vi "ParseResults.vi"(8 "error in (no error)":errorcluster, 10 "Path":path=path "C:/temp/MEScannerF1_262_153145_G16_PD_TS_v3__G16_OC_TS_v2.txt", 11 "Sequence Context In":refnum<k7>) -> (0 "error out":errorcluster, 1 "Array":T1[](array[typedef])=[{"Test_Name"="59. GetScannerDeviceType", "Step_Type"="StringValueTest", "LowLimit"=0.0, "HighLimit"=0.0, "RValue"="7", "RStatus"="PASS", "RetVal"="0", "Units"="", "header1"="", "header2"="\r", "ExpectedValue"=""}, {"Test_Name"="66. PromptUserPassFail \"Please listen for a beep!\" \"OK\" \"Cancel\"", "Step_Type"="StringValueTest", "LowLimit"=0.0, "HighLimit"=0.0, "RValue"="True", "RStatus"="PASS", "RetVal"="None", "Units"="", "header1"="", "header2"="\r\r", "ExpectedValue"=""}, {"Test_Name"="67. Beep", "Step_Type"="", "LowLimit"=0.0, "HighLimit"=0.0, "RValue"="", "RStatus"="", "RetVal"="0", "Units"="", "header1"="", "header2"="\r\r\r", "ExpectedValue"=""}, {"Test_Name"="68. PromptUserPassFail \"Did you hear a beep?\" \"YES\" \"NO\"", "Step_Type"="StringValueTest", "LowLimit"=0.0, "HighLimit"=0.0, "RValue"="True", "RStatus"="PASS", "RetVal"="None", "Units"="", "header1"="", "header2"="\r\r\r\r", "ExpectedValue"=""}, {"Test_Name"="71. SetDebugLEDs \"1\"", "Step_Type"="", "LowLimit"=0.0, "HighLimit"=0.0, "RValue"="", "RStatus"="", "RetVal"="0", "Units"="", "header1"="", "header2"="\r\r\r\r\r", "ExpectedValue"=""}, {"Test_Name"="72. PromptUserPassFail \"Did you Verify the 2 LEDs turn on near uSD connector?\" \"YES\" \"NO\"", "Step_Type"="StringValueTest", "LowLimit"=0.0, "HighLimit"=0.0, "RValue"="True", "RStatus"="PASS", "RetVal"="None", "Units"="", "header1"="", "header2"="\r\r\r\r\r\r", "ExpectedValue"=""}, {"Test_Name"="73. SetDebugLEDs \"0\"", "Step_Type"="", "LowLimit"=0.0, "HighLimit"=0.0, "RValue"="", "RStatus"="", "RetVal"="0", "Units"="", "header1"="", "header2"="\r\r\r\r\r\r\r", "ExpectedValue"=""}, {"Test_Name"="93. --- Pin Driver Complete Test ---", "Step_Type"="", "LowLimit"=0.0, "HighLimit"=0.0, "RValue"="", "RStatus"="", "RetVal"="", "Units"="", "header1"="", "header2"="--- Pin Driver Complete Test -----------\r", "ExpectedValue"=""}, {"Test_Name"="96. SetG15PullupVbat \"0\" \"0\"", "Step_Type"="", "LowLimit"=0.0, "HighLimit"=0.0, "RValue"="", "RStatus"="", "RetVal"="0", "Units"="", "header1"="", "header2"="--- Pin Driver Complete Test -----------\r\r", "ExpectedValue"=""}, {"Test_Name"="97. SetG15PullUp \"A\" \"0\"", "Step_Type"="", "LowLimit"=0.0, "HighLimit"=0.0, "RValue"="", "RStatus"="", "RetVal"="0", "Units"="", "header1"="", "header2"="--- Pin Driver Complete Test -----------\r\r\r", "ExpectedValue"=""}, {"Test_Name"="98. SetG15PullUp \"B\" \"0\"", "Step_Type"="", "LowLimit"=0.0, "HighLimit"=0.0, "RValue"="", "RStatus"="", "RetVal"="0", "Units"="", "header1"="", "header2"="--- Pin Driver Complete Test -----------\r\r\r\r", "ExpectedValue"=""}, {"Test_Name"="99. SetG15PullDown \"A\" \"0\"", "Step_Type"="", "LowLimit"=0.0, "HighLimit"=0.0, "RValue"="", "RStatus"="", "RetVal"="0", "Units"="", "header1"="", "header2"="--- Pin Driver Complete Test -----------\r\r\r\r\r", "ExpectedValue"=""}, {"Test_Name"="100. SetG15PullDown \"B\" \"0\"", "Step_Type"="", "LowLimit"=0.0, "HighLimit"=0.0, "RValue"="", "RStatus"="", "RetVal"="0", "Units"="", "header1"="", "header2"="--- Pin Driver Complete Test -----------\r\r\r\r\r\r", "ExpectedValue"=""}, {"Test_Name"="101. SelectAllMuxA \"1\" \"0\"", "Step_Type"="", "LowLimit"=0.0, "HighLimit"=0.0, "RValue"="", "RStatus"="", "RetVal"="0", "Units"="", "header1"="", "header2"="--- Pin Driver Complete Test -----------\r\r\r\r\r\r\r", "ExpectedValue"=""}, {"Test_Name"="102. SelectAllMuxB \"1\" \"0\"", "Step_Type"="", "LowLimit"=0.0, "HighLimit"=0.0, "RValue"="", "RStatus"="", "RetVal"="0", "Units"="", "header1"="", "header2"="--- Pin Driver Complete Test -----------\r\r\r\r\r\r\r\r", "ExpectedValue"=""}, {"Test_Name"="103. SetG15PullUp \"C\" \"0\"", "Step_Type"="", "LowLimit"=0.0, "HighLimit"=0.0, "RValue"="", "RStatus"="", "RetVal"="0", "Units"="", "header1"="", "header2"="--- Pin Driver Complete Test -----------\r\r\r\r\r\r\r\r\r", "ExpectedValue"=""}, {"Test_Name"="104. SetG15PullUp \"D\" \"0\"", "Step_Type"="", "LowLimit"=0.0, "HighLimit"=0.0, "RValue"="", "RStatus"="", "RetVal"="0", "Units"="", "header1"="", "header2"="--- Pin Driver Complete Test -----------\r\r\r\r\r\r\r\r\r\r", "ExpectedValue"=""}, {"Test_Name"="105. SetG15PullDown \"C\" \"0\"", "Step_Type"="", "LowLimit"=0.0, "HighLimit"=0.0, "RValue"="", "RStatus"="", "RetVal"="0", "Units"="", "header1"="", "header2"="--- Pin Driver Complete Test -----------\r\r\r\r\r\r\r\r\r\r\r", "ExpectedValue"=""}, {"Test_Name"="106. SetG15PullDown \"D\" \"0\"", "Step_Type"="", "LowLimit"=0.0, "HighLimit"=0.0, "RValue"="", "RStatus"="", "RetVal"="0", "Units"="", "header1"="", "header2"="--- Pin Driver Complete Test -----------\r\r\r\r\r\r\r\r\r\r\r\r", "ExpectedValue"=""}, {"Test_Name"="107. SelectAllMuxA \"2\" \"0\"", "Step_Type"="", "LowLimit"=0.0, "HighLimit"=0.0, "RValue"="", "RStatus"="", "RetVal"="0", "Units"="", "header1"="", "header2"="--- Pin Driver Complete Test -----------\r\r\r\r\r\r\r\r\r\r\r\r\r", "ExpectedValue"=""}, {"Test_Name"="108. SelectAllMuxB \"2\" \"0\"", "Step_Type"="", "LowLimit"=0.0, "HighLimit"=0.0, "RValue"="", "RStatus"="", "RetVal"="0", "Units"="", "header1"="", "header2"="--- Pin Driver Complete Test -----------\r\r\r\r\r\r\r\r\r\r\r\r\r\r", "ExpectedValue"=""}, {"Test_Name"="109. SelectAllPins \"0\"", "Step_Type"="", "LowLimit"=0.0, "HighLimit"=0.0, "RValue"="", "RStatus"="", "RetVal"="0", "Units"="", "header1"="", "header2"="--- Pin Driver Complete Test -----------\r\r\r\r\r\r\r\r\r\r\r\r\r\r\r", "ExpectedValue"=""}, {"Test_Name"="110. ResetAsicRegister \"1\" \"ALL\"", "Step_Type"="", "LowLimit"=0.0, "HighLimit"=0.0, "RValue"="", "RStatus"="", "RetVal"="0", "Units"="", "header1"="", "header2"="--- Pin Driver Complete Test -----------\r\r\r\r\r\r\r\r\r\r\r\r\r\r\r\r", "ExpectedValue"=""}, {"Test_Name"="111. ResetAsicRegister \"2\" \"ALL\"", "Step_Type"="", "LowLimit"=0.0, "HighLimit"=0.0, "RValue"="", "RStatus"="", "RetVal"="0", "Units"="", "header1"="", "header2"="--- Pin Driver Complete Test -----------\r\r\r\r\r\r\r\r\r\r\r\r\r\r\r\r\r", "ExpectedValue"=""}, {"Test_Name"="112. SetFpgaRegister \"129\" \"0\"", "Step_Type"="", "LowLimit"=0.0, "HighLimit"=0.0, "RValue"="", "RStatus"="", "RetVal"="0", "Units"="", "header1"="", "header2"="--- Pin Driver Complete Test -----------\r\r\r\r\r\r\r\r\r\r\r\r\r\r\r\r\r\r", "ExpectedValue"=""}, {"Test_Name"="113. SetFpgaRegister \"8AD\" \"1\"", "Step_Type"="", "LowLimit"=0.0, "HighLimit"=0.0, "RValue"="", "RStatus"="", "RetVal"="0", "Units"="", "header1"="", "header2"="--- Pin Driver Complete Test -----------\r\r\r\r\r\r\r\r\r\r\r\r\r\r\r\r\r\r\r", "ExpectedValue"=""}, {"Test_Name"="115. ---CHECK System MEMORY---", "Step_Type"="", "LowLimit"=0.0, "HighLimit"=0.0, "RValue"="", "RStatus"="", "RetVal"="", "Units"="", "header1"="", "header2"="---CHECK System MEMORY------------------\r", "ExpectedValue"=""}, {"Test_Name"="116. CheckSystemMemory", "Step_Type"="", "LowLimit"=0.0, "HighLimit"=0.0, "RValue"="", "RStatus"="", "RetVal"="0", "Units"="", "header1"="", "header2"="---CHECK System MEMORY------------------\r\r", "ExpectedValue"=""}, {"Test_Name"="118. --- Software Verification ---", "Step_Type"="", "LowLimit"=0.0, "HighLimit"=0.0, "RValue"="", "RStatus"="", "RetVal"="", "Units"="", "header1"="", "header2"="--- Software Verification --------------\r", "ExpectedValue"=""}, {"Test_Name"="119. CheckTestAppVersion \"2.6\"", "Step_Type"="StringValueTest", "LowLimit"=0.0, "HighLimit"=0.0, "RValue"="2.6", "RStatus"="PASS", "RetVal"="None", "Units"="", "header1"="", "header2"="--- Software Verification --------------\r\r", "ExpectedValue"=""}, {"Test_Name"="120. CheckFPGAVersion \"2.7\"", "Step_Type"="StringValueTest", "LowLimit"=0.0, "HighLimit"=0.0, "RValue"="2.7", "RStatus"="PASS", "RetVal"="None", "Units"="", "header1"="", "header2"="--- Software Verification --------------\r\r\r", "ExpectedValue"=""}, {"Test_Name"="121. CheckIPLVersion \"0.6\"", "Step_Type"="StringValueTest", "LowLimit"=0.0, "HighLimit"=0.0, "RValue"="0.6", "RStatus"="PASS", "RetVal"="None", "Units"="", "header1"="", "header2"="--- Software Verification --------------\r\r\r\r", "ExpectedValue"=""}, {"Test_Name"="122. CheckSPL1Version \"0.8\"", "Step_Type"="StringValueTest", "LowLimit"=0.0, "HighLimit"=0.0, "RValue"="0.8", "RStatus"="PASS", "RetVal"="None", "Units"="", "header1"="", "header2"="--- Software Verification --------------\r\r\r\r\r", "ExpectedValue"=""}, {"Test_Name"="125. SetRealtimeClock", "Step_Type"="", "LowLimit"=0.0, "HighLimit"=0.0, "RValue"="", "RStatus"="", "RetVal"="0", "Units"="", "header1"="", "header2"="--- Software Verification --------------\r\r\r\r\r\r", "ExpectedValue"=""}, {"Test_Name"="127. ---   ADC VEHICLE VBAT check ---", "Step_Type"="", "LowLimit"=0.0, "HighLimit"=0.0, "RValue"="", "RStatus"="", "RetVal"="", "Units"="", "header1"="", "header2"="---   ADC VEHICLE VBAT check -----------\r", "ExpectedValue"=""}, {"Test_Name"="128. CheckCFAdc \"VBAT\" \"14.5\" \"15.6\"", "Step_Type"="NumericLimitTest", "LowLimit"=14.5, "HighLimit"=15.6, "RValue"="14.722999572753906", "RStatus"="PASS", "RetVal"="0", "Units"="Volts", "header1"="", "header2"="---   ADC VEHICLE VBAT check -----------\r\r", "ExpectedValue"=""}, {"Test_Name"="129. Apply_10V_to_J5001-T5002.exe", "Step_Type"="", "LowLimit"=0.0, "HighLimit"=0.0, "RValue"="", "RStatus"="", "RetVal"="", "Units"="", "header1"="", "header2"="---   ADC VEHICLE VBAT check -----------\r\r\r", "ExpectedValue"=""}, {"Test_Name"="131. CheckCFAdc \"PVA_Volts\" \"9.7\" \"10.3\"", "Step_Type"="NumericLimitTest", "LowLimit"=9.7, "HighLimit"=10.3, "RValue"="9.906999588012695", "RStatus"="PASS", "RetVal"="0", "Units"="Volts", "header1"="", "header2"="---   ADC VEHICLE VBAT check -----------\r\r\r\r", "ExpectedValue"=""}, {"Test_Name"="133. --- 20 VOLT CAL CHECK ---", "Step_Type"="", "LowLimit"=0.0, "HighLimit"=0.0, "RValue"="", "RStatus"="", "RetVal"="", "Units"="", "header1"="", "header2"="--- 20 VOLT CAL CHECK ------------------\r", "ExpectedValue"=""}, {"Test_Name"="134. Apply_20V_to_J5000-1.exe", "Step_Type"="", "LowLimit"=0.0, "HighLimit"=0.0, "RValue"="", "RStatus"="", "RetVal"="", "Units"="", "header1"="", "header2"="--- 20 VOLT CAL CHECK ------------------\r\r", "ExpectedValue"=""}, {"Test_Name"="136. SelectMuxA \"1\" \"1\" \"1\"", "Step_Type"="", "LowLimit"=0.0, "HighLimit"=0.0, "RValue"="", "RStatus"="", "RetVal"="0", "Units"="", "header1"="", "header2"="--- 20 VOLT CAL CHECK ------------------\r\r\r", "ExpectedValue"=""}, {"Test_Name"="137. SelectMuxB \"1\" \"1\" \"1\"", "Step_Type"="", "LowLimit"=0.0, "HighLimit"=0.0, "RValue"="", "RStatus"="", "RetVal"="0", "Units"="", "header1"="", "header2"="--- 20 VOLT CAL CHECK ------------------\r\r\r\r", "ExpectedValue"=""}, {"Test_Name"="138. SelectMuxA \"2\" \"1\" \"1\"", "Step_Type"="", "LowLimit"=0.0, "HighLimit"=0.0, "RValue"="", "RStatus"="", "RetVal"="0", "Units"="", "header1"="", "header2"="--- 20 VOLT CAL CHECK ------------------\r\r\r\r\r", "ExpectedValue"=""}, {"Test_Name"="139. SelectMuxB \"2\" \"1\" \"1\"", "Step_Type"="", "LowLimit"=0.0, "HighLimit"=0.0, "RValue"="", "RStatus"="", "RetVal"="0", "Units"="", "header1"="", "header2"="--- 20 VOLT CAL CHECK ------------------\r\r\r\r\r\r", "ExpectedValue"=""}, {"Test_Name"="140. CheckCFAdc \"PD1\" \"19.5\" \"20.5\"", "Step_Type"="NumericLimitTest", "LowLimit"=19.5, "HighLimit"=20.5, "RValue"="20.009000778198242", "RStatus"="PASS", "RetVal"="0", "Units"="Volts", "header1"="", "header2"="--- 20 VOLT CAL CHECK ------------------\r\r\r\r\r\r\r", "ExpectedValue"=""}, {"Test_Name"="141. CheckCFAdc \"PD2\" \"19.5\" \"20.5\"", "Step_Type"="NumericLimitTest", "LowLimit"=19.5, "HighLimit"=20.5, "RValue"="20.009000778198242", "RStatus"="PASS", "RetVal"="0", "Units"="Volts", "header1"="", "header2"="--- 20 VOLT CAL CHECK ------------------\r\r\r\r\r\r\r\r", "ExpectedValue"=""}, {"Test_Name"="142. CheckCFAdc \"PD3\" \"19.5\" \"20.5\"", "Step_Type"="NumericLimitTest", "LowLimit"=19.5, "HighLimit"=20.5, "RValue"="20.01799964904785", "RStatus"="PASS", "RetVal"="0", "Units"="Volts", "header1"="", "header2"="--- 20 VOLT CAL CHECK ------------------\r\r\r\r\r\r\r\r\r", "ExpectedValue"=""}, {"Test_Name"="143. CheckCFAdc \"PD4\" \"19.5\" \"20.5\"", "Step_Type"="NumericLimitTest", "LowLimit"=19.5, "HighLimit"=20.5, "RValue"="20.009000778198242", "RStatus"="PASS", "RetVal"="0", "Units"="Volts", "header1"="", "header2"="--- 20 VOLT CAL CHECK ------------------\r\r\r\r\r\r\r\r\r\r", "ExpectedValue"=""}, {"Test_Name"="144. CheckFpgaRegister \"8ae\" \"0\" \"1\"", "Step_Type"="StringValueTest", "LowLimit"=0.0, "HighLimit"=0.0, "RValue"="1", "RStatus"="PASS", "RetVal"="0", "Units"="", "header1"="", "header2"="--- 20 VOLT CAL CHECK ------------------\r\r\r\r\r\r\r\r\r\r\r", "ExpectedValue"=""}, {"Test_Name"="145. SelectMuxA \"1\" \"1\" \"0\"", "Step_Type"="", "LowLimit"=0.0, "HighLimit"=0.0, "RValue"="", "RStatus"="", "RetVal"="0", "Units"="", "header1"="", "header2"="--- 20 VOLT CAL CHECK ------------------\r\r\r\r\r\r\r\r\r\r\r\r", "ExpectedValue"=""}, {"Test_Name"="146. SelectMuxB \"1\" \"1\" \"0\"", "Step_Type"="", "LowLimit"=0.0, "HighLimit"=0.0, "RValue"="", "RStatus"="", "RetVal"="0", "Units"="", "header1"="", "header2"="--- 20 VOLT CAL CHECK ------------------\r\r\r\r\r\r\r\r\r\r\r\r\r", "ExpectedValue"=""}, {"Test_Name"="147. SelectMuxA \"2\" \"1\" \"0\"", "Step_Type"="", "LowLimit"=0.0, "HighLimit"=0.0, "RValue"="", "RStatus"="", "RetVal"="0", "Units"="", "header1"="", "header2"="--- 20 VOLT CAL CHECK ------------------\r\r\r\r\r\r\r\r\r\r\r\r\r\r", "ExpectedValue"=""}, {"Test_Name"="148. SelectMuxB \"2\" \"1\" \"0\"", "Step_Type"="", "LowLimit"=0.0, "HighLimit"=0.0, "RValue"="", "RStatus"="", "RetVal"="0", "Units"="", "header1"="", "header2"="--- 20 VOLT CAL CHECK ------------------\r\r\r\r\r\r\r\r\r\r\r\r\r\r\r", "ExpectedValue"=""}, {"Test_Name"="149. Disconnect_Voltage_Reference_from_UUT.exe", "Step_Type"="", "LowLimit"=0.0, "HighLimit"=0.0, "RValue"="", "RStatus"="", "RetVal"="", "Units"="", "header1"="", "header2"="--- 20 VOLT CAL CHECK ------------------\r\r\r\r\r\r\r\r\r\r\r\r\r\r\r\r", "ExpectedValue"=""}, {"Test_Name"="153. --- Start Pin Driver test for ASIC 1 ---", "Step_Type"="", "LowLimit"=0.0, "HighLimit"=0.0, "RValue"="", "RStatus"="", "RetVal"="", "Units"="", "header1"="", "header2"="--- Start Pin Driver test for ASIC 1 ---\r", "ExpectedValue"=""}, {"Test_Name"="155. SetReference \"128\"", "Step_Type"="", "LowLimit"=0.0, "HighLimit"=0.0, "RValue"="", "RStatus"="", "RetVal"="0", "Units"="", "header1"="", "header2"="--- Start Pin Driver test for ASIC 1 ---\r\r", "ExpectedValue"=""}, {"Test_Name"="156. SetBaud \"1\"", "Step_Type"="", "LowLimit"=0.0, "HighLimit"=0.0, "RValue"="", "RStatus"="", "RetVal"="0", "Units"="", "header1"="", "header2"="--- Start Pin Driver test for ASIC 1 ---\r\r\r", "ExpectedValue"=""}, {"Test_Name"="157. SelectAllMuxA \"1\" \"0\"", "Step_Type"="", "LowLimit"=0.0, "HighLimit"=0.0, "RValue"="", "RStatus"="", "RetVal"="0", "Units"="", "header1"="", "header2"="--- Start Pin Driver test for ASIC 1 ---\r\r\r\r", "ExpectedValue"=""}, {"Test_Name"="158. SelectAllMuxB \"1\" \"0\"", "Step_Type"="", "LowLimit"=0.0, "HighLimit"=0.0, "RValue"="", "RStatus"="", "RetVal"="0", "Units"="", "header1"="", "header2"="--- Start Pin Driver test for ASIC 1 ---\r\r\r\r\r", "ExpectedValue"=""}, {"Test_Name"="159. SelectAllMuxA \"2\" \"0\"", "Step_Type"="", "LowLimit"=0.0, "HighLimit"=0.0, "RValue"="", "RStatus"="", "RetVal"="0", "Units"="", "header1"="", "header2"="--- Start Pin Driver test for ASIC 1 ---\r\r\r\r\r\r", "ExpectedValue"=""}, {"Test_Name"="160. SelectAllMuxB \"2\" \"0\"", "Step_Type"="", "LowLimit"=0.0, "HighLimit"=0.0, "RValue"="", "RStatus"="", "RetVal"="0", "Units"="", "header1"="", "header2"="--- Start Pin Driver test for ASIC 1 ---\r\r\r\r\r\r\r", "ExpectedValue"=""}, {"Test_Name"="163. SetG15PullUp \"A\" \"1\"", "Step_Type"="", "LowLimit"=0.0, "HighLimit"=0.0, "RValue"="", "RStatus"="", "RetVal"="0", "Units"="", "header1"="", "header2"="--- Start Pin Driver test for ASIC 1 ---\r\r\r\r\r\r\r\r", "ExpectedValue"=""}, {"Test_Name"="164. SetG15PullUp \"B\" \"1\"", "Step_Type"="", "LowLimit"=0.0, "HighLimit"=0.0, "RValue"="", "RStatus"="", "RetVal"="0", "Units"="", "header1"="", "header2"="--- Start Pin Driver test for ASIC 1 ---\r\r\r\r\r\r\r\r\r", "ExpectedValue"=""}, {"Test_Name"="165. CheckCFAdc \"PD1\" \"4.5\" \"5.0\"", "Step_Type"="NumericLimitTest", "LowLimit"=4.5, "HighLimit"=5.0, "RValue"="4.775000095367432", "RStatus"="PASS", "RetVal"="0", "Units"="Volts", "header1"="", "header2"="--- Start Pin Driver test for ASIC 1 ---\r\r\r\r\r\r\r\r\r\r", "ExpectedValue"=""}, {"Test_Name"="166. CheckCFAdc \"PD2\" \"4.5\" \"5.0\"", "Step_Type"="NumericLimitTest", "LowLimit"=4.5, "HighLimit"=5.0, "RValue"="4.78000020980835", "RStatus"="PASS", "RetVal"="0", "Units"="Volts", "header1"="", "header2"="--- Start Pin Driver test for ASIC 1 ---\r\r\r\r\r\r\r\r\r\r\r", "ExpectedValue"=""}, {"Test_Name"="169. SetG15PullDown \"A\" \"3\"", "Step_Type"="", "LowLimit"=0.0, "HighLimit"=0.0, "RValue"="", "RStatus"="", "RetVal"="0", "Units"="", "header1"="", "header2"="--- Start Pin Driver test for ASIC 1 ---\r\r\r\r\r\r\r\r\r\r\r\r", "ExpectedValue"=""}, {"Test_Name"="170. SetG15PullDown \"B\" \"3\"", "Step_Type"="", "LowLimit"=0.0, "HighLimit"=0.0, "RValue"="", "RStatus"="", "RetVal"="0", "Units"="", "header1"="", "header2"="--- Start Pin Driver test for ASIC 1 ---\r\r\r\r\r\r\r\r\r\r\r\r\r", "ExpectedValue"=""}, {"Test_Name"="171. CheckCFAdc \"PD1\" \"4.1\" \"4.55\"", "Step_Type"="NumericLimitTest", "LowLimit"=4.1, "HighLimit"=4.55, "RValue"="4.36899995803833", "RStatus"="PASS", "RetVal"="0", "Units"="Volts", "header1"="", "header2"="--- Start Pin Driver test for ASIC 1 ---\r\r\r\r\r\r\r\r\r\r\r\r\r\r", "ExpectedValue"=""}, {"Test_Name"="172. CheckCFAdc \"PD2\" \"4.1\" \"4.55\"", "Step_Type"="NumericLimitTest", "LowLimit"=4.1, "HighLimit"=4.55, "RValue"="4.364999771118164", "RStatus"="PASS", "RetVal"="0", "Units"="Volts", "header1"="", "header2"="--- Start Pin Driver test for ASIC 1 ---\r\r\r\r\r\r\r\r\r\r\r\r\r\r\r", "ExpectedValue"=""}, {"Test_Name"="175. SetG15PullUp \"A\" \"7\"", "Step_Type"="", "LowLimit"=0.0, "HighLimit"=0.0, "RValue"="", "RStatus"="", "RetVal"="0", "Units"="", "header1"="", "header2"="--- Start Pin Driver test for ASIC 1 ---\r\r\r\r\r\r\r\r\r\r\r\r\r\r\r\r", "ExpectedValue"=""}, {"Test_Name"="176. SetG15PullUp \"B\" \"7\"", "Step_Type"="", "LowLimit"=0.0, "HighLimit"=0.0, "RValue"="", "RStatus"="", "RetVal"="0", "Units"="", "header1"="", "header2"="--- Start Pin Driver test for ASIC 1 ---\r\r\r\r\r\r\r\r\r\r\r\r\r\r\r\r\r", "ExpectedValue"=""}, {"Test_Name"="177. CheckCFAdc \"PD1\" \"2.3\" \"2.6\"", "Step_Type"="NumericLimitTest", "LowLimit"=2.3, "HighLimit"=2.6, "RValue"="2.428999900817871", "RStatus"="PASS", "RetVal"="0", "Units"="Volts", "header1"="", "header2"="--- Start Pin Driver test for ASIC 1 ---\r\r\r\r\r\r\r\r\r\r\r\r\r\r\r\r\r\r", "ExpectedValue"=""}, {"Test_Name"="178. CheckCFAdc \"PD2\" \"2.3\" \"2.6\"", "Step_Type"="NumericLimitTest", "LowLimit"=2.3, "HighLimit"=2.6, "RValue"="2.444999933242798", "RStatus"="PASS", "RetVal"="0", "Units"="Volts", "header1"="", "header2"="--- Start Pin Driver test for ASIC 1 ---\r\r\r\r\r\r\r\r\r\r\r\r\r\r\r\r\r\r\r", "ExpectedValue"=""}, {"Test_Name"="181. SetG15PullUp \"A\" \"1\"", "Step_Type"="", "LowLimit"=0.0, "HighLimit"=0.0, "RValue"="", "RStatus"="", "RetVal"="0", "Units"="", "header1"="", "header2"="--- Start Pin Driver test for ASIC 1 ---\r\r\r\r\r\r\r\r\r\r\r\r\r\r\r\r\r\r\r\r", "ExpectedValue"=""}, {"Test_Name"="182. SetG15PullUp \"B\" \"1\"", "Step_Type"="", "LowLimit"=0.0, "HighLimit"=0.0, "RValue"="", "RStatus"="", "RetVal"="0", "Units"="", "header1"="", "header2"="--- Start Pin Driver test for ASIC 1 ---\r\r\r\r\r\r\r\r\r\r\r\r\r\r\r\r\r\r\r\r\r", "ExpectedValue"=""}, {"Test_Name"="183. SetG15PullDown \"A\" \"4\"", "Step_Type"="", "LowLimit"=0.0, "HighLimit"=0.0, "RValue"="", "RStatus"="", "RetVal"="0", "Units"="", "header1"="", "header2"="--- Start Pin Driver test for ASIC 1 ---\r\r\r\r\r\r\r\r\r\r\r\r\r\r\r\r\r\r\r\r\r\r", "ExpectedValue"=""}, {"Test_Name"="184. SetG15PullDown \"B\" \"4\"", "Step_Type"="", "LowLimit"=0.0, "HighLimit"=0.0, "RValue"="", "RStatus"="", "RetVal"="0", "Units"="", "header1"="", "header2"="--- Start Pin Driver test for ASIC 1 ---\r\r\r\r\r\r\r\r\r\r\r\r\r\r\r\r\r\r\r\r\r\r\r", "ExpectedValue"=""}, {"Test_Name"="185. CheckCFAdc \"PD1\" \"4.35\" \"4.85\"", "Step_Type"="NumericLimitTest", "LowLimit"=4.35, "HighLimit"=4.85, "RValue"="4.599999904632568", "RStatus"="PASS", "RetVal"="0", "Units"="Volts", "header1"="", "header2"="--- Start Pin Driver test for ASIC 1 ---\r\r\r\r\r\r\r\r\r\r\r\r\r\r\r\r\r\r\r\r\r\r\r\r", "ExpectedValue"=""}, {"Test_Name"="186. CheckCFAdc \"PD2\" \"4.35\" \"4.85\"", "Step_Type"="NumericLimitTest", "LowLimit"=4.35, "HighLimit"=4.85, "RValue"="4.613999843597412", "RStatus"="PASS", "RetVal"="0", "Units"="Volts", "header1"="", "header2"="--- Start Pin Driver test for ASIC 1 ---\r\r\r\r\r\r\r\r\r\r\r\r\r\r\r\r\r\r\r\r\r\r\r\r\r", "ExpectedValue"=""}, {"Test_Name"="189. SetG15PullUp \"A\" \"2\"", "Step_Type"="", "LowLimit"=0.0, "HighLimit"=0.0, "RValue"="", "RStatus"="", "RetVal"="0", "Units"="", "header1"="", "header2"="--- Start Pin Driver test for ASIC 1 ---\r\r\r\r\r\r\r\r\r\r\r\r\r\r\r\r\r\r\r\r\r\r\r\r\r\r", "ExpectedValue"=""}, {"Test_Name"="190. SetG15PullUp \"B\" \"2\"", "Step_Type"="", "LowLimit"=0.0, "HighLimit"=0.0, "RValue"="", "RStatus"="", "RetVal"="0", "Units"="", "header1"="", "header2"="--- Start Pin Driver test for ASIC 1 ---\r\r\r\r\r\r\r\r\r\r\r\r\r\r\r\r\r\r\r\r\r\r\r\r\r\r\r", "ExpectedValue"=""}, {"Test_Name"="191. SetG15PullDown \"A\" \"3\"", "Step_Type"="", "LowLimit"=0.0, "HighLimit"=0.0, "RValue"="", "RStatus"="", "RetVal"="0", "Units"="", "header1"="", "header2"="--- Start Pin Driver test for ASIC 1 ---\r\r\r\r\r\r\r\r\r\r\r\r\r\r\r\r\r\r\r\r\r\r\r\r\r\r\r\r", "ExpectedValue"=""}, {"Test_Name"="192. SetG15PullDown \"B\" \"3\"", "Step_Type"="", "LowLimit"=0.0, "HighLimit"=0.0, "RValue"="", "RStatus"="", "RetVal"="0", "Units"="", "header1"="", "header2"="--- Start Pin Driver test for ASIC 1 ---\r\r\r\r\r\r\r\r\r\r\r\r\r\r\r\r\r\r\r\r\r\r\r\r\r\r\r\r\r", "ExpectedValue"=""}, {"Test_Name"="193. CheckCFAdc \"PD1\" \"3.95\" \"4.45\"", "Step_Type"="NumericLimitTest", "LowLimit"=3.95, "HighLimit"=4.45, "RValue"="4.230000019073486", "RStatus"="PASS", "RetVal"="0", "Units"="Volts", "header1"="", "header2"="--- Start Pin Driver test for ASIC 1 ---\r\r\r\r\r\r\r\r\r\r\r\r\r\r\r\r\r\r\r\r\r\r\r\r\r\r\r\r\r\r", "ExpectedValue"=""}, {"Test_Name"="194. CheckCFAdc \"PD2\" \"3.95\" \"4.45\"", "Step_Type"="NumericLimitTest", "LowLimit"=3.95, "HighLimit"=4.45, "RValue"="4.236000061035156", "RStatus"="PASS", "RetVal"="0", "Units"="Volts", "header1"="", "header2"="--- Start Pin Driver test for ASIC 1 ---\r\r\r\r\r\r\r\r\r\r\r\r\r\r\r\r\r\r\r\r\r\r\r\r\r\r\r\r\r\r\r", "ExpectedValue"=""}, {"Test_Name"="197. SetG15PullUp \"A\" \"2\"", "Step_Type"="", "LowLimit"=0.0, "HighLimit"=0.0, "RValue"="", "RStatus"="", "RetVal"="0", "Units"="", "header1"="", "header2"="--- Start Pin Driver test for ASIC 1 ---\r\r\r\r\r\r\r\r\r\r\r\r\r\r\r\r\r\r\r\r\r\r\r\r\r\r\r\r\r\r\r\r", "ExpectedValue"=""}, {"Test_Name"="198. SetG15PullUp \"B\" \"2\"", "Step_Type"="", "LowLimit"=0.0, "HighLimit"=0.0, "RValue"="", "RStatus"="", "RetVal"="0", "Units"="", "header1"="", "header2"="--- Start Pin Driver test for ASIC 1 ---\r\r\r\r\r\r\r\r\r\r\r\r\r\r\r\r\r\r\r\r\r\r\r\r\r\r\r\r\r\r\r\r\r", "ExpectedValue"=""}, {"Test_Name"="199. SetG15PullDown \"A\" \"4\"", "Step_Type"="", "LowLimit"=0.0, "HighLimit"=0.0, "RValue"="", "RStatus"="", "RetVal"="0", "Units"="", "header1"="", "header2"="--- Start Pin Driver test for ASIC 1 ---\r\r\r\r\r\r\r\r\r\r\r\r\r\r\r\r\r\r\r\r\r\r\r\r\r\r\r\r\r\r\r\r\r\r", "ExpectedValue"=""}, {"Test_Name"="200. SetG15PullDown \"B\" \"4\"", "Step_Type"="", "LowLimit"=0.0, "HighLimit"=0.0, "RValue"="", "RStatus"="", "RetVal"="0", "Units"="", "header1"="", "header2"="--- Start Pin Driver test for ASIC 1 ---\r\r\r\r\r\r\r\r\r\r\r\r\r\r\r\r\r\r\r\r\r\r\r\r\r\r\r\r\r\r\r\r\r\r\r", "ExpectedValue"=""}, {"Test_Name"="201. CheckCFAdc \"PD1\" \"4.3\" \"4.8\"", "Step_Type"="NumericLimitTest", "LowLimit"=4.3, "HighLimit"=4.8, "RValue"="4.563000202178955", "RStatus"="PASS", "RetVal"="0", "Units"="Volts", "header1"="", "header2"="--- Start Pin Driver test for ASIC 1 ---\r\r\r\r\r\r\r\r\r\r\r\r\r\r\r\r\r\r\r\r\r\r\r\r\r\r\r\r\r\r\r\r\r\r\r\r", "ExpectedValue"=""}, {"Test_Name"="202. CheckCFAdc \"PD2\" \"4.3\" \"4.8\"", "Step_Type"="NumericLimitTest", "LowLimit"=4.3, "HighLimit"=4.8, "RValue"="4.567999839782715", "RStatus"="PASS", "RetVal"="0", "Units"="Volts", "header1"="", "header2"="--- Start Pin Driver test for ASIC 1 ---\r\r\r\r\r\r\r\r\r\r\r\r\r\r\r\r\r\r\r\r\r\r\r\r\r\r\r\r\r\r\r\r\r\r\r\r\r", "ExpectedValue"=""}, {"Test_Name"="205. SetG15PullUp \"A\" \"3\"", "Step_Type"="", "LowLimit"=0.0, "HighLimit"=0.0, "RValue"="", "RStatus"="", "RetVal"="0", "Units"="", "header1"="", "header2"="--- Start Pin Driver test for ASIC 1 ---\r\r\r\r\r\r\r\r\r\r\r\r\r\r\r\r\r\r\r\r\r\r\r\r\r\r\r\r\r\r\r\r\r\r\r\r\r\r", "ExpectedValue"=""}, {"Test_Name"="206. SetG15PullUp \"B\" \"3\"", "Step_Type"="", "LowLimit"=0.0, "HighLimit"=0.0, "RValue"="", "RStatus"="", "RetVal"="0", "Units"="", "header1"="", "header2"="--- Start Pin Driver test for ASIC 1 ---\r\r\r\r\r\r\r\r\r\r\r\r\r\r\r\r\r\r\r\r\r\r\r\r\r\r\r\r\r\r\r\r\r\r\r\r\r\r\r", "ExpectedValue"=""}, {"Test_Name"="207. SetG15PullDown \"A\" \"4\"", "Step_Type"="", "LowLimit"=0.0, "HighLimit"=0.0, "RValue"="", "RStatus"="", "RetVal"="0", "Units"="", "header1"="", "header2"="--- Start Pin Driver test for ASIC 1 ---\r\r\r\r\r\r\r\r\r\r\r\r\r\r\r\r\r\r\r\r\r\r\r\r\r\r\r\r\r\r\r\r\r\r\r\r\r\r\r\r", "ExpectedValue"=""}, {"Test_Name"="208. SetG15PullDown \"B\" \"4\"", "Step_Type"="", "LowLimit"=0.0, "HighLimit"=0.0, "RValue"="", "RStatus"="", "RetVal"="0", "Units"="", "header1"="", "header2"="--- Start Pin Driver test for ASIC 1 ---\r\r\r\r\r\r\r\r\r\r\r\r\r\r\r\r\r\r\r\r\r\r\r\r\r\r\r\r\r\r\r\r\r\r\r\r\r\r\r\r\r", "ExpectedValue"=""}, {"Test_Name"="209. CheckCFAdc \"PD1\" \"4.1\" \"4.6\"", "Step_Type"="NumericLimitTest", "LowLimit"=4.1, "HighLimit"=4.6, "RValue"="4.314000129699707", "RStatus"="PASS", "RetVal"="0", "Units"="Volts", "header1"="", "header2"="--- Start Pin Driver test for ASIC 1 ---\r\r\r\r\r\r\r\r\r\r\r\r\r\r\r\r\r\r\r\r\r\r\r\r\r\r\r\r\r\r\r\r\r\r\r\r\r\r\r\r\r\r", "ExpectedValue"=""}, {"Test_Name"="210. CheckCFAdc \"PD2\" \"4.1\" \"4.6\"", "Step_Type"="NumericLimitTest", "LowLimit"=4.1, "HighLimit"=4.6, "RValue"="4.328000068664551", "RStatus"="PASS", "RetVal"="0", "Units"="Volts", "header1"="", "header2"="--- Start Pin Driver test for ASIC 1 ---\r\r\r\r\r\r\r\r\r\r\r\r\r\r\r\r\r\r\r\r\r\r\r\r\r\r\r\r\r\r\r\r\r\r\r\r\r\r\r\r\r\r\r", "ExpectedValue"=""}, {"Test_Name"="213. SetG15PullUp \"A\" \"4\"", "Step_Type"="", "LowLimit"=0.0, "HighLimit"=0.0, "RValue"="", "RStatus"="", "RetVal"="0", "Units"="", "header1"="", "header2"="--- Start Pin Driver test for ASIC 1 ---\r\r\r\r\r\r\r\r\r\r\r\r\r\r\r\r\r\r\r\r\r\r\r\r\r\r\r\r\r\r\r\r\r\r\r\r\r\r\r\r\r\r\r\r", "ExpectedValue"=""}, {"Test_Name"="214. SetG15PullUp \"B\" \"4\"", "Step_Type"="", "LowLimit"=0.0, "HighLimit"=0.0, "RValue"="", "RStatus"="", "RetVal"="0", "Units"="", "header1"="", "header2"="--- Start Pin Driver test for ASIC 1 ---\r\r\r\r\r\r\r\r\r\r\r\r\r\r\r\r\r\r\r\r\r\r\r\r\r\r\r\r\r\r\r\r\r\r\r\r\r\r\r\r\r\r\r\r\r", "ExpectedValue"=""}, {"Test_Name"="215. SetG15PullDown \"A\" \"4\"", "Step_Type"="", "LowLimit"=0.0, "HighLimit"=0.0, "RValue"="", "RStatus"="", "RetVal"="0", "Units"="", "header1"="", "header2"="--- Start Pin Driver test for ASIC 1 ---\r\r\r\r\r\r\r\r\r\r\r\r\r\r\r\r\r\r\r\r\r\r\r\r\r\r\r\r\r\r\r\r\r\r\r\r\r\r\r\r\r\r\r\r\r\r", "ExpectedValue"=""}, {"Test_Name"="216. SetG15PullDown \"B\" \"4\"", "Step_Type"="", "LowLimit"=0.0, "HighLimit"=0.0, "RValue"="", "RStatus"="", "RetVal"="0", "Units"="", "header1"="", "header2"="--- Start Pin Driver test for ASIC 1 ---\r\r\r\r\r\r\r\r\r\r\r\r\r\r\r\r\r\r\r\r\r\r\r\r\r\r\r\r\r\r\r\r\r\r\r\r\r\r\r\r\r\r\r\r\r\r\r", "ExpectedValue"=""}, {"Test_Name"="217. CheckCFAdc \"PD1\" \"3.7\" \"4.2\"", "Step_Type"="NumericLimitTest", "LowLimit"=3.7, "HighLimit"=4.2, "RValue"="3.953000068664551", "RStatus"="PASS", "RetVal"="0", "Units"="Volts", "header1"="", "header2"="--- Start Pin Driver test for ASIC 1 ---\r\r\r\r\r\r\r\r\r\r\r\r\r\r\r\r\r\r\r\r\r\r\r\r\r\r\r\r\r\r\r\r\r\r\r\r\r\r\r\r\r\r\r\r\r\r\r\r", "ExpectedValue"=""}, {"Test_Name"="218. CheckCFAdc \"PD2\" \"3.7\" \"4.2\"", "Step_Type"="NumericLimitTest", "LowLimit"=3.7, "HighLimit"=4.2, "RValue"="3.9679999351501465", "RStatus"="PASS", "RetVal"="0", "Units"="Volts", "header1"="", "header2"="--- Start Pin Driver test for ASIC 1 ---\r\r\r\r\r\r\r\r\r\r\r\r\r\r\r\r\r\r\r\r\r\r\r\r\r\r\r\r\r\r\r\r\r\r\r\r\r\r\r\r\r\r\r\r\r\r\r\r\r", "ExpectedValue"=""}, {"Test_Name"="221. SetG15PullUp \"A\" \"5\"", "Step_Type"="", "LowLimit"=0.0, "HighLimit"=0.0, "RValue"="", "RStatus"="", "RetVal"="0", "Units"="", "header1"="", "header2"="--- Start Pin Driver test for ASIC 1 ---\r\r\r\r\r\r\r\r\r\r\r\r\r\r\r\r\r\r\r\r\r\r\r\r\r\r\r\r\r\r\r\r\r\r\r\r\r\r\r\r\r\r\r\r\r\r\r\r\r\r", "ExpectedValue"=""}, {"Test_Name"="222. SetG15PullUp \"B\" \"5\"", "Step_Type"="", "LowLimit"=0.0, "HighLimit"=0.0, "RValue"="", "RStatus"="", "RetVal"="0", "Units"="", "header1"="", "header2"="--- Start Pin Driver test for ASIC 1 ---\r\r\r\r\r\r\r\r\r\r\r\r\r\r\r\r\r\r\r\r\r\r\r\r\r\r\r\r\r\r\r\r\r\r\r\r\r\r\r\r\r\r\r\r\r\r\r\r\r\r\r", "ExpectedValue"=""}, {"Test_Name"="223. SetG15PullDown \"A\" \"4\"", "Step_Type"="", "LowLimit"=0.0, "HighLimit"=0.0, "RValue"="", "RStatus"="", "RetVal"="0", "Units"="", "header1"="", "header2"="--- Start Pin Driver test for ASIC 1 ---\r\r\r\r\r\r\r\r\r\r\r\r\r\r\r\r\r\r\r\r\r\r\r\r\r\r\r\r\r\r\r\r\r\r\r\r\r\r\r\r\r\r\r\r\r\r\r\r\r\r\r\r", "ExpectedValue"=""}, {"Test_Name"="224. SetG15PullDown \"B\" \"4\"", "Step_Type"="", "LowLimit"=0.0, "HighLimit"=0.0, "RValue"="", "RStatus"="", "RetVal"="0", "Units"="", "header1"="", "header2"="--- Start Pin Driver test for ASIC 1 ---\r\r\r\r\r\r\r\r\r\r\r\r\r\r\r\r\r\r\r\r\r\r\r\r\r\r\r\r\r\r\r\r\r\r\r\r\r\r\r\r\r\r\r\r\r\r\r\r\r\r\r\r\r", "ExpectedValue"=""}, {"Test_Name"="225. CheckCFAdc \"PD1\" \"3.5\" \"4.0\"", "Step_Type"="NumericLimitTest", "LowLimit"=3.5, "HighLimit"=4.0, "RValue"="3.7780001163482666", "RStatus"="PASS", "RetVal"="0", "Units"="Volts", "header1"="", "header2"="--- Start Pin Driver test for ASIC 1 ---\r\r\r\r\r\r\r\r\r\r\r\r\r\r\r\r\r\r\r\r\r\r\r\r\r\r\r\r\r\r\r\r\r\r\r\r\r\r\r\r\r\r\r\r\r\r\r\r\r\r\r\r\r\r", "ExpectedValue"=""}, {"Test_Name"="226. CheckCFAdc \"PD2\" \"3.5\" \"4.0\"", "Step_Type"="NumericLimitTest", "LowLimit"=3.5, "HighLimit"=4.0, "RValue"="3.802000045776367", "RStatus"="PASS", "RetVal"="0", "Units"="Volts", "header1"="", "header2"="--- Start Pin Driver test for ASIC 1 ---\r\r\r\r\r\r\r\r\r\r\r\r\r\r\r\r\r\r\r\r\r\r\r\r\r\r\r\r\r\r\r\r\r\r\r\r\r\r\r\r\r\r\r\r\r\r\r\r\r\r\r\r\r\r\r", "ExpectedValue"=""}, {"Test_Name"="229. SetG15PullUp \"A\" \"6\"", "Step_Type"="", "LowLimit"=0.0, "HighLimit"=0.0, "RValue"="", "RStatus"="", "RetVal"="0", "Units"="", "header1"="", "header2"="--- Start Pin Driver test for ASIC 1 ---\r\r\r\r\r\r\r\r\r\r\r\r\r\r\r\r\r\r\r\r\r\r\r\r\r\r\r\r\r\r\r\r\r\r\r\r\r\r\r\r\r\r\r\r\r\r\r\r\r\r\r\r\r\r\r\r", "ExpectedValue"=""}, {"Test_Name"="230. SetG15PullUp \"B\" \"6\"", "Step_Type"="", "LowLimit"=0.0, "HighLimit"=0.0, "RValue"="", "RStatus"="", "RetVal"="0", "Units"="", "header1"="", "header2"="--- Start Pin Driver test for ASIC 1 ---\r\r\r\r\r\r\r\r\r\r\r\r\r\r\r\r\r\r\r\r\r\r\r\r\r\r\r\r\r\r\r\r\r\r\r\r\r\r\r\r\r\r\r\r\r\r\r\r\r\r\r\r\r\r\r\r\r", "ExpectedValue"=""}, {"Test_Name"="231. SetG15PullDown \"A\" \"4\"", "Step_Type"="", "LowLimit"=0.0, "HighLimit"=0.0, "RValue"="", "RStatus"="", "RetVal"="0", "Units"="", "header1"="", "header2"="--- Start Pin Driver test for ASIC 1 ---\r\r\r\r\r\r\r\r\r\r\r\r\r\r\r\r\r\r\r\r\r\r\r\r\r\r\r\r\r\r\r\r\r\r\r\r\r\r\r\r\r\r\r\r\r\r\r\r\r\r\r\r\r\r\r\r\r\r", "ExpectedValue"=""}, {"Test_Name"="232. SetG15PullDown \"B\" \"4\"", "Step_Type"="", "LowLimit"=0.0, "HighLimit"=0.0, "RValue"="", "RStatus"="", "RetVal"="0", "Units"="", "header1"="", "header2"="--- Start Pin Driver test for ASIC 1 ---\r\r\r\r\r\r\r\r\r\r\r\r\r\r\r\r\r\r\r\r\r\r\r\r\r\r\r\r\r\r\r\r\r\r\r\r\r\r\r\r\r\r\r\r\r\r\r\r\r\r\r\r\r\r\r\r\r\r\r", "ExpectedValue"=""}, {"Test_Name"="233. CheckCFAdc \"PD1\" \"3.4\" \"3.9\"", "Step_Type"="NumericLimitTest", "LowLimit"=3.4, "HighLimit"=3.9, "RValue"="3.6579999923706055", "RStatus"="PASS", "RetVal"="0", "Units"="Volts", "header1"="", "header2"="--- Start Pin Driver test for ASIC 1 ---\r\r\r\r\r\r\r\r\r\r\r\r\r\r\r\r\r\r\r\r\r\r\r\r\r\r\r\r\r\r\r\r\r\r\r\r\r\r\r\r\r\r\r\r\r\r\r\r\r\r\r\r\r\r\r\r\r\r\r\r", "ExpectedValue"=""}, {"Test_Name"="234. CheckCFAdc \"PD2\" \"3.4\" \"3.9\"", "Step_Type"="NumericLimitTest", "LowLimit"=3.4, "HighLimit"=3.9, "RValue"="3.6730000972747803", "RStatus"="PASS", "RetVal"="0", "Units"="Volts", "header1"="", "header2"="--- Start Pin Driver test for ASIC 1 ---\r\r\r\r\r\r\r\r\r\r\r\r\r\r\r\r\r\r\r\r\r\r\r\r\r\r\r\r\r\r\r\r\r\r\r\r\r\r\r\r\r\r\r\r\r\r\r\r\r\r\r\r\r\r\r\r\r\r\r\r\r", "ExpectedValue"=""}, {"Test_Name"="237. SetG15PullUp \"A\" \"7\"", "Step_Type"="", "LowLimit"=0.0, "HighLimit"=0.0, "RValue"="", "RStatus"="", "RetVal"="0", "Units"="", "header1"="", "header2"="--- Start Pin Driver test for ASIC 1 ---\r\r\r\r\r\r\r\r\r\r\r\r\r\r\r\r\r\r\r\r\r\r\r\r\r\r\r\r\r\r\r\r\r\r\r\r\r\r\r\r\r\r\r\r\r\r\r\r\r\r\r\r\r\r\r\r\r\r\r\r\r\r", "ExpectedValue"=""}, {"Test_Name"="238. SetG15PullUp \"B\" \"7\"", "Step_Type"="", "LowLimit"=0.0, "HighLimit"=0.0, "RValue"="", "RStatus"="", "RetVal"="0", "Units"="", "header1"="", "header2"="--- Start Pin Driver test for ASIC 1 ---\r\r\r\r\r\r\r\r\r\r\r\r\r\r\r\r\r\r\r\r\r\r\r\r\r\r\r\r\r\r\r\r\r\r\r\r\r\r\r\r\r\r\r\r\r\r\r\r\r\r\r\r\r\r\r\r\r\r\r\r\r\r\r", "ExpectedValue"=""}, {"Test_Name"="239. SetG15PullDown \"A\" \"4\"", "Step_Type"="", "LowLimit"=0.0, "HighLimit"=0.0, "RValue"="", "RStatus"="", "RetVal"="0", "Units"="", "header1"="", "header2"="--- Start Pin Driver test for ASIC 1 ---\r\r\r\r\r\r\r\r\r\r\r\r\r\r\r\r\r\r\r\r\r\r\r\r\r\r\r\r\r\r\r\r\r\r\r\r\r\r\r\r\r\r\r\r\r\r\r\r\r\r\r\r\r\r\r\r\r\r\r\r\r\r\r\r", "ExpectedValue"=""}, {"Test_Name"="240. SetG15PullDown \"B\" \"4\"", "Step_Type"="", "LowLimit"=0.0, "HighLimit"=0.0, "RValue"="", "RStatus"="", "RetVal"="0", "Units"="", "header1"="", "header2"="--- Start Pin Driver test for ASIC 1 ---\r\r\r\r\r\r\r\r\r\r\r\r\r\r\r\r\r\r\r\r\r\r\r\r\r\r\r\r\r\r\r\r\r\r\r\r\r\r\r\r\r\r\r\r\r\r\r\r\r\r\r\r\r\r\r\r\r\r\r\r\r\r\r\r\r", "ExpectedValue"=""}, {"Test_Name"="241. CheckCFAdc \"PD1\" \"3.25\" \"3.7\"", "Step_Type"="NumericLimitTest", "LowLimit"=3.25, "HighLimit"=3.7, "RValue"="3.4730000495910645", "RStatus"="PASS", "RetVal"="0", "Units"="Volts", "header1"="", "header2"="--- Start Pin Driver test for ASIC 1 ---\r\r\r\r\r\r\r\r\r\r\r\r\r\r\r\r\r\r\r\r\r\r\r\r\r\r\r\r\r\r\r\r\r\r\r\r\r\r\r\r\r\r\r\r\r\r\r\r\r\r\r\r\r\r\r\r\r\r\r\r\r\r\r\r\r\r", "ExpectedValue"=""}, {"Test_Name"="242. CheckCFAdc \"PD2\" \"3.25\" \"3.7\"", "Step_Type"="NumericLimitTest", "LowLimit"=3.25, "HighLimit"=3.7, "RValue"="3.48799991607666", "RStatus"="PASS", "RetVal"="0", "Units"="Volts", "header1"="", "header2"="--- Start Pin Driver test for ASIC 1 ---\r\r\r\r\r\r\r\r\r\r\r\r\r\r\r\r\r\r\r\r\r\r\r\r\r\r\r\r\r\r\r\r\r\r\r\r\r\r\r\r\r\r\r\r\r\r\r\r\r\r\r\r\r\r\r\r\r\r\r\r\r\r\r\r\r\r\r", "ExpectedValue"=""}, {"Test_Name"="245. SetG15PullUp \"A\" \"8\"", "Step_Type"="", "LowLimit"=0.0, "HighLimit"=0.0, "RValue"="", "RStatus"="", "RetVal"="0", "Units"="", "header1"="", "header2"="--- Start Pin Driver test for ASIC 1 ---\r\r\r\r\r\r\r\r\r\r\r\r\r\r\r\r\r\r\r\r\r\r\r\r\r\r\r\r\r\r\r\r\r\r\r\r\r\r\r\r\r\r\r\r\r\r\r\r\r\r\r\r\r\r\r\r\r\r\r\r\r\r\r\r\r\r\r\r", "ExpectedValue"=""}, {"Test_Name"="246. SetG15PullUp \"B\" \"8\"", "Step_Type"="", "LowLimit"=0.0, "HighLimit"=0.0, "RValue"="", "RStatus"="", "RetVal"="0", "Units"="", "header1"="", "header2"="--- Start Pin Driver test for ASIC 1 ---\r\r\r\r\r\r\r\r\r\r\r\r\r\r\r\r\r\r\r\r\r\r\r\r\r\r\r\r\r\r\r\r\r\r\r\r\r\r\r\r\r\r\r\r\r\r\r\r\r\r\r\r\r\r\r\r\r\r\r\r\r\r\r\r\r\r\r\r\r", "ExpectedValue"=""}, {"Test_Name"="247. SetG15PullDown \"A\" \"4\"", "Step_Type"="", "LowLimit"=0.0, "HighLimit"=0.0, "RValue"="", "RStatus"="", "RetVal"="0", "Units"="", "header1"="", "header2"="--- Start Pin Driver test for ASIC 1 ---\r\r\r\r\r\r\r\r\r\r\r\r\r\r\r\r\r\r\r\r\r\r\r\r\r\r\r\r\r\r\r\r\r\r\r\r\r\r\r\r\r\r\r\r\r\r\r\r\r\r\r\r\r\r\r\r\r\r\r\r\r\r\r\r\r\r\r\r\r\r", "ExpectedValue"=""}, {"Test_Name"="248. SetG15PullDown \"B\" \"4\"", "Step_Type"="", "LowLimit"=0.0, "HighLimit"=0.0, "RValue"="", "RStatus"="", "RetVal"="0", "Units"="", "header1"="", "header2"="--- Start Pin Driver test for ASIC 1 ---\r\r\r\r\r\r\r\r\r\r\r\r\r\r\r\r\r\r\r\r\r\r\r\r\r\r\r\r\r\r\r\r\r\r\r\r\r\r\r\r\r\r\r\r\r\r\r\r\r\r\r\r\r\r\r\r\r\r\r\r\r\r\r\r\r\r\r\r\r\r\r", "ExpectedValue"=""}, {"Test_Name"="249. CheckCFAdc \"PD1\" \"3.1\" \"3.5\"", "Step_Type"="NumericLimitTest", "LowLimit"=3.1, "HighLimit"=3.5, "RValue"="3.306999921798706", "RStatus"="PASS", "RetVal"="0", "Units"="Volts", "header1"="", "header2"="--- Start Pin Driver test for ASIC 1 ---\r\r\r\r\r\r\r\r\r\r\r\r\r\r\r\r\r\r\r\r\r\r\r\r\r\r\r\r\r\r\r\r\r\r\r\r\r\r\r\r\r\r\r\r\r\r\r\r\r\r\r\r\r\r\r\r\r\r\r\r\r\r\r\r\r\r\r\r\r\r\r\r", "ExpectedValue"=""}, {"Test_Name"="250. CheckCFAdc \"PD2\" \"3.1\" \"3.5\"", "Step_Type"="NumericLimitTest", "LowLimit"=3.1, "HighLimit"=3.5, "RValue"="3.322000026702881", "RStatus"="PASS", "RetVal"="0", "Units"="Volts", "header1"="", "header2"="--- Start Pin Driver test for ASIC 1 ---\r\r\r\r\r\r\r\r\r\r\r\r\r\r\r\r\r\r\r\r\r\r\r\r\r\r\r\r\r\r\r\r\r\r\r\r\r\r\r\r\r\r\r\r\r\r\r\r\r\r\r\r\r\r\r\r\r\r\r\r\r\r\r\r\r\r\r\r\r\r\r\r\r", "ExpectedValue"=""}, {"Test_Name"="253. SetG15PullUp \"A\" \"9\"", "Step_Type"="", "LowLimit"=0.0, "HighLimit"=0.0, "RValue"="", "RStatus"="", "RetVal"="0", "Units"="", "header1"="", "header2"="--- Start Pin Driver test for ASIC 1 ---\r\r\r\r\r\r\r\r\r\r\r\r\r\r\r\r\r\r\r\r\r\r\r\r\r\r\r\r\r\r\r\r\r\r\r\r\r\r\r\r\r\r\r\r\r\r\r\r\r\r\r\r\r\r\r\r\r\r\r\r\r\r\r\r\r\r\r\r\r\r\r\r\r\r", "ExpectedValue"=""}, {"Test_Name"="254. SetG15PullUp \"B\" \"9\"", "Step_Type"="", "LowLimit"=0.0, "HighLimit"=0.0, "RValue"="", "RStatus"="", "RetVal"="0", "Units"="", "header1"="", "header2"="--- Start Pin Driver test for ASIC 1 ---\r\r\r\r\r\r\r\r\r\r\r\r\r\r\r\r\r\r\r\r\r\r\r\r\r\r\r\r\r\r\r\r\r\r\r\r\r\r\r\r\r\r\r\r\r\r\r\r\r\r\r\r\r\r\r\r\r\r\r\r\r\r\r\r\r\r\r\r\r\r\r\r\r\r\r", "ExpectedValue"=""}, {"Test_Name"="255. SetG15PullDown \"A\" \"4\"", "Step_Type"="", "LowLimit"=0.0, "HighLimit"=0.0, "RValue"="", "RStatus"="", "RetVal"="0", "Units"="", "header1"="", "header2"="--- Start Pin Driver test for ASIC 1 ---\r\r\r\r\r\r\r\r\r\r\r\r\r\r\r\r\r\r\r\r\r\r\r\r\r\r\r\r\r\r\r\r\r\r\r\r\r\r\r\r\r\r\r\r\r\r\r\r\r\r\r\r\r\r\r\r\r\r\r\r\r\r\r\r\r\r\r\r\r\r\r\r\r\r\r\r", "ExpectedValue"=""}, {"Test_Name"="256. SetG15PullDown \"B\" \"4\"", "Step_Type"="", "LowLimit"=0.0, "HighLimit"=0.0, "RValue"="", "RStatus"="", "RetVal"="0", "Units"="", "header1"="", "header2"="--- Start Pin Driver test for ASIC 1 ---\r\r\r\r\r\r\r\r\r\r\r\r\r\r\r\r\r\r\r\r\r\r\r\r\r\r\r\r\r\r\r\r\r\r\r\r\r\r\r\r\r\r\r\r\r\r\r\r\r\r\r\r\r\r\r\r\r\r\r\r\r\r\r\r\r\r\r\r\r\r\r\r\r\r\r\r\r", "ExpectedValue"=""}, {"Test_Name"="257. CheckCFAdc \"PD1\" \"2.25\" \"2.65\"", "Step_Type"="NumericLimitTest", "LowLimit"=2.25, "HighLimit"=2.65, "RValue"="2.437999963760376", "RStatus"="PASS", "RetVal"="0", "Units"="Volts", "header1"="", "header2"="--- Start Pin Driver test for ASIC 1 ---\r\r\r\r\r\r\r\r\r\r\r\r\r\r\r\r\r\r\r\r\r\r\r\r\r\r\r\r\r\r\r\r\r\r\r\r\r\r\r\r\r\r\r\r\r\r\r\r\r\r\r\r\r\r\r\r\r\r\r\r\r\r\r\r\r\r\r\r\r\r\r\r\r\r\r\r\r\r", "ExpectedValue"=""}, {"Test_Name"="258. CheckCFAdc \"PD2\" \"2.25\" \"2.65\"", "Step_Type"="NumericLimitTest", "LowLimit"=2.25, "HighLimit"=2.65, "RValue"="2.4549999237060547", "RStatus"="PASS", "RetVal"="0", "Units"="Volts", "header1"="", "header2"="--- Start Pin Driver test for ASIC 1 ---\r\r\r\r\r\r\r\r\r\r\r\r\r\r\r\r\r\r\r\r\r\r\r\r\r\r\r\r\r\r\r\r\r\r\r\r\r\r\r\r\r\r\r\r\r\r\r\r\r\r\r\r\r\r\r\r\r\r\r\r\r\r\r\r\r\r\r\r\r\r\r\r\r\r\r\r\r\r\r", "ExpectedValue"=""}, {"Test_Name"="261. SetG15PullUp \"A\" \"2\"", "Step_Type"="", "LowLimit"=0.0, "HighLimit"=0.0, "RValue"="", "RStatus"="", "RetVal"="0", "Units"="", "header1"="", "header2"="--- Start Pin Driver test for ASIC 1 ---\r\r\r\r\r\r\r\r\r\r\r\r\r\r\r\r\r\r\r\r\r\r\r\r\r\r\r\r\r\r\r\r\r\r\r\r\r\r\r\r\r\r\r\r\r\r\r\r\r\r\r\r\r\r\r\r\r\r\r\r\r\r\r\r\r\r\r\r\r\r\r\r\r\r\r\r\r\r\r\r", "ExpectedValue"=""}, {"Test_Name"="262. SetG15PullUp \"B\" \"2\"", "Step_Type"="", "LowLimit"=0.0, "HighLimit"=0.0, "RValue"="", "RStatus"="", "RetVal"="0", "Units"="", "header1"="", "header2"="--- Start Pin Driver test for ASIC 1 ---\r\r\r\r\r\r\r\r\r\r\r\r\r\r\r\r\r\r\r\r\r\r\r\r\r\r\r\r\r\r\r\r\r\r\r\r\r\r\r\r\r\r\r\r\r\r\r\r\r\r\r\r\r\r\r\r\r\r\r\r\r\r\r\r\r\r\r\r\r\r\r\r\r\r\r\r\r\r\r\r\r", "ExpectedValue"=""}, {"Test_Name"="263. SetG15PullDown \"A\" \"0\"", "Step_Type"="", "LowLimit"=0.0, "HighLimit"=0.0, "RValue"="", "RStatus"="", "RetVal"="0", "Units"="", "header1"="", "header2"="--- Start Pin Driver test for ASIC 1 ---\r\r\r\r\r\r\r\r\r\r\r\r\r\r\r\r\r\r\r\r\r\r\r\r\r\r\r\r\r\r\r\r\r\r\r\r\r\r\r\r\r\r\r\r\r\r\r\r\r\r\r\r\r\r\r\r\r\r\r\r\r\r\r\r\r\r\r\r\r\r\r\r\r\r\r\r\r\r\r\r\r\r", "ExpectedValue"=""}, {"Test_Name"="264. SetG15PullDown \"B\" \"0\"", "Step_Type"="", "LowLimit"=0.0, "HighLimit"=0.0, "RValue"="", "RStatus"="", "RetVal"="0", "Units"="", "header1"="", "header2"="--- Start Pin Driver test for ASIC 1 ---\r\r\r\r\r\r\r\r\r\r\r\r\r\r\r\r\r\r\r\r\r\r\r\r\r\r\r\r\r\r\r\r\r\r\r\r\r\r\r\r\r\r\r\r\r\r\r\r\r\r\r\r\r\r\r\r\r\r\r\r\r\r\r\r\r\r\r\r\r\r\r\r\r\r\r\r\r\r\r\r\r\r\r", "ExpectedValue"=""}, {"Test_Name"="265. CheckCFAdc \"PD1\" \"4.55\" \"5.0\"", "Step_Type"="NumericLimitTest", "LowLimit"=4.55, "HighLimit"=5.0, "RValue"="4.811999797821045", "RStatus"="PASS", "RetVal"="0", "Units"="Volts", "header1"="", "header2"="--- Start Pin Driver test for ASIC 1 ---\r\r\r\r\r\r\r\r\r\r\r\r\r\r\r\r\r\r\r\r\r\r\r\r\r\r\r\r\r\r\r\r\r\r\r\r\r\r\r\r\r\r\r\r\r\r\r\r\r\r\r\r\r\r\r\r\r\r\r\r\r\r\r\r\r\r\r\r\r\r\r\r\r\r\r\r\r\r\r\r\r\r\r\r", "ExpectedValue"=""}, {"Test_Name"="266. CheckCFAdc \"PD2\" \"4.55\" \"5.0\"", "Step_Type"="NumericLimitTest", "LowLimit"=4.55, "HighLimit"=5.0, "RValue"="4.816999912261963", "RStatus"="PASS", "RetVal"="0", "Units"="Volts", "header1"="", "header2"="--- Start Pin Driver test for ASIC 1 ---\r\r\r\r\r\r\r\r\r\r\r\r\r\r\r\r\r\r\r\r\r\r\r\r\r\r\r\r\r\r\r\r\r\r\r\r\r\r\r\r\r\r\r\r\r\r\r\r\r\r\r\r\r\r\r\r\r\r\r\r\r\r\r\r\r\r\r\r\r\r\r\r\r\r\r\r\r\r\r\r\r\r\r\r\r", "ExpectedValue"=""}, {"Test_Name"="269. SetG15PullUp \"A\" \"2\"", "Step_Type"="", "LowLimit"=0.0, "HighLimit"=0.0, "RValue"="", "RStatus"="", "RetVal"="0", "Units"="", "header1"="", "header2"="--- Start Pin Driver test for ASIC 1 ---\r\r\r\r\r\r\r\r\r\r\r\r\r\r\r\r\r\r\r\r\r\r\r\r\r\r\r\r\r\r\r\r\r\r\r\r\r\r\r\r\r\r\r\r\r\r\r\r\r\r\r\r\r\r\r\r\r\r\r\r\r\r\r\r\r\r\r\r\r\r\r\r\r\r\r\r\r\r\r\r\r\r\r\r\r\r", "ExpectedValue"=""}, {"Test_Name"="270. SetG15PullUp \"B\" \"2\"", "Step_Type"="", "LowLimit"=0.0, "HighLimit"=0.0, "RValue"="", "RStatus"="", "RetVal"="0", "Units"="", "header1"="", "header2"="--- Start Pin Driver test for ASIC 1 ---\r\r\r\r\r\r\r\r\r\r\r\r\r\r\r\r\r\r\r\r\r\r\r\r\r\r\r\r\r\r\r\r\r\r\r\r\r\r\r\r\r\r\r\r\r\r\r\r\r\r\r\r\r\r\r\r\r\r\r\r\r\r\r\r\r\r\r\r\r\r\r\r\r\r\r\r\r\r\r\r\r\r\r\r\r\r\r", "ExpectedValue"=""}, {"Test_Name"="271. SetG15PullDown \"A\" \"5\"", "Step_Type"="", "LowLimit"=0.0, "HighLimit"=0.0, "RValue"="", "RStatus"="", "RetVal"="0", "Units"="", "header1"="", "header2"="--- Start Pin Driver test for ASIC 1 ---\r\r\r\r\r\r\r\r\r\r\r\r\r\r\r\r\r\r\r\r\r\r\r\r\r\r\r\r\r\r\r\r\r\r\r\r\r\r\r\r\r\r\r\r\r\r\r\r\r\r\r\r\r\r\r\r\r\r\r\r\r\r\r\r\r\r\r\r\r\r\r\r\r\r\r\r\r\r\r\r\r\r\r\r\r\r\r\r", "ExpectedValue"=""}, {"Test_Name"="272. SetG15PullDown \"B\" \"5\"", "Step_Type"="", "LowLimit"=0.0, "HighLimit"=0.0, "RValue"="", "RStatus"="", "RetVal"="0", "Units"="", "header1"="", "header2"="--- Start Pin Driver test for ASIC 1 ---\r\r\r\r\r\r\r\r\r\r\r\r\r\r\r\r\r\r\r\r\r\r\r\r\r\r\r\r\r\r\r\r\r\r\r\r\r\r\r\r\r\r\r\r\r\r\r\r\r\r\r\r\r\r\r\r\r\r\r\r\r\r\r\r\r\r\r\r\r\r\r\r\r\r\r\r\r\r\r\r\r\r\r\r\r\r\r\r\r", "ExpectedValue"=""}, {"Test_Name"="273. CheckCFAdc \"PD1\" \"-.15\" \".3\"", "Step_Type"="NumericLimitTest", "LowLimit"=-0.15, "HighLimit"=0.3, "RValue"="0.017999999225139618", "RStatus"="PASS", "RetVal"="0", "Units"="Volts", "header1"="", "header2"="--- Start Pin Driver test for ASIC 1 ---\r\r\r\r\r\r\r\r\r\r\r\r\r\r\r\r\r\r\r\r\r\r\r\r\r\r\r\r\r\r\r\r\r\r\r\r\r\r\r\r\r\r\r\r\r\r\r\r\r\r\r\r\r\r\r\r\r\r\r\r\r\r\r\r\r\r\r\r\r\r\r\r\r\r\r\r\r\r\r\r\r\r\r\r\r\r\r\r\r\r", "ExpectedValue"=""}, {"Test_Name"="274. CheckCFAdc \"PD2\" \"-.15\" \".3\"", "Step_Type"="NumericLimitTest", "LowLimit"=-0.15, "HighLimit"=0.3, "RValue"="0.017999999225139618", "RStatus"="PASS", "RetVal"="0", "Units"="Volts", "header1"="", "header2"="--- Start Pin Driver test for ASIC 1 ---\r\r\r\r\r\r\r\r\r\r\r\r\r\r\r\r\r\r\r\r\r\r\r\r\r\r\r\r\r\r\r\r\r\r\r\r\r\r\r\r\r\r\r\r\r\r\r\r\r\r\r\r\r\r\r\r\r\r\r\r\r\r\r\r\r\r\r\r\r\r\r\r\r\r\r\r\r\r\r\r\r\r\r\r\r\r\r\r\r\r\r", "ExpectedValue"=""}, {"Test_Name"="276. SetG15PullUp \"A\" \"0\"", "Step_Type"="", "LowLimit"=0.0, "HighLimit"=0.0, "RValue"="", "RStatus"="", "RetVal"="0", "Units"="", "header1"="", "header2"="--- Start Pin Driver test for ASIC 1 ---\r\r\r\r\r\r\r\r\r\r\r\r\r\r\r\r\r\r\r\r\r\r\r\r\r\r\r\r\r\r\r\r\r\r\r\r\r\r\r\r\r\r\r\r\r\r\r\r\r\r\r\r\r\r\r\r\r\r\r\r\r\r\r\r\r\r\r\r\r\r\r\r\r\r\r\r\r\r\r\r\r\r\r\r\r\r\r\r\r\r\r\r", "ExpectedValue"=""}, {"Test_Name"="277. SetG15PullUp \"B\" \"0\"", "Step_Type"="", "LowLimit"=0.0, "HighLimit"=0.0, "RValue"="", "RStatus"="", "RetVal"="0", "Units"="", "header1"="", "header2"="--- Start Pin Driver test for ASIC 1 ---\r\r\r\r\r\r\r\r\r\r\r\r\r\r\r\r\r\r\r\r\r\r\r\r\r\r\r\r\r\r\r\r\r\r\r\r\r\r\r\r\r\r\r\r\r\r\r\r\r\r\r\r\r\r\r\r\r\r\r\r\r\r\r\r\r\r\r\r\r\r\r\r\r\r\r\r\r\r\r\r\r\r\r\r\r\r\r\r\r\r\r\r\r", "ExpectedValue"=""}, {"Test_Name"="278. SetG15PullDown \"A\" \"0\"", "Step_Type"="", "LowLimit"=0.0, "HighLimit"=0.0, "RValue"="", "RStatus"="", "RetVal"="0", "Units"="", "header1"="", "header2"="--- Start Pin Driver test for ASIC 1 ---\r\r\r\r\r\r\r\r\r\r\r\r\r\r\r\r\r\r\r\r\r\r\r\r\r\r\r\r\r\r\r\r\r\r\r\r\r\r\r\r\r\r\r\r\r\r\r\r\r\r\r\r\r\r\r\r\r\r\r\r\r\r\r\r\r\r\r\r\r\r\r\r\r\r\r\r\r\r\r\r\r\r\r\r\r\r\r\r\r\r\r\r\r\r", "ExpectedValue"=""}, {"Test_Name"="279. SetG15PullDown \"B\" \"0\"", "Step_Type"="", "LowLimit"=0.0, "HighLimit"=0.0, "RValue"="", "RStatus"="", "RetVal"="0", "Units"="", "header1"="", "header2"="--- Start Pin Driver test for ASIC 1 ---\r\r\r\r\r\r\r\r\r\r\r\r\r\r\r\r\r\r\r\r\r\r\r\r\r\r\r\r\r\r\r\r\r\r\r\r\r\r\r\r\r\r\r\r\r\r\r\r\r\r\r\r\r\r\r\r\r\r\r\r\r\r\r\r\r\r\r\r\r\r\r\r\r\r\r\r\r\r\r\r\r\r\r\r\r\r\r\r\r\r\r\r\r\r\r", "ExpectedValue"=""}, {"Test_Name"="280. SelectAllPins \"0\"", "Step_Type"="", "LowLimit"=0.0, "HighLimit"=0.0, "RValue"="", "RStatus"="", "RetVal"="0", "Units"="", "header1"="", "header2"="--- Start Pin Driver test for ASIC 1 ---\r\r\r\r\r\r\r\r\r\r\r\r\r\r\r\r\r\r\r\r\r\r\r\r\r\r\r\r\r\r\r\r\r\r\r\r\r\r\r\r\r\r\r\r\r\r\r\r\r\r\r\r\r\r\r\r\r\r\r\r\r\r\r\r\r\r\r\r\r\r\r\r\r\r\r\r\r\r\r\r\r\r\r\r\r\r\r\r\r\r\r\r\r\r\r\r", "ExpectedValue"=""}, {"Test_Name"="282.  --- special test for pins 9, 7, and 15 ---", "Step_Type"="", "LowLimit"=0.0, "HighLimit"=0.0, "RValue"="", "RStatus"="", "RetVal"="", "Units"="", "header1"="", "header2"="--- special test for pins 9, 7, and 15 ---\r", "ExpectedValue"=""}, {"Test_Name"="286. SelectAllMuxA \"1\" \"0\"", "Step_Type"="", "LowLimit"=0.0, "HighLimit"=0.0, "RValue"="", "RStatus"="", "RetVal"="0", "Units"="", "header1"="", "header2"="--- special test for pins 9, 7, and 15 ---\r\r", "ExpectedValue"=""}, {"Test_Name"="287. SelectAllMuxB \"1\" \"0\"", "Step_Type"="", "LowLimit"=0.0, "HighLimit"=0.0, "RValue"="", "RStatus"="", "RetVal"="0", "Units"="", "header1"="", "header2"="--- special test for pins 9, 7, and 15 ---\r\r\r", "ExpectedValue"=""}, {"Test_Name"="290. SetG15PullUp \"A\" \"1\"", "Step_Type"="", "LowLimit"=0.0, "HighLimit"=0.0, "RValue"="", "RStatus"="", "RetVal"="0", "Units"="", "header1"="", "header2"="--- special test for pins 9, 7, and 15 ---\r\r\r\r", "ExpectedValue"=""}, {"Test_Name"="291. SetG15PullupVbat \"0\" \"1\"", "Step_Type"="", "LowLimit"=0.0, "HighLimit"=0.0, "RValue"="", "RStatus"="", "RetVal"="0", "Units"="", "header1"="", "header2"="--- special test for pins 9, 7, and 15 ---\r\r\r\r\r", "ExpectedValue"=""}, {"Test_Name"="292. CheckCFAdc \"PD1\" \"14\" \"15.5\"", "Step_Type"="NumericLimitTest", "LowLimit"=14.0, "HighLimit"=15.5, "RValue"="14.36400032043457", "RStatus"="PASS", "RetVal"="0", "Units"="Volts", "header1"="", "header2"="--- special test for pins 9, 7, and 15 ---\r\r\r\r\r\r", "ExpectedValue"=""}, {"Test_Name"="294. SelectMuxA \"1\" \"9\" \"1\"", "Step_Type"="", "LowLimit"=0.0, "HighLimit"=0.0, "RValue"="", "RStatus"="", "RetVal"="0", "Units"="", "header1"="", "header2"="--- special test for pins 9, 7, and 15 ---\r\r\r\r\r\r\r", "ExpectedValue"=""}, {"Test_Name"="295. SetFpgaRegister \"89F\" \"01\"", "Step_Type"="", "LowLimit"=0.0, "HighLimit"=0.0, "RValue"="", "RStatus"="", "RetVal"="0", "Units"="", "header1"="", "header2"="--- special test for pins 9, 7, and 15 ---\r\r\r\r\r\r\r\r", "ExpectedValue"=""}, {"Test_Name"="296. CheckCFAdc \"PD1\" \"-.15\" \".3\"", "Step_Type"="NumericLimitTest", "LowLimit"=-0.15, "HighLimit"=0.3, "RValue"="0.23000000417232513", "RStatus"="PASS", "RetVal"="0", "Units"="Volts", "header1"="", "header2"="--- special test for pins 9, 7, and 15 ---\r\r\r\r\r\r\r\r\r", "ExpectedValue"=""}, {"Test_Name"="297. SetFpgaRegister \"89F\" \"00\"", "Step_Type"="", "LowLimit"=0.0, "HighLimit"=0.0, "RValue"="", "RStatus"="", "RetVal"="0", "Units"="", "header1"="", "header2"="--- special test for pins 9, 7, and 15 ---\r\r\r\r\r\r\r\r\r\r", "ExpectedValue"=""}, {"Test_Name"="298. CheckCFAdc \"PD1\" \"14\" \"15.5\"", "Step_Type"="NumericLimitTest", "LowLimit"=14.0, "HighLimit"=15.5, "RValue"="14.36400032043457", "RStatus"="PASS", "RetVal"="0", "Units"="Volts", "header1"="", "header2"="--- special test for pins 9, 7, and 15 ---\r\r\r\r\r\r\r\r\r\r\r", "ExpectedValue"=""}, {"Test_Name"="300. SelectAllMuxA \"1\" \"0\"", "Step_Type"="", "LowLimit"=0.0, "HighLimit"=0.0, "RValue"="", "RStatus"="", "RetVal"="0", "Units"="", "header1"="", "header2"="--- special test for pins 9, 7, and 15 ---\r\r\r\r\r\r\r\r\r\r\r\r", "ExpectedValue"=""}, {"Test_Name"="301. SelectAllMuxB \"1\" \"0\"", "Step_Type"="", "LowLimit"=0.0, "HighLimit"=0.0, "RValue"="", "RStatus"="", "RetVal"="0", "Units"="", "header1"="", "header2"="--- special test for pins 9, 7, and 15 ---\r\r\r\r\r\r\r\r\r\r\r\r\r", "ExpectedValue"=""}, {"Test_Name"="302. SetG15PullUp \"A\" \"0\"", "Step_Type"="", "LowLimit"=0.0, "HighLimit"=0.0, "RValue"="", "RStatus"="", "RetVal"="0", "Units"="", "header1"="", "header2"="--- special test for pins 9, 7, and 15 ---\r\r\r\r\r\r\r\r\r\r\r\r\r\r", "ExpectedValue"=""}, {"Test_Name"="303. SetG15PullUp \"B\" \"0\"", "Step_Type"="", "LowLimit"=0.0, "HighLimit"=0.0, "RValue"="", "RStatus"="", "RetVal"="0", "Units"="", "header1"="", "header2"="--- special test for pins 9, 7, and 15 ---\r\r\r\r\r\r\r\r\r\r\r\r\r\r\r", "ExpectedValue"=""}, {"Test_Name"="304. SetG15PullDown \"A\" \"0\"", "Step_Type"="", "LowLimit"=0.0, "HighLimit"=0.0, "RValue"="", "RStatus"="", "RetVal"="0", "Units"="", "header1"="", "header2"="--- special test for pins 9, 7, and 15 ---\r\r\r\r\r\r\r\r\r\r\r\r\r\r\r\r", "ExpectedValue"=""}, {"Test_Name"="305. SetG15PullDown \"B\" \"0\"", "Step_Type"="", "LowLimit"=0.0, "HighLimit"=0.0, "RValue"="", "RStatus"="", "RetVal"="0", "Units"="", "header1"="", "header2"="--- special test for pins 9, 7, and 15 ---\r\r\r\r\r\r\r\r\r\r\r\r\r\r\r\r\r", "ExpectedValue"=""}, {"Test_Name"="308. SelectMuxA \"1\" \"7\" \"1\"", "Step_Type"="", "LowLimit"=0.0, "HighLimit"=0.0, "RValue"="", "RStatus"="", "RetVal"="0", "Units"="", "header1"="", "header2"="--- special test for pins 9, 7, and 15 ---\r\r\r\r\r\r\r\r\r\r\r\r\r\r\r\r\r\r", "ExpectedValue"=""}, {"Test_Name"="309. SelectMuxB \"1\" \"15\" \"1\"", "Step_Type"="", "LowLimit"=0.0, "HighLimit"=0.0, "RValue"="", "RStatus"="", "RetVal"="0", "Units"="", "header1"="", "header2"="--- special test for pins 9, 7, and 15 ---\r\r\r\r\r\r\r\r\r\r\r\r\r\r\r\r\r\r\r", "ExpectedValue"=""}, {"Test_Name"="310. SetAsicRegister \"1\" \"5\" \"0\"", "Step_Type"="", "LowLimit"=0.0, "HighLimit"=0.0, "RValue"="", "RStatus"="", "RetVal"="0", "Units"="", "header1"="", "header2"="--- special test for pins 9, 7, and 15 ---\r\r\r\r\r\r\r\r\r\r\r\r\r\r\r\r\r\r\r\r", "ExpectedValue"=""}, {"Test_Name"="312. CheckCFAdc \"PD1\" \"-.15\" \"1.2\"", "Step_Type"="NumericLimitTest", "LowLimit"=-0.15, "HighLimit"=1.2, "RValue"="0.6460000276565552", "RStatus"="PASS", "RetVal"="0", "Units"="Volts", "header1"="", "header2"="--- special test for pins 9, 7, and 15 ---\r\r\r\r\r\r\r\r\r\r\r\r\r\r\r\r\r\r\r\r\r", "ExpectedValue"=""}, {"Test_Name"="313. SetAsicRegister \"1\" \"5\" \"40\"", "Step_Type"="", "LowLimit"=0.0, "HighLimit"=0.0, "RValue"="", "RStatus"="", "RetVal"="0", "Units"="", "header1"="", "header2"="--- special test for pins 9, 7, and 15 ---\r\r\r\r\r\r\r\r\r\r\r\r\r\r\r\r\r\r\r\r\r\r", "ExpectedValue"=""}, {"Test_Name"="314. SetG15PullDown \"A\" \"3\"", "Step_Type"="", "LowLimit"=0.0, "HighLimit"=0.0, "RValue"="", "RStatus"="", "RetVal"="0", "Units"="", "header1"="", "header2"="--- special test for pins 9, 7, and 15 ---\r\r\r\r\r\r\r\r\r\r\r\r\r\r\r\r\r\r\r\r\r\r\r", "ExpectedValue"=""}, {"Test_Name"="315. CheckCFAdc \"PD1\" \"12.5\" \"13.5\"", "Step_Type"="NumericLimitTest", "LowLimit"=12.5, "HighLimit"=13.5, "RValue"="12.88599967956543", "RStatus"="PASS", "RetVal"="0", "Units"="Volts", "header1"="", "header2"="--- special test for pins 9, 7, and 15 ---\r\r\r\r\r\r\r\r\r\r\r\r\r\r\r\r\r\r\r\r\r\r\r\r", "ExpectedValue"=""}, {"Test_Name"="316. SetAsicRegister \"1\" \"5\" \"80\"", "Step_Type"="", "LowLimit"=0.0, "HighLimit"=0.0, "RValue"="", "RStatus"="", "RetVal"="0", "Units"="", "header1"="", "header2"="--- special test for pins 9, 7, and 15 ---\r\r\r\r\r\r\r\r\r\r\r\r\r\r\r\r\r\r\r\r\r\r\r\r\r", "ExpectedValue"=""}, {"Test_Name"="317. CheckCFAdc \"PD1\" \"11\" \"12.2\"", "Step_Type"="NumericLimitTest", "LowLimit"=11.0, "HighLimit"=12.2, "RValue"="11.583999633789062", "RStatus"="PASS", "RetVal"="0", "Units"="Volts", "header1"="", "header2"="--- special test for pins 9, 7, and 15 ---\r\r\r\r\r\r\r\r\r\r\r\r\r\r\r\r\r\r\r\r\r\r\r\r\r\r", "ExpectedValue"=""}, {"Test_Name"="318. SetG15PullDown \"A\" \"0\"", "Step_Type"="", "LowLimit"=0.0, "HighLimit"=0.0, "RValue"="", "RStatus"="", "RetVal"="0", "Units"="", "header1"="", "header2"="--- special test for pins 9, 7, and 15 ---\r\r\r\r\r\r\r\r\r\r\r\r\r\r\r\r\r\r\r\r\r\r\r\r\r\r\r", "ExpectedValue"=""}, {"Test_Name"="319. SetG15PullUp \"A\" \"0\"", "Step_Type"="", "LowLimit"=0.0, "HighLimit"=0.0, "RValue"="", "RStatus"="", "RetVal"="0", "Units"="", "header1"="", "header2"="--- special test for pins 9, 7, and 15 ---\r\r\r\r\r\r\r\r\r\r\r\r\r\r\r\r\r\r\r\r\r\r\r\r\r\r\r\r", "ExpectedValue"=""}, {"Test_Name"="321. CheckCFAdc \"PD2\" \"-.15\" \"1.4\"", "Step_Type"="NumericLimitTest", "LowLimit"=-0.15, "HighLimit"=1.4, "RValue"="0.968999981880188", "RStatus"="PASS", "RetVal"="0", "Units"="Volts", "header1"="", "header2"="--- special test for pins 9, 7, and 15 ---\r\r\r\r\r\r\r\r\r\r\r\r\r\r\r\r\r\r\r\r\r\r\r\r\r\r\r\r\r", "ExpectedValue"=""}, {"Test_Name"="322. SetAsicRegister \"1\" \"5\" \"10\"", "Step_Type"="", "LowLimit"=0.0, "HighLimit"=0.0, "RValue"="", "RStatus"="", "RetVal"="0", "Units"="", "header1"="", "header2"="--- special test for pins 9, 7, and 15 ---\r\r\r\r\r\r\r\r\r\r\r\r\r\r\r\r\r\r\r\r\r\r\r\r\r\r\r\r\r\r", "ExpectedValue"=""}, {"Test_Name"="323. SetG15PullDown \"B\" \"3\"", "Step_Type"="", "LowLimit"=0.0, "HighLimit"=0.0, "RValue"="", "RStatus"="", "RetVal"="0", "Units"="", "header1"="", "header2"="--- special test for pins 9, 7, and 15 ---\r\r\r\r\r\r\r\r\r\r\r\r\r\r\r\r\r\r\r\r\r\r\r\r\r\r\r\r\r\r\r", "ExpectedValue"=""}, {"Test_Name"="324. CheckCFAdc \"PD2\" \"12.3\" \"13.7\"", "Step_Type"="NumericLimitTest", "LowLimit"=12.3, "HighLimit"=13.7, "RValue"="12.892999649047852", "RStatus"="PASS", "RetVal"="0", "Units"="Volts", "header1"="", "header2"="--- special test for pins 9, 7, and 15 ---\r\r\r\r\r\r\r\r\r\r\r\r\r\r\r\r\r\r\r\r\r\r\r\r\r\r\r\r\r\r\r\r", "ExpectedValue"=""}, {"Test_Name"="325. SetAsicRegister \"1\" \"5\" \"20\"", "Step_Type"="", "LowLimit"=0.0, "HighLimit"=0.0, "RValue"="", "RStatus"="", "RetVal"="0", "Units"="", "header1"="", "header2"="--- special test for pins 9, 7, and 15 ---\r\r\r\r\r\r\r\r\r\r\r\r\r\r\r\r\r\r\r\r\r\r\r\r\r\r\r\r\r\r\r\r\r", "ExpectedValue"=""}, {"Test_Name"="326. CheckCFAdc \"PD2\" \"11\" \"12.2\"", "Step_Type"="NumericLimitTest", "LowLimit"=11.0, "HighLimit"=12.2, "RValue"="11.60099983215332", "RStatus"="PASS", "RetVal"="0", "Units"="Volts", "header1"="", "header2"="--- special test for pins 9, 7, and 15 ---\r\r\r\r\r\r\r\r\r\r\r\r\r\r\r\r\r\r\r\r\r\r\r\r\r\r\r\r\r\r\r\r\r\r", "ExpectedValue"=""}, {"Test_Name"="327. SetG15PullDown \"B\" \"0\"", "Step_Type"="", "LowLimit"=0.0, "HighLimit"=0.0, "RValue"="", "RStatus"="", "RetVal"="0", "Units"="", "header1"="", "header2"="--- special test for pins 9, 7, and 15 ---\r\r\r\r\r\r\r\r\r\r\r\r\r\r\r\r\r\r\r\r\r\r\r\r\r\r\r\r\r\r\r\r\r\r\r", "ExpectedValue"=""}, {"Test_Name"="328. CheckCFAdc \"PD2\" \"14\" \"15.5\"", "Step_Type"="NumericLimitTest", "LowLimit"=14.0, "HighLimit"=15.5, "RValue"="14.581999778747559", "RStatus"="PASS", "RetVal"="0", "Units"="Volts", "header1"="", "header2"="--- special test for pins 9, 7, and 15 ---\r\r\r\r\r\r\r\r\r\r\r\r\r\r\r\r\r\r\r\r\r\r\r\r\r\r\r\r\r\r\r\r\r\r\r\r", "ExpectedValue"=""}, {"Test_Name"="329. SetFpgaRegister \"89F\" \"04\"", "Step_Type"="", "LowLimit"=0.0, "HighLimit"=0.0, "RValue"="", "RStatus"="", "RetVal"="0", "Units"="", "header1"="", "header2"="--- special test for pins 9, 7, and 15 ---\r\r\r\r\r\r\r\r\r\r\r\r\r\r\r\r\r\r\r\r\r\r\r\r\r\r\r\r\r\r\r\r\r\r\r\r\r", "ExpectedValue"=""}, {"Test_Name"="330. CheckCFAdc \"PD2\" \"-.15\" \".3\"", "Step_Type"="NumericLimitTest", "LowLimit"=-0.15, "HighLimit"=0.3, "RValue"="0.04600000008940697", "RStatus"="PASS", "RetVal"="0", "Units"="Volts", "header1"="", "header2"="--- special test for pins 9, 7, and 15 ---\r\r\r\r\r\r\r\r\r\r\r\r\r\r\r\r\r\r\r\r\r\r\r\r\r\r\r\r\r\r\r\r\r\r\r\r\r\r", "ExpectedValue"=""}, {"Test_Name"="332. SelectAllMuxA \"1\" \"0\"", "Step_Type"="", "LowLimit"=0.0, "HighLimit"=0.0, "RValue"="", "RStatus"="", "RetVal"="0", "Units"="", "header1"="", "header2"="--- special test for pins 9, 7, and 15 ---\r\r\r\r\r\r\r\r\r\r\r\r\r\r\r\r\r\r\r\r\r\r\r\r\r\r\r\r\r\r\r\r\r\r\r\r\r\r\r", "ExpectedValue"=""}, {"Test_Name"="333. SelectAllMuxB \"1\" \"0\"", "Step_Type"="", "LowLimit"=0.0, "HighLimit"=0.0, "RValue"="", "RStatus"="", "RetVal"="0", "Units"="", "header1"="", "header2"="--- special test for pins 9, 7, and 15 ---\r\r\r\r\r\r\r\r\r\r\r\r\r\r\r\r\r\r\r\r\r\r\r\r\r\r\r\r\r\r\r\r\r\r\r\r\r\r\r\r", "ExpectedValue"=""}, {"Test_Name"="334. SetG15PullUp \"A\" \"0\"", "Step_Type"="", "LowLimit"=0.0, "HighLimit"=0.0, "RValue"="", "RStatus"="", "RetVal"="0", "Units"="", "header1"="", "header2"="--- special test for pins 9, 7, and 15 ---\r\r\r\r\r\r\r\r\r\r\r\r\r\r\r\r\r\r\r\r\r\r\r\r\r\r\r\r\r\r\r\r\r\r\r\r\r\r\r\r\r", "ExpectedValue"=""}, {"Test_Name"="335. SetG15PullUp \"B\" \"0\"", "Step_Type"="", "LowLimit"=0.0, "HighLimit"=0.0, "RValue"="", "RStatus"="", "RetVal"="0", "Units"="", "header1"="", "header2"="--- special test for pins 9, 7, and 15 ---\r\r\r\r\r\r\r\r\r\r\r\r\r\r\r\r\r\r\r\r\r\r\r\r\r\r\r\r\r\r\r\r\r\r\r\r\r\r\r\r\r\r", "ExpectedValue"=""}, {"Test_Name"="336. SetG15PullDown \"A\" \"0\"", "Step_Type"="", "LowLimit"=0.0, "HighLimit"=0.0, "RValue"="", "RStatus"="", "RetVal"="0", "Units"="", "header1"="", "header2"="--- special test for pins 9, 7, and 15 ---\r\r\r\r\r\r\r\r\r\r\r\r\r\r\r\r\r\r\r\r\r\r\r\r\r\r\r\r\r\r\r\r\r\r\r\r\r\r\r\r\r\r\r", "ExpectedValue"=""}, {"Test_Name"="337. SetG15PullDown \"B\" \"0\"", "Step_Type"="", "LowLimit"=0.0, "HighLimit"=0.0, "RValue"="", "RStatus"="", "RetVal"="0", "Units"="", "header1"="", "header2"="--- special test for pins 9, 7, and 15 ---\r\r\r\r\r\r\r\r\r\r\r\r\r\r\r\r\r\r\r\r\r\r\r\r\r\r\r\r\r\r\r\r\r\r\r\r\r\r\r\r\r\r\r\r", "ExpectedValue"=""}, {"Test_Name"="338. SetAsicRegister \"1\" \"5\" \"00\"", "Step_Type"="", "LowLimit"=0.0, "HighLimit"=0.0, "RValue"="", "RStatus"="", "RetVal"="0", "Units"="", "header1"="", "header2"="--- special test for pins 9, 7, and 15 ---\r\r\r\r\r\r\r\r\r\r\r\r\r\r\r\r\r\r\r\r\r\r\r\r\r\r\r\r\r\r\r\r\r\r\r\r\r\r\r\r\r\r\r\r\r", "ExpectedValue"=""}, {"Test_Name"="339. SetFpgaRegister \"89F\" \"00\"", "Step_Type"="", "LowLimit"=0.0, "HighLimit"=0.0, "RValue"="", "RStatus"="", "RetVal"="0", "Units"="", "header1"="", "header2"="--- special test for pins 9, 7, and 15 ---\r\r\r\r\r\r\r\r\r\r\r\r\r\r\r\r\r\r\r\r\r\r\r\r\r\r\r\r\r\r\r\r\r\r\r\r\r\r\r\r\r\r\r\r\r\r", "ExpectedValue"=""}, {"Test_Name"="341. ---Start Pull Up to 15v test---", "Step_Type"="", "LowLimit"=0.0, "HighLimit"=0.0, "RValue"="", "RStatus"="", "RetVal"="", "Units"="", "header1"="", "header2"="---Start Pull Up to 15v test------------\r", "ExpectedValue"=""}, {"Test_Name"="342. SetG15PullUp \"A\" \"9\"", "Step_Type"="", "LowLimit"=0.0, "HighLimit"=0.0, "RValue"="", "RStatus"="", "RetVal"="0", "Units"="", "header1"="", "header2"="---Start Pull Up to 15v test------------\r\r", "ExpectedValue"=""}, {"Test_Name"="343. SetG15PullUp \"B\" \"9\"", "Step_Type"="", "LowLimit"=0.0, "HighLimit"=0.0, "RValue"="", "RStatus"="", "RetVal"="0", "Units"="", "header1"="", "header2"="---Start Pull Up to 15v test------------\r\r\r", "ExpectedValue"=""}, {"Test_Name"="344. SetG15PullDown \"A\" \"4\"", "Step_Type"="", "LowLimit"=0.0, "HighLimit"=0.0, "RValue"="", "RStatus"="", "RetVal"="0", "Units"="", "header1"="", "header2"="---Start Pull Up to 15v test------------\r\r\r\r", "ExpectedValue"=""}, {"Test_Name"="345. SetG15PullDown \"B\" \"4\"", "Step_Type"="", "LowLimit"=0.0, "HighLimit"=0.0, "RValue"="", "RStatus"="", "RetVal"="0", "Units"="", "header1"="", "header2"="---Start Pull Up to 15v test------------\r\r\r\r\r", "ExpectedValue"=""}, {"Test_Name"="346. SetG15PullupVbat \"0\" \"1\"", "Step_Type"="", "LowLimit"=0.0, "HighLimit"=0.0, "RValue"="", "RStatus"="", "RetVal"="0", "Units"="", "header1"="", "header2"="---Start Pull Up to 15v test------------\r\r\r\r\r\r", "ExpectedValue"=""}, {"Test_Name"="347. CheckCFAdc \"PD1\" \"6.9\" \"7.7\"", "Step_Type"="NumericLimitTest", "LowLimit"=6.9, "HighLimit"=7.7, "RValue"="7.269999980926514", "RStatus"="PASS", "RetVal"="0", "Units"="Volts", "header1"="", "header2"="---Start Pull Up to 15v test------------\r\r\r\r\r\r\r", "ExpectedValue"=""}, {"Test_Name"="348. CheckCFAdc \"PD2\" \"6.9\" \"7.7\"", "Step_Type"="NumericLimitTest", "LowLimit"=6.9, "HighLimit"=7.7, "RValue"="7.309000015258789", "RStatus"="PASS", "RetVal"="0", "Units"="Volts", "header1"="", "header2"="---Start Pull Up to 15v test------------\r\r\r\r\r\r\r\r", "ExpectedValue"=""}, {"Test_Name"="350. SetG15PullupVbat \"0\" \"0\"", "Step_Type"="", "LowLimit"=0.0, "HighLimit"=0.0, "RValue"="", "RStatus"="", "RetVal"="0", "Units"="", "header1"="", "header2"="---Start Pull Up to 15v test------------\r\r\r\r\r\r\r\r\r", "ExpectedValue"=""}, {"Test_Name"="352. CheckCFAdc \"PD1\" \"2.15\" \"2.65\"", "Step_Type"="NumericLimitTest", "LowLimit"=2.15, "HighLimit"=2.65, "RValue"="2.437999963760376", "RStatus"="PASS", "RetVal"="0", "Units"="Volts", "header1"="", "header2"="---Start Pull Up to 15v test------------\r\r\r\r\r\r\r\r\r\r", "ExpectedValue"=""}, {"Test_Name"="353. CheckCFAdc \"PD2\" \"2.15\" \"2.65\"", "Step_Type"="NumericLimitTest", "LowLimit"=2.15, "HighLimit"=2.65, "RValue"="2.4549999237060547", "RStatus"="PASS", "RetVal"="0", "Units"="Volts", "header1"="", "header2"="---Start Pull Up to 15v test------------\r\r\r\r\r\r\r\r\r\r\r", "ExpectedValue"=""}, {"Test_Name"="355. SetG15PullUp \"A\" \"0\"", "Step_Type"="", "LowLimit"=0.0, "HighLimit"=0.0, "RValue"="", "RStatus"="", "RetVal"="0", "Units"="", "header1"="", "header2"="---Start Pull Up to 15v test------------\r\r\r\r\r\r\r\r\r\r\r\r", "ExpectedValue"=""}, {"Test_Name"="356. SetG15PullUp \"B\" \"0\"", "Step_Type"="", "LowLimit"=0.0, "HighLimit"=0.0, "RValue"="", "RStatus"="", "RetVal"="0", "Units"="", "header1"="", "header2"="---Start Pull Up to 15v test------------\r\r\r\r\r\r\r\r\r\r\r\r\r", "ExpectedValue"=""}, {"Test_Name"="357. SetG15PullDown \"A\" \"0\"", "Step_Type"="", "LowLimit"=0.0, "HighLimit"=0.0, "RValue"="", "RStatus"="", "RetVal"="0", "Units"="", "header1"="", "header2"="---Start Pull Up to 15v test------------\r\r\r\r\r\r\r\r\r\r\r\r\r\r", "ExpectedValue"=""}, {"Test_Name"="358. SetG15PullDown \"B\" \"0\"", "Step_Type"="", "LowLimit"=0.0, "HighLimit"=0.0, "RValue"="", "RStatus"="", "RetVal"="0", "Units"="", "header1"="", "header2"="---Start Pull Up to 15v test------------\r\r\r\r\r\r\r\r\r\r\r\r\r\r\r", "ExpectedValue"=""}, {"Test_Name"="361. --- DAC Comparator Tests ---", "Step_Type"="", "LowLimit"=0.0, "HighLimit"=0.0, "RValue"="", "RStatus"="", "RetVal"="", "Units"="", "header1"="", "header2"="--- DAC Comparator Tests ---------------\r", "ExpectedValue"=""}, {"Test_Name"="363. SetBaud \"1\"", "Step_Type"="", "LowLimit"=0.0, "HighLimit"=0.0, "RValue"="", "RStatus"="", "RetVal"="0", "Units"="", "header1"="", "header2"="--- DAC Comparator Tests ---------------\r\r", "ExpectedValue"=""}, {"Test_Name"="364. SelectMuxA \"1\" \"9\" \"1\"", "Step_Type"="", "LowLimit"=0.0, "HighLimit"=0.0, "RValue"="", "RStatus"="", "RetVal"="0", "Units"="", "header1"="", "header2"="--- DAC Comparator Tests ---------------\r\r\r", "ExpectedValue"=""}, {"Test_Name"="365. SelectMuxB \"1\" \"15\" \"1\"", "Step_Type"="", "LowLimit"=0.0, "HighLimit"=0.0, "RValue"="", "RStatus"="", "RetVal"="0", "Units"="", "header1"="", "header2"="--- DAC Comparator Tests ---------------\r\r\r\r", "ExpectedValue"=""}, {"Test_Name"="368. SetG15PullUp \"A\" \"9\"", "Step_Type"="", "LowLimit"=0.0, "HighLimit"=0.0, "RValue"="", "RStatus"="", "RetVal"="0", "Units"="", "header1"="", "header2"="--- DAC Comparator Tests ---------------\r\r\r\r\r", "ExpectedValue"=""}, {"Test_Name"="369. SetG15PullUp \"B\" \"9\"", "Step_Type"="", "LowLimit"=0.0, "HighLimit"=0.0, "RValue"="", "RStatus"="", "RetVal"="0", "Units"="", "header1"="", "header2"="--- DAC Comparator Tests ---------------\r\r\r\r\r\r", "ExpectedValue"=""}, {"Test_Name"="370. SetG15PullDown \"A\" \"4\"", "Step_Type"="", "LowLimit"=0.0, "HighLimit"=0.0, "RValue"="", "RStatus"="", "RetVal"="0", "Units"="", "header1"="", "header2"="--- DAC Comparator Tests ---------------\r\r\r\r\r\r\r", "ExpectedValue"=""}, {"Test_Name"="371. SetG15PullDown \"B\" \"4\"", "Step_Type"="", "LowLimit"=0.0, "HighLimit"=0.0, "RValue"="", "RStatus"="", "RetVal"="0", "Units"="", "header1"="", "header2"="--- DAC Comparator Tests ---------------\r\r\r\r\r\r\r\r", "ExpectedValue"=""}, {"Test_Name"="373. CheckCFAdc \"PD1\" \"2.15\" \"2.65\"", "Step_Type"="NumericLimitTest", "LowLimit"=2.15, "HighLimit"=2.65, "RValue"="2.437999963760376", "RStatus"="PASS", "RetVal"="0", "Units"="Volts", "header1"="", "header2"="--- DAC Comparator Tests ---------------\r\r\r\r\r\r\r\r\r", "ExpectedValue"=""}, {"Test_Name"="376. SetReference \"53\"", "Step_Type"="", "LowLimit"=0.0, "HighLimit"=0.0, "RValue"="", "RStatus"="", "RetVal"="0", "Units"="", "header1"="", "header2"="--- DAC Comparator Tests ---------------\r\r\r\r\r\r\r\r\r\r", "ExpectedValue"=""}, {"Test_Name"="377. Pause \"100\"", "Step_Type"="", "LowLimit"=0.0, "HighLimit"=0.0, "RValue"="", "RStatus"="", "RetVal"="0", "Units"="", "header1"="", "header2"="--- DAC Comparator Tests ---------------\r\r\r\r\r\r\r\r\r\r\r", "ExpectedValue"=""}, {"Test_Name"="378. CheckFpgaRegister \"8A8\" \"0\" \"0\"", "Step_Type"="StringValueTest", "LowLimit"=0.0, "HighLimit"=0.0, "RValue"="12", "RStatus"="PASS", "RetVal"="0", "Units"="", "header1"="", "header2"="--- DAC Comparator Tests ---------------\r\r\r\r\r\r\r\r\r\r\r\r", "ExpectedValue"=""}, {"Test_Name"="379. CheckFpgaRegister \"8A8\" \"1\" \"0\"", "Step_Type"="StringValueTest", "LowLimit"=0.0, "HighLimit"=0.0, "RValue"="12", "RStatus"="PASS", "RetVal"="0", "Units"="", "header1"="", "header2"="--- DAC Comparator Tests ---------------\r\r\r\r\r\r\r\r\r\r\r\r\r", "ExpectedValue"=""}, {"Test_Name"="380. CheckFpgaRegister \"858\" \"4\" \"0\"", "Step_Type"="StringValueTest", "LowLimit"=0.0, "HighLimit"=0.0, "RValue"="0", "RStatus"="PASS", "RetVal"="0", "Units"="", "header1"="", "header2"="--- DAC Comparator Tests ---------------\r\r\r\r\r\r\r\r\r\r\r\r\r\r", "ExpectedValue"=""}, {"Test_Name"="381. CheckFpgaRegister \"859\" \"6\" \"0\"", "Step_Type"="StringValueTest", "LowLimit"=0.0, "HighLimit"=0.0, "RValue"="0", "RStatus"="PASS", "RetVal"="0", "Units"="", "header1"="", "header2"="--- DAC Comparator Tests ---------------\r\r\r\r\r\r\r\r\r\r\r\r\r\r\r", "ExpectedValue"=""}, {"Test_Name"="382. ComparatorCheck \"9\" \"0\"", "Step_Type"="StringValueTest", "LowLimit"=0.0, "HighLimit"=0.0, "RValue"="", "RStatus"="PASS", "RetVal"="0", "Units"="", "header1"="", "header2"="--- DAC Comparator Tests ---------------\r\r\r\r\r\r\r\r\r\r\r\r\r\r\r\r", "ExpectedValue"=""}, {"Test_Name"="383. ComparatorCheck \"15\" \"0\"", "Step_Type"="StringValueTest", "LowLimit"=0.0, "HighLimit"=0.0, "RValue"="", "RStatus"="PASS", "RetVal"="0", "Units"="", "header1"="", "header2"="--- DAC Comparator Tests ---------------\r\r\r\r\r\r\r\r\r\r\r\r\r\r\r\r\r", "ExpectedValue"=""}, {"Test_Name"="385. ---Change comparator DAC voltage BELOW", "Step_Type"="", "LowLimit"=0.0, "HighLimit"=0.0, "RValue"="", "RStatus"="", "RetVal"="", "Units"="", "header1"="", "header2"="---Change comparator DAC voltage BELOW--\r", "ExpectedValue"=""}, {"Test_Name"="386. SetReference \"65\"", "Step_Type"="", "LowLimit"=0.0, "HighLimit"=0.0, "RValue"="", "RStatus"="", "RetVal"="0", "Units"="", "header1"="", "header2"="---Change comparator DAC voltage BELOW--\r\r", "ExpectedValue"=""}, {"Test_Name"="387. Pause \"100\"", "Step_Type"="", "LowLimit"=0.0, "HighLimit"=0.0, "RValue"="", "RStatus"="", "RetVal"="0", "Units"="", "header1"="", "header2"="---Change comparator DAC voltage BELOW--\r\r\r", "ExpectedValue"=""}, {"Test_Name"="388. CheckFpgaRegister \"8A8\" \"0\" \"1\"", "Step_Type"="StringValueTest", "LowLimit"=0.0, "HighLimit"=0.0, "RValue"="15", "RStatus"="PASS", "RetVal"="0", "Units"="", "header1"="", "header2"="---Change comparator DAC voltage BELOW--\r\r\r\r", "ExpectedValue"=""}, {"Test_Name"="389. CheckFpgaRegister \"8A8\" \"1\" \"1\"", "Step_Type"="StringValueTest", "LowLimit"=0.0, "HighLimit"=0.0, "RValue"="15", "RStatus"="PASS", "RetVal"="0", "Units"="", "header1"="", "header2"="---Change comparator DAC voltage BELOW--\r\r\r\r\r", "ExpectedValue"=""}, {"Test_Name"="390. CheckFpgaRegister \"858\" \"4\" \"1\"", "Step_Type"="StringValueTest", "LowLimit"=0.0, "HighLimit"=0.0, "RValue"="16", "RStatus"="PASS", "RetVal"="0", "Units"="", "header1"="", "header2"="---Change comparator DAC voltage BELOW--\r\r\r\r\r\r", "ExpectedValue"=""}, {"Test_Name"="391. CheckFpgaRegister \"859\" \"6\" \"1\"", "Step_Type"="StringValueTest", "LowLimit"=0.0, "HighLimit"=0.0, "RValue"="64", "RStatus"="PASS", "RetVal"="0", "Units"="", "header1"="", "header2"="---Change comparator DAC voltage BELOW--\r\r\r\r\r\r\r", "ExpectedValue"=""}, {"Test_Name"="392. ComparatorCheck \"9\" \"1\"", "Step_Type"="StringValueTest", "LowLimit"=0.0, "HighLimit"=0.0, "RValue"="", "RStatus"="PASS", "RetVal"="1", "Units"="", "header1"="", "header2"="---Change comparator DAC voltage BELOW--\r\r\r\r\r\r\r\r", "ExpectedValue"=""}, {"Test_Name"="393. ComparatorCheck \"15\" \"1\"", "Step_Type"="StringValueTest", "LowLimit"=0.0, "HighLimit"=0.0, "RValue"="", "RStatus"="PASS", "RetVal"="1", "Units"="", "header1"="", "header2"="---Change comparator DAC voltage BELOW--\r\r\r\r\r\r\r\r\r", "ExpectedValue"=""}, {"Test_Name"="395. SetReference \"128\"", "Step_Type"="", "LowLimit"=0.0, "HighLimit"=0.0, "RValue"="", "RStatus"="", "RetVal"="0", "Units"="", "header1"="", "header2"="---Change comparator DAC voltage BELOW--\r\r\r\r\r\r\r\r\r\r", "ExpectedValue"=""}, {"Test_Name"="396. SelectAllMuxA \"1\" \"0\"", "Step_Type"="", "LowLimit"=0.0, "HighLimit"=0.0, "RValue"="", "RStatus"="", "RetVal"="0", "Units"="", "header1"="", "header2"="---Change comparator DAC voltage BELOW--\r\r\r\r\r\r\r\r\r\r\r", "ExpectedValue"=""}, {"Test_Name"="397. SelectAllMuxB \"1\" \"0\"", "Step_Type"="", "LowLimit"=0.0, "HighLimit"=0.0, "RValue"="", "RStatus"="", "RetVal"="0", "Units"="", "header1"="", "header2"="---Change comparator DAC voltage BELOW--\r\r\r\r\r\r\r\r\r\r\r\r", "ExpectedValue"=""}, {"Test_Name"="398. SetG15PullUp \"A\" \"0\"", "Step_Type"="", "LowLimit"=0.0, "HighLimit"=0.0, "RValue"="", "RStatus"="", "RetVal"="0", "Units"="", "header1"="", "header2"="---Change comparator DAC voltage BELOW--\r\r\r\r\r\r\r\r\r\r\r\r\r", "ExpectedValue"=""}, {"Test_Name"="399. SetG15PullUp \"B\" \"0\"", "Step_Type"="", "LowLimit"=0.0, "HighLimit"=0.0, "RValue"="", "RStatus"="", "RetVal"="0", "Units"="", "header1"="", "header2"="---Change comparator DAC voltage BELOW--\r\r\r\r\r\r\r\r\r\r\r\r\r\r", "ExpectedValue"=""}, {"Test_Name"="400. SetG15PullDown \"A\" \"0\"", "Step_Type"="", "LowLimit"=0.0, "HighLimit"=0.0, "RValue"="", "RStatus"="", "RetVal"="0", "Units"="", "header1"="", "header2"="---Change comparator DAC voltage BELOW--\r\r\r\r\r\r\r\r\r\r\r\r\r\r\r", "ExpectedValue"=""}, {"Test_Name"="401. SetG15PullDown \"B\" \"0\"", "Step_Type"="", "LowLimit"=0.0, "HighLimit"=0.0, "RValue"="", "RStatus"="", "RetVal"="0", "Units"="", "header1"="", "header2"="---Change comparator DAC voltage BELOW--\r\r\r\r\r\r\r\r\r\r\r\r\r\r\r\r", "ExpectedValue"=""}, {"Test_Name"="404. --- Start Switch Matrix 1A MUX A (ASIC 1) and Switch Matrix 1A MUX C (ASIC 2) Tests ---", "Step_Type"="", "LowLimit"=0.0, "HighLimit"=0.0, "RValue"="", "RStatus"="", "RetVal"="", "Units"="", "header1"="", "header2"="--- Start Switch Matrix 1A MUX A (ASIC 1) and Switch Matrix 1A MUX C (ASIC 2) Tests ---\r", "ExpectedValue"=""}, {"Test_Name"="408. SelectAllMuxA \"1\" \"0\"", "Step_Type"="", "LowLimit"=0.0, "HighLimit"=0.0, "RValue"="", "RStatus"="", "RetVal"="0", "Units"="", "header1"="", "header2"="--- Start Switch Matrix 1A MUX A (ASIC 1) and Switch Matrix 1A MUX C (ASIC 2) Tests ---\r\r", "ExpectedValue"=""}, {"Test_Name"="409. SelectAllMuxA \"2\" \"0\"", "Step_Type"="", "LowLimit"=0.0, "HighLimit"=0.0, "RValue"="", "RStatus"="", "RetVal"="0", "Units"="", "header1"="", "header2"="--- Start Switch Matrix 1A MUX A (ASIC 1) and Switch Matrix 1A MUX C (ASIC 2) Tests ---\r\r\r", "ExpectedValue"=""}, {"Test_Name"="412. SetG15PullUp \"A\" \"9\"", "Step_Type"="", "LowLimit"=0.0, "HighLimit"=0.0, "RValue"="", "RStatus"="", "RetVal"="0", "Units"="", "header1"="", "header2"="--- Start Switch Matrix 1A MUX A (ASIC 1) and Switch Matrix 1A MUX C (ASIC 2) Tests ---\r\r\r\r", "ExpectedValue"=""}, {"Test_Name"="413. SetG15PullUp \"C\" \"0\"", "Step_Type"="", "LowLimit"=0.0, "HighLimit"=0.0, "RValue"="", "RStatus"="", "RetVal"="0", "Units"="", "header1"="", "header2"="--- Start Switch Matrix 1A MUX A (ASIC 1) and Switch Matrix 1A MUX C (ASIC 2) Tests ---\r\r\r\r\r", "ExpectedValue"=""}, {"Test_Name"="414. SetG15PullDown \"A\" \"4\"", "Step_Type"="", "LowLimit"=0.0, "HighLimit"=0.0, "RValue"="", "RStatus"="", "RetVal"="0", "Units"="", "header1"="", "header2"="--- Start Switch Matrix 1A MUX A (ASIC 1) and Switch Matrix 1A MUX C (ASIC 2) Tests ---\r\r\r\r\r\r", "ExpectedValue"=""}, {"Test_Name"="415. SetG15PullDown \"C\" \"0\"", "Step_Type"="", "LowLimit"=0.0, "HighLimit"=0.0, "RValue"="", "RStatus"="", "RetVal"="0", "Units"="", "header1"="", "header2"="--- Start Switch Matrix 1A MUX A (ASIC 1) and Switch Matrix 1A MUX C (ASIC 2) Tests ---\r\r\r\r\r\r\r", "ExpectedValue"=""}, {"Test_Name"="416. CheckCFAdc \"PD1\" \"2.2\" \"2.65\"", "Step_Type"="NumericLimitTest", "LowLimit"=2.2, "HighLimit"=2.65, "RValue"="2.437999963760376", "RStatus"="PASS", "RetVal"="0", "Units"="Volts", "header1"="", "header2"="--- Start Switch Matrix 1A MUX A (ASIC 1) and Switch Matrix 1A MUX C (ASIC 2) Tests ---\r\r\r\r\r\r\r\r", "ExpectedValue"=""}, {"Test_Name"="417. CheckCFAdc \"PD3\" \"-.15\" \"1.2\"", "Step_Type"="NumericLimitTest", "LowLimit"=-0.15, "HighLimit"=1.2, "RValue"="0.7519999742507935", "RStatus"="PASS", "RetVal"="0", "Units"="Volts", "header1"="", "header2"="--- Start Switch Matrix 1A MUX A (ASIC 1) and Switch Matrix 1A MUX C (ASIC 2) Tests ---\r\r\r\r\r\r\r\r\r", "ExpectedValue"=""}, {"Test_Name"="419. SelectMuxA \"1\" \"1\" \"1\"", "Step_Type"="", "LowLimit"=0.0, "HighLimit"=0.0, "RValue"="", "RStatus"="", "RetVal"="0", "Units"="", "header1"="", "header2"="--- Start Switch Matrix 1A MUX A (ASIC 1) and Switch Matrix 1A MUX C (ASIC 2) Tests ---\r\r\r\r\r\r\r\r\r\r", "ExpectedValue"=""}, {"Test_Name"="420. SelectMuxA \"2\" \"1\" \"1\"", "Step_Type"="", "LowLimit"=0.0, "HighLimit"=0.0, "RValue"="", "RStatus"="", "RetVal"="0", "Units"="", "header1"="", "header2"="--- Start Switch Matrix 1A MUX A (ASIC 1) and Switch Matrix 1A MUX C (ASIC 2) Tests ---\r\r\r\r\r\r\r\r\r\r\r", "ExpectedValue"=""}, {"Test_Name"="421. CheckCFAdc \"PD3\" \"2.2\" \"2.65\"", "Step_Type"="NumericLimitTest", "LowLimit"=2.2, "HighLimit"=2.65, "RValue"="2.4509999752044678", "RStatus"="PASS", "RetVal"="0", "Units"="Volts", "header1"="", "header2"="--- Start Switch Matrix 1A MUX A (ASIC 1) and Switch Matrix 1A MUX C (ASIC 2) Tests ---\r\r\r\r\r\r\r\r\r\r\r\r", "ExpectedValue"=""}, {"Test_Name"="422. SelectAllMuxA \"1\" \"0\"", "Step_Type"="", "LowLimit"=0.0, "HighLimit"=0.0, "RValue"="", "RStatus"="", "RetVal"="0", "Units"="", "header1"="", "header2"="--- Start Switch Matrix 1A MUX A (ASIC 1) and Switch Matrix 1A MUX C (ASIC 2) Tests ---\r\r\r\r\r\r\r\r\r\r\r\r\r", "ExpectedValue"=""}, {"Test_Name"="423. SelectAllMuxA \"2\" \"0\"", "Step_Type"="", "LowLimit"=0.0, "HighLimit"=0.0, "RValue"="", "RStatus"="", "RetVal"="0", "Units"="", "header1"="", "header2"="--- Start Switch Matrix 1A MUX A (ASIC 1) and Switch Matrix 1A MUX C (ASIC 2) Tests ---\r\r\r\r\r\r\r\r\r\r\r\r\r\r", "ExpectedValue"=""}, {"Test_Name"="425. SelectMuxA \"1\" \"2\" \"1\"", "Step_Type"="", "LowLimit"=0.0, "HighLimit"=0.0, "RValue"="", "RStatus"="", "RetVal"="0", "Units"="", "header1"="", "header2"="--- Start Switch Matrix 1A MUX A (ASIC 1) and Switch Matrix 1A MUX C (ASIC 2) Tests ---\r\r\r\r\r\r\r\r\r\r\r\r\r\r\r", "ExpectedValue"=""}, {"Test_Name"="426. SelectMuxA \"2\" \"2\" \"1\"", "Step_Type"="", "LowLimit"=0.0, "HighLimit"=0.0, "RValue"="", "RStatus"="", "RetVal"="0", "Units"="", "header1"="", "header2"="--- Start Switch Matrix 1A MUX A (ASIC 1) and Switch Matrix 1A MUX C (ASIC 2) Tests ---\r\r\r\r\r\r\r\r\r\r\r\r\r\r\r\r", "ExpectedValue"=""}, {"Test_Name"="427. CheckCFAdc \"PD3\" \"2.2\" \"2.65\"", "Step_Type"="NumericLimitTest", "LowLimit"=2.2, "HighLimit"=2.65, "RValue"="2.4509999752044678", "RStatus"="PASS", "RetVal"="0", "Units"="Volts", "header1"="", "header2"="--- Start Switch Matrix 1A MUX A (ASIC 1) and Switch Matrix 1A MUX C (ASIC 2) Tests ---\r\r\r\r\r\r\r\r\r\r\r\r\r\r\r\r\r", "ExpectedValue"=""}, {"Test_Name"="428. SelectAllMuxA \"1\" \"0\"", "Step_Type"="", "LowLimit"=0.0, "HighLimit"=0.0, "RValue"="", "RStatus"="", "RetVal"="0", "Units"="", "header1"="", "header2"="--- Start Switch Matrix 1A MUX A (ASIC 1) and Switch Matrix 1A MUX C (ASIC 2) Tests ---\r\r\r\r\r\r\r\r\r\r\r\r\r\r\r\r\r\r", "ExpectedValue"=""}, {"Test_Name"="429. SelectAllMuxA \"2\" \"0\"", "Step_Type"="", "LowLimit"=0.0, "HighLimit"=0.0, "RValue"="", "RStatus"="", "RetVal"="0", "Units"="", "header1"="", "header2"="--- Start Switch Matrix 1A MUX A (ASIC 1) and Switch Matrix 1A MUX C (ASIC 2) Tests ---\r\r\r\r\r\r\r\r\r\r\r\r\r\r\r\r\r\r\r", "ExpectedValue"=""}, {"Test_Name"="431. SelectMuxA \"1\" \"3\" \"1\"", "Step_Type"="", "LowLimit"=0.0, "HighLimit"=0.0, "RValue"="", "RStatus"="", "RetVal"="0", "Units"="", "header1"="", "header2"="--- Start Switch Matrix 1A MUX A (ASIC 1) and Switch Matrix 1A MUX C (ASIC 2) Tests ---\r\r\r\r\r\r\r\r\r\r\r\r\r\r\r\r\r\r\r\r", "ExpectedValue"=""}, {"Test_Name"="432. SelectMuxA \"2\" \"3\" \"1\"", "Step_Type"="", "LowLimit"=0.0, "HighLimit"=0.0, "RValue"="", "RStatus"="", "RetVal"="0", "Units"="", "header1"="", "header2"="--- Start Switch Matrix 1A MUX A (ASIC 1) and Switch Matrix 1A MUX C (ASIC 2) Tests ---\r\r\r\r\r\r\r\r\r\r\r\r\r\r\r\r\r\r\r\r\r", "ExpectedValue"=""}, {"Test_Name"="433. CheckCFAdc \"PD3\" \"2.2\" \"2.65\"", "Step_Type"="NumericLimitTest", "LowLimit"=2.2, "HighLimit"=2.65, "RValue"="2.4509999752044678", "RStatus"="PASS", "RetVal"="0", "Units"="Volts", "header1"="", "header2"="--- Start Switch Matrix 1A MUX A (ASIC 1) and Switch Matrix 1A MUX C (ASIC 2) Tests ---\r\r\r\r\r\r\r\r\r\r\r\r\r\r\r\r\r\r\r\r\r\r", "ExpectedValue"=""}, {"Test_Name"="434. SelectAllMuxA \"1\" \"0\"", "Step_Type"="", "LowLimit"=0.0, "HighLimit"=0.0, "RValue"="", "RStatus"="", "RetVal"="0", "Units"="", "header1"="", "header2"="--- Start Switch Matrix 1A MUX A (ASIC 1) and Switch Matrix 1A MUX C (ASIC 2) Tests ---\r\r\r\r\r\r\r\r\r\r\r\r\r\r\r\r\r\r\r\r\r\r\r", "ExpectedValue"=""}, {"Test_Name"="435. SelectAllMuxA \"2\" \"0\"", "Step_Type"="", "LowLimit"=0.0, "HighLimit"=0.0, "RValue"="", "RStatus"="", "RetVal"="0", "Units"="", "header1"="", "header2"="--- Start Switch Matrix 1A MUX A (ASIC 1) and Switch Matrix 1A MUX C (ASIC 2) Tests ---\r\r\r\r\r\r\r\r\r\r\r\r\r\r\r\r\r\r\r\r\r\r\r\r", "ExpectedValue"=""}, {"Test_Name"="437. SelectMuxA \"1\" \"6\" \"1\"", "Step_Type"="", "LowLimit"=0.0, "HighLimit"=0.0, "RValue"="", "RStatus"="", "RetVal"="0", "Units"="", "header1"="", "header2"="--- Start Switch Matrix 1A MUX A (ASIC 1) and Switch Matrix 1A MUX C (ASIC 2) Tests ---\r\r\r\r\r\r\r\r\r\r\r\r\r\r\r\r\r\r\r\r\r\r\r\r\r", "ExpectedValue"=""}, {"Test_Name"="438. SelectMuxA \"2\" \"6\" \"1\"", "Step_Type"="", "LowLimit"=0.0, "HighLimit"=0.0, "RValue"="", "RStatus"="", "RetVal"="0", "Units"="", "header1"="", "header2"="--- Start Switch Matrix 1A MUX A (ASIC 1) and Switch Matrix 1A MUX C (ASIC 2) Tests ---\r\r\r\r\r\r\r\r\r\r\r\r\r\r\r\r\r\r\r\r\r\r\r\r\r\r", "ExpectedValue"=""}, {"Test_Name"="439. CheckCFAdc \"PD3\" \"2.2\" \"2.65\"", "Step_Type"="NumericLimitTest", "LowLimit"=2.2, "HighLimit"=2.65, "RValue"="2.4509999752044678", "RStatus"="PASS", "RetVal"="0", "Units"="Volts", "header1"="", "header2"="--- Start Switch Matrix 1A MUX A (ASIC 1) and Switch Matrix 1A MUX C (ASIC 2) Tests ---\r\r\r\r\r\r\r\r\r\r\r\r\r\r\r\r\r\r\r\r\r\r\r\r\r\r\r", "ExpectedValue"=""}, {"Test_Name"="440. SelectAllMuxA \"1\" \"0\"", "Step_Type"="", "LowLimit"=0.0, "HighLimit"=0.0, "RValue"="", "RStatus"="", "RetVal"="0", "Units"="", "header1"="", "header2"="--- Start Switch Matrix 1A MUX A (ASIC 1) and Switch Matrix 1A MUX C (ASIC 2) Tests ---\r\r\r\r\r\r\r\r\r\r\r\r\r\r\r\r\r\r\r\r\r\r\r\r\r\r\r\r", "ExpectedValue"=""}, {"Test_Name"="441. SelectAllMuxA \"2\" \"0\"", "Step_Type"="", "LowLimit"=0.0, "HighLimit"=0.0, "RValue"="", "RStatus"="", "RetVal"="0", "Units"="", "header1"="", "header2"="--- Start Switch Matrix 1A MUX A (ASIC 1) and Switch Matrix 1A MUX C (ASIC 2) Tests ---\r\r\r\r\r\r\r\r\r\r\r\r\r\r\r\r\r\r\r\r\r\r\r\r\r\r\r\r\r", "ExpectedValue"=""}, {"Test_Name"="443. SelectMuxA \"1\" \"7\" \"1\"", "Step_Type"="", "LowLimit"=0.0, "HighLimit"=0.0, "RValue"="", "RStatus"="", "RetVal"="0", "Units"="", "header1"="", "header2"="--- Start Switch Matrix 1A MUX A (ASIC 1) and Switch Matrix 1A MUX C (ASIC 2) Tests ---\r\r\r\r\r\r\r\r\r\r\r\r\r\r\r\r\r\r\r\r\r\r\r\r\r\r\r\r\r\r", "ExpectedValue"=""}, {"Test_Name"="444. SelectMuxA \"2\" \"7\" \"1\"", "Step_Type"="", "LowLimit"=0.0, "HighLimit"=0.0, "RValue"="", "RStatus"="", "RetVal"="0", "Units"="", "header1"="", "header2"="--- Start Switch Matrix 1A MUX A (ASIC 1) and Switch Matrix 1A MUX C (ASIC 2) Tests ---\r\r\r\r\r\r\r\r\r\r\r\r\r\r\r\r\r\r\r\r\r\r\r\r\r\r\r\r\r\r\r", "ExpectedValue"=""}, {"Test_Name"="445. CheckCFAdc \"PD3\" \"2.2\" \"2.65\"", "Step_Type"="NumericLimitTest", "LowLimit"=2.2, "HighLimit"=2.65, "RValue"="2.431999921798706", "RStatus"="PASS", "RetVal"="0", "Units"="Volts", "header1"="", "header2"="--- Start Switch Matrix 1A MUX A (ASIC 1) and Switch Matrix 1A MUX C (ASIC 2) Tests ---\r\r\r\r\r\r\r\r\r\r\r\r\r\r\r\r\r\r\r\r\r\r\r\r\r\r\r\r\r\r\r\r", "ExpectedValue"=""}, {"Test_Name"="446. SelectAllMuxA \"1\" \"0\"", "Step_Type"="", "LowLimit"=0.0, "HighLimit"=0.0, "RValue"="", "RStatus"="", "RetVal"="0", "Units"="", "header1"="", "header2"="--- Start Switch Matrix 1A MUX A (ASIC 1) and Switch Matrix 1A MUX C (ASIC 2) Tests ---\r\r\r\r\r\r\r\r\r\r\r\r\r\r\r\r\r\r\r\r\r\r\r\r\r\r\r\r\r\r\r\r\r", "ExpectedValue"=""}, {"Test_Name"="447. SelectAllMuxA \"2\" \"0\"", "Step_Type"="", "LowLimit"=0.0, "HighLimit"=0.0, "RValue"="", "RStatus"="", "RetVal"="0", "Units"="", "header1"="", "header2"="--- Start Switch Matrix 1A MUX A (ASIC 1) and Switch Matrix 1A MUX C (ASIC 2) Tests ---\r\r\r\r\r\r\r\r\r\r\r\r\r\r\r\r\r\r\r\r\r\r\r\r\r\r\r\r\r\r\r\r\r\r", "ExpectedValue"=""}, {"Test_Name"="449. SelectMuxA \"1\" \"8\" \"1\"", "Step_Type"="", "LowLimit"=0.0, "HighLimit"=0.0, "RValue"="", "RStatus"="", "RetVal"="0", "Units"="", "header1"="", "header2"="--- Start Switch Matrix 1A MUX A (ASIC 1) and Switch Matrix 1A MUX C (ASIC 2) Tests ---\r\r\r\r\r\r\r\r\r\r\r\r\r\r\r\r\r\r\r\r\r\r\r\r\r\r\r\r\r\r\r\r\r\r\r", "ExpectedValue"=""}, {"Test_Name"="450. SelectMuxA \"2\" \"8\" \"1\"", "Step_Type"="", "LowLimit"=0.0, "HighLimit"=0.0, "RValue"="", "RStatus"="", "RetVal"="0", "Units"="", "header1"="", "header2"="--- Start Switch Matrix 1A MUX A (ASIC 1) and Switch Matrix 1A MUX C (ASIC 2) Tests ---\r\r\r\r\r\r\r\r\r\r\r\r\r\r\r\r\r\r\r\r\r\r\r\r\r\r\r\r\r\r\r\r\r\r\r\r", "ExpectedValue"=""}, {"Test_Name"="451. CheckCFAdc \"PD3\" \"2.2\" \"2.65\"", "Step_Type"="NumericLimitTest", "LowLimit"=2.2, "HighLimit"=2.65, "RValue"="2.4509999752044678", "RStatus"="PASS", "RetVal"="0", "Units"="Volts", "header1"="", "header2"="--- Start Switch Matrix 1A MUX A (ASIC 1) and Switch Matrix 1A MUX C (ASIC 2) Tests ---\r\r\r\r\r\r\r\r\r\r\r\r\r\r\r\r\r\r\r\r\r\r\r\r\r\r\r\r\r\r\r\r\r\r\r\r\r", "ExpectedValue"=""}, {"Test_Name"="452. SelectAllMuxA \"1\" \"0\"", "Step_Type"="", "LowLimit"=0.0, "HighLimit"=0.0, "RValue"="", "RStatus"="", "RetVal"="0", "Units"="", "header1"="", "header2"="--- Start Switch Matrix 1A MUX A (ASIC 1) and Switch Matrix 1A MUX C (ASIC 2) Tests ---\r\r\r\r\r\r\r\r\r\r\r\r\r\r\r\r\r\r\r\r\r\r\r\r\r\r\r\r\r\r\r\r\r\r\r\r\r\r", "ExpectedValue"=""}, {"Test_Name"="453. SelectAllMuxA \"2\" \"0\"", "Step_Type"="", "LowLimit"=0.0, "HighLimit"=0.0, "RValue"="", "RStatus"="", "RetVal"="0", "Units"="", "header1"="", "header2"="--- Start Switch Matrix 1A MUX A (ASIC 1) and Switch Matrix 1A MUX C (ASIC 2) Tests ---\r\r\r\r\r\r\r\r\r\r\r\r\r\r\r\r\r\r\r\r\r\r\r\r\r\r\r\r\r\r\r\r\r\r\r\r\r\r\r", "ExpectedValue"=""}, {"Test_Name"="455. SelectMuxA \"1\" \"9\" \"1\"", "Step_Type"="", "LowLimit"=0.0, "HighLimit"=0.0, "RValue"="", "RStatus"="", "RetVal"="0", "Units"="", "header1"="", "header2"="--- Start Switch Matrix 1A MUX A (ASIC 1) and Switch Matrix 1A MUX C (ASIC 2) Tests ---\r\r\r\r\r\r\r\r\r\r\r\r\r\r\r\r\r\r\r\r\r\r\r\r\r\r\r\r\r\r\r\r\r\r\r\r\r\r\r\r", "ExpectedValue"=""}, {"Test_Name"="456. SelectMuxA \"2\" \"9\" \"1\"", "Step_Type"="", "LowLimit"=0.0, "HighLimit"=0.0, "RValue"="", "RStatus"="", "RetVal"="0", "Units"="", "header1"="", "header2"="--- Start Switch Matrix 1A MUX A (ASIC 1) and Switch Matrix 1A MUX C (ASIC 2) Tests ---\r\r\r\r\r\r\r\r\r\r\r\r\r\r\r\r\r\r\r\r\r\r\r\r\r\r\r\r\r\r\r\r\r\r\r\r\r\r\r\r\r", "ExpectedValue"=""}, {"Test_Name"="457. CheckCFAdc \"PD3\" \"2.2\" \"2.65\"", "Step_Type"="NumericLimitTest", "LowLimit"=2.2, "HighLimit"=2.65, "RValue"="2.4509999752044678", "RStatus"="PASS", "RetVal"="0", "Units"="Volts", "header1"="", "header2"="--- Start Switch Matrix 1A MUX A (ASIC 1) and Switch Matrix 1A MUX C (ASIC 2) Tests ---\r\r\r\r\r\r\r\r\r\r\r\r\r\r\r\r\r\r\r\r\r\r\r\r\r\r\r\r\r\r\r\r\r\r\r\r\r\r\r\r\r\r", "ExpectedValue"=""}, {"Test_Name"="458. SelectAllMuxA \"1\" \"0\"", "Step_Type"="", "LowLimit"=0.0, "HighLimit"=0.0, "RValue"="", "RStatus"="", "RetVal"="0", "Units"="", "header1"="", "header2"="--- Start Switch Matrix 1A MUX A (ASIC 1) and Switch Matrix 1A MUX C (ASIC 2) Tests ---\r\r\r\r\r\r\r\r\r\r\r\r\r\r\r\r\r\r\r\r\r\r\r\r\r\r\r\r\r\r\r\r\r\r\r\r\r\r\r\r\r\r\r", "ExpectedValue"=""}, {"Test_Name"="459. SelectAllMuxA \"2\" \"0\"", "Step_Type"="", "LowLimit"=0.0, "HighLimit"=0.0, "RValue"="", "RStatus"="", "RetVal"="0", "Units"="", "header1"="", "header2"="--- Start Switch Matrix 1A MUX A (ASIC 1) and Switch Matrix 1A MUX C (ASIC 2) Tests ---\r\r\r\r\r\r\r\r\r\r\r\r\r\r\r\r\r\r\r\r\r\r\r\r\r\r\r\r\r\r\r\r\r\r\r\r\r\r\r\r\r\r\r\r", "ExpectedValue"=""}, {"Test_Name"="461. SelectMuxA \"1\" \"10\" \"1\"", "Step_Type"="", "LowLimit"=0.0, "HighLimit"=0.0, "RValue"="", "RStatus"="", "RetVal"="0", "Units"="", "header1"="", "header2"="--- Start Switch Matrix 1A MUX A (ASIC 1) and Switch Matrix 1A MUX C (ASIC 2) Tests ---\r\r\r\r\r\r\r\r\r\r\r\r\r\r\r\r\r\r\r\r\r\r\r\r\r\r\r\r\r\r\r\r\r\r\r\r\r\r\r\r\r\r\r\r\r", "ExpectedValue"=""}, {"Test_Name"="462. SelectMuxA \"2\" \"10\" \"1\"", "Step_Type"="", "LowLimit"=0.0, "HighLimit"=0.0, "RValue"="", "RStatus"="", "RetVal"="0", "Units"="", "header1"="", "header2"="--- Start Switch Matrix 1A MUX A (ASIC 1) and Switch Matrix 1A MUX C (ASIC 2) Tests ---\r\r\r\r\r\r\r\r\r\r\r\r\r\r\r\r\r\r\r\r\r\r\r\r\r\r\r\r\r\r\r\r\r\r\r\r\r\r\r\r\r\r\r\r\r\r", "ExpectedValue"=""}, {"Test_Name"="463. CheckCFAdc \"PD3\" \"2.2\" \"2.65\"", "Step_Type"="NumericLimitTest", "LowLimit"=2.2, "HighLimit"=2.65, "RValue"="2.4509999752044678", "RStatus"="PASS", "RetVal"="0", "Units"="Volts", "header1"="", "header2"="--- Start Switch Matrix 1A MUX A (ASIC 1) and Switch Matrix 1A MUX C (ASIC 2) Tests ---\r\r\r\r\r\r\r\r\r\r\r\r\r\r\r\r\r\r\r\r\r\r\r\r\r\r\r\r\r\r\r\r\r\r\r\r\r\r\r\r\r\r\r\r\r\r\r", "ExpectedValue"=""}, {"Test_Name"="464. SelectAllMuxA \"1\" \"0\"", "Step_Type"="", "LowLimit"=0.0, "HighLimit"=0.0, "RValue"="", "RStatus"="", "RetVal"="0", "Units"="", "header1"="", "header2"="--- Start Switch Matrix 1A MUX A (ASIC 1) and Switch Matrix 1A MUX C (ASIC 2) Tests ---\r\r\r\r\r\r\r\r\r\r\r\r\r\r\r\r\r\r\r\r\r\r\r\r\r\r\r\r\r\r\r\r\r\r\r\r\r\r\r\r\r\r\r\r\r\r\r\r", "ExpectedValue"=""}, {"Test_Name"="465. SelectAllMuxA \"2\" \"0\"", "Step_Type"="", "LowLimit"=0.0, "HighLimit"=0.0, "RValue"="", "RStatus"="", "RetVal"="0", "Units"="", "header1"="", "header2"="--- Start Switch Matrix 1A MUX A (ASIC 1) and Switch Matrix 1A MUX C (ASIC 2) Tests ---\r\r\r\r\r\r\r\r\r\r\r\r\r\r\r\r\r\r\r\r\r\r\r\r\r\r\r\r\r\r\r\r\r\r\r\r\r\r\r\r\r\r\r\r\r\r\r\r\r", "ExpectedValue"=""}, {"Test_Name"="467. SelectMuxA \"1\" \"11\" \"1\"", "Step_Type"="", "LowLimit"=0.0, "HighLimit"=0.0, "RValue"="", "RStatus"="", "RetVal"="0", "Units"="", "header1"="", "header2"="--- Start Switch Matrix 1A MUX A (ASIC 1) and Switch Matrix 1A MUX C (ASIC 2) Tests ---\r\r\r\r\r\r\r\r\r\r\r\r\r\r\r\r\r\r\r\r\r\r\r\r\r\r\r\r\r\r\r\r\r\r\r\r\r\r\r\r\r\r\r\r\r\r\r\r\r\r", "ExpectedValue"=""}, {"Test_Name"="468. SelectMuxA \"2\" \"11\" \"1\"", "Step_Type"="", "LowLimit"=0.0, "HighLimit"=0.0, "RValue"="", "RStatus"="", "RetVal"="0", "Units"="", "header1"="", "header2"="--- Start Switch Matrix 1A MUX A (ASIC 1) and Switch Matrix 1A MUX C (ASIC 2) Tests ---\r\r\r\r\r\r\r\r\r\r\r\r\r\r\r\r\r\r\r\r\r\r\r\r\r\r\r\r\r\r\r\r\r\r\r\r\r\r\r\r\r\r\r\r\r\r\r\r\r\r\r", "ExpectedValue"=""}, {"Test_Name"="469. CheckCFAdc \"PD3\" \"2.2\" \"2.65\"", "Step_Type"="NumericLimitTest", "LowLimit"=2.2, "HighLimit"=2.65, "RValue"="2.4509999752044678", "RStatus"="PASS", "RetVal"="0", "Units"="Volts", "header1"="", "header2"="--- Start Switch Matrix 1A MUX A (ASIC 1) and Switch Matrix 1A MUX C (ASIC 2) Tests ---\r\r\r\r\r\r\r\r\r\r\r\r\r\r\r\r\r\r\r\r\r\r\r\r\r\r\r\r\r\r\r\r\r\r\r\r\r\r\r\r\r\r\r\r\r\r\r\r\r\r\r\r", "ExpectedValue"=""}, {"Test_Name"="470. SelectAllMuxA \"1\" \"0\"", "Step_Type"="", "LowLimit"=0.0, "HighLimit"=0.0, "RValue"="", "RStatus"="", "RetVal"="0", "Units"="", "header1"="", "header2"="--- Start Switch Matrix 1A MUX A (ASIC 1) and Switch Matrix 1A MUX C (ASIC 2) Tests ---\r\r\r\r\r\r\r\r\r\r\r\r\r\r\r\r\r\r\r\r\r\r\r\r\r\r\r\r\r\r\r\r\r\r\r\r\r\r\r\r\r\r\r\r\r\r\r\r\r\r\r\r\r", "ExpectedValue"=""}, {"Test_Name"="471. SelectAllMuxA \"2\" \"0\"", "Step_Type"="", "LowLimit"=0.0, "HighLimit"=0.0, "RValue"="", "RStatus"="", "RetVal"="0", "Units"="", "header1"="", "header2"="--- Start Switch Matrix 1A MUX A (ASIC 1) and Switch Matrix 1A MUX C (ASIC 2) Tests ---\r\r\r\r\r\r\r\r\r\r\r\r\r\r\r\r\r\r\r\r\r\r\r\r\r\r\r\r\r\r\r\r\r\r\r\r\r\r\r\r\r\r\r\r\r\r\r\r\r\r\r\r\r\r", "ExpectedValue"=""}, {"Test_Name"="473. SelectMuxA \"1\" \"12\" \"1\"", "Step_Type"="", "LowLimit"=0.0, "HighLimit"=0.0, "RValue"="", "RStatus"="", "RetVal"="0", "Units"="", "header1"="", "header2"="--- Start Switch Matrix 1A MUX A (ASIC 1) and Switch Matrix 1A MUX C (ASIC 2) Tests ---\r\r\r\r\r\r\r\r\r\r\r\r\r\r\r\r\r\r\r\r\r\r\r\r\r\r\r\r\r\r\r\r\r\r\r\r\r\r\r\r\r\r\r\r\r\r\r\r\r\r\r\r\r\r\r", "ExpectedValue"=""}, {"Test_Name"="474. SelectMuxA \"2\" \"12\" \"1\"", "Step_Type"="", "LowLimit"=0.0, "HighLimit"=0.0, "RValue"="", "RStatus"="", "RetVal"="0", "Units"="", "header1"="", "header2"="--- Start Switch Matrix 1A MUX A (ASIC 1) and Switch Matrix 1A MUX C (ASIC 2) Tests ---\r\r\r\r\r\r\r\r\r\r\r\r\r\r\r\r\r\r\r\r\r\r\r\r\r\r\r\r\r\r\r\r\r\r\r\r\r\r\r\r\r\r\r\r\r\r\r\r\r\r\r\r\r\r\r\r", "ExpectedValue"=""}, {"Test_Name"="475. CheckCFAdc \"PD3\" \"2.2\" \"2.65\"", "Step_Type"="NumericLimitTest", "LowLimit"=2.2, "HighLimit"=2.65, "RValue"="2.4509999752044678", "RStatus"="PASS", "RetVal"="0", "Units"="Volts", "header1"="", "header2"="--- Start Switch Matrix 1A MUX A (ASIC 1) and Switch Matrix 1A MUX C (ASIC 2) Tests ---\r\r\r\r\r\r\r\r\r\r\r\r\r\r\r\r\r\r\r\r\r\r\r\r\r\r\r\r\r\r\r\r\r\r\r\r\r\r\r\r\r\r\r\r\r\r\r\r\r\r\r\r\r\r\r\r\r", "ExpectedValue"=""}, {"Test_Name"="476. SelectAllMuxA \"1\" \"0\"", "Step_Type"="", "LowLimit"=0.0, "HighLimit"=0.0, "RValue"="", "RStatus"="", "RetVal"="0", "Units"="", "header1"="", "header2"="--- Start Switch Matrix 1A MUX A (ASIC 1) and Switch Matrix 1A MUX C (ASIC 2) Tests ---\r\r\r\r\r\r\r\r\r\r\r\r\r\r\r\r\r\r\r\r\r\r\r\r\r\r\r\r\r\r\r\r\r\r\r\r\r\r\r\r\r\r\r\r\r\r\r\r\r\r\r\r\r\r\r\r\r\r", "ExpectedValue"=""}, {"Test_Name"="477. SelectAllMuxA \"2\" \"0\"", "Step_Type"="", "LowLimit"=0.0, "HighLimit"=0.0, "RValue"="", "RStatus"="", "RetVal"="0", "Units"="", "header1"="", "header2"="--- Start Switch Matrix 1A MUX A (ASIC 1) and Switch Matrix 1A MUX C (ASIC 2) Tests ---\r\r\r\r\r\r\r\r\r\r\r\r\r\r\r\r\r\r\r\r\r\r\r\r\r\r\r\r\r\r\r\r\r\r\r\r\r\r\r\r\r\r\r\r\r\r\r\r\r\r\r\r\r\r\r\r\r\r\r", "ExpectedValue"=""}, {"Test_Name"="479. SelectMuxA \"1\" \"13\" \"1\"", "Step_Type"="", "LowLimit"=0.0, "HighLimit"=0.0, "RValue"="", "RStatus"="", "RetVal"="0", "Units"="", "header1"="", "header2"="--- Start Switch Matrix 1A MUX A (ASIC 1) and Switch Matrix 1A MUX C (ASIC 2) Tests ---\r\r\r\r\r\r\r\r\r\r\r\r\r\r\r\r\r\r\r\r\r\r\r\r\r\r\r\r\r\r\r\r\r\r\r\r\r\r\r\r\r\r\r\r\r\r\r\r\r\r\r\r\r\r\r\r\r\r\r\r", "ExpectedValue"=""}, {"Test_Name"="480. SelectMuxA \"2\" \"13\" \"1\"", "Step_Type"="", "LowLimit"=0.0, "HighLimit"=0.0, "RValue"="", "RStatus"="", "RetVal"="0", "Units"="", "header1"="", "header2"="--- Start Switch Matrix 1A MUX A (ASIC 1) and Switch Matrix 1A MUX C (ASIC 2) Tests ---\r\r\r\r\r\r\r\r\r\r\r\r\r\r\r\r\r\r\r\r\r\r\r\r\r\r\r\r\r\r\r\r\r\r\r\r\r\r\r\r\r\r\r\r\r\r\r\r\r\r\r\r\r\r\r\r\r\r\r\r\r", "ExpectedValue"=""}, {"Test_Name"="481. CheckCFAdc \"PD3\" \"2.2\" \"2.65\"", "Step_Type"="NumericLimitTest", "LowLimit"=2.2, "HighLimit"=2.65, "RValue"="2.440999984741211", "RStatus"="PASS", "RetVal"="0", "Units"="Volts", "header1"="", "header2"="--- Start Switch Matrix 1A MUX A (ASIC 1) and Switch Matrix 1A MUX C (ASIC 2) Tests ---\r\r\r\r\r\r\r\r\r\r\r\r\r\r\r\r\r\r\r\r\r\r\r\r\r\r\r\r\r\r\r\r\r\r\r\r\r\r\r\r\r\r\r\r\r\r\r\r\r\r\r\r\r\r\r\r\r\r\r\r\r\r", "ExpectedValue"=""}, {"Test_Name"="482. SelectAllMuxA \"1\" \"0\"", "Step_Type"="", "LowLimit"=0.0, "HighLimit"=0.0, "RValue"="", "RStatus"="", "RetVal"="0", "Units"="", "header1"="", "header2"="--- Start Switch Matrix 1A MUX A (ASIC 1) and Switch Matrix 1A MUX C (ASIC 2) Tests ---\r\r\r\r\r\r\r\r\r\r\r\r\r\r\r\r\r\r\r\r\r\r\r\r\r\r\r\r\r\r\r\r\r\r\r\r\r\r\r\r\r\r\r\r\r\r\r\r\r\r\r\r\r\r\r\r\r\r\r\r\r\r\r", "ExpectedValue"=""}, {"Test_Name"="483. SelectAllMuxA \"2\" \"0\"", "Step_Type"="", "LowLimit"=0.0, "HighLimit"=0.0, "RValue"="", "RStatus"="", "RetVal"="0", "Units"="", "header1"="", "header2"="--- Start Switch Matrix 1A MUX A (ASIC 1) and Switch Matrix 1A MUX C (ASIC 2) Tests ---\r\r\r\r\r\r\r\r\r\r\r\r\r\r\r\r\r\r\r\r\r\r\r\r\r\r\r\r\r\r\r\r\r\r\r\r\r\r\r\r\r\r\r\r\r\r\r\r\r\r\r\r\r\r\r\r\r\r\r\r\r\r\r\r", "ExpectedValue"=""}, {"Test_Name"="485. SelectMuxA \"1\" \"14\" \"1\"", "Step_Type"="", "LowLimit"=0.0, "HighLimit"=0.0, "RValue"="", "RStatus"="", "RetVal"="0", "Units"="", "header1"="", "header2"="--- Start Switch Matrix 1A MUX A (ASIC 1) and Switch Matrix 1A MUX C (ASIC 2) Tests ---\r\r\r\r\r\r\r\r\r\r\r\r\r\r\r\r\r\r\r\r\r\r\r\r\r\r\r\r\r\r\r\r\r\r\r\r\r\r\r\r\r\r\r\r\r\r\r\r\r\r\r\r\r\r\r\r\r\r\r\r\r\r\r\r\r", "ExpectedValue"=""}, {"Test_Name"="486. SelectMuxA \"2\" \"14\" \"1\"", "Step_Type"="", "LowLimit"=0.0, "HighLimit"=0.0, "RValue"="", "RStatus"="", "RetVal"="0", "Units"="", "header1"="", "header2"="--- Start Switch Matrix 1A MUX A (ASIC 1) and Switch Matrix 1A MUX C (ASIC 2) Tests ---\r\r\r\r\r\r\r\r\r\r\r\r\r\r\r\r\r\r\r\r\r\r\r\r\r\r\r\r\r\r\r\r\r\r\r\r\r\r\r\r\r\r\r\r\r\r\r\r\r\r\r\r\r\r\r\r\r\r\r\r\r\r\r\r\r\r", "ExpectedValue"=""}, {"Test_Name"="487. CheckCFAdc \"PD3\" \"2.2\" \"2.65\"", "Step_Type"="NumericLimitTest", "LowLimit"=2.2, "HighLimit"=2.65, "RValue"="2.4509999752044678", "RStatus"="PASS", "RetVal"="0", "Units"="Volts", "header1"="", "header2"="--- Start Switch Matrix 1A MUX A (ASIC 1) and Switch Matrix 1A MUX C (ASIC 2) Tests ---\r\r\r\r\r\r\r\r\r\r\r\r\r\r\r\r\r\r\r\r\r\r\r\r\r\r\r\r\r\r\r\r\r\r\r\r\r\r\r\r\r\r\r\r\r\r\r\r\r\r\r\r\r\r\r\r\r\r\r\r\r\r\r\r\r\r\r", "ExpectedValue"=""}, {"Test_Name"="488. SelectAllMuxA \"1\" \"0\"", "Step_Type"="", "LowLimit"=0.0, "HighLimit"=0.0, "RValue"="", "RStatus"="", "RetVal"="0", "Units"="", "header1"="", "header2"="--- Start Switch Matrix 1A MUX A (ASIC 1) and Switch Matrix 1A MUX C (ASIC 2) Tests ---\r\r\r\r\r\r\r\r\r\r\r\r\r\r\r\r\r\r\r\r\r\r\r\r\r\r\r\r\r\r\r\r\r\r\r\r\r\r\r\r\r\r\r\r\r\r\r\r\r\r\r\r\r\r\r\r\r\r\r\r\r\r\r\r\r\r\r\r", "ExpectedValue"=""}, {"Test_Name"="489. SelectAllMuxA \"2\" \"0\"", "Step_Type"="", "LowLimit"=0.0, "HighLimit"=0.0, "RValue"="", "RStatus"="", "RetVal"="0", "Units"="", "header1"="", "header2"="--- Start Switch Matrix 1A MUX A (ASIC 1) and Switch Matrix 1A MUX C (ASIC 2) Tests ---\r\r\r\r\r\r\r\r\r\r\r\r\r\r\r\r\r\r\r\r\r\r\r\r\r\r\r\r\r\r\r\r\r\r\r\r\r\r\r\r\r\r\r\r\r\r\r\r\r\r\r\r\r\r\r\r\r\r\r\r\r\r\r\r\r\r\r\r\r", "ExpectedValue"=""}, {"Test_Name"="491. SelectMuxA \"1\" \"15\" \"1\"", "Step_Type"="", "LowLimit"=0.0, "HighLimit"=0.0, "RValue"="", "RStatus"="", "RetVal"="0", "Units"="", "header1"="", "header2"="--- Start Switch Matrix 1A MUX A (ASIC 1) and Switch Matrix 1A MUX C (ASIC 2) Tests ---\r\r\r\r\r\r\r\r\r\r\r\r\r\r\r\r\r\r\r\r\r\r\r\r\r\r\r\r\r\r\r\r\r\r\r\r\r\r\r\r\r\r\r\r\r\r\r\r\r\r\r\r\r\r\r\r\r\r\r\r\r\r\r\r\r\r\r\r\r\r", "ExpectedValue"=""}, {"Test_Name"="492. SelectMuxA \"2\" \"15\" \"1\"", "Step_Type"="", "LowLimit"=0.0, "HighLimit"=0.0, "RValue"="", "RStatus"="", "RetVal"="0", "Units"="", "header1"="", "header2"="--- Start Switch Matrix 1A MUX A (ASIC 1) and Switch Matrix 1A MUX C (ASIC 2) Tests ---\r\r\r\r\r\r\r\r\r\r\r\r\r\r\r\r\r\r\r\r\r\r\r\r\r\r\r\r\r\r\r\r\r\r\r\r\r\r\r\r\r\r\r\r\r\r\r\r\r\r\r\r\r\r\r\r\r\r\r\r\r\r\r\r\r\r\r\r\r\r\r", "ExpectedValue"=""}, {"Test_Name"="493. CheckCFAdc \"PD3\" \"2.2\" \"2.65\"", "Step_Type"="NumericLimitTest", "LowLimit"=2.2, "HighLimit"=2.65, "RValue"="2.431999921798706", "RStatus"="PASS", "RetVal"="0", "Units"="Volts", "header1"="", "header2"="--- Start Switch Matrix 1A MUX A (ASIC 1) and Switch Matrix 1A MUX C (ASIC 2) Tests ---\r\r\r\r\r\r\r\r\r\r\r\r\r\r\r\r\r\r\r\r\r\r\r\r\r\r\r\r\r\r\r\r\r\r\r\r\r\r\r\r\r\r\r\r\r\r\r\r\r\r\r\r\r\r\r\r\r\r\r\r\r\r\r\r\r\r\r\r\r\r\r\r", "ExpectedValue"=""}, {"Test_Name"="494. SelectAllMuxA \"1\" \"0\"", "Step_Type"="", "LowLimit"=0.0, "HighLimit"=0.0, "RValue"="", "RStatus"="", "RetVal"="0", "Units"="", "header1"="", "header2"="--- Start Switch Matrix 1A MUX A (ASIC 1) and Switch Matrix 1A MUX C (ASIC 2) Tests ---\r\r\r\r\r\r\r\r\r\r\r\r\r\r\r\r\r\r\r\r\r\r\r\r\r\r\r\r\r\r\r\r\r\r\r\r\r\r\r\r\r\r\r\r\r\r\r\r\r\r\r\r\r\r\r\r\r\r\r\r\r\r\r\r\r\r\r\r\r\r\r\r\r", "ExpectedValue"=""}, {"Test_Name"="495. SelectAllMuxA \"2\" \"0\"", "Step_Type"="", "LowLimit"=0.0, "HighLimit"=0.0, "RValue"="", "RStatus"="", "RetVal"="0", "Units"="", "header1"="", "header2"="--- Start Switch Matrix 1A MUX A (ASIC 1) and Switch Matrix 1A MUX C (ASIC 2) Tests ---\r\r\r\r\r\r\r\r\r\r\r\r\r\r\r\r\r\r\r\r\r\r\r\r\r\r\r\r\r\r\r\r\r\r\r\r\r\r\r\r\r\r\r\r\r\r\r\r\r\r\r\r\r\r\r\r\r\r\r\r\r\r\r\r\r\r\r\r\r\r\r\r\r\r", "ExpectedValue"=""}, {"Test_Name"="497. SetG15PullUp \"A\" \"0\"", "Step_Type"="", "LowLimit"=0.0, "HighLimit"=0.0, "RValue"="", "RStatus"="", "RetVal"="0", "Units"="", "header1"="", "header2"="--- Start Switch Matrix 1A MUX A (ASIC 1) and Switch Matrix 1A MUX C (ASIC 2) Tests ---\r\r\r\r\r\r\r\r\r\r\r\r\r\r\r\r\r\r\r\r\r\r\r\r\r\r\r\r\r\r\r\r\r\r\r\r\r\r\r\r\r\r\r\r\r\r\r\r\r\r\r\r\r\r\r\r\r\r\r\r\r\r\r\r\r\r\r\r\r\r\r\r\r\r\r", "ExpectedValue"=""}, {"Test_Name"="498. SetG15PullUp \"C\" \"0\"", "Step_Type"="", "LowLimit"=0.0, "HighLimit"=0.0, "RValue"="", "RStatus"="", "RetVal"="0", "Units"="", "header1"="", "header2"="--- Start Switch Matrix 1A MUX A (ASIC 1) and Switch Matrix 1A MUX C (ASIC 2) Tests ---\r\r\r\r\r\r\r\r\r\r\r\r\r\r\r\r\r\r\r\r\r\r\r\r\r\r\r\r\r\r\r\r\r\r\r\r\r\r\r\r\r\r\r\r\r\r\r\r\r\r\r\r\r\r\r\r\r\r\r\r\r\r\r\r\r\r\r\r\r\r\r\r\r\r\r\r", "ExpectedValue"=""}, {"Test_Name"="499. SetG15PullDown \"A\" \"0\"", "Step_Type"="", "LowLimit"=0.0, "HighLimit"=0.0, "RValue"="", "RStatus"="", "RetVal"="0", "Units"="", "header1"="", "header2"="--- Start Switch Matrix 1A MUX A (ASIC 1) and Switch Matrix 1A MUX C (ASIC 2) Tests ---\r\r\r\r\r\r\r\r\r\r\r\r\r\r\r\r\r\r\r\r\r\r\r\r\r\r\r\r\r\r\r\r\r\r\r\r\r\r\r\r\r\r\r\r\r\r\r\r\r\r\r\r\r\r\r\r\r\r\r\r\r\r\r\r\r\r\r\r\r\r\r\r\r\r\r\r\r", "ExpectedValue"=""}, {"Test_Name"="500. SetG15PullDown \"C\" \"0\"", "Step_Type"="", "LowLimit"=0.0, "HighLimit"=0.0, "RValue"="", "RStatus"="", "RetVal"="0", "Units"="", "header1"="", "header2"="--- Start Switch Matrix 1A MUX A (ASIC 1) and Switch Matrix 1A MUX C (ASIC 2) Tests ---\r\r\r\r\r\r\r\r\r\r\r\r\r\r\r\r\r\r\r\r\r\r\r\r\r\r\r\r\r\r\r\r\r\r\r\r\r\r\r\r\r\r\r\r\r\r\r\r\r\r\r\r\r\r\r\r\r\r\r\r\r\r\r\r\r\r\r\r\r\r\r\r\r\r\r\r\r\r", "ExpectedValue"=""}, {"Test_Name"="503.  --- CCD Termination Tests  SW3 in Asic---", "Step_Type"="", "LowLimit"=0.0, "HighLimit"=0.0, "RValue"="", "RStatus"="", "RetVal"="", "Units"="", "header1"="", "header2"="--- CCD Termination Tests  SW3 in Asic---\r", "ExpectedValue"=""}, {"Test_Name"="504. SetAsicRegister \"1\" \"7\" \"0C\"", "Step_Type"="", "LowLimit"=0.0, "HighLimit"=0.0, "RValue"="", "RStatus"="", "RetVal"="0", "Units"="", "header1"="", "header2"="--- CCD Termination Tests  SW3 in Asic---\r\r", "ExpectedValue"=""}, {"Test_Name"="505. CheckCFAdc \"PD1\" \"2.3\" \"2.7\"", "Step_Type"="NumericLimitTest", "LowLimit"=2.3, "HighLimit"=2.7, "RValue"="2.51200008392334", "RStatus"="PASS", "RetVal"="0", "Units"="Volts", "header1"="", "header2"="--- CCD Termination Tests  SW3 in Asic---\r\r\r", "ExpectedValue"=""}, {"Test_Name"="506. CheckCFAdc \"PD2\" \"2.3\" \"2.7\"", "Step_Type"="NumericLimitTest", "LowLimit"=2.3, "HighLimit"=2.7, "RValue"="2.5380001068115234", "RStatus"="PASS", "RetVal"="0", "Units"="Volts", "header1"="", "header2"="--- CCD Termination Tests  SW3 in Asic---\r\r\r\r", "ExpectedValue"=""}, {"Test_Name"="507. SetAsicRegister \"1\" \"7\" \"0\"", "Step_Type"="", "LowLimit"=0.0, "HighLimit"=0.0, "RValue"="", "RStatus"="", "RetVal"="0", "Units"="", "header1"="", "header2"="--- CCD Termination Tests  SW3 in Asic---\r\r\r\r\r", "ExpectedValue"=""}, {"Test_Name"="509.  ---VCOMM and MUX 2A & 2B and Internal J1850 and CAN 1 transciever Rx---", "Step_Type"="", "LowLimit"=0.0, "HighLimit"=0.0, "RValue"="", "RStatus"="", "RetVal"="", "Units"="", "header1"="", "header2"="---VCOMM and MUX 2A & 2B and Internal J1850 and CAN 1 transciever Rx---\r", "ExpectedValue"=""}, {"Test_Name"="511. SetFpgaRegister \"89E\" \"40\"", "Step_Type"="", "LowLimit"=0.0, "HighLimit"=0.0, "RValue"="", "RStatus"="", "RetVal"="0", "Units"="", "header1"="", "header2"="---VCOMM and MUX 2A & 2B and Internal J1850 and CAN 1 transciever Rx---\r\r", "ExpectedValue"=""}, {"Test_Name"="512. SetFpgaRegister \"959\" \"02\"", "Step_Type"="", "LowLimit"=0.0, "HighLimit"=0.0, "RValue"="", "RStatus"="", "RetVal"="0", "Units"="", "header1"="", "header2"="---VCOMM and MUX 2A & 2B and Internal J1850 and CAN 1 transciever Rx---\r\r\r", "ExpectedValue"=""}, {"Test_Name"="513. SetAsicRegister \"1\" \"0\" \"80\"", "Step_Type"="", "LowLimit"=0.0, "HighLimit"=0.0, "RValue"="", "RStatus"="", "RetVal"="0", "Units"="", "header1"="", "header2"="---VCOMM and MUX 2A & 2B and Internal J1850 and CAN 1 transciever Rx---\r\r\r\r", "ExpectedValue"=""}, {"Test_Name"="514. SetAsicRegister \"1\" \"2\" \"80\"", "Step_Type"="", "LowLimit"=0.0, "HighLimit"=0.0, "RValue"="", "RStatus"="", "RetVal"="0", "Units"="", "header1"="", "header2"="---VCOMM and MUX 2A & 2B and Internal J1850 and CAN 1 transciever Rx---\r\r\r\r\r", "ExpectedValue"=""}, {"Test_Name"="516. CheckCFAdc \"PD1\" \"-.15\" \".3\"", "Step_Type"="NumericLimitTest", "LowLimit"=-0.15, "HighLimit"=0.3, "RValue"="0.027000000700354576", "RStatus"="PASS", "RetVal"="0", "Units"="Volts", "header1"="", "header2"="---VCOMM and MUX 2A & 2B and Internal J1850 and CAN 1 transciever Rx---\r\r\r\r\r\r", "ExpectedValue"=""}, {"Test_Name"="517. CheckCFAdc \"PD2\" \"7.2\" \"8\"", "Step_Type"="NumericLimitTest", "LowLimit"=7.2, "HighLimit"=8.0, "RValue"="7.577000141143799", "RStatus"="PASS", "RetVal"="0", "Units"="Volts", "header1"="", "header2"="---VCOMM and MUX 2A & 2B and Internal J1850 and CAN 1 transciever Rx---\r\r\r\r\r\r\r", "ExpectedValue"=""}, {"Test_Name"="519. SetAsicRegister \"1\" \"4\" \"08\"", "Step_Type"="", "LowLimit"=0.0, "HighLimit"=0.0, "RValue"="", "RStatus"="", "RetVal"="0", "Units"="", "header1"="", "header2"="---VCOMM and MUX 2A & 2B and Internal J1850 and CAN 1 transciever Rx---\r\r\r\r\r\r\r\r", "ExpectedValue"=""}, {"Test_Name"="520. CheckCFAdc \"PD1\" \"3.35\" \"3.85\"", "Step_Type"="NumericLimitTest", "LowLimit"=3.35, "HighLimit"=3.85, "RValue"="3.630000114440918", "RStatus"="PASS", "RetVal"="0", "Units"="Volts", "header1"="", "header2"="---VCOMM and MUX 2A & 2B and Internal J1850 and CAN 1 transciever Rx---\r\r\r\r\r\r\r\r\r", "ExpectedValue"=""}, {"Test_Name"="521. CheckCFAdc \"PD2\" \"7.2\" \"8.0\"", "Step_Type"="NumericLimitTest", "LowLimit"=7.2, "HighLimit"=8.0, "RValue"="7.585999965667725", "RStatus"="PASS", "RetVal"="0", "Units"="Volts", "header1"="", "header2"="---VCOMM and MUX 2A & 2B and Internal J1850 and CAN 1 transciever Rx---\r\r\r\r\r\r\r\r\r\r", "ExpectedValue"=""}, {"Test_Name"="522. CheckFpgaRegister \"984\" \"1\" \"0\"", "Step_Type"="StringValueTest", "LowLimit"=0.0, "HighLimit"=0.0, "RValue"="0", "RStatus"="PASS", "RetVal"="0", "Units"="", "header1"="", "header2"="---VCOMM and MUX 2A & 2B and Internal J1850 and CAN 1 transciever Rx---\r\r\r\r\r\r\r\r\r\r\r", "ExpectedValue"=""}, {"Test_Name"="523. SetAsicRegister \"1\" \"4\" \"04\"", "Step_Type"="", "LowLimit"=0.0, "HighLimit"=0.0, "RValue"="", "RStatus"="", "RetVal"="0", "Units"="", "header1"="", "header2"="---VCOMM and MUX 2A & 2B and Internal J1850 and CAN 1 transciever Rx---\r\r\r\r\r\r\r\r\r\r\r\r", "ExpectedValue"=""}, {"Test_Name"="524. CheckCFAdc \"PD1\" \"-.15\" \".3\"", "Step_Type"="NumericLimitTest", "LowLimit"=-0.15, "HighLimit"=0.3, "RValue"="0.035999998450279236", "RStatus"="PASS", "RetVal"="0", "Units"="Volts", "header1"="", "header2"="---VCOMM and MUX 2A & 2B and Internal J1850 and CAN 1 transciever Rx---\r\r\r\r\r\r\r\r\r\r\r\r\r", "ExpectedValue"=""}, {"Test_Name"="525. CheckCFAdc \"PD2\" \"3.5\" \"3.95\"", "Step_Type"="NumericLimitTest", "LowLimit"=3.5, "HighLimit"=3.95, "RValue"="3.7100000381469727", "RStatus"="PASS", "RetVal"="0", "Units"="Volts", "header1"="", "header2"="---VCOMM and MUX 2A & 2B and Internal J1850 and CAN 1 transciever Rx---\r\r\r\r\r\r\r\r\r\r\r\r\r\r", "ExpectedValue"=""}, {"Test_Name"="527. SetG15PullUp \"A\" \"1\"", "Step_Type"="", "LowLimit"=0.0, "HighLimit"=0.0, "RValue"="", "RStatus"="", "RetVal"="0", "Units"="", "header1"="", "header2"="---VCOMM and MUX 2A & 2B and Internal J1850 and CAN 1 transciever Rx---\r\r\r\r\r\r\r\r\r\r\r\r\r\r\r", "ExpectedValue"=""}, {"Test_Name"="528. CheckCFAdc \"PD1\" \"4.3\" \"4.9\"", "Step_Type"="NumericLimitTest", "LowLimit"=4.3, "HighLimit"=4.9, "RValue"="4.609000205993652", "RStatus"="PASS", "RetVal"="0", "Units"="Volts", "header1"="", "header2"="---VCOMM and MUX 2A & 2B and Internal J1850 and CAN 1 transciever Rx---\r\r\r\r\r\r\r\r\r\r\r\r\r\r\r\r", "ExpectedValue"=""}, {"Test_Name"="529. CheckCFAdc \"PD2\" \"3.5\" \"3.9\"", "Step_Type"="NumericLimitTest", "LowLimit"=3.5, "HighLimit"=3.9, "RValue"="3.7100000381469727", "RStatus"="PASS", "RetVal"="0", "Units"="Volts", "header1"="", "header2"="---VCOMM and MUX 2A & 2B and Internal J1850 and CAN 1 transciever Rx---\r\r\r\r\r\r\r\r\r\r\r\r\r\r\r\r\r", "ExpectedValue"=""}, {"Test_Name"="530. CheckFpgaRegister \"984\" \"1\" \"1\"", "Step_Type"="StringValueTest", "LowLimit"=0.0, "HighLimit"=0.0, "RValue"="2", "RStatus"="PASS", "RetVal"="0", "Units"="", "header1"="", "header2"="---VCOMM and MUX 2A & 2B and Internal J1850 and CAN 1 transciever Rx---\r\r\r\r\r\r\r\r\r\r\r\r\r\r\r\r\r\r", "ExpectedValue"=""}, {"Test_Name"="532. SetAsicRegister \"1\" \"7\" \"10\"", "Step_Type"="", "LowLimit"=0.0, "HighLimit"=0.0, "RValue"="", "RStatus"="", "RetVal"="0", "Units"="", "header1"="", "header2"="---VCOMM and MUX 2A & 2B and Internal J1850 and CAN 1 transciever Rx---\r\r\r\r\r\r\r\r\r\r\r\r\r\r\r\r\r\r\r", "ExpectedValue"=""}, {"Test_Name"="533. CheckFpgaRegister \"984\" \"1\" \"0\"", "Step_Type"="StringValueTest", "LowLimit"=0.0, "HighLimit"=0.0, "RValue"="0", "RStatus"="PASS", "RetVal"="0", "Units"="", "header1"="", "header2"="---VCOMM and MUX 2A & 2B and Internal J1850 and CAN 1 transciever Rx---\r\r\r\r\r\r\r\r\r\r\r\r\r\r\r\r\r\r\r\r", "ExpectedValue"=""}, {"Test_Name"="534. SetAsicRegister \"1\" \"7\" \"00\"", "Step_Type"="", "LowLimit"=0.0, "HighLimit"=0.0, "RValue"="", "RStatus"="", "RetVal"="0", "Units"="", "header1"="", "header2"="---VCOMM and MUX 2A & 2B and Internal J1850 and CAN 1 transciever Rx---\r\r\r\r\r\r\r\r\r\r\r\r\r\r\r\r\r\r\r\r\r", "ExpectedValue"=""}, {"Test_Name"="535. CheckFpgaRegister \"984\" \"1\" \"1\"", "Step_Type"="StringValueTest", "LowLimit"=0.0, "HighLimit"=0.0, "RValue"="2", "RStatus"="PASS", "RetVal"="0", "Units"="", "header1"="", "header2"="---VCOMM and MUX 2A & 2B and Internal J1850 and CAN 1 transciever Rx---\r\r\r\r\r\r\r\r\r\r\r\r\r\r\r\r\r\r\r\r\r\r", "ExpectedValue"=""}, {"Test_Name"="536. SetAsicRegister \"1\" \"4\" \"00\"", "Step_Type"="", "LowLimit"=0.0, "HighLimit"=0.0, "RValue"="", "RStatus"="", "RetVal"="0", "Units"="", "header1"="", "header2"="---VCOMM and MUX 2A & 2B and Internal J1850 and CAN 1 transciever Rx---\r\r\r\r\r\r\r\r\r\r\r\r\r\r\r\r\r\r\r\r\r\r\r", "ExpectedValue"=""}, {"Test_Name"="537. SetG15PullUp \"A\" \"0\"", "Step_Type"="", "LowLimit"=0.0, "HighLimit"=0.0, "RValue"="", "RStatus"="", "RetVal"="0", "Units"="", "header1"="", "header2"="---VCOMM and MUX 2A & 2B and Internal J1850 and CAN 1 transciever Rx---\r\r\r\r\r\r\r\r\r\r\r\r\r\r\r\r\r\r\r\r\r\r\r\r", "ExpectedValue"=""}, {"Test_Name"="538. CheckFpgaRegister \"984\" \"1\" \"0\"", "Step_Type"="StringValueTest", "LowLimit"=0.0, "HighLimit"=0.0, "RValue"="0", "RStatus"="PASS", "RetVal"="0", "Units"="", "header1"="", "header2"="---VCOMM and MUX 2A & 2B and Internal J1850 and CAN 1 transciever Rx---\r\r\r\r\r\r\r\r\r\r\r\r\r\r\r\r\r\r\r\r\r\r\r\r\r", "ExpectedValue"=""}, {"Test_Name"="539. SetFpgaRegister \"983\" \"4\"", "Step_Type"="", "LowLimit"=0.0, "HighLimit"=0.0, "RValue"="", "RStatus"="", "RetVal"="0", "Units"="", "header1"="", "header2"="---VCOMM and MUX 2A & 2B and Internal J1850 and CAN 1 transciever Rx---\r\r\r\r\r\r\r\r\r\r\r\r\r\r\r\r\r\r\r\r\r\r\r\r\r\r", "ExpectedValue"=""}, {"Test_Name"="541. CheckCFAdc \"PD1\" \"7.4\" \"8.3\"", "Step_Type"="NumericLimitTest", "LowLimit"=7.4, "HighLimit"=8.3, "RValue"="7.869999885559082", "RStatus"="PASS", "RetVal"="0", "Units"="Volts", "header1"="", "header2"="---VCOMM and MUX 2A & 2B and Internal J1850 and CAN 1 transciever Rx---\r\r\r\r\r\r\r\r\r\r\r\r\r\r\r\r\r\r\r\r\r\r\r\r\r\r\r", "ExpectedValue"=""}, {"Test_Name"="542. CheckCFAdc \"PD2\" \"-.15\" \".3\"", "Step_Type"="NumericLimitTest", "LowLimit"=-0.15, "HighLimit"=0.3, "RValue"="0.017999999225139618", "RStatus"="PASS", "RetVal"="0", "Units"="Volts", "header1"="", "header2"="---VCOMM and MUX 2A & 2B and Internal J1850 and CAN 1 transciever Rx---\r\r\r\r\r\r\r\r\r\r\r\r\r\r\r\r\r\r\r\r\r\r\r\r\r\r\r\r", "ExpectedValue"=""}, {"Test_Name"="543. SetAsicRegister \"1\" \"4\" \"02\"", "Step_Type"="", "LowLimit"=0.0, "HighLimit"=0.0, "RValue"="", "RStatus"="", "RetVal"="0", "Units"="", "header1"="", "header2"="---VCOMM and MUX 2A & 2B and Internal J1850 and CAN 1 transciever Rx---\r\r\r\r\r\r\r\r\r\r\r\r\r\r\r\r\r\r\r\r\r\r\r\r\r\r\r\r\r", "ExpectedValue"=""}, {"Test_Name"="544. CheckCFAdc \"PD1\" \"-.15\" \".3\"", "Step_Type"="NumericLimitTest", "LowLimit"=-0.15, "HighLimit"=0.3, "RValue"="0.035999998450279236", "RStatus"="PASS", "RetVal"="0", "Units"="Volts", "header1"="", "header2"="---VCOMM and MUX 2A & 2B and Internal J1850 and CAN 1 transciever Rx---\r\r\r\r\r\r\r\r\r\r\r\r\r\r\r\r\r\r\r\r\r\r\r\r\r\r\r\r\r\r", "ExpectedValue"=""}, {"Test_Name"="545. CheckCFAdc \"PD2\" \"-.15\" \".3\"", "Step_Type"="NumericLimitTest", "LowLimit"=-0.15, "HighLimit"=0.3, "RValue"="0.017999999225139618", "RStatus"="PASS", "RetVal"="0", "Units"="Volts", "header1"="", "header2"="---VCOMM and MUX 2A & 2B and Internal J1850 and CAN 1 transciever Rx---\r\r\r\r\r\r\r\r\r\r\r\r\r\r\r\r\r\r\r\r\r\r\r\r\r\r\r\r\r\r\r", "ExpectedValue"=""}, {"Test_Name"="546. SetAsicRegister \"1\" \"4\" \"01\"", "Step_Type"="", "LowLimit"=0.0, "HighLimit"=0.0, "RValue"="", "RStatus"="", "RetVal"="0", "Units"="", "header1"="", "header2"="---VCOMM and MUX 2A & 2B and Internal J1850 and CAN 1 transciever Rx---\r\r\r\r\r\r\r\r\r\r\r\r\r\r\r\r\r\r\r\r\r\r\r\r\r\r\r\r\r\r\r\r", "ExpectedValue"=""}, {"Test_Name"="547. CheckCFAdc \"PD1\" \"7.4\" \"8.3\"", "Step_Type"="NumericLimitTest", "LowLimit"=7.4, "HighLimit"=8.3, "RValue"="7.869999885559082", "RStatus"="PASS", "RetVal"="0", "Units"="Volts", "header1"="", "header2"="---VCOMM and MUX 2A & 2B and Internal J1850 and CAN 1 transciever Rx---\r\r\r\r\r\r\r\r\r\r\r\r\r\r\r\r\r\r\r\r\r\r\r\r\r\r\r\r\r\r\r\r\r", "ExpectedValue"=""}, {"Test_Name"="548. CheckCFAdc \"PD2\" \"7.2\" \"8.0\"", "Step_Type"="NumericLimitTest", "LowLimit"=7.2, "HighLimit"=8.0, "RValue"="7.585999965667725", "RStatus"="PASS", "RetVal"="0", "Units"="Volts", "header1"="", "header2"="---VCOMM and MUX 2A & 2B and Internal J1850 and CAN 1 transciever Rx---\r\r\r\r\r\r\r\r\r\r\r\r\r\r\r\r\r\r\r\r\r\r\r\r\r\r\r\r\r\r\r\r\r\r", "ExpectedValue"=""}, {"Test_Name"="549. SetFpgaRegister \"983\" \"00\"", "Step_Type"="", "LowLimit"=0.0, "HighLimit"=0.0, "RValue"="", "RStatus"="", "RetVal"="0", "Units"="", "header1"="", "header2"="---VCOMM and MUX 2A & 2B and Internal J1850 and CAN 1 transciever Rx---\r\r\r\r\r\r\r\r\r\r\r\r\r\r\r\r\r\r\r\r\r\r\r\r\r\r\r\r\r\r\r\r\r\r\r", "ExpectedValue"=""}, {"Test_Name"="550. CheckCFAdc \"PD1\" \"-.15\" \".3\"", "Step_Type"="NumericLimitTest", "LowLimit"=-0.15, "HighLimit"=0.3, "RValue"="0.035999998450279236", "RStatus"="PASS", "RetVal"="0", "Units"="Volts", "header1"="", "header2"="---VCOMM and MUX 2A & 2B and Internal J1850 and CAN 1 transciever Rx---\r\r\r\r\r\r\r\r\r\r\r\r\r\r\r\r\r\r\r\r\r\r\r\r\r\r\r\r\r\r\r\r\r\r\r\r", "ExpectedValue"=""}, {"Test_Name"="551. CheckCFAdc \"PD2\" \"7.2\" \"8.0\"", "Step_Type"="NumericLimitTest", "LowLimit"=7.2, "HighLimit"=8.0, "RValue"="7.585999965667725", "RStatus"="PASS", "RetVal"="0", "Units"="Volts", "header1"="", "header2"="---VCOMM and MUX 2A & 2B and Internal J1850 and CAN 1 transciever Rx---\r\r\r\r\r\r\r\r\r\r\r\r\r\r\r\r\r\r\r\r\r\r\r\r\r\r\r\r\r\r\r\r\r\r\r\r\r", "ExpectedValue"=""}, {"Test_Name"="553. SetFpgaRegister \"89E\" \"60\"", "Step_Type"="", "LowLimit"=0.0, "HighLimit"=0.0, "RValue"="", "RStatus"="", "RetVal"="0", "Units"="", "header1"="", "header2"="---VCOMM and MUX 2A & 2B and Internal J1850 and CAN 1 transciever Rx---\r\r\r\r\r\r\r\r\r\r\r\r\r\r\r\r\r\r\r\r\r\r\r\r\r\r\r\r\r\r\r\r\r\r\r\r\r\r", "ExpectedValue"=""}, {"Test_Name"="554. SetFpgaRegister \"959\" \"00\"", "Step_Type"="", "LowLimit"=0.0, "HighLimit"=0.0, "RValue"="", "RStatus"="", "RetVal"="0", "Units"="", "header1"="", "header2"="---VCOMM and MUX 2A & 2B and Internal J1850 and CAN 1 transciever Rx---\r\r\r\r\r\r\r\r\r\r\r\r\r\r\r\r\r\r\r\r\r\r\r\r\r\r\r\r\r\r\r\r\r\r\r\r\r\r\r", "ExpectedValue"=""}, {"Test_Name"="555. Pause \"100\"", "Step_Type"="", "LowLimit"=0.0, "HighLimit"=0.0, "RValue"="", "RStatus"="", "RetVal"="0", "Units"="", "header1"="", "header2"="---VCOMM and MUX 2A & 2B and Internal J1850 and CAN 1 transciever Rx---\r\r\r\r\r\r\r\r\r\r\r\r\r\r\r\r\r\r\r\r\r\r\r\r\r\r\r\r\r\r\r\r\r\r\r\r\r\r\r\r", "ExpectedValue"=""}, {"Test_Name"="558. CheckCFAdc \"PD1\" \"-.15\" \".3\"", "Step_Type"="NumericLimitTest", "LowLimit"=-0.15, "HighLimit"=0.3, "RValue"="0.035999998450279236", "RStatus"="PASS", "RetVal"="0", "Units"="Volts", "header1"="", "header2"="---VCOMM and MUX 2A & 2B and Internal J1850 and CAN 1 transciever Rx---\r\r\r\r\r\r\r\r\r\r\r\r\r\r\r\r\r\r\r\r\r\r\r\r\r\r\r\r\r\r\r\r\r\r\r\r\r\r\r\r\r", "ExpectedValue"=""}, {"Test_Name"="559. CheckCFAdc \"PD2\" \"12.8\" \"14\"", "Step_Type"="NumericLimitTest", "LowLimit"=12.8, "HighLimit"=14.0, "RValue"="13.428000450134277", "RStatus"="PASS", "RetVal"="0", "Units"="Volts", "header1"="", "header2"="---VCOMM and MUX 2A & 2B and Internal J1850 and CAN 1 transciever Rx---\r\r\r\r\r\r\r\r\r\r\r\r\r\r\r\r\r\r\r\r\r\r\r\r\r\r\r\r\r\r\r\r\r\r\r\r\r\r\r\r\r\r", "ExpectedValue"=""}, {"Test_Name"="565. SetFpgaRegister \"89E\" \"40\"", "Step_Type"="", "LowLimit"=0.0, "HighLimit"=0.0, "RValue"="", "RStatus"="", "RetVal"="0", "Units"="", "header1"="", "header2"="---VCOMM and MUX 2A & 2B and Internal J1850 and CAN 1 transciever Rx---\r\r\r\r\r\r\r\r\r\r\r\r\r\r\r\r\r\r\r\r\r\r\r\r\r\r\r\r\r\r\r\r\r\r\r\r\r\r\r\r\r\r\r", "ExpectedValue"=""}, {"Test_Name"="566. SetFpgaRegister \"839\" \"04\"", "Step_Type"="", "LowLimit"=0.0, "HighLimit"=0.0, "RValue"="", "RStatus"="", "RetVal"="0", "Units"="", "header1"="", "header2"="---VCOMM and MUX 2A & 2B and Internal J1850 and CAN 1 transciever Rx---\r\r\r\r\r\r\r\r\r\r\r\r\r\r\r\r\r\r\r\r\r\r\r\r\r\r\r\r\r\r\r\r\r\r\r\r\r\r\r\r\r\r\r\r", "ExpectedValue"=""}, {"Test_Name"="567. Pause 200", "Step_Type"="", "LowLimit"=0.0, "HighLimit"=0.0, "RValue"="", "RStatus"="", "RetVal"="0", "Units"="", "header1"="", "header2"="---VCOMM and MUX 2A & 2B and Internal J1850 and CAN 1 transciever Rx---\r\r\r\r\r\r\r\r\r\r\r\r\r\r\r\r\r\r\r\r\r\r\r\r\r\r\r\r\r\r\r\r\r\r\r\r\r\r\r\r\r\r\r\r\r", "ExpectedValue"=""}, {"Test_Name"="568. SetFpgaRegister \"983\" \"04\"", "Step_Type"="", "LowLimit"=0.0, "HighLimit"=0.0, "RValue"="", "RStatus"="", "RetVal"="0", "Units"="", "header1"="", "header2"="---VCOMM and MUX 2A & 2B and Internal J1850 and CAN 1 transciever Rx---\r\r\r\r\r\r\r\r\r\r\r\r\r\r\r\r\r\r\r\r\r\r\r\r\r\r\r\r\r\r\r\r\r\r\r\r\r\r\r\r\r\r\r\r\r\r", "ExpectedValue"=""}, {"Test_Name"="569. CheckCFAdc \"PD1\" \"5.0\" \"5.5\"", "Step_Type"="NumericLimitTest", "LowLimit"=5.0, "HighLimit"=5.5, "RValue"="5.283999919891357", "RStatus"="PASS", "RetVal"="0", "Units"="Volts", "header1"="", "header2"="---VCOMM and MUX 2A & 2B and Internal J1850 and CAN 1 transciever Rx---\r\r\r\r\r\r\r\r\r\r\r\r\r\r\r\r\r\r\r\r\r\r\r\r\r\r\r\r\r\r\r\r\r\r\r\r\r\r\r\r\r\r\r\r\r\r\r", "ExpectedValue"=""}, {"Test_Name"="570. CheckCFAdc \"PD2\" \"4.8\" \"5.3\"", "Step_Type"="NumericLimitTest", "LowLimit"=4.8, "HighLimit"=5.3, "RValue"="5.047999858856201", "RStatus"="PASS", "RetVal"="0", "Units"="Volts", "header1"="", "header2"="---VCOMM and MUX 2A & 2B and Internal J1850 and CAN 1 transciever Rx---\r\r\r\r\r\r\r\r\r\r\r\r\r\r\r\r\r\r\r\r\r\r\r\r\r\r\r\r\r\r\r\r\r\r\r\r\r\r\r\r\r\r\r\r\r\r\r\r", "ExpectedValue"=""}, {"Test_Name"="571. SetFpgaRegister \"983\" \"00\"", "Step_Type"="", "LowLimit"=0.0, "HighLimit"=0.0, "RValue"="", "RStatus"="", "RetVal"="0", "Units"="", "header1"="", "header2"="---VCOMM and MUX 2A & 2B and Internal J1850 and CAN 1 transciever Rx---\r\r\r\r\r\r\r\r\r\r\r\r\r\r\r\r\r\r\r\r\r\r\r\r\r\r\r\r\r\r\r\r\r\r\r\r\r\r\r\r\r\r\r\r\r\r\r\r\r", "ExpectedValue"=""}, {"Test_Name"="572. CheckCFAdc \"PD1\" \"-.15\" \"0.3\"", "Step_Type"="NumericLimitTest", "LowLimit"=-0.15, "HighLimit"=0.3, "RValue"="0.035999998450279236", "RStatus"="PASS", "RetVal"="0", "Units"="Volts", "header1"="", "header2"="---VCOMM and MUX 2A & 2B and Internal J1850 and CAN 1 transciever Rx---\r\r\r\r\r\r\r\r\r\r\r\r\r\r\r\r\r\r\r\r\r\r\r\r\r\r\r\r\r\r\r\r\r\r\r\r\r\r\r\r\r\r\r\r\r\r\r\r\r\r", "ExpectedValue"=""}, {"Test_Name"="573. CheckCFAdc \"PD2\" \"4.8\" \"5.3\"", "Step_Type"="NumericLimitTest", "LowLimit"=4.8, "HighLimit"=5.3, "RValue"="5.047999858856201", "RStatus"="PASS", "RetVal"="0", "Units"="Volts", "header1"="", "header2"="---VCOMM and MUX 2A & 2B and Internal J1850 and CAN 1 transciever Rx---\r\r\r\r\r\r\r\r\r\r\r\r\r\r\r\r\r\r\r\r\r\r\r\r\r\r\r\r\r\r\r\r\r\r\r\r\r\r\r\r\r\r\r\r\r\r\r\r\r\r\r", "ExpectedValue"=""}, {"Test_Name"="574. SetFpgaRegister \"89E\" \"00\"", "Step_Type"="", "LowLimit"=0.0, "HighLimit"=0.0, "RValue"="", "RStatus"="", "RetVal"="0", "Units"="", "header1"="", "header2"="---VCOMM and MUX 2A & 2B and Internal J1850 and CAN 1 transciever Rx---\r\r\r\r\r\r\r\r\r\r\r\r\r\r\r\r\r\r\r\r\r\r\r\r\r\r\r\r\r\r\r\r\r\r\r\r\r\r\r\r\r\r\r\r\r\r\r\r\r\r\r\r", "ExpectedValue"=""}, {"Test_Name"="575. SetFpgaRegister \"839\" \"00\"", "Step_Type"="", "LowLimit"=0.0, "HighLimit"=0.0, "RValue"="", "RStatus"="", "RetVal"="0", "Units"="", "header1"="", "header2"="---VCOMM and MUX 2A & 2B and Internal J1850 and CAN 1 transciever Rx---\r\r\r\r\r\r\r\r\r\r\r\r\r\r\r\r\r\r\r\r\r\r\r\r\r\r\r\r\r\r\r\r\r\r\r\r\r\r\r\r\r\r\r\r\r\r\r\r\r\r\r\r\r", "ExpectedValue"=""}, {"Test_Name"="576. SetFpgaRegister \"983\" \"00\"", "Step_Type"="", "LowLimit"=0.0, "HighLimit"=0.0, "RValue"="", "RStatus"="", "RetVal"="0", "Units"="", "header1"="", "header2"="---VCOMM and MUX 2A & 2B and Internal J1850 and CAN 1 transciever Rx---\r\r\r\r\r\r\r\r\r\r\r\r\r\r\r\r\r\r\r\r\r\r\r\r\r\r\r\r\r\r\r\r\r\r\r\r\r\r\r\r\r\r\r\r\r\r\r\r\r\r\r\r\r\r", "ExpectedValue"=""}, {"Test_Name"="581. SetG15PullUp \"A\" \"9\"", "Step_Type"="", "LowLimit"=0.0, "HighLimit"=0.0, "RValue"="", "RStatus"="", "RetVal"="0", "Units"="", "header1"="", "header2"="---VCOMM and MUX 2A & 2B and Internal J1850 and CAN 1 transciever Rx---\r\r\r\r\r\r\r\r\r\r\r\r\r\r\r\r\r\r\r\r\r\r\r\r\r\r\r\r\r\r\r\r\r\r\r\r\r\r\r\r\r\r\r\r\r\r\r\r\r\r\r\r\r\r\r", "ExpectedValue"=""}, {"Test_Name"="582. SetAsicRegister \"1\" \"0\" \"40\"", "Step_Type"="", "LowLimit"=0.0, "HighLimit"=0.0, "RValue"="", "RStatus"="", "RetVal"="0", "Units"="", "header1"="", "header2"="---VCOMM and MUX 2A & 2B and Internal J1850 and CAN 1 transciever Rx---\r\r\r\r\r\r\r\r\r\r\r\r\r\r\r\r\r\r\r\r\r\r\r\r\r\r\r\r\r\r\r\r\r\r\r\r\r\r\r\r\r\r\r\r\r\r\r\r\r\r\r\r\r\r\r\r", "ExpectedValue"=""}, {"Test_Name"="583. SetAsicRegister \"1\" \"2\" \"40\"", "Step_Type"="", "LowLimit"=0.0, "HighLimit"=0.0, "RValue"="", "RStatus"="", "RetVal"="0", "Units"="", "header1"="", "header2"="---VCOMM and MUX 2A & 2B and Internal J1850 and CAN 1 transciever Rx---\r\r\r\r\r\r\r\r\r\r\r\r\r\r\r\r\r\r\r\r\r\r\r\r\r\r\r\r\r\r\r\r\r\r\r\r\r\r\r\r\r\r\r\r\r\r\r\r\r\r\r\r\r\r\r\r\r", "ExpectedValue"=""}, {"Test_Name"="584. CheckCFAdc \"PD1\" \"4.5\" \"5.0\"", "Step_Type"="NumericLimitTest", "LowLimit"=4.5, "HighLimit"=5.0, "RValue"="4.748000144958496", "RStatus"="PASS", "RetVal"="0", "Units"="Volts", "header1"="", "header2"="---VCOMM and MUX 2A & 2B and Internal J1850 and CAN 1 transciever Rx---\r\r\r\r\r\r\r\r\r\r\r\r\r\r\r\r\r\r\r\r\r\r\r\r\r\r\r\r\r\r\r\r\r\r\r\r\r\r\r\r\r\r\r\r\r\r\r\r\r\r\r\r\r\r\r\r\r\r", "ExpectedValue"=""}, {"Test_Name"="585. CheckCFAdc \"PD2\" \".5\" \"1.4\"", "Step_Type"="NumericLimitTest", "LowLimit"=0.5, "HighLimit"=1.4, "RValue"="1.0609999895095825", "RStatus"="PASS", "RetVal"="0", "Units"="Volts", "header1"="", "header2"="---VCOMM and MUX 2A & 2B and Internal J1850 and CAN 1 transciever Rx---\r\r\r\r\r\r\r\r\r\r\r\r\r\r\r\r\r\r\r\r\r\r\r\r\r\r\r\r\r\r\r\r\r\r\r\r\r\r\r\r\r\r\r\r\r\r\r\r\r\r\r\r\r\r\r\r\r\r\r", "ExpectedValue"=""}, {"Test_Name"="586. CheckFpgaRegister \"632\" \"0\" \"0\"", "Step_Type"="StringValueTest", "LowLimit"=0.0, "HighLimit"=0.0, "RValue"="0", "RStatus"="PASS", "RetVal"="0", "Units"="", "header1"="", "header2"="---VCOMM and MUX 2A & 2B and Internal J1850 and CAN 1 transciever Rx---\r\r\r\r\r\r\r\r\r\r\r\r\r\r\r\r\r\r\r\r\r\r\r\r\r\r\r\r\r\r\r\r\r\r\r\r\r\r\r\r\r\r\r\r\r\r\r\r\r\r\r\r\r\r\r\r\r\r\r\r", "ExpectedValue"=""}, {"Test_Name"="587. ReadFpgaRegister \"632\"", "Step_Type"="", "LowLimit"=0.0, "HighLimit"=0.0, "RValue"="0", "RStatus"="", "RetVal"="0", "Units"="", "header1"="", "header2"="---VCOMM and MUX 2A & 2B and Internal J1850 and CAN 1 transciever Rx---\r\r\r\r\r\r\r\r\r\r\r\r\r\r\r\r\r\r\r\r\r\r\r\r\r\r\r\r\r\r\r\r\r\r\r\r\r\r\r\r\r\r\r\r\r\r\r\r\r\r\r\r\r\r\r\r\r\r\r\r\r", "ExpectedValue"=""}, {"Test_Name"="588. SetG15PullUp \"A\" \"0\"", "Step_Type"="", "LowLimit"=0.0, "HighLimit"=0.0, "RValue"="", "RStatus"="", "RetVal"="0", "Units"="", "header1"="", "header2"="---VCOMM and MUX 2A & 2B and Internal J1850 and CAN 1 transciever Rx---\r\r\r\r\r\r\r\r\r\r\r\r\r\r\r\r\r\r\r\r\r\r\r\r\r\r\r\r\r\r\r\r\r\r\r\r\r\r\r\r\r\r\r\r\r\r\r\r\r\r\r\r\r\r\r\r\r\r\r\r\r\r", "ExpectedValue"=""}, {"Test_Name"="589. SetG15PullUp \"B\" \"9\"", "Step_Type"="", "LowLimit"=0.0, "HighLimit"=0.0, "RValue"="", "RStatus"="", "RetVal"="0", "Units"="", "header1"="", "header2"="---VCOMM and MUX 2A & 2B and Internal J1850 and CAN 1 transciever Rx---\r\r\r\r\r\r\r\r\r\r\r\r\r\r\r\r\r\r\r\r\r\r\r\r\r\r\r\r\r\r\r\r\r\r\r\r\r\r\r\r\r\r\r\r\r\r\r\r\r\r\r\r\r\r\r\r\r\r\r\r\r\r\r", "ExpectedValue"=""}, {"Test_Name"="590. CheckCFAdc \"PD1\" \".5\" \"1.5\"", "Step_Type"="NumericLimitTest", "LowLimit"=0.5, "HighLimit"=1.5, "RValue"="1.0529999732971191", "RStatus"="PASS", "RetVal"="0", "Units"="Volts", "header1"="", "header2"="---VCOMM and MUX 2A & 2B and Internal J1850 and CAN 1 transciever Rx---\r\r\r\r\r\r\r\r\r\r\r\r\r\r\r\r\r\r\r\r\r\r\r\r\r\r\r\r\r\r\r\r\r\r\r\r\r\r\r\r\r\r\r\r\r\r\r\r\r\r\r\r\r\r\r\r\r\r\r\r\r\r\r\r", "ExpectedValue"=""}, {"Test_Name"="591. CheckCFAdc \"PD2\" \"4.5\" \"5.0\"", "Step_Type"="NumericLimitTest", "LowLimit"=4.5, "HighLimit"=5.0, "RValue"="4.770999908447266", "RStatus"="PASS", "RetVal"="0", "Units"="Volts", "header1"="", "header2"="---VCOMM and MUX 2A & 2B and Internal J1850 and CAN 1 transciever Rx---\r\r\r\r\r\r\r\r\r\r\r\r\r\r\r\r\r\r\r\r\r\r\r\r\r\r\r\r\r\r\r\r\r\r\r\r\r\r\r\r\r\r\r\r\r\r\r\r\r\r\r\r\r\r\r\r\r\r\r\r\r\r\r\r\r", "ExpectedValue"=""}, {"Test_Name"="592. CheckFpgaRegister \"632\" \"0\" \"1\"", "Step_Type"="StringValueTest", "LowLimit"=0.0, "HighLimit"=0.0, "RValue"="1", "RStatus"="PASS", "RetVal"="0", "Units"="", "header1"="", "header2"="---VCOMM and MUX 2A & 2B and Internal J1850 and CAN 1 transciever Rx---\r\r\r\r\r\r\r\r\r\r\r\r\r\r\r\r\r\r\r\r\r\r\r\r\r\r\r\r\r\r\r\r\r\r\r\r\r\r\r\r\r\r\r\r\r\r\r\r\r\r\r\r\r\r\r\r\r\r\r\r\r\r\r\r\r\r", "ExpectedValue"=""}, {"Test_Name"="593. SetG15PullUp \"B\" \"0\"", "Step_Type"="", "LowLimit"=0.0, "HighLimit"=0.0, "RValue"="", "RStatus"="", "RetVal"="0", "Units"="", "header1"="", "header2"="---VCOMM and MUX 2A & 2B and Internal J1850 and CAN 1 transciever Rx---\r\r\r\r\r\r\r\r\r\r\r\r\r\r\r\r\r\r\r\r\r\r\r\r\r\r\r\r\r\r\r\r\r\r\r\r\r\r\r\r\r\r\r\r\r\r\r\r\r\r\r\r\r\r\r\r\r\r\r\r\r\r\r\r\r\r\r", "ExpectedValue"=""}, {"Test_Name"="594. SetG15PullUp \"A\" \"9\"", "Step_Type"="", "LowLimit"=0.0, "HighLimit"=0.0, "RValue"="", "RStatus"="", "RetVal"="0", "Units"="", "header1"="", "header2"="---VCOMM and MUX 2A & 2B and Internal J1850 and CAN 1 transciever Rx---\r\r\r\r\r\r\r\r\r\r\r\r\r\r\r\r\r\r\r\r\r\r\r\r\r\r\r\r\r\r\r\r\r\r\r\r\r\r\r\r\r\r\r\r\r\r\r\r\r\r\r\r\r\r\r\r\r\r\r\r\r\r\r\r\r\r\r\r", "ExpectedValue"=""}, {"Test_Name"="595. CheckCFAdc \"PD1\" \"4.5\" \"5.0\"", "Step_Type"="NumericLimitTest", "LowLimit"=4.5, "HighLimit"=5.0, "RValue"="4.748000144958496", "RStatus"="PASS", "RetVal"="0", "Units"="Volts", "header1"="", "header2"="---VCOMM and MUX 2A & 2B and Internal J1850 and CAN 1 transciever Rx---\r\r\r\r\r\r\r\r\r\r\r\r\r\r\r\r\r\r\r\r\r\r\r\r\r\r\r\r\r\r\r\r\r\r\r\r\r\r\r\r\r\r\r\r\r\r\r\r\r\r\r\r\r\r\r\r\r\r\r\r\r\r\r\r\r\r\r\r\r", "ExpectedValue"=""}, {"Test_Name"="596. CheckCFAdc \"PD2\" \".5\" \"1.6\"", "Step_Type"="NumericLimitTest", "LowLimit"=0.5, "HighLimit"=1.6, "RValue"="1.2730000019073486", "RStatus"="PASS", "RetVal"="0", "Units"="Volts", "header1"="", "header2"="---VCOMM and MUX 2A & 2B and Internal J1850 and CAN 1 transciever Rx---\r\r\r\r\r\r\r\r\r\r\r\r\r\r\r\r\r\r\r\r\r\r\r\r\r\r\r\r\r\r\r\r\r\r\r\r\r\r\r\r\r\r\r\r\r\r\r\r\r\r\r\r\r\r\r\r\r\r\r\r\r\r\r\r\r\r\r\r\r\r", "ExpectedValue"=""}, {"Test_Name"="597. CheckFpgaRegister \"632\" \"0\" \"0\"", "Step_Type"="StringValueTest", "LowLimit"=0.0, "HighLimit"=0.0, "RValue"="0", "RStatus"="PASS", "RetVal"="0", "Units"="", "header1"="", "header2"="---VCOMM and MUX 2A & 2B and Internal J1850 and CAN 1 transciever Rx---\r\r\r\r\r\r\r\r\r\r\r\r\r\r\r\r\r\r\r\r\r\r\r\r\r\r\r\r\r\r\r\r\r\r\r\r\r\r\r\r\r\r\r\r\r\r\r\r\r\r\r\r\r\r\r\r\r\r\r\r\r\r\r\r\r\r\r\r\r\r\r", "ExpectedValue"=""}, {"Test_Name"="598. SetG15PullUp \"A\" \"0\"", "Step_Type"="", "LowLimit"=0.0, "HighLimit"=0.0, "RValue"="", "RStatus"="", "RetVal"="0", "Units"="", "header1"="", "header2"="---VCOMM and MUX 2A & 2B and Internal J1850 and CAN 1 transciever Rx---\r\r\r\r\r\r\r\r\r\r\r\r\r\r\r\r\r\r\r\r\r\r\r\r\r\r\r\r\r\r\r\r\r\r\r\r\r\r\r\r\r\r\r\r\r\r\r\r\r\r\r\r\r\r\r\r\r\r\r\r\r\r\r\r\r\r\r\r\r\r\r\r", "ExpectedValue"=""}, {"Test_Name"="599. SetFpgaRegister \"630\" \"04\"", "Step_Type"="", "LowLimit"=0.0, "HighLimit"=0.0, "RValue"="", "RStatus"="", "RetVal"="0", "Units"="", "header1"="", "header2"="---VCOMM and MUX 2A & 2B and Internal J1850 and CAN 1 transciever Rx---\r\r\r\r\r\r\r\r\r\r\r\r\r\r\r\r\r\r\r\r\r\r\r\r\r\r\r\r\r\r\r\r\r\r\r\r\r\r\r\r\r\r\r\r\r\r\r\r\r\r\r\r\r\r\r\r\r\r\r\r\r\r\r\r\r\r\r\r\r\r\r\r\r", "ExpectedValue"=""}, {"Test_Name"="600. ReadFpgaRegister \"630\"", "Step_Type"="", "LowLimit"=0.0, "HighLimit"=0.0, "RValue"="4", "RStatus"="", "RetVal"="0", "Units"="", "header1"="", "header2"="---VCOMM and MUX 2A & 2B and Internal J1850 and CAN 1 transciever Rx---\r\r\r\r\r\r\r\r\r\r\r\r\r\r\r\r\r\r\r\r\r\r\r\r\r\r\r\r\r\r\r\r\r\r\r\r\r\r\r\r\r\r\r\r\r\r\r\r\r\r\r\r\r\r\r\r\r\r\r\r\r\r\r\r\r\r\r\r\r\r\r\r\r\r", "ExpectedValue"=""}, {"Test_Name"="601. CheckCFAdc \"PD1\" \"4.6\" \"5.2\"", "Step_Type"="NumericLimitTest", "LowLimit"=4.6, "HighLimit"=5.2, "RValue"="4.914000034332275", "RStatus"="PASS", "RetVal"="0", "Units"="Volts", "header1"="", "header2"="---VCOMM and MUX 2A & 2B and Internal J1850 and CAN 1 transciever Rx---\r\r\r\r\r\r\r\r\r\r\r\r\r\r\r\r\r\r\r\r\r\r\r\r\r\r\r\r\r\r\r\r\r\r\r\r\r\r\r\r\r\r\r\r\r\r\r\r\r\r\r\r\r\r\r\r\r\r\r\r\r\r\r\r\r\r\r\r\r\r\r\r\r\r\r", "ExpectedValue"=""}, {"Test_Name"="602. CheckCFAdc \"PD2\" \"-.15\" \".3\"", "Step_Type"="NumericLimitTest", "LowLimit"=-0.15, "HighLimit"=0.3, "RValue"="0.09200000017881393", "RStatus"="PASS", "RetVal"="0", "Units"="Volts", "header1"="", "header2"="---VCOMM and MUX 2A & 2B and Internal J1850 and CAN 1 transciever Rx---\r\r\r\r\r\r\r\r\r\r\r\r\r\r\r\r\r\r\r\r\r\r\r\r\r\r\r\r\r\r\r\r\r\r\r\r\r\r\r\r\r\r\r\r\r\r\r\r\r\r\r\r\r\r\r\r\r\r\r\r\r\r\r\r\r\r\r\r\r\r\r\r\r\r\r\r", "ExpectedValue"=""}, {"Test_Name"="603. ReadFpgaRegister \"632\"", "Step_Type"="", "LowLimit"=0.0, "HighLimit"=0.0, "RValue"="0", "RStatus"="", "RetVal"="0", "Units"="", "header1"="", "header2"="---VCOMM and MUX 2A & 2B and Internal J1850 and CAN 1 transciever Rx---\r\r\r\r\r\r\r\r\r\r\r\r\r\r\r\r\r\r\r\r\r\r\r\r\r\r\r\r\r\r\r\r\r\r\r\r\r\r\r\r\r\r\r\r\r\r\r\r\r\r\r\r\r\r\r\r\r\r\r\r\r\r\r\r\r\r\r\r\r\r\r\r\r\r\r\r\r", "ExpectedValue"=""}, {"Test_Name"="604. SetFpgaRegister \"630\" \"00\"", "Step_Type"="", "LowLimit"=0.0, "HighLimit"=0.0, "RValue"="", "RStatus"="", "RetVal"="0", "Units"="", "header1"="", "header2"="---VCOMM and MUX 2A & 2B and Internal J1850 and CAN 1 transciever Rx---\r\r\r\r\r\r\r\r\r\r\r\r\r\r\r\r\r\r\r\r\r\r\r\r\r\r\r\r\r\r\r\r\r\r\r\r\r\r\r\r\r\r\r\r\r\r\r\r\r\r\r\r\r\r\r\r\r\r\r\r\r\r\r\r\r\r\r\r\r\r\r\r\r\r\r\r\r\r", "ExpectedValue"=""}, {"Test_Name"="605. ReadFpgaRegister \"630\"", "Step_Type"="", "LowLimit"=0.0, "HighLimit"=0.0, "RValue"="0", "RStatus"="", "RetVal"="0", "Units"="", "header1"="", "header2"="---VCOMM and MUX 2A & 2B and Internal J1850 and CAN 1 transciever Rx---\r\r\r\r\r\r\r\r\r\r\r\r\r\r\r\r\r\r\r\r\r\r\r\r\r\r\r\r\r\r\r\r\r\r\r\r\r\r\r\r\r\r\r\r\r\r\r\r\r\r\r\r\r\r\r\r\r\r\r\r\r\r\r\r\r\r\r\r\r\r\r\r\r\r\r\r\r\r\r", "ExpectedValue"=""}, {"Test_Name"="606. CheckCFAdc \"PD1\" \".5\" \"1.5\"", "Step_Type"="NumericLimitTest", "LowLimit"=0.5, "HighLimit"=1.5, "RValue"="1.0429999828338623", "RStatus"="PASS", "RetVal"="0", "Units"="Volts", "header1"="", "header2"="---VCOMM and MUX 2A & 2B and Internal J1850 and CAN 1 transciever Rx---\r\r\r\r\r\r\r\r\r\r\r\r\r\r\r\r\r\r\r\r\r\r\r\r\r\r\r\r\r\r\r\r\r\r\r\r\r\r\r\r\r\r\r\r\r\r\r\r\r\r\r\r\r\r\r\r\r\r\r\r\r\r\r\r\r\r\r\r\r\r\r\r\r\r\r\r\r\r\r\r", "ExpectedValue"=""}, {"Test_Name"="607. CheckCFAdc \"PD2\" \".5\" \"2.4\"", "Step_Type"="NumericLimitTest", "LowLimit"=0.5, "HighLimit"=2.4, "RValue"="1.8079999685287476", "RStatus"="PASS", "RetVal"="0", "Units"="Volts", "header1"="", "header2"="---VCOMM and MUX 2A & 2B and Internal J1850 and CAN 1 transciever Rx---\r\r\r\r\r\r\r\r\r\r\r\r\r\r\r\r\r\r\r\r\r\r\r\r\r\r\r\r\r\r\r\r\r\r\r\r\r\r\r\r\r\r\r\r\r\r\r\r\r\r\r\r\r\r\r\r\r\r\r\r\r\r\r\r\r\r\r\r\r\r\r\r\r\r\r\r\r\r\r\r\r", "ExpectedValue"=""}, {"Test_Name"="608. ReadFpgaRegister \"632\"", "Step_Type"="", "LowLimit"=0.0, "HighLimit"=0.0, "RValue"="1", "RStatus"="", "RetVal"="0", "Units"="", "header1"="", "header2"="---VCOMM and MUX 2A & 2B and Internal J1850 and CAN 1 transciever Rx---\r\r\r\r\r\r\r\r\r\r\r\r\r\r\r\r\r\r\r\r\r\r\r\r\r\r\r\r\r\r\r\r\r\r\r\r\r\r\r\r\r\r\r\r\r\r\r\r\r\r\r\r\r\r\r\r\r\r\r\r\r\r\r\r\r\r\r\r\r\r\r\r\r\r\r\r\r\r\r\r\r\r", "ExpectedValue"=""}, {"Test_Name"="610. SetCANGpioMode \"1\"", "Step_Type"="", "LowLimit"=0.0, "HighLimit"=0.0, "RValue"="", "RStatus"="", "RetVal"="0", "Units"="", "header1"="", "header2"="---VCOMM and MUX 2A & 2B and Internal J1850 and CAN 1 transciever Rx---\r\r\r\r\r\r\r\r\r\r\r\r\r\r\r\r\r\r\r\r\r\r\r\r\r\r\r\r\r\r\r\r\r\r\r\r\r\r\r\r\r\r\r\r\r\r\r\r\r\r\r\r\r\r\r\r\r\r\r\r\r\r\r\r\r\r\r\r\r\r\r\r\r\r\r\r\r\r\r\r\r\r\r", "ExpectedValue"=""}, {"Test_Name"="611. SetFpgaRegister \"839\" \"01\"", "Step_Type"="", "LowLimit"=0.0, "HighLimit"=0.0, "RValue"="", "RStatus"="", "RetVal"="0", "Units"="", "header1"="", "header2"="---VCOMM and MUX 2A & 2B and Internal J1850 and CAN 1 transciever Rx---\r\r\r\r\r\r\r\r\r\r\r\r\r\r\r\r\r\r\r\r\r\r\r\r\r\r\r\r\r\r\r\r\r\r\r\r\r\r\r\r\r\r\r\r\r\r\r\r\r\r\r\r\r\r\r\r\r\r\r\r\r\r\r\r\r\r\r\r\r\r\r\r\r\r\r\r\r\r\r\r\r\r\r\r", "ExpectedValue"=""}, {"Test_Name"="612. SetAsicRegister \"1\" \"0\" \"20\"", "Step_Type"="", "LowLimit"=0.0, "HighLimit"=0.0, "RValue"="", "RStatus"="", "RetVal"="0", "Units"="", "header1"="", "header2"="---VCOMM and MUX 2A & 2B and Internal J1850 and CAN 1 transciever Rx---\r\r\r\r\r\r\r\r\r\r\r\r\r\r\r\r\r\r\r\r\r\r\r\r\r\r\r\r\r\r\r\r\r\r\r\r\r\r\r\r\r\r\r\r\r\r\r\r\r\r\r\r\r\r\r\r\r\r\r\r\r\r\r\r\r\r\r\r\r\r\r\r\r\r\r\r\r\r\r\r\r\r\r\r\r", "ExpectedValue"=""}, {"Test_Name"="613. SetAsicRegister \"1\" \"2\" \"20\"", "Step_Type"="", "LowLimit"=0.0, "HighLimit"=0.0, "RValue"="", "RStatus"="", "RetVal"="0", "Units"="", "header1"="", "header2"="---VCOMM and MUX 2A & 2B and Internal J1850 and CAN 1 transciever Rx---\r\r\r\r\r\r\r\r\r\r\r\r\r\r\r\r\r\r\r\r\r\r\r\r\r\r\r\r\r\r\r\r\r\r\r\r\r\r\r\r\r\r\r\r\r\r\r\r\r\r\r\r\r\r\r\r\r\r\r\r\r\r\r\r\r\r\r\r\r\r\r\r\r\r\r\r\r\r\r\r\r\r\r\r\r\r", "ExpectedValue"=""}, {"Test_Name"="614. CheckCFAdc \"PD1\" \"2.3\" \"2.75\"", "Step_Type"="NumericLimitTest", "LowLimit"=2.3, "HighLimit"=2.75, "RValue"="2.5399999618530273", "RStatus"="PASS", "RetVal"="0", "Units"="Volts", "header1"="", "header2"="---VCOMM and MUX 2A & 2B and Internal J1850 and CAN 1 transciever Rx---\r\r\r\r\r\r\r\r\r\r\r\r\r\r\r\r\r\r\r\r\r\r\r\r\r\r\r\r\r\r\r\r\r\r\r\r\r\r\r\r\r\r\r\r\r\r\r\r\r\r\r\r\r\r\r\r\r\r\r\r\r\r\r\r\r\r\r\r\r\r\r\r\r\r\r\r\r\r\r\r\r\r\r\r\r\r\r", "ExpectedValue"=""}, {"Test_Name"="615. CheckCFAdc \"PD2\" \"2.3\" \"2.65\"", "Step_Type"="NumericLimitTest", "LowLimit"=2.3, "HighLimit"=2.65, "RValue"="2.565000057220459", "RStatus"="PASS", "RetVal"="0", "Units"="Volts", "header1"="", "header2"="---VCOMM and MUX 2A & 2B and Internal J1850 and CAN 1 transciever Rx---\r\r\r\r\r\r\r\r\r\r\r\r\r\r\r\r\r\r\r\r\r\r\r\r\r\r\r\r\r\r\r\r\r\r\r\r\r\r\r\r\r\r\r\r\r\r\r\r\r\r\r\r\r\r\r\r\r\r\r\r\r\r\r\r\r\r\r\r\r\r\r\r\r\r\r\r\r\r\r\r\r\r\r\r\r\r\r\r", "ExpectedValue"=""}, {"Test_Name"="617. SetG15PullUp \"A\" \"2\"", "Step_Type"="", "LowLimit"=0.0, "HighLimit"=0.0, "RValue"="", "RStatus"="", "RetVal"="0", "Units"="", "header1"="", "header2"="---VCOMM and MUX 2A & 2B and Internal J1850 and CAN 1 transciever Rx---\r\r\r\r\r\r\r\r\r\r\r\r\r\r\r\r\r\r\r\r\r\r\r\r\r\r\r\r\r\r\r\r\r\r\r\r\r\r\r\r\r\r\r\r\r\r\r\r\r\r\r\r\r\r\r\r\r\r\r\r\r\r\r\r\r\r\r\r\r\r\r\r\r\r\r\r\r\r\r\r\r\r\r\r\r\r\r\r\r", "ExpectedValue"=""}, {"Test_Name"="618. CheckCFAdc \"PD1\" \"4.5\" \"5.0\"", "Step_Type"="NumericLimitTest", "LowLimit"=4.5, "HighLimit"=5.0, "RValue"="4.729000091552734", "RStatus"="PASS", "RetVal"="0", "Units"="Volts", "header1"="", "header2"="---VCOMM and MUX 2A & 2B and Internal J1850 and CAN 1 transciever Rx---\r\r\r\r\r\r\r\r\r\r\r\r\r\r\r\r\r\r\r\r\r\r\r\r\r\r\r\r\r\r\r\r\r\r\r\r\r\r\r\r\r\r\r\r\r\r\r\r\r\r\r\r\r\r\r\r\r\r\r\r\r\r\r\r\r\r\r\r\r\r\r\r\r\r\r\r\r\r\r\r\r\r\r\r\r\r\r\r\r\r", "ExpectedValue"=""}, {"Test_Name"="619. Pause 100", "Step_Type"="", "LowLimit"=0.0, "HighLimit"=0.0, "RValue"="", "RStatus"="", "RetVal"="0", "Units"="", "header1"="", "header2"="---VCOMM and MUX 2A & 2B and Internal J1850 and CAN 1 transciever Rx---\r\r\r\r\r\r\r\r\r\r\r\r\r\r\r\r\r\r\r\r\r\r\r\r\r\r\r\r\r\r\r\r\r\r\r\r\r\r\r\r\r\r\r\r\r\r\r\r\r\r\r\r\r\r\r\r\r\r\r\r\r\r\r\r\r\r\r\r\r\r\r\r\r\r\r\r\r\r\r\r\r\r\r\r\r\r\r\r\r\r\r", "ExpectedValue"=""}, {"Test_Name"="620. CheckCanRxStatus \"0\"", "Step_Type"="StringValueTest", "LowLimit"=0.0, "HighLimit"=0.0, "RValue"="0", "RStatus"="PASS", "RetVal"="0", "Units"="", "header1"="", "header2"="---VCOMM and MUX 2A & 2B and Internal J1850 and CAN 1 transciever Rx---\r\r\r\r\r\r\r\r\r\r\r\r\r\r\r\r\r\r\r\r\r\r\r\r\r\r\r\r\r\r\r\r\r\r\r\r\r\r\r\r\r\r\r\r\r\r\r\r\r\r\r\r\r\r\r\r\r\r\r\r\r\r\r\r\r\r\r\r\r\r\r\r\r\r\r\r\r\r\r\r\r\r\r\r\r\r\r\r\r\r\r\r", "ExpectedValue"=""}, {"Test_Name"="621. SetG15PullDown \"A\" \"5\"", "Step_Type"="", "LowLimit"=0.0, "HighLimit"=0.0, "RValue"="", "RStatus"="", "RetVal"="0", "Units"="", "header1"="", "header2"="---VCOMM and MUX 2A & 2B and Internal J1850 and CAN 1 transciever Rx---\r\r\r\r\r\r\r\r\r\r\r\r\r\r\r\r\r\r\r\r\r\r\r\r\r\r\r\r\r\r\r\r\r\r\r\r\r\r\r\r\r\r\r\r\r\r\r\r\r\r\r\r\r\r\r\r\r\r\r\r\r\r\r\r\r\r\r\r\r\r\r\r\r\r\r\r\r\r\r\r\r\r\r\r\r\r\r\r\r\r\r\r\r", "ExpectedValue"=""}, {"Test_Name"="622. CheckCFAdc \"PD1\" \"-.15\" \".3\"", "Step_Type"="NumericLimitTest", "LowLimit"=-0.15, "HighLimit"=0.3, "RValue"="0.017999999225139618", "RStatus"="PASS", "RetVal"="0", "Units"="Volts", "header1"="", "header2"="---VCOMM and MUX 2A & 2B and Internal J1850 and CAN 1 transciever Rx---\r\r\r\r\r\r\r\r\r\r\r\r\r\r\r\r\r\r\r\r\r\r\r\r\r\r\r\r\r\r\r\r\r\r\r\r\r\r\r\r\r\r\r\r\r\r\r\r\r\r\r\r\r\r\r\r\r\r\r\r\r\r\r\r\r\r\r\r\r\r\r\r\r\r\r\r\r\r\r\r\r\r\r\r\r\r\r\r\r\r\r\r\r\r", "ExpectedValue"=""}, {"Test_Name"="623. CheckCFAdc \"PD2\" \"2.3\" \"2.7\"", "Step_Type"="NumericLimitTest", "LowLimit"=2.3, "HighLimit"=2.7, "RValue"="2.546999931335449", "RStatus"="PASS", "RetVal"="0", "Units"="Volts", "header1"="", "header2"="---VCOMM and MUX 2A & 2B and Internal J1850 and CAN 1 transciever Rx---\r\r\r\r\r\r\r\r\r\r\r\r\r\r\r\r\r\r\r\r\r\r\r\r\r\r\r\r\r\r\r\r\r\r\r\r\r\r\r\r\r\r\r\r\r\r\r\r\r\r\r\r\r\r\r\r\r\r\r\r\r\r\r\r\r\r\r\r\r\r\r\r\r\r\r\r\r\r\r\r\r\r\r\r\r\r\r\r\r\r\r\r\r\r\r", "ExpectedValue"=""}, {"Test_Name"="624. CheckCanRxStatus \"1\"", "Step_Type"="StringValueTest", "LowLimit"=0.0, "HighLimit"=0.0, "RValue"="1", "RStatus"="PASS", "RetVal"="0", "Units"="", "header1"="", "header2"="---VCOMM and MUX 2A & 2B and Internal J1850 and CAN 1 transciever Rx---\r\r\r\r\r\r\r\r\r\r\r\r\r\r\r\r\r\r\r\r\r\r\r\r\r\r\r\r\r\r\r\r\r\r\r\r\r\r\r\r\r\r\r\r\r\r\r\r\r\r\r\r\r\r\r\r\r\r\r\r\r\r\r\r\r\r\r\r\r\r\r\r\r\r\r\r\r\r\r\r\r\r\r\r\r\r\r\r\r\r\r\r\r\r\r\r", "ExpectedValue"=""}, {"Test_Name"="625. SetG15PullUp \"A\" \"0\"", "Step_Type"="", "LowLimit"=0.0, "HighLimit"=0.0, "RValue"="", "RStatus"="", "RetVal"="0", "Units"="", "header1"="", "header2"="---VCOMM and MUX 2A & 2B and Internal J1850 and CAN 1 transciever Rx---\r\r\r\r\r\r\r\r\r\r\r\r\r\r\r\r\r\r\r\r\r\r\r\r\r\r\r\r\r\r\r\r\r\r\r\r\r\r\r\r\r\r\r\r\r\r\r\r\r\r\r\r\r\r\r\r\r\r\r\r\r\r\r\r\r\r\r\r\r\r\r\r\r\r\r\r\r\r\r\r\r\r\r\r\r\r\r\r\r\r\r\r\r\r\r\r\r", "ExpectedValue"=""}, {"Test_Name"="626. SetG15PullDown \"A\" \"0\"", "Step_Type"="", "LowLimit"=0.0, "HighLimit"=0.0, "RValue"="", "RStatus"="", "RetVal"="0", "Units"="", "header1"="", "header2"="---VCOMM and MUX 2A & 2B and Internal J1850 and CAN 1 transciever Rx---\r\r\r\r\r\r\r\r\r\r\r\r\r\r\r\r\r\r\r\r\r\r\r\r\r\r\r\r\r\r\r\r\r\r\r\r\r\r\r\r\r\r\r\r\r\r\r\r\r\r\r\r\r\r\r\r\r\r\r\r\r\r\r\r\r\r\r\r\r\r\r\r\r\r\r\r\r\r\r\r\r\r\r\r\r\r\r\r\r\r\r\r\r\r\r\r\r\r", "ExpectedValue"=""}, {"Test_Name"="627. SetG15PullDown \"B\" \"5\"", "Step_Type"="", "LowLimit"=0.0, "HighLimit"=0.0, "RValue"="", "RStatus"="", "RetVal"="0", "Units"="", "header1"="", "header2"="---VCOMM and MUX 2A & 2B and Internal J1850 and CAN 1 transciever Rx---\r\r\r\r\r\r\r\r\r\r\r\r\r\r\r\r\r\r\r\r\r\r\r\r\r\r\r\r\r\r\r\r\r\r\r\r\r\r\r\r\r\r\r\r\r\r\r\r\r\r\r\r\r\r\r\r\r\r\r\r\r\r\r\r\r\r\r\r\r\r\r\r\r\r\r\r\r\r\r\r\r\r\r\r\r\r\r\r\r\r\r\r\r\r\r\r\r\r\r", "ExpectedValue"=""}, {"Test_Name"="628. CheckCFAdc \"PD1\" \"2.3\" \"2.7\"", "Step_Type"="NumericLimitTest", "LowLimit"=2.3, "HighLimit"=2.7, "RValue"="2.5209999084472656", "RStatus"="PASS", "RetVal"="0", "Units"="Volts", "header1"="", "header2"="---VCOMM and MUX 2A & 2B and Internal J1850 and CAN 1 transciever Rx---\r\r\r\r\r\r\r\r\r\r\r\r\r\r\r\r\r\r\r\r\r\r\r\r\r\r\r\r\r\r\r\r\r\r\r\r\r\r\r\r\r\r\r\r\r\r\r\r\r\r\r\r\r\r\r\r\r\r\r\r\r\r\r\r\r\r\r\r\r\r\r\r\r\r\r\r\r\r\r\r\r\r\r\r\r\r\r\r\r\r\r\r\r\r\r\r\r\r\r\r", "ExpectedValue"=""}, {"Test_Name"="629. CheckCFAdc \"PD2\" \"-.15\" \".3\"", "Step_Type"="NumericLimitTest", "LowLimit"=-0.15, "HighLimit"=0.3, "RValue"="0.017999999225139618", "RStatus"="PASS", "RetVal"="0", "Units"="Volts", "header1"="", "header2"="---VCOMM and MUX 2A & 2B and Internal J1850 and CAN 1 transciever Rx---\r\r\r\r\r\r\r\r\r\r\r\r\r\r\r\r\r\r\r\r\r\r\r\r\r\r\r\r\r\r\r\r\r\r\r\r\r\r\r\r\r\r\r\r\r\r\r\r\r\r\r\r\r\r\r\r\r\r\r\r\r\r\r\r\r\r\r\r\r\r\r\r\r\r\r\r\r\r\r\r\r\r\r\r\r\r\r\r\r\r\r\r\r\r\r\r\r\r\r\r\r", "ExpectedValue"=""}, {"Test_Name"="630. CheckCanRxStatus \"0\"", "Step_Type"="StringValueTest", "LowLimit"=0.0, "HighLimit"=0.0, "RValue"="0", "RStatus"="PASS", "RetVal"="0", "Units"="", "header1"="", "header2"="---VCOMM and MUX 2A & 2B and Internal J1850 and CAN 1 transciever Rx---\r\r\r\r\r\r\r\r\r\r\r\r\r\r\r\r\r\r\r\r\r\r\r\r\r\r\r\r\r\r\r\r\r\r\r\r\r\r\r\r\r\r\r\r\r\r\r\r\r\r\r\r\r\r\r\r\r\r\r\r\r\r\r\r\r\r\r\r\r\r\r\r\r\r\r\r\r\r\r\r\r\r\r\r\r\r\r\r\r\r\r\r\r\r\r\r\r\r\r\r\r\r", "ExpectedValue"=""}, {"Test_Name"="631. SetAsicRegister \"1\" \"0\" \"00\"", "Step_Type"="", "LowLimit"=0.0, "HighLimit"=0.0, "RValue"="", "RStatus"="", "RetVal"="0", "Units"="", "header1"="", "header2"="---VCOMM and MUX 2A & 2B and Internal J1850 and CAN 1 transciever Rx---\r\r\r\r\r\r\r\r\r\r\r\r\r\r\r\r\r\r\r\r\r\r\r\r\r\r\r\r\r\r\r\r\r\r\r\r\r\r\r\r\r\r\r\r\r\r\r\r\r\r\r\r\r\r\r\r\r\r\r\r\r\r\r\r\r\r\r\r\r\r\r\r\r\r\r\r\r\r\r\r\r\r\r\r\r\r\r\r\r\r\r\r\r\r\r\r\r\r\r\r\r\r\r", "ExpectedValue"=""}, {"Test_Name"="632. SetAsicRegister \"1\" \"2\" \"00\"", "Step_Type"="", "LowLimit"=0.0, "HighLimit"=0.0, "RValue"="", "RStatus"="", "RetVal"="0", "Units"="", "header1"="", "header2"="---VCOMM and MUX 2A & 2B and Internal J1850 and CAN 1 transciever Rx---\r\r\r\r\r\r\r\r\r\r\r\r\r\r\r\r\r\r\r\r\r\r\r\r\r\r\r\r\r\r\r\r\r\r\r\r\r\r\r\r\r\r\r\r\r\r\r\r\r\r\r\r\r\r\r\r\r\r\r\r\r\r\r\r\r\r\r\r\r\r\r\r\r\r\r\r\r\r\r\r\r\r\r\r\r\r\r\r\r\r\r\r\r\r\r\r\r\r\r\r\r\r\r\r", "ExpectedValue"=""}, {"Test_Name"="633. SetFpgaRegister \"839\" \"00\"", "Step_Type"="", "LowLimit"=0.0, "HighLimit"=0.0, "RValue"="", "RStatus"="", "RetVal"="0", "Units"="", "header1"="", "header2"="---VCOMM and MUX 2A & 2B and Internal J1850 and CAN 1 transciever Rx---\r\r\r\r\r\r\r\r\r\r\r\r\r\r\r\r\r\r\r\r\r\r\r\r\r\r\r\r\r\r\r\r\r\r\r\r\r\r\r\r\r\r\r\r\r\r\r\r\r\r\r\r\r\r\r\r\r\r\r\r\r\r\r\r\r\r\r\r\r\r\r\r\r\r\r\r\r\r\r\r\r\r\r\r\r\r\r\r\r\r\r\r\r\r\r\r\r\r\r\r\r\r\r\r\r", "ExpectedValue"=""}, {"Test_Name"="634. SetFpgaRegister \"89E\" \"00\"", "Step_Type"="", "LowLimit"=0.0, "HighLimit"=0.0, "RValue"="", "RStatus"="", "RetVal"="0", "Units"="", "header1"="", "header2"="---VCOMM and MUX 2A & 2B and Internal J1850 and CAN 1 transciever Rx---\r\r\r\r\r\r\r\r\r\r\r\r\r\r\r\r\r\r\r\r\r\r\r\r\r\r\r\r\r\r\r\r\r\r\r\r\r\r\r\r\r\r\r\r\r\r\r\r\r\r\r\r\r\r\r\r\r\r\r\r\r\r\r\r\r\r\r\r\r\r\r\r\r\r\r\r\r\r\r\r\r\r\r\r\r\r\r\r\r\r\r\r\r\r\r\r\r\r\r\r\r\r\r\r\r\r", "ExpectedValue"=""}, {"Test_Name"="635. SetCANGpioMode \"0\"", "Step_Type"="", "LowLimit"=0.0, "HighLimit"=0.0, "RValue"="", "RStatus"="", "RetVal"="0", "Units"="", "header1"="", "header2"="---VCOMM and MUX 2A & 2B and Internal J1850 and CAN 1 transciever Rx---\r\r\r\r\r\r\r\r\r\r\r\r\r\r\r\r\r\r\r\r\r\r\r\r\r\r\r\r\r\r\r\r\r\r\r\r\r\r\r\r\r\r\r\r\r\r\r\r\r\r\r\r\r\r\r\r\r\r\r\r\r\r\r\r\r\r\r\r\r\r\r\r\r\r\r\r\r\r\r\r\r\r\r\r\r\r\r\r\r\r\r\r\r\r\r\r\r\r\r\r\r\r\r\r\r\r\r", "ExpectedValue"=""}, {"Test_Name"="637. SetG15PullUp \"A\" \"0\"", "Step_Type"="", "LowLimit"=0.0, "HighLimit"=0.0, "RValue"="", "RStatus"="", "RetVal"="0", "Units"="", "header1"="", "header2"="---VCOMM and MUX 2A & 2B and Internal J1850 and CAN 1 transciever Rx---\r\r\r\r\r\r\r\r\r\r\r\r\r\r\r\r\r\r\r\r\r\r\r\r\r\r\r\r\r\r\r\r\r\r\r\r\r\r\r\r\r\r\r\r\r\r\r\r\r\r\r\r\r\r\r\r\r\r\r\r\r\r\r\r\r\r\r\r\r\r\r\r\r\r\r\r\r\r\r\r\r\r\r\r\r\r\r\r\r\r\r\r\r\r\r\r\r\r\r\r\r\r\r\r\r\r\r\r", "ExpectedValue"=""}, {"Test_Name"="638. SetG15PullUp \"B\" \"0\"", "Step_Type"="", "LowLimit"=0.0, "HighLimit"=0.0, "RValue"="", "RStatus"="", "RetVal"="0", "Units"="", "header1"="", "header2"="---VCOMM and MUX 2A & 2B and Internal J1850 and CAN 1 transciever Rx---\r\r\r\r\r\r\r\r\r\r\r\r\r\r\r\r\r\r\r\r\r\r\r\r\r\r\r\r\r\r\r\r\r\r\r\r\r\r\r\r\r\r\r\r\r\r\r\r\r\r\r\r\r\r\r\r\r\r\r\r\r\r\r\r\r\r\r\r\r\r\r\r\r\r\r\r\r\r\r\r\r\r\r\r\r\r\r\r\r\r\r\r\r\r\r\r\r\r\r\r\r\r\r\r\r\r\r\r\r", "ExpectedValue"=""}, {"Test_Name"="639. SetG15PullDown \"A\" \"0\"", "Step_Type"="", "LowLimit"=0.0, "HighLimit"=0.0, "RValue"="", "RStatus"="", "RetVal"="0", "Units"="", "header1"="", "header2"="---VCOMM and MUX 2A & 2B and Internal J1850 and CAN 1 transciever Rx---\r\r\r\r\r\r\r\r\r\r\r\r\r\r\r\r\r\r\r\r\r\r\r\r\r\r\r\r\r\r\r\r\r\r\r\r\r\r\r\r\r\r\r\r\r\r\r\r\r\r\r\r\r\r\r\r\r\r\r\r\r\r\r\r\r\r\r\r\r\r\r\r\r\r\r\r\r\r\r\r\r\r\r\r\r\r\r\r\r\r\r\r\r\r\r\r\r\r\r\r\r\r\r\r\r\r\r\r\r\r", "ExpectedValue"=""}, {"Test_Name"="640. SetG15PullDown \"B\" \"0\"", "Step_Type"="", "LowLimit"=0.0, "HighLimit"=0.0, "RValue"="", "RStatus"="", "RetVal"="0", "Units"="", "header1"="", "header2"="---VCOMM and MUX 2A & 2B and Internal J1850 and CAN 1 transciever Rx---\r\r\r\r\r\r\r\r\r\r\r\r\r\r\r\r\r\r\r\r\r\r\r\r\r\r\r\r\r\r\r\r\r\r\r\r\r\r\r\r\r\r\r\r\r\r\r\r\r\r\r\r\r\r\r\r\r\r\r\r\r\r\r\r\r\r\r\r\r\r\r\r\r\r\r\r\r\r\r\r\r\r\r\r\r\r\r\r\r\r\r\r\r\r\r\r\r\r\r\r\r\r\r\r\r\r\r\r\r\r\r", "ExpectedValue"=""}, {"Test_Name"="642. === CCD overvoltage protection test ===", "Step_Type"="", "LowLimit"=0.0, "HighLimit"=0.0, "RValue"="", "RStatus"="", "RetVal"="", "Units"="", "header1"="=== CCD overvoltage protection test ====", "header2"="---VCOMM and MUX 2A & 2B and Internal J1850 and CAN 1 transciever Rx---\r\r\r\r\r\r\r\r\r\r\r\r\r\r\r\r\r\r\r\r\r\r\r\r\r\r\r\r\r\r\r\r\r\r\r\r\r\r\r\r\r\r\r\r\r\r\r\r\r\r\r\r\r\r\r\r\r\r\r\r\r\r\r\r\r\r\r\r\r\r\r\r\r\r\r\r\r\r\r\r\r\r\r\r\r\r\r\r\r\r\r\r\r\r\r\r\r\r\r\r\r\r\r\r\r\r\r\r\r\r\r\r", "ExpectedValue"=""}, {"Test_Name"="646. SetG15PullDown \"A\" \"4\"", "Step_Type"="", "LowLimit"=0.0, "HighLimit"=0.0, "RValue"="", "RStatus"="", "RetVal"="0", "Units"="", "header1"="=== CCD overvoltage protection test ====", "header2"="---VCOMM and MUX 2A & 2B and Internal J1850 and CAN 1 transciever Rx---\r\r\r\r\r\r\r\r\r\r\r\r\r\r\r\r\r\r\r\r\r\r\r\r\r\r\r\r\r\r\r\r\r\r\r\r\r\r\r\r\r\r\r\r\r\r\r\r\r\r\r\r\r\r\r\r\r\r\r\r\r\r\r\r\r\r\r\r\r\r\r\r\r\r\r\r\r\r\r\r\r\r\r\r\r\r\r\r\r\r\r\r\r\r\r\r\r\r\r\r\r\r\r\r\r\r\r\r\r\r\r\r\r", "ExpectedValue"=""}, {"Test_Name"="647. SetG15PullUp \"B\" \"9\"", "Step_Type"="", "LowLimit"=0.0, "HighLimit"=0.0, "RValue"="", "RStatus"="", "RetVal"="0", "Units"="", "header1"="=== CCD overvoltage protection test ====", "header2"="---VCOMM and MUX 2A & 2B and Internal J1850 and CAN 1 transciever Rx---\r\r\r\r\r\r\r\r\r\r\r\r\r\r\r\r\r\r\r\r\r\r\r\r\r\r\r\r\r\r\r\r\r\r\r\r\r\r\r\r\r\r\r\r\r\r\r\r\r\r\r\r\r\r\r\r\r\r\r\r\r\r\r\r\r\r\r\r\r\r\r\r\r\r\r\r\r\r\r\r\r\r\r\r\r\r\r\r\r\r\r\r\r\r\r\r\r\r\r\r\r\r\r\r\r\r\r\r\r\r\r\r\r\r", "ExpectedValue"=""}, {"Test_Name"="648. SetG15PullDown \"B\" \"4\"", "Step_Type"="", "LowLimit"=0.0, "HighLimit"=0.0, "RValue"="", "RStatus"="", "RetVal"="0", "Units"="", "header1"="=== CCD overvoltage protection test ====", "header2"="---VCOMM and MUX 2A & 2B and Internal J1850 and CAN 1 transciever Rx---\r\r\r\r\r\r\r\r\r\r\r\r\r\r\r\r\r\r\r\r\r\r\r\r\r\r\r\r\r\r\r\r\r\r\r\r\r\r\r\r\r\r\r\r\r\r\r\r\r\r\r\r\r\r\r\r\r\r\r\r\r\r\r\r\r\r\r\r\r\r\r\r\r\r\r\r\r\r\r\r\r\r\r\r\r\r\r\r\r\r\r\r\r\r\r\r\r\r\r\r\r\r\r\r\r\r\r\r\r\r\r\r\r\r\r", "ExpectedValue"=""}, {"Test_Name"="650. SetAsicRegister \"1\" \"0\" \"40\"", "Step_Type"="", "LowLimit"=0.0, "HighLimit"=0.0, "RValue"="", "RStatus"="", "RetVal"="0", "Units"="", "header1"="=== CCD overvoltage protection test ====", "header2"="---VCOMM and MUX 2A & 2B and Internal J1850 and CAN 1 transciever Rx---\r\r\r\r\r\r\r\r\r\r\r\r\r\r\r\r\r\r\r\r\r\r\r\r\r\r\r\r\r\r\r\r\r\r\r\r\r\r\r\r\r\r\r\r\r\r\r\r\r\r\r\r\r\r\r\r\r\r\r\r\r\r\r\r\r\r\r\r\r\r\r\r\r\r\r\r\r\r\r\r\r\r\r\r\r\r\r\r\r\r\r\r\r\r\r\r\r\r\r\r\r\r\r\r\r\r\r\r\r\r\r\r\r\r\r\r", "ExpectedValue"=""}, {"Test_Name"="651. SetAsicRegister \"1\" \"2\" \"40\"", "Step_Type"="", "LowLimit"=0.0, "HighLimit"=0.0, "RValue"="", "RStatus"="", "RetVal"="0", "Units"="", "header1"="=== CCD overvoltage protection test ====", "header2"="---VCOMM and MUX 2A & 2B and Internal J1850 and CAN 1 transciever Rx---\r\r\r\r\r\r\r\r\r\r\r\r\r\r\r\r\r\r\r\r\r\r\r\r\r\r\r\r\r\r\r\r\r\r\r\r\r\r\r\r\r\r\r\r\r\r\r\r\r\r\r\r\r\r\r\r\r\r\r\r\r\r\r\r\r\r\r\r\r\r\r\r\r\r\r\r\r\r\r\r\r\r\r\r\r\r\r\r\r\r\r\r\r\r\r\r\r\r\r\r\r\r\r\r\r\r\r\r\r\r\r\r\r\r\r\r\r", "ExpectedValue"=""}, {"Test_Name"="654. SetFpgaRegister \"630\" \"00\"", "Step_Type"="", "LowLimit"=0.0, "HighLimit"=0.0, "RValue"="", "RStatus"="", "RetVal"="0", "Units"="", "header1"="=== CCD overvoltage protection test ====", "header2"="---VCOMM and MUX 2A & 2B and Internal J1850 and CAN 1 transciever Rx---\r\r\r\r\r\r\r\r\r\r\r\r\r\r\r\r\r\r\r\r\r\r\r\r\r\r\r\r\r\r\r\r\r\r\r\r\r\r\r\r\r\r\r\r\r\r\r\r\r\r\r\r\r\r\r\r\r\r\r\r\r\r\r\r\r\r\r\r\r\r\r\r\r\r\r\r\r\r\r\r\r\r\r\r\r\r\r\r\r\r\r\r\r\r\r\r\r\r\r\r\r\r\r\r\r\r\r\r\r\r\r\r\r\r\r\r\r\r", "ExpectedValue"=""}, {"Test_Name"="655. CheckCFAdc \"PD1\" \"-.15\" \".3\"", "Step_Type"="NumericLimitTest", "LowLimit"=-0.15, "HighLimit"=0.3, "RValue"="0.035999998450279236", "RStatus"="PASS", "RetVal"="0", "Units"="Volts", "header1"="=== CCD overvoltage protection test ====", "header2"="---VCOMM and MUX 2A & 2B and Internal J1850 and CAN 1 transciever Rx---\r\r\r\r\r\r\r\r\r\r\r\r\r\r\r\r\r\r\r\r\r\r\r\r\r\r\r\r\r\r\r\r\r\r\r\r\r\r\r\r\r\r\r\r\r\r\r\r\r\r\r\r\r\r\r\r\r\r\r\r\r\r\r\r\r\r\r\r\r\r\r\r\r\r\r\r\r\r\r\r\r\r\r\r\r\r\r\r\r\r\r\r\r\r\r\r\r\r\r\r\r\r\r\r\r\r\r\r\r\r\r\r\r\r\r\r\r\r\r", "ExpectedValue"=""}, {"Test_Name"="656. CheckCFAdc \"PD2\" \"2.2\" \"2.65\"", "Step_Type"="NumericLimitTest", "LowLimit"=2.2, "HighLimit"=2.65, "RValue"="2.4549999237060547", "RStatus"="PASS", "RetVal"="0", "Units"="Volts", "header1"="=== CCD overvoltage protection test ====", "header2"="---VCOMM and MUX 2A & 2B and Internal J1850 and CAN 1 transciever Rx---\r\r\r\r\r\r\r\r\r\r\r\r\r\r\r\r\r\r\r\r\r\r\r\r\r\r\r\r\r\r\r\r\r\r\r\r\r\r\r\r\r\r\r\r\r\r\r\r\r\r\r\r\r\r\r\r\r\r\r\r\r\r\r\r\r\r\r\r\r\r\r\r\r\r\r\r\r\r\r\r\r\r\r\r\r\r\r\r\r\r\r\r\r\r\r\r\r\r\r\r\r\r\r\r\r\r\r\r\r\r\r\r\r\r\r\r\r\r\r\r", "ExpectedValue"=""}, {"Test_Name"="658. SetFpgaRegister \"630\" \"04\"", "Step_Type"="", "LowLimit"=0.0, "HighLimit"=0.0, "RValue"="", "RStatus"="", "RetVal"="0", "Units"="", "header1"="=== CCD overvoltage protection test ====", "header2"="---VCOMM and MUX 2A & 2B and Internal J1850 and CAN 1 transciever Rx---\r\r\r\r\r\r\r\r\r\r\r\r\r\r\r\r\r\r\r\r\r\r\r\r\r\r\r\r\r\r\r\r\r\r\r\r\r\r\r\r\r\r\r\r\r\r\r\r\r\r\r\r\r\r\r\r\r\r\r\r\r\r\r\r\r\r\r\r\r\r\r\r\r\r\r\r\r\r\r\r\r\r\r\r\r\r\r\r\r\r\r\r\r\r\r\r\r\r\r\r\r\r\r\r\r\r\r\r\r\r\r\r\r\r\r\r\r\r\r\r\r", "ExpectedValue"=""}, {"Test_Name"="659. CheckCFAdc \"PD1\" \"4.4\" \"4.9\"", "Step_Type"="NumericLimitTest", "LowLimit"=4.4, "HighLimit"=4.9, "RValue"="4.618000030517578", "RStatus"="PASS", "RetVal"="0", "Units"="Volts", "header1"="=== CCD overvoltage protection test ====", "header2"="---VCOMM and MUX 2A & 2B and Internal J1850 and CAN 1 transciever Rx---\r\r\r\r\r\r\r\r\r\r\r\r\r\r\r\r\r\r\r\r\r\r\r\r\r\r\r\r\r\r\r\r\r\r\r\r\r\r\r\r\r\r\r\r\r\r\r\r\r\r\r\r\r\r\r\r\r\r\r\r\r\r\r\r\r\r\r\r\r\r\r\r\r\r\r\r\r\r\r\r\r\r\r\r\r\r\r\r\r\r\r\r\r\r\r\r\r\r\r\r\r\r\r\r\r\r\r\r\r\r\r\r\r\r\r\r\r\r\r\r\r\r", "ExpectedValue"=""}, {"Test_Name"="660. CheckCFAdc \"PD2\" \".2\" \".6\"", "Step_Type"="NumericLimitTest", "LowLimit"=0.2, "HighLimit"=0.6, "RValue"="0.3959999978542328", "RStatus"="PASS", "RetVal"="0", "Units"="Volts", "header1"="=== CCD overvoltage protection test ====", "header2"="---VCOMM and MUX 2A & 2B and Internal J1850 and CAN 1 transciever Rx---\r\r\r\r\r\r\r\r\r\r\r\r\r\r\r\r\r\r\r\r\r\r\r\r\r\r\r\r\r\r\r\r\r\r\r\r\r\r\r\r\r\r\r\r\r\r\r\r\r\r\r\r\r\r\r\r\r\r\r\r\r\r\r\r\r\r\r\r\r\r\r\r\r\r\r\r\r\r\r\r\r\r\r\r\r\r\r\r\r\r\r\r\r\r\r\r\r\r\r\r\r\r\r\r\r\r\r\r\r\r\r\r\r\r\r\r\r\r\r\r\r\r\r", "ExpectedValue"=""}, {"Test_Name"="663. SetFpgaRegister \"630\" \"00\"", "Step_Type"="", "LowLimit"=0.0, "HighLimit"=0.0, "RValue"="", "RStatus"="", "RetVal"="0", "Units"="", "header1"="=== CCD overvoltage protection test ====", "header2"="---VCOMM and MUX 2A & 2B and Internal J1850 and CAN 1 transciever Rx---\r\r\r\r\r\r\r\r\r\r\r\r\r\r\r\r\r\r\r\r\r\r\r\r\r\r\r\r\r\r\r\r\r\r\r\r\r\r\r\r\r\r\r\r\r\r\r\r\r\r\r\r\r\r\r\r\r\r\r\r\r\r\r\r\r\r\r\r\r\r\r\r\r\r\r\r\r\r\r\r\r\r\r\r\r\r\r\r\r\r\r\r\r\r\r\r\r\r\r\r\r\r\r\r\r\r\r\r\r\r\r\r\r\r\r\r\r\r\r\r\r\r\r\r", "ExpectedValue"=""}, {"Test_Name"="664. SetG15PullupVbat \"0\" \"1\"", "Step_Type"="", "LowLimit"=0.0, "HighLimit"=0.0, "RValue"="", "RStatus"="", "RetVal"="0", "Units"="", "header1"="=== CCD overvoltage protection test ====", "header2"="---VCOMM and MUX 2A & 2B and Internal J1850 and CAN 1 transciever Rx---\r\r\r\r\r\r\r\r\r\r\r\r\r\r\r\r\r\r\r\r\r\r\r\r\r\r\r\r\r\r\r\r\r\r\r\r\r\r\r\r\r\r\r\r\r\r\r\r\r\r\r\r\r\r\r\r\r\r\r\r\r\r\r\r\r\r\r\r\r\r\r\r\r\r\r\r\r\r\r\r\r\r\r\r\r\r\r\r\r\r\r\r\r\r\r\r\r\r\r\r\r\r\r\r\r\r\r\r\r\r\r\r\r\r\r\r\r\r\r\r\r\r\r\r\r", "ExpectedValue"=""}, {"Test_Name"="665. Pause \"500\"", "Step_Type"="", "LowLimit"=0.0, "HighLimit"=0.0, "RValue"="", "RStatus"="", "RetVal"="0", "Units"="", "header1"="=== CCD overvoltage protection test ====", "header2"="---VCOMM and MUX 2A & 2B and Internal J1850 and CAN 1 transciever Rx---\r\r\r\r\r\r\r\r\r\r\r\r\r\r\r\r\r\r\r\r\r\r\r\r\r\r\r\r\r\r\r\r\r\r\r\r\r\r\r\r\r\r\r\r\r\r\r\r\r\r\r\r\r\r\r\r\r\r\r\r\r\r\r\r\r\r\r\r\r\r\r\r\r\r\r\r\r\r\r\r\r\r\r\r\r\r\r\r\r\r\r\r\r\r\r\r\r\r\r\r\r\r\r\r\r\r\r\r\r\r\r\r\r\r\r\r\r\r\r\r\r\r\r\r\r\r", "ExpectedValue"=""}, {"Test_Name"="666. SetFpgaRegister \"630\" \"04\"", "Step_Type"="", "LowLimit"=0.0, "HighLimit"=0.0, "RValue"="", "RStatus"="", "RetVal"="0", "Units"="", "header1"="=== CCD overvoltage protection test ====", "header2"="---VCOMM and MUX 2A & 2B and Internal J1850 and CAN 1 transciever Rx---\r\r\r\r\r\r\r\r\r\r\r\r\r\r\r\r\r\r\r\r\r\r\r\r\r\r\r\r\r\r\r\r\r\r\r\r\r\r\r\r\r\r\r\r\r\r\r\r\r\r\r\r\r\r\r\r\r\r\r\r\r\r\r\r\r\r\r\r\r\r\r\r\r\r\r\r\r\r\r\r\r\r\r\r\r\r\r\r\r\r\r\r\r\r\r\r\r\r\r\r\r\r\r\r\r\r\r\r\r\r\r\r\r\r\r\r\r\r\r\r\r\r\r\r\r\r\r", "ExpectedValue"=""}, {"Test_Name"="667. CheckCFAdc \"PD1\" \"-.15\" \".3\"", "Step_Type"="NumericLimitTest", "LowLimit"=-0.15, "HighLimit"=0.3, "RValue"="0.035999998450279236", "RStatus"="PASS", "RetVal"="0", "Units"="Volts", "header1"="=== CCD overvoltage protection test ====", "header2"="---VCOMM and MUX 2A & 2B and Internal J1850 and CAN 1 transciever Rx---\r\r\r\r\r\r\r\r\r\r\r\r\r\r\r\r\r\r\r\r\r\r\r\r\r\r\r\r\r\r\r\r\r\r\r\r\r\r\r\r\r\r\r\r\r\r\r\r\r\r\r\r\r\r\r\r\r\r\r\r\r\r\r\r\r\r\r\r\r\r\r\r\r\r\r\r\r\r\r\r\r\r\r\r\r\r\r\r\r\r\r\r\r\r\r\r\r\r\r\r\r\r\r\r\r\r\r\r\r\r\r\r\r\r\r\r\r\r\r\r\r\r\r\r\r\r\r\r", "ExpectedValue"=""}, {"Test_Name"="668. CheckCFAdc \"PD2\" \"6.9\" \"7.7\"", "Step_Type"="NumericLimitTest", "LowLimit"=6.9, "HighLimit"=7.7, "RValue"="7.271999835968018", "RStatus"="PASS", "RetVal"="0", "Units"="Volts", "header1"="=== CCD overvoltage protection test ====", "header2"="---VCOMM and MUX 2A & 2B and Internal J1850 and CAN 1 transciever Rx---\r\r\r\r\r\r\r\r\r\r\r\r\r\r\r\r\r\r\r\r\r\r\r\r\r\r\r\r\r\r\r\r\r\r\r\r\r\r\r\r\r\r\r\r\r\r\r\r\r\r\r\r\r\r\r\r\r\r\r\r\r\r\r\r\r\r\r\r\r\r\r\r\r\r\r\r\r\r\r\r\r\r\r\r\r\r\r\r\r\r\r\r\r\r\r\r\r\r\r\r\r\r\r\r\r\r\r\r\r\r\r\r\r\r\r\r\r\r\r\r\r\r\r\r\r\r\r\r\r", "ExpectedValue"=""}, {"Test_Name"="669. SetG15PullupVbat \"0\" \"0\"", "Step_Type"="", "LowLimit"=0.0, "HighLimit"=0.0, "RValue"="", "RStatus"="", "RetVal"="0", "Units"="", "header1"="=== CCD overvoltage protection test ====", "header2"="---VCOMM and MUX 2A & 2B and Internal J1850 and CAN 1 transciever Rx---\r\r\r\r\r\r\r\r\r\r\r\r\r\r\r\r\r\r\r\r\r\r\r\r\r\r\r\r\r\r\r\r\r\r\r\r\r\r\r\r\r\r\r\r\r\r\r\r\r\r\r\r\r\r\r\r\r\r\r\r\r\r\r\r\r\r\r\r\r\r\r\r\r\r\r\r\r\r\r\r\r\r\r\r\r\r\r\r\r\r\r\r\r\r\r\r\r\r\r\r\r\r\r\r\r\r\r\r\r\r\r\r\r\r\r\r\r\r\r\r\r\r\r\r\r\r\r\r\r\r", "ExpectedValue"=""}, {"Test_Name"="671. SetFpgaRegister \"630\" \"00\"", "Step_Type"="", "LowLimit"=0.0, "HighLimit"=0.0, "RValue"="", "RStatus"="", "RetVal"="0", "Units"="", "header1"="=== CCD overvoltage protection test ====", "header2"="---VCOMM and MUX 2A & 2B and Internal J1850 and CAN 1 transciever Rx---\r\r\r\r\r\r\r\r\r\r\r\r\r\r\r\r\r\r\r\r\r\r\r\r\r\r\r\r\r\r\r\r\r\r\r\r\r\r\r\r\r\r\r\r\r\r\r\r\r\r\r\r\r\r\r\r\r\r\r\r\r\r\r\r\r\r\r\r\r\r\r\r\r\r\r\r\r\r\r\r\r\r\r\r\r\r\r\r\r\r\r\r\r\r\r\r\r\r\r\r\r\r\r\r\r\r\r\r\r\r\r\r\r\r\r\r\r\r\r\r\r\r\r\r\r\r\r\r\r\r\r", "ExpectedValue"=""}, {"Test_Name"="672. ReadFpgaRegister \"632\"", "Step_Type"="", "LowLimit"=0.0, "HighLimit"=0.0, "RValue"="7", "RStatus"="", "RetVal"="0", "Units"="", "header1"="=== CCD overvoltage protection test ====", "header2"="---VCOMM and MUX 2A & 2B and Internal J1850 and CAN 1 transciever Rx---\r\r\r\r\r\r\r\r\r\r\r\r\r\r\r\r\r\r\r\r\r\r\r\r\r\r\r\r\r\r\r\r\r\r\r\r\r\r\r\r\r\r\r\r\r\r\r\r\r\r\r\r\r\r\r\r\r\r\r\r\r\r\r\r\r\r\r\r\r\r\r\r\r\r\r\r\r\r\r\r\r\r\r\r\r\r\r\r\r\r\r\r\r\r\r\r\r\r\r\r\r\r\r\r\r\r\r\r\r\r\r\r\r\r\r\r\r\r\r\r\r\r\r\r\r\r\r\r\r\r\r\r", "ExpectedValue"=""}, {"Test_Name"="673. ReadFpgaRegister \"630\"", "Step_Type"="", "LowLimit"=0.0, "HighLimit"=0.0, "RValue"="0", "RStatus"="", "RetVal"="0", "Units"="", "header1"="=== CCD overvoltage protection test ====", "header2"="---VCOMM and MUX 2A & 2B and Internal J1850 and CAN 1 transciever Rx---\r\r\r\r\r\r\r\r\r\r\r\r\r\r\r\r\r\r\r\r\r\r\r\r\r\r\r\r\r\r\r\r\r\r\r\r\r\r\r\r\r\r\r\r\r\r\r\r\r\r\r\r\r\r\r\r\r\r\r\r\r\r\r\r\r\r\r\r\r\r\r\r\r\r\r\r\r\r\r\r\r\r\r\r\r\r\r\r\r\r\r\r\r\r\r\r\r\r\r\r\r\r\r\r\r\r\r\r\r\r\r\r\r\r\r\r\r\r\r\r\r\r\r\r\r\r\r\r\r\r\r\r\r", "ExpectedValue"=""}, {"Test_Name"="674. SetG15PullUp \"A\" \"0\"", "Step_Type"="", "LowLimit"=0.0, "HighLimit"=0.0, "RValue"="", "RStatus"="", "RetVal"="0", "Units"="", "header1"="=== CCD overvoltage protection test ====", "header2"="---VCOMM and MUX 2A & 2B and Internal J1850 and CAN 1 transciever Rx---\r\r\r\r\r\r\r\r\r\r\r\r\r\r\r\r\r\r\r\r\r\r\r\r\r\r\r\r\r\r\r\r\r\r\r\r\r\r\r\r\r\r\r\r\r\r\r\r\r\r\r\r\r\r\r\r\r\r\r\r\r\r\r\r\r\r\r\r\r\r\r\r\r\r\r\r\r\r\r\r\r\r\r\r\r\r\r\r\r\r\r\r\r\r\r\r\r\r\r\r\r\r\r\r\r\r\r\r\r\r\r\r\r\r\r\r\r\r\r\r\r\r\r\r\r\r\r\r\r\r\r\r\r\r", "ExpectedValue"=""}, {"Test_Name"="675. SetG15PullUp \"B\" \"0\"", "Step_Type"="", "LowLimit"=0.0, "HighLimit"=0.0, "RValue"="", "RStatus"="", "RetVal"="0", "Units"="", "header1"="=== CCD overvoltage protection test ====", "header2"="---VCOMM and MUX 2A & 2B and Internal J1850 and CAN 1 transciever Rx---\r\r\r\r\r\r\r\r\r\r\r\r\r\r\r\r\r\r\r\r\r\r\r\r\r\r\r\r\r\r\r\r\r\r\r\r\r\r\r\r\r\r\r\r\r\r\r\r\r\r\r\r\r\r\r\r\r\r\r\r\r\r\r\r\r\r\r\r\r\r\r\r\r\r\r\r\r\r\r\r\r\r\r\r\r\r\r\r\r\r\r\r\r\r\r\r\r\r\r\r\r\r\r\r\r\r\r\r\r\r\r\r\r\r\r\r\r\r\r\r\r\r\r\r\r\r\r\r\r\r\r\r\r\r\r", "ExpectedValue"=""}, {"Test_Name"="676. SetG15PullDown \"A\" \"0\"", "Step_Type"="", "LowLimit"=0.0, "HighLimit"=0.0, "RValue"="", "RStatus"="", "RetVal"="0", "Units"="", "header1"="=== CCD overvoltage protection test ====", "header2"="---VCOMM and MUX 2A & 2B and Internal J1850 and CAN 1 transciever Rx---\r\r\r\r\r\r\r\r\r\r\r\r\r\r\r\r\r\r\r\r\r\r\r\r\r\r\r\r\r\r\r\r\r\r\r\r\r\r\r\r\r\r\r\r\r\r\r\r\r\r\r\r\r\r\r\r\r\r\r\r\r\r\r\r\r\r\r\r\r\r\r\r\r\r\r\r\r\r\r\r\r\r\r\r\r\r\r\r\r\r\r\r\r\r\r\r\r\r\r\r\r\r\r\r\r\r\r\r\r\r\r\r\r\r\r\r\r\r\r\r\r\r\r\r\r\r\r\r\r\r\r\r\r\r\r\r", "ExpectedValue"=""}, {"Test_Name"="677. SetG15PullDown \"B\" \"0\"", "Step_Type"="", "LowLimit"=0.0, "HighLimit"=0.0, "RValue"="", "RStatus"="", "RetVal"="0", "Units"="", "header1"="=== CCD overvoltage protection test ====", "header2"="---VCOMM and MUX 2A & 2B and Internal J1850 and CAN 1 transciever Rx---\r\r\r\r\r\r\r\r\r\r\r\r\r\r\r\r\r\r\r\r\r\r\r\r\r\r\r\r\r\r\r\r\r\r\r\r\r\r\r\r\r\r\r\r\r\r\r\r\r\r\r\r\r\r\r\r\r\r\r\r\r\r\r\r\r\r\r\r\r\r\r\r\r\r\r\r\r\r\r\r\r\r\r\r\r\r\r\r\r\r\r\r\r\r\r\r\r\r\r\r\r\r\r\r\r\r\r\r\r\r\r\r\r\r\r\r\r\r\r\r\r\r\r\r\r\r\r\r\r\r\r\r\r\r\r\r\r", "ExpectedValue"=""}, {"Test_Name"="678. SetAsicRegister \"1\" \"0\" \"00\"", "Step_Type"="", "LowLimit"=0.0, "HighLimit"=0.0, "RValue"="", "RStatus"="", "RetVal"="0", "Units"="", "header1"="=== CCD overvoltage protection test ====", "header2"="---VCOMM and MUX 2A & 2B and Internal J1850 and CAN 1 transciever Rx---\r\r\r\r\r\r\r\r\r\r\r\r\r\r\r\r\r\r\r\r\r\r\r\r\r\r\r\r\r\r\r\r\r\r\r\r\r\r\r\r\r\r\r\r\r\r\r\r\r\r\r\r\r\r\r\r\r\r\r\r\r\r\r\r\r\r\r\r\r\r\r\r\r\r\r\r\r\r\r\r\r\r\r\r\r\r\r\r\r\r\r\r\r\r\r\r\r\r\r\r\r\r\r\r\r\r\r\r\r\r\r\r\r\r\r\r\r\r\r\r\r\r\r\r\r\r\r\r\r\r\r\r\r\r\r\r\r\r", "ExpectedValue"=""}, {"Test_Name"="679. SetAsicRegister \"1\" \"2\" \"00\"", "Step_Type"="", "LowLimit"=0.0, "HighLimit"=0.0, "RValue"="", "RStatus"="", "RetVal"="0", "Units"="", "header1"="=== CCD overvoltage protection test ====", "header2"="---VCOMM and MUX 2A & 2B and Internal J1850 and CAN 1 transciever Rx---\r\r\r\r\r\r\r\r\r\r\r\r\r\r\r\r\r\r\r\r\r\r\r\r\r\r\r\r\r\r\r\r\r\r\r\r\r\r\r\r\r\r\r\r\r\r\r\r\r\r\r\r\r\r\r\r\r\r\r\r\r\r\r\r\r\r\r\r\r\r\r\r\r\r\r\r\r\r\r\r\r\r\r\r\r\r\r\r\r\r\r\r\r\r\r\r\r\r\r\r\r\r\r\r\r\r\r\r\r\r\r\r\r\r\r\r\r\r\r\r\r\r\r\r\r\r\r\r\r\r\r\r\r\r\r\r\r\r\r", "ExpectedValue"=""}, {"Test_Name"="683.  ---121ohm PWM terminations S2A ---", "Step_Type"="", "LowLimit"=0.0, "HighLimit"=0.0, "RValue"="", "RStatus"="", "RetVal"="", "Units"="", "header1"="=== CCD overvoltage protection test ====", "header2"="---121ohm PWM terminations S2A ---------\r", "ExpectedValue"=""}, {"Test_Name"="685. SetFpgaRegister \"982\" \"08\"", "Step_Type"="", "LowLimit"=0.0, "HighLimit"=0.0, "RValue"="", "RStatus"="", "RetVal"="0", "Units"="", "header1"="=== CCD overvoltage protection test ====", "header2"="---121ohm PWM terminations S2A ---------\r\r", "ExpectedValue"=""}, {"Test_Name"="686. SetFpgaRegister \"980\" \"10\"", "Step_Type"="", "LowLimit"=0.0, "HighLimit"=0.0, "RValue"="", "RStatus"="", "RetVal"="0", "Units"="", "header1"="=== CCD overvoltage protection test ====", "header2"="---121ohm PWM terminations S2A ---------\r\r\r", "ExpectedValue"=""}, {"Test_Name"="687. SetG15PullUp \"A\" \"1\"", "Step_Type"="", "LowLimit"=0.0, "HighLimit"=0.0, "RValue"="", "RStatus"="", "RetVal"="0", "Units"="", "header1"="=== CCD overvoltage protection test ====", "header2"="---121ohm PWM terminations S2A ---------\r\r\r\r", "ExpectedValue"=""}, {"Test_Name"="688. CheckCFAdc \"PD1\" \"1.0\" \"1.5\"", "Step_Type"="NumericLimitTest", "LowLimit"=1.0, "HighLimit"=1.5, "RValue"="1.3209999799728394", "RStatus"="PASS", "RetVal"="0", "Units"="Volts", "header1"="=== CCD overvoltage protection test ====", "header2"="---121ohm PWM terminations S2A ---------\r\r\r\r\r", "ExpectedValue"=""}, {"Test_Name"="689. CheckCFAdc \"PD2\" \".1\" \"1.0\"", "Step_Type"="NumericLimitTest", "LowLimit"=0.1, "HighLimit"=1.0, "RValue"="0.8859999775886536", "RStatus"="PASS", "RetVal"="0", "Units"="Volts", "header1"="=== CCD overvoltage protection test ====", "header2"="---121ohm PWM terminations S2A ---------\r\r\r\r\r\r", "ExpectedValue"=""}, {"Test_Name"="690. SetG15PullUp \"A\" \"0\"", "Step_Type"="", "LowLimit"=0.0, "HighLimit"=0.0, "RValue"="", "RStatus"="", "RetVal"="0", "Units"="", "header1"="=== CCD overvoltage protection test ====", "header2"="---121ohm PWM terminations S2A ---------\r\r\r\r\r\r\r", "ExpectedValue"=""}, {"Test_Name"="694. SetFpgaRegister \"982\" \"00\"", "Step_Type"="", "LowLimit"=0.0, "HighLimit"=0.0, "RValue"="", "RStatus"="", "RetVal"="0", "Units"="", "header1"="=== CCD overvoltage protection test ====", "header2"="---121ohm PWM terminations S2A ---------\r\r\r\r\r\r\r\r", "ExpectedValue"=""}, {"Test_Name"="695. SetG15PullupVbat \"0\" \"1\"", "Step_Type"="", "LowLimit"=0.0, "HighLimit"=0.0, "RValue"="", "RStatus"="", "RetVal"="0", "Units"="", "header1"="=== CCD overvoltage protection test ====", "header2"="---121ohm PWM terminations S2A ---------\r\r\r\r\r\r\r\r\r", "ExpectedValue"=""}, {"Test_Name"="696. SetG15PullUp \"A\" \"9\"", "Step_Type"="", "LowLimit"=0.0, "HighLimit"=0.0, "RValue"="", "RStatus"="", "RetVal"="0", "Units"="", "header1"="=== CCD overvoltage protection test ====", "header2"="---121ohm PWM terminations S2A ---------\r\r\r\r\r\r\r\r\r\r", "ExpectedValue"=""}, {"Test_Name"="697. SetG15PullDown \"A\" \"4\"", "Step_Type"="", "LowLimit"=0.0, "HighLimit"=0.0, "RValue"="", "RStatus"="", "RetVal"="0", "Units"="", "header1"="=== CCD overvoltage protection test ====", "header2"="---121ohm PWM terminations S2A ---------\r\r\r\r\r\r\r\r\r\r\r", "ExpectedValue"=""}, {"Test_Name"="698. SetFpgaRegister \"982\" \"08\"", "Step_Type"="", "LowLimit"=0.0, "HighLimit"=0.0, "RValue"="", "RStatus"="", "RetVal"="0", "Units"="", "header1"="=== CCD overvoltage protection test ====", "header2"="---121ohm PWM terminations S2A ---------\r\r\r\r\r\r\r\r\r\r\r\r", "ExpectedValue"=""}, {"Test_Name"="699. CheckCFAdc \"PD1\" \"6.9\" \"7.7\"", "Step_Type"="NumericLimitTest", "LowLimit"=6.9, "HighLimit"=7.7, "RValue"="7.269999980926514", "RStatus"="PASS", "RetVal"="0", "Units"="Volts", "header1"="=== CCD overvoltage protection test ====", "header2"="---121ohm PWM terminations S2A ---------\r\r\r\r\r\r\r\r\r\r\r\r\r", "ExpectedValue"=""}, {"Test_Name"="700. SetG15PullupVbat \"0\" \"0\"", "Step_Type"="", "LowLimit"=0.0, "HighLimit"=0.0, "RValue"="", "RStatus"="", "RetVal"="0", "Units"="", "header1"="=== CCD overvoltage protection test ====", "header2"="---121ohm PWM terminations S2A ---------\r\r\r\r\r\r\r\r\r\r\r\r\r\r", "ExpectedValue"=""}, {"Test_Name"="701. SetG15PullUp \"A\" \"0\"", "Step_Type"="", "LowLimit"=0.0, "HighLimit"=0.0, "RValue"="", "RStatus"="", "RetVal"="0", "Units"="", "header1"="=== CCD overvoltage protection test ====", "header2"="---121ohm PWM terminations S2A ---------\r\r\r\r\r\r\r\r\r\r\r\r\r\r\r", "ExpectedValue"=""}, {"Test_Name"="702. SetG15PullDown \"A\" \"0\"", "Step_Type"="", "LowLimit"=0.0, "HighLimit"=0.0, "RValue"="", "RStatus"="", "RetVal"="0", "Units"="", "header1"="=== CCD overvoltage protection test ====", "header2"="---121ohm PWM terminations S2A ---------\r\r\r\r\r\r\r\r\r\r\r\r\r\r\r\r", "ExpectedValue"=""}, {"Test_Name"="705. SetFpgaRegister \"980\" \"20\"", "Step_Type"="", "LowLimit"=0.0, "HighLimit"=0.0, "RValue"="", "RStatus"="", "RetVal"="0", "Units"="", "header1"="=== CCD overvoltage protection test ====", "header2"="---121ohm PWM terminations S2A ---------\r\r\r\r\r\r\r\r\r\r\r\r\r\r\r\r\r", "ExpectedValue"=""}, {"Test_Name"="706. SetG15PullDown \"B\" \"3\"", "Step_Type"="", "LowLimit"=0.0, "HighLimit"=0.0, "RValue"="", "RStatus"="", "RetVal"="0", "Units"="", "header1"="=== CCD overvoltage protection test ====", "header2"="---121ohm PWM terminations S2A ---------\r\r\r\r\r\r\r\r\r\r\r\r\r\r\r\r\r\r", "ExpectedValue"=""}, {"Test_Name"="707. CheckCFAdc \"PD1\" \"-.15\" \".3\"", "Step_Type"="NumericLimitTest", "LowLimit"=-0.15, "HighLimit"=0.3, "RValue"="0.11999999731779099", "RStatus"="PASS", "RetVal"="0", "Units"="Volts", "header1"="=== CCD overvoltage protection test ====", "header2"="---121ohm PWM terminations S2A ---------\r\r\r\r\r\r\r\r\r\r\r\r\r\r\r\r\r\r\r", "ExpectedValue"=""}, {"Test_Name"="708. CheckCFAdc \"PD2\" \"4.4\" \"4.9\"", "Step_Type"="NumericLimitTest", "LowLimit"=4.4, "HighLimit"=4.9, "RValue"="4.623000144958496", "RStatus"="PASS", "RetVal"="0", "Units"="Volts", "header1"="=== CCD overvoltage protection test ====", "header2"="---121ohm PWM terminations S2A ---------\r\r\r\r\r\r\r\r\r\r\r\r\r\r\r\r\r\r\r\r", "ExpectedValue"=""}, {"Test_Name"="709. SetFpgaRegister \"982\" \"00\"", "Step_Type"="", "LowLimit"=0.0, "HighLimit"=0.0, "RValue"="", "RStatus"="", "RetVal"="0", "Units"="", "header1"="=== CCD overvoltage protection test ====", "header2"="---121ohm PWM terminations S2A ---------\r\r\r\r\r\r\r\r\r\r\r\r\r\r\r\r\r\r\r\r\r", "ExpectedValue"=""}, {"Test_Name"="710. CheckCFAdc \"PD2\" \"-.15\" \".3\"", "Step_Type"="NumericLimitTest", "LowLimit"=-0.15, "HighLimit"=0.3, "RValue"="0.017999999225139618", "RStatus"="PASS", "RetVal"="0", "Units"="Volts", "header1"="=== CCD overvoltage protection test ====", "header2"="---121ohm PWM terminations S2A ---------\r\r\r\r\r\r\r\r\r\r\r\r\r\r\r\r\r\r\r\r\r\r", "ExpectedValue"=""}, {"Test_Name"="712. SetG15PullUp \"A\" \"0\"", "Step_Type"="", "LowLimit"=0.0, "HighLimit"=0.0, "RValue"="", "RStatus"="", "RetVal"="0", "Units"="", "header1"="=== CCD overvoltage protection test ====", "header2"="---121ohm PWM terminations S2A ---------\r\r\r\r\r\r\r\r\r\r\r\r\r\r\r\r\r\r\r\r\r\r\r", "ExpectedValue"=""}, {"Test_Name"="713. SetG15PullUp \"B\" \"0\"", "Step_Type"="", "LowLimit"=0.0, "HighLimit"=0.0, "RValue"="", "RStatus"="", "RetVal"="0", "Units"="", "header1"="=== CCD overvoltage protection test ====", "header2"="---121ohm PWM terminations S2A ---------\r\r\r\r\r\r\r\r\r\r\r\r\r\r\r\r\r\r\r\r\r\r\r\r", "ExpectedValue"=""}, {"Test_Name"="714. SetG15PullDown \"A\" \"0\"", "Step_Type"="", "LowLimit"=0.0, "HighLimit"=0.0, "RValue"="", "RStatus"="", "RetVal"="0", "Units"="", "header1"="=== CCD overvoltage protection test ====", "header2"="---121ohm PWM terminations S2A ---------\r\r\r\r\r\r\r\r\r\r\r\r\r\r\r\r\r\r\r\r\r\r\r\r\r", "ExpectedValue"=""}, {"Test_Name"="715. SetG15PullDown \"B\" \"0\"", "Step_Type"="", "LowLimit"=0.0, "HighLimit"=0.0, "RValue"="", "RStatus"="", "RetVal"="0", "Units"="", "header1"="=== CCD overvoltage protection test ====", "header2"="---121ohm PWM terminations S2A ---------\r\r\r\r\r\r\r\r\r\r\r\r\r\r\r\r\r\r\r\r\r\r\r\r\r\r", "ExpectedValue"=""}, {"Test_Name"="717.  ---SW2 CAN2A and CAN2B Can2 Transceiver Rx test---", "Step_Type"="", "LowLimit"=0.0, "HighLimit"=0.0, "RValue"="", "RStatus"="", "RetVal"="", "Units"="", "header1"="=== CCD overvoltage protection test ====", "header2"="---SW2 CAN2A and CAN2B Can2 Transceiver Rx test---\r", "ExpectedValue"=""}, {"Test_Name"="718. SetCANGpioMode \"1\"", "Step_Type"="", "LowLimit"=0.0, "HighLimit"=0.0, "RValue"="", "RStatus"="", "RetVal"="0", "Units"="", "header1"="=== CCD overvoltage protection test ====", "header2"="---SW2 CAN2A and CAN2B Can2 Transceiver Rx test---\r\r", "ExpectedValue"=""}, {"Test_Name"="719. SetFpgaRegister \"839\" \"08\"", "Step_Type"="", "LowLimit"=0.0, "HighLimit"=0.0, "RValue"="", "RStatus"="", "RetVal"="0", "Units"="", "header1"="=== CCD overvoltage protection test ====", "header2"="---SW2 CAN2A and CAN2B Can2 Transceiver Rx test---\r\r\r", "ExpectedValue"=""}, {"Test_Name"="721. SetAsicRegister \"1\" \"4\" \"C0\"", "Step_Type"="", "LowLimit"=0.0, "HighLimit"=0.0, "RValue"="", "RStatus"="", "RetVal"="0", "Units"="", "header1"="=== CCD overvoltage protection test ====", "header2"="---SW2 CAN2A and CAN2B Can2 Transceiver Rx test---\r\r\r\r", "ExpectedValue"=""}, {"Test_Name"="722. SelectMuxA \"1\" \"6\" \"1\"", "Step_Type"="", "LowLimit"=0.0, "HighLimit"=0.0, "RValue"="", "RStatus"="", "RetVal"="0", "Units"="", "header1"="=== CCD overvoltage protection test ====", "header2"="---SW2 CAN2A and CAN2B Can2 Transceiver Rx test---\r\r\r\r\r", "ExpectedValue"=""}, {"Test_Name"="723. SelectMuxB \"1\" \"14\" \"1\"", "Step_Type"="", "LowLimit"=0.0, "HighLimit"=0.0, "RValue"="", "RStatus"="", "RetVal"="0", "Units"="", "header1"="=== CCD overvoltage protection test ====", "header2"="---SW2 CAN2A and CAN2B Can2 Transceiver Rx test---\r\r\r\r\r\r", "ExpectedValue"=""}, {"Test_Name"="724. CheckCFAdc \"PD1\" \"2.3\" \"2.7\"", "Step_Type"="NumericLimitTest", "LowLimit"=2.3, "HighLimit"=2.7, "RValue"="2.558000087738037", "RStatus"="PASS", "RetVal"="0", "Units"="Volts", "header1"="=== CCD overvoltage protection test ====", "header2"="---SW2 CAN2A and CAN2B Can2 Transceiver Rx test---\r\r\r\r\r\r\r", "ExpectedValue"=""}, {"Test_Name"="725. CheckCFAdc \"PD2\" \"2.3\" \"2.7\"", "Step_Type"="NumericLimitTest", "LowLimit"=2.3, "HighLimit"=2.7, "RValue"="2.5929999351501465", "RStatus"="PASS", "RetVal"="0", "Units"="Volts", "header1"="=== CCD overvoltage protection test ====", "header2"="---SW2 CAN2A and CAN2B Can2 Transceiver Rx test---\r\r\r\r\r\r\r\r", "ExpectedValue"=""}, {"Test_Name"="726. SetG15PullUp \"A\" \"2\"", "Step_Type"="", "LowLimit"=0.0, "HighLimit"=0.0, "RValue"="", "RStatus"="", "RetVal"="0", "Units"="", "header1"="=== CCD overvoltage protection test ====", "header2"="---SW2 CAN2A and CAN2B Can2 Transceiver Rx test---\r\r\r\r\r\r\r\r\r", "ExpectedValue"=""}, {"Test_Name"="727. CheckCFAdc \"PD1\" \"4.4\" \"5.0\"", "Step_Type"="NumericLimitTest", "LowLimit"=4.4, "HighLimit"=5.0, "RValue"="4.71999979019165", "RStatus"="PASS", "RetVal"="0", "Units"="Volts", "header1"="=== CCD overvoltage protection test ====", "header2"="---SW2 CAN2A and CAN2B Can2 Transceiver Rx test---\r\r\r\r\r\r\r\r\r\r", "ExpectedValue"=""}, {"Test_Name"="728. Pause 100", "Step_Type"="", "LowLimit"=0.0, "HighLimit"=0.0, "RValue"="", "RStatus"="", "RetVal"="0", "Units"="", "header1"="=== CCD overvoltage protection test ====", "header2"="---SW2 CAN2A and CAN2B Can2 Transceiver Rx test---\r\r\r\r\r\r\r\r\r\r\r", "ExpectedValue"=""}, {"Test_Name"="729. CheckCanRxStatus \"0\"", "Step_Type"="StringValueTest", "LowLimit"=0.0, "HighLimit"=0.0, "RValue"="0", "RStatus"="PASS", "RetVal"="0", "Units"="", "header1"="=== CCD overvoltage protection test ====", "header2"="---SW2 CAN2A and CAN2B Can2 Transceiver Rx test---\r\r\r\r\r\r\r\r\r\r\r\r", "ExpectedValue"=""}, {"Test_Name"="730. SetG15PullDown \"A\" \"5\"", "Step_Type"="", "LowLimit"=0.0, "HighLimit"=0.0, "RValue"="", "RStatus"="", "RetVal"="0", "Units"="", "header1"="=== CCD overvoltage protection test ====", "header2"="---SW2 CAN2A and CAN2B Can2 Transceiver Rx test---\r\r\r\r\r\r\r\r\r\r\r\r\r", "ExpectedValue"=""}, {"Test_Name"="731. CheckCFAdc \"PD1\" \"-.15\" \".3\"", "Step_Type"="NumericLimitTest", "LowLimit"=-0.15, "HighLimit"=0.3, "RValue"="0.017999999225139618", "RStatus"="PASS", "RetVal"="0", "Units"="Volts", "header1"="=== CCD overvoltage protection test ====", "header2"="---SW2 CAN2A and CAN2B Can2 Transceiver Rx test---\r\r\r\r\r\r\r\r\r\r\r\r\r\r", "ExpectedValue"=""}, {"Test_Name"="732. CheckCFAdc \"PD2\" \"2.3\" \"2.7\"", "Step_Type"="NumericLimitTest", "LowLimit"=2.3, "HighLimit"=2.7, "RValue"="2.565000057220459", "RStatus"="PASS", "RetVal"="0", "Units"="Volts", "header1"="=== CCD overvoltage protection test ====", "header2"="---SW2 CAN2A and CAN2B Can2 Transceiver Rx test---\r\r\r\r\r\r\r\r\r\r\r\r\r\r\r", "ExpectedValue"=""}, {"Test_Name"="733. CheckCanRxStatus \"1\"", "Step_Type"="StringValueTest", "LowLimit"=0.0, "HighLimit"=0.0, "RValue"="1", "RStatus"="PASS", "RetVal"="0", "Units"="", "header1"="=== CCD overvoltage protection test ====", "header2"="---SW2 CAN2A and CAN2B Can2 Transceiver Rx test---\r\r\r\r\r\r\r\r\r\r\r\r\r\r\r\r", "ExpectedValue"=""}, {"Test_Name"="734. SetG15PullUp \"A\" \"0\"", "Step_Type"="", "LowLimit"=0.0, "HighLimit"=0.0, "RValue"="", "RStatus"="", "RetVal"="0", "Units"="", "header1"="=== CCD overvoltage protection test ====", "header2"="---SW2 CAN2A and CAN2B Can2 Transceiver Rx test---\r\r\r\r\r\r\r\r\r\r\r\r\r\r\r\r\r", "ExpectedValue"=""}, {"Test_Name"="735. SetG15PullDown \"A\" \"0\"", "Step_Type"="", "LowLimit"=0.0, "HighLimit"=0.0, "RValue"="", "RStatus"="", "RetVal"="0", "Units"="", "header1"="=== CCD overvoltage protection test ====", "header2"="---SW2 CAN2A and CAN2B Can2 Transceiver Rx test---\r\r\r\r\r\r\r\r\r\r\r\r\r\r\r\r\r\r", "ExpectedValue"=""}, {"Test_Name"="736. SetG15PullDown \"B\" \"5\"", "Step_Type"="", "LowLimit"=0.0, "HighLimit"=0.0, "RValue"="", "RStatus"="", "RetVal"="0", "Units"="", "header1"="=== CCD overvoltage protection test ====", "header2"="---SW2 CAN2A and CAN2B Can2 Transceiver Rx test---\r\r\r\r\r\r\r\r\r\r\r\r\r\r\r\r\r\r\r", "ExpectedValue"=""}, {"Test_Name"="737. CheckCFAdc \"PD1\" \"2.3\" \"2.7\"", "Step_Type"="NumericLimitTest", "LowLimit"=2.3, "HighLimit"=2.7, "RValue"="2.5309998989105225", "RStatus"="PASS", "RetVal"="0", "Units"="Volts", "header1"="=== CCD overvoltage protection test ====", "header2"="---SW2 CAN2A and CAN2B Can2 Transceiver Rx test---\r\r\r\r\r\r\r\r\r\r\r\r\r\r\r\r\r\r\r\r", "ExpectedValue"=""}, {"Test_Name"="738. CheckCFAdc \"PD2\" \"-.15\" \".3\"", "Step_Type"="NumericLimitTest", "LowLimit"=-0.15, "HighLimit"=0.3, "RValue"="0.017999999225139618", "RStatus"="PASS", "RetVal"="0", "Units"="Volts", "header1"="=== CCD overvoltage protection test ====", "header2"="---SW2 CAN2A and CAN2B Can2 Transceiver Rx test---\r\r\r\r\r\r\r\r\r\r\r\r\r\r\r\r\r\r\r\r\r", "ExpectedValue"=""}, {"Test_Name"="739. CheckCanRxStatus \"0\"", "Step_Type"="StringValueTest", "LowLimit"=0.0, "HighLimit"=0.0, "RValue"="0", "RStatus"="PASS", "RetVal"="0", "Units"="", "header1"="=== CCD overvoltage protection test ====", "header2"="---SW2 CAN2A and CAN2B Can2 Transceiver Rx test---\r\r\r\r\r\r\r\r\r\r\r\r\r\r\r\r\r\r\r\r\r\r", "ExpectedValue"=""}, {"Test_Name"="741. SetFpgaRegister \"839\" \"0\"", "Step_Type"="", "LowLimit"=0.0, "HighLimit"=0.0, "RValue"="", "RStatus"="", "RetVal"="0", "Units"="", "header1"="=== CCD overvoltage protection test ====", "header2"="---SW2 CAN2A and CAN2B Can2 Transceiver Rx test---\r\r\r\r\r\r\r\r\r\r\r\r\r\r\r\r\r\r\r\r\r\r\r", "ExpectedValue"=""}, {"Test_Name"="742. SetAsicRegister \"1\" \"4\" \"00\"", "Step_Type"="", "LowLimit"=0.0, "HighLimit"=0.0, "RValue"="", "RStatus"="", "RetVal"="0", "Units"="", "header1"="=== CCD overvoltage protection test ====", "header2"="---SW2 CAN2A and CAN2B Can2 Transceiver Rx test---\r\r\r\r\r\r\r\r\r\r\r\r\r\r\r\r\r\r\r\r\r\r\r\r", "ExpectedValue"=""}, {"Test_Name"="743. SetCANGpioMode \"0\"", "Step_Type"="", "LowLimit"=0.0, "HighLimit"=0.0, "RValue"="", "RStatus"="", "RetVal"="0", "Units"="", "header1"="=== CCD overvoltage protection test ====", "header2"="---SW2 CAN2A and CAN2B Can2 Transceiver Rx test---\r\r\r\r\r\r\r\r\r\r\r\r\r\r\r\r\r\r\r\r\r\r\r\r\r", "ExpectedValue"=""}, {"Test_Name"="744. SelectAllMuxA \"1\" \"0\"", "Step_Type"="", "LowLimit"=0.0, "HighLimit"=0.0, "RValue"="", "RStatus"="", "RetVal"="0", "Units"="", "header1"="=== CCD overvoltage protection test ====", "header2"="---SW2 CAN2A and CAN2B Can2 Transceiver Rx test---\r\r\r\r\r\r\r\r\r\r\r\r\r\r\r\r\r\r\r\r\r\r\r\r\r\r", "ExpectedValue"=""}, {"Test_Name"="745. SelectAllMuxB \"1\" \"0\"", "Step_Type"="", "LowLimit"=0.0, "HighLimit"=0.0, "RValue"="", "RStatus"="", "RetVal"="0", "Units"="", "header1"="=== CCD overvoltage protection test ====", "header2"="---SW2 CAN2A and CAN2B Can2 Transceiver Rx test---\r\r\r\r\r\r\r\r\r\r\r\r\r\r\r\r\r\r\r\r\r\r\r\r\r\r\r", "ExpectedValue"=""}, {"Test_Name"="746. SetG15PullUp \"A\" \"0\"", "Step_Type"="", "LowLimit"=0.0, "HighLimit"=0.0, "RValue"="", "RStatus"="", "RetVal"="0", "Units"="", "header1"="=== CCD overvoltage protection test ====", "header2"="---SW2 CAN2A and CAN2B Can2 Transceiver Rx test---\r\r\r\r\r\r\r\r\r\r\r\r\r\r\r\r\r\r\r\r\r\r\r\r\r\r\r\r", "ExpectedValue"=""}, {"Test_Name"="747. SetG15PullUp \"B\" \"0\"", "Step_Type"="", "LowLimit"=0.0, "HighLimit"=0.0, "RValue"="", "RStatus"="", "RetVal"="0", "Units"="", "header1"="=== CCD overvoltage protection test ====", "header2"="---SW2 CAN2A and CAN2B Can2 Transceiver Rx test---\r\r\r\r\r\r\r\r\r\r\r\r\r\r\r\r\r\r\r\r\r\r\r\r\r\r\r\r\r", "ExpectedValue"=""}, {"Test_Name"="748. SetG15PullDown \"A\" \"0\"", "Step_Type"="", "LowLimit"=0.0, "HighLimit"=0.0, "RValue"="", "RStatus"="", "RetVal"="0", "Units"="", "header1"="=== CCD overvoltage protection test ====", "header2"="---SW2 CAN2A and CAN2B Can2 Transceiver Rx test---\r\r\r\r\r\r\r\r\r\r\r\r\r\r\r\r\r\r\r\r\r\r\r\r\r\r\r\r\r\r", "ExpectedValue"=""}, {"Test_Name"="749. SetG15PullDown \"B\" \"0\"", "Step_Type"="", "LowLimit"=0.0, "HighLimit"=0.0, "RValue"="", "RStatus"="", "RetVal"="0", "Units"="", "header1"="=== CCD overvoltage protection test ====", "header2"="---SW2 CAN2A and CAN2B Can2 Transceiver Rx test---\r\r\r\r\r\r\r\r\r\r\r\r\r\r\r\r\r\r\r\r\r\r\r\r\r\r\r\r\r\r\r", "ExpectedValue"=""}, {"Test_Name"="751.  --- SW 1 ---", "Step_Type"="", "LowLimit"=0.0, "HighLimit"=0.0, "RValue"="", "RStatus"="", "RetVal"="", "Units"="", "header1"="=== CCD overvoltage protection test ====", "header2"="--- SW 1 -------------------------------\r", "ExpectedValue"=""}, {"Test_Name"="752. SetFpgaRegister \"89E\" \"40\"", "Step_Type"="", "LowLimit"=0.0, "HighLimit"=0.0, "RValue"="", "RStatus"="", "RetVal"="0", "Units"="", "header1"="=== CCD overvoltage protection test ====", "header2"="--- SW 1 -------------------------------\r\r", "ExpectedValue"=""}, {"Test_Name"="753. SetFpgaRegister \"959\" \"02\"", "Step_Type"="", "LowLimit"=0.0, "HighLimit"=0.0, "RValue"="", "RStatus"="", "RetVal"="0", "Units"="", "header1"="=== CCD overvoltage protection test ====", "header2"="--- SW 1 -------------------------------\r\r\r", "ExpectedValue"=""}, {"Test_Name"="754. SetAsicRegister \"1\" \"4\" \"30\"", "Step_Type"="", "LowLimit"=0.0, "HighLimit"=0.0, "RValue"="", "RStatus"="", "RetVal"="0", "Units"="", "header1"="=== CCD overvoltage protection test ====", "header2"="--- SW 1 -------------------------------\r\r\r\r", "ExpectedValue"=""}, {"Test_Name"="755. SelectMuxA \"1\" \"2\" \"1\"", "Step_Type"="", "LowLimit"=0.0, "HighLimit"=0.0, "RValue"="", "RStatus"="", "RetVal"="0", "Units"="", "header1"="=== CCD overvoltage protection test ====", "header2"="--- SW 1 -------------------------------\r\r\r\r\r", "ExpectedValue"=""}, {"Test_Name"="756. SelectMuxB \"1\" \"10\" \"1\"", "Step_Type"="", "LowLimit"=0.0, "HighLimit"=0.0, "RValue"="", "RStatus"="", "RetVal"="0", "Units"="", "header1"="=== CCD overvoltage protection test ====", "header2"="--- SW 1 -------------------------------\r\r\r\r\r\r", "ExpectedValue"=""}, {"Test_Name"="757. CheckCFAdc \"PD1\" \"-.15\" \".3\"", "Step_Type"="NumericLimitTest", "LowLimit"=-0.15, "HighLimit"=0.3, "RValue"="0.04600000008940697", "RStatus"="PASS", "RetVal"="0", "Units"="Volts", "header1"="=== CCD overvoltage protection test ====", "header2"="--- SW 1 -------------------------------\r\r\r\r\r\r\r", "ExpectedValue"=""}, {"Test_Name"="758. CheckCFAdc \"PD2\" \"7.3\" \"8.0\"", "Step_Type"="NumericLimitTest", "LowLimit"=7.3, "HighLimit"=8.0, "RValue"="7.613999843597412", "RStatus"="PASS", "RetVal"="0", "Units"="Volts", "header1"="=== CCD overvoltage protection test ====", "header2"="--- SW 1 -------------------------------\r\r\r\r\r\r\r\r", "ExpectedValue"=""}, {"Test_Name"="760. SetAsicRegister \"1\" \"4\" \"38\"", "Step_Type"="", "LowLimit"=0.0, "HighLimit"=0.0, "RValue"="", "RStatus"="", "RetVal"="0", "Units"="", "header1"="=== CCD overvoltage protection test ====", "header2"="--- SW 1 -------------------------------\r\r\r\r\r\r\r\r\r", "ExpectedValue"=""}, {"Test_Name"="761. CheckCFAdc \"PD1\" \"3.4\" \"3.85\"", "Step_Type"="NumericLimitTest", "LowLimit"=3.4, "HighLimit"=3.85, "RValue"="3.6389999389648438", "RStatus"="PASS", "RetVal"="0", "Units"="Volts", "header1"="=== CCD overvoltage protection test ====", "header2"="--- SW 1 -------------------------------\r\r\r\r\r\r\r\r\r\r", "ExpectedValue"=""}, {"Test_Name"="762. CheckCFAdc \"PD2\" \"7.3\" \"8.0\"", "Step_Type"="NumericLimitTest", "LowLimit"=7.3, "HighLimit"=8.0, "RValue"="7.623000144958496", "RStatus"="PASS", "RetVal"="0", "Units"="Volts", "header1"="=== CCD overvoltage protection test ====", "header2"="--- SW 1 -------------------------------\r\r\r\r\r\r\r\r\r\r\r", "ExpectedValue"=""}, {"Test_Name"="763. SelectAllMuxA \"1\" \"0\"", "Step_Type"="", "LowLimit"=0.0, "HighLimit"=0.0, "RValue"="", "RStatus"="", "RetVal"="0", "Units"="", "header1"="=== CCD overvoltage protection test ====", "header2"="--- SW 1 -------------------------------\r\r\r\r\r\r\r\r\r\r\r\r", "ExpectedValue"=""}, {"Test_Name"="764. SelectAllMuxB \"1\" \"0\"", "Step_Type"="", "LowLimit"=0.0, "HighLimit"=0.0, "RValue"="", "RStatus"="", "RetVal"="0", "Units"="", "header1"="=== CCD overvoltage protection test ====", "header2"="--- SW 1 -------------------------------\r\r\r\r\r\r\r\r\r\r\r\r\r", "ExpectedValue"=""}, {"Test_Name"="765. SetFpgaRegister \"89E\" \"00\"", "Step_Type"="", "LowLimit"=0.0, "HighLimit"=0.0, "RValue"="", "RStatus"="", "RetVal"="0", "Units"="", "header1"="=== CCD overvoltage protection test ====", "header2"="--- SW 1 -------------------------------\r\r\r\r\r\r\r\r\r\r\r\r\r\r", "ExpectedValue"=""}, {"Test_Name"="766. SetFpgaRegister \"959\" \"00\"", "Step_Type"="", "LowLimit"=0.0, "HighLimit"=0.0, "RValue"="", "RStatus"="", "RetVal"="0", "Units"="", "header1"="=== CCD overvoltage protection test ====", "header2"="--- SW 1 -------------------------------\r\r\r\r\r\r\r\r\r\r\r\r\r\r\r", "ExpectedValue"=""}, {"Test_Name"="767. SetAsicRegister \"1\" \"4\" \"00\"", "Step_Type"="", "LowLimit"=0.0, "HighLimit"=0.0, "RValue"="", "RStatus"="", "RetVal"="0", "Units"="", "header1"="=== CCD overvoltage protection test ====", "header2"="--- SW 1 -------------------------------\r\r\r\r\r\r\r\r\r\r\r\r\r\r\r\r", "ExpectedValue"=""}, {"Test_Name"="770.  ---ISO---", "Step_Type"="", "LowLimit"=0.0, "HighLimit"=0.0, "RValue"="", "RStatus"="", "RetVal"="", "Units"="", "header1"="=== CCD overvoltage protection test ====", "header2"="---ISO----------------------------------\r", "ExpectedValue"=""}, {"Test_Name"="771. SetFpgaRegister \"89E\" \"60\"", "Step_Type"="", "LowLimit"=0.0, "HighLimit"=0.0, "RValue"="", "RStatus"="", "RetVal"="0", "Units"="", "header1"="=== CCD overvoltage protection test ====", "header2"="---ISO----------------------------------\r\r", "ExpectedValue"=""}, {"Test_Name"="772. SetG15PullupVbat \"0\" \"1\"", "Step_Type"="", "LowLimit"=0.0, "HighLimit"=0.0, "RValue"="", "RStatus"="", "RetVal"="0", "Units"="", "header1"="=== CCD overvoltage protection test ====", "header2"="---ISO----------------------------------\r\r\r", "ExpectedValue"=""}, {"Test_Name"="773. SelectMuxA \"1\" \"7\" \"1\"", "Step_Type"="", "LowLimit"=0.0, "HighLimit"=0.0, "RValue"="", "RStatus"="", "RetVal"="0", "Units"="", "header1"="=== CCD overvoltage protection test ====", "header2"="---ISO----------------------------------\r\r\r\r", "ExpectedValue"=""}, {"Test_Name"="774. SelectMuxB \"1\" \"15 \"1\"", "Step_Type"="", "LowLimit"=0.0, "HighLimit"=0.0, "RValue"="", "RStatus"="", "RetVal"="0", "Units"="", "header1"="=== CCD overvoltage protection test ====", "header2"="---ISO----------------------------------\r\r\r\r\r", "ExpectedValue"=""}, {"Test_Name"="775. SetG15PullUp \"A\" \"2\"", "Step_Type"="", "LowLimit"=0.0, "HighLimit"=0.0, "RValue"="", "RStatus"="", "RetVal"="0", "Units"="", "header1"="=== CCD overvoltage protection test ====", "header2"="---ISO----------------------------------\r\r\r\r\r\r", "ExpectedValue"=""}, {"Test_Name"="776. SetG15PullUp \"B\" \"2\"", "Step_Type"="", "LowLimit"=0.0, "HighLimit"=0.0, "RValue"="", "RStatus"="", "RetVal"="0", "Units"="", "header1"="=== CCD overvoltage protection test ====", "header2"="---ISO----------------------------------\r\r\r\r\r\r\r", "ExpectedValue"=""}, {"Test_Name"="778. CheckFpgaRegister \"984\" \"0\" \"1\"", "Step_Type"="StringValueTest", "LowLimit"=0.0, "HighLimit"=0.0, "RValue"="1", "RStatus"="PASS", "RetVal"="0", "Units"="", "header1"="=== CCD overvoltage protection test ====", "header2"="---ISO----------------------------------\r\r\r\r\r\r\r\r", "ExpectedValue"=""}, {"Test_Name"="779. SetFpgaRegister \"983\" \"30\"", "Step_Type"="", "LowLimit"=0.0, "HighLimit"=0.0, "RValue"="", "RStatus"="", "RetVal"="0", "Units"="", "header1"="=== CCD overvoltage protection test ====", "header2"="---ISO----------------------------------\r\r\r\r\r\r\r\r\r", "ExpectedValue"=""}, {"Test_Name"="780. SetAsicRegister \"1\" \"5\" \"04\"", "Step_Type"="", "LowLimit"=0.0, "HighLimit"=0.0, "RValue"="", "RStatus"="", "RetVal"="0", "Units"="", "header1"="=== CCD overvoltage protection test ====", "header2"="---ISO----------------------------------\r\r\r\r\r\r\r\r\r\r", "ExpectedValue"=""}, {"Test_Name"="781. CheckCFAdc \"PD1\" \"-.15\" \".44\"", "Step_Type"="NumericLimitTest", "LowLimit"=-0.15, "HighLimit"=0.44, "RValue"="0.24899999797344208", "RStatus"="PASS", "RetVal"="0", "Units"="Volts", "header1"="=== CCD overvoltage protection test ====", "header2"="---ISO----------------------------------\r\r\r\r\r\r\r\r\r\r\r", "ExpectedValue"=""}, {"Test_Name"="782. CheckCFAdc \"PD2\" \"14\" \"15\"", "Step_Type"="NumericLimitTest", "LowLimit"=14.0, "HighLimit"=15.0, "RValue"="14.406999588012695", "RStatus"="PASS", "RetVal"="0", "Units"="Volts", "header1"="=== CCD overvoltage protection test ====", "header2"="---ISO----------------------------------\r\r\r\r\r\r\r\r\r\r\r\r", "ExpectedValue"=""}, {"Test_Name"="783. CheckFpgaRegister \"984\" \"0\" \"0\"", "Step_Type"="StringValueTest", "LowLimit"=0.0, "HighLimit"=0.0, "RValue"="0", "RStatus"="PASS", "RetVal"="0", "Units"="", "header1"="=== CCD overvoltage protection test ====", "header2"="---ISO----------------------------------\r\r\r\r\r\r\r\r\r\r\r\r\r", "ExpectedValue"=""}, {"Test_Name"="784. SetAsicRegister \"1\" \"5\" \"05\"", "Step_Type"="", "LowLimit"=0.0, "HighLimit"=0.0, "RValue"="", "RStatus"="", "RetVal"="0", "Units"="", "header1"="=== CCD overvoltage protection test ====", "header2"="---ISO----------------------------------\r\r\r\r\r\r\r\r\r\r\r\r\r\r", "ExpectedValue"=""}, {"Test_Name"="785. CheckFpgaRegister \"984\" \"0\" \"1\"", "Step_Type"="StringValueTest", "LowLimit"=0.0, "HighLimit"=0.0, "RValue"="1", "RStatus"="PASS", "RetVal"="0", "Units"="", "header1"="=== CCD overvoltage protection test ====", "header2"="---ISO----------------------------------\r\r\r\r\r\r\r\r\r\r\r\r\r\r\r", "ExpectedValue"=""}, {"Test_Name"="786. SetFpgaRegister \"983\" \"28\"", "Step_Type"="", "LowLimit"=0.0, "HighLimit"=0.0, "RValue"="", "RStatus"="", "RetVal"="0", "Units"="", "header1"="=== CCD overvoltage protection test ====", "header2"="---ISO----------------------------------\r\r\r\r\r\r\r\r\r\r\r\r\r\r\r\r", "ExpectedValue"=""}, {"Test_Name"="787. CheckCFAdc \"PD2\" \"-.15\" \".4\"", "Step_Type"="NumericLimitTest", "LowLimit"=-0.15, "HighLimit"=0.4, "RValue"="0.24899999797344208", "RStatus"="PASS", "RetVal"="0", "Units"="Volts", "header1"="=== CCD overvoltage protection test ====", "header2"="---ISO----------------------------------\r\r\r\r\r\r\r\r\r\r\r\r\r\r\r\r\r", "ExpectedValue"=""}, {"Test_Name"="788. CheckCFAdc \"PD1\" \"14\" \"15\"", "Step_Type"="NumericLimitTest", "LowLimit"=14.0, "HighLimit"=15.0, "RValue"="14.401000022888184", "RStatus"="PASS", "RetVal"="0", "Units"="Volts", "header1"="=== CCD overvoltage protection test ====", "header2"="---ISO----------------------------------\r\r\r\r\r\r\r\r\r\r\r\r\r\r\r\r\r\r", "ExpectedValue"=""}, {"Test_Name"="789. CheckFpgaRegister \"984\" \"0\" \"0\"", "Step_Type"="StringValueTest", "LowLimit"=0.0, "HighLimit"=0.0, "RValue"="0", "RStatus"="PASS", "RetVal"="0", "Units"="", "header1"="=== CCD overvoltage protection test ====", "header2"="---ISO----------------------------------\r\r\r\r\r\r\r\r\r\r\r\r\r\r\r\r\r\r\r", "ExpectedValue"=""}, {"Test_Name"="790. SetAsicRegister \"1\" \"5\" \"06\"", "Step_Type"="", "LowLimit"=0.0, "HighLimit"=0.0, "RValue"="", "RStatus"="", "RetVal"="0", "Units"="", "header1"="=== CCD overvoltage protection test ====", "header2"="---ISO----------------------------------\r\r\r\r\r\r\r\r\r\r\r\r\r\r\r\r\r\r\r\r", "ExpectedValue"=""}, {"Test_Name"="791. CheckFpgaRegister \"984\" \"0\" \"1\"", "Step_Type"="StringValueTest", "LowLimit"=0.0, "HighLimit"=0.0, "RValue"="1", "RStatus"="PASS", "RetVal"="0", "Units"="", "header1"="=== CCD overvoltage protection test ====", "header2"="---ISO----------------------------------\r\r\r\r\r\r\r\r\r\r\r\r\r\r\r\r\r\r\r\r\r", "ExpectedValue"=""}, {"Test_Name"="792. SetAsicRegister \"1\" \"5\" \"08\"", "Step_Type"="", "LowLimit"=0.0, "HighLimit"=0.0, "RValue"="", "RStatus"="", "RetVal"="0", "Units"="", "header1"="=== CCD overvoltage protection test ====", "header2"="---ISO----------------------------------\r\r\r\r\r\r\r\r\r\r\r\r\r\r\r\r\r\r\r\r\r\r", "ExpectedValue"=""}, {"Test_Name"="793. SetFpgaRegister \"983\" \"30\"", "Step_Type"="", "LowLimit"=0.0, "HighLimit"=0.0, "RValue"="", "RStatus"="", "RetVal"="0", "Units"="", "header1"="=== CCD overvoltage protection test ====", "header2"="---ISO----------------------------------\r\r\r\r\r\r\r\r\r\r\r\r\r\r\r\r\r\r\r\r\r\r\r", "ExpectedValue"=""}, {"Test_Name"="794. CheckCFAdc \"PD1\" \"-.15\" \".44\"", "Step_Type"="NumericLimitTest", "LowLimit"=-0.15, "HighLimit"=0.44, "RValue"="0.24899999797344208", "RStatus"="PASS", "RetVal"="0", "Units"="Volts", "header1"="=== CCD overvoltage protection test ====", "header2"="---ISO----------------------------------\r\r\r\r\r\r\r\r\r\r\r\r\r\r\r\r\r\r\r\r\r\r\r\r", "ExpectedValue"=""}, {"Test_Name"="795. CheckCFAdc \"PD2\" \"-.15\" \".4\"", "Step_Type"="NumericLimitTest", "LowLimit"=-0.15, "HighLimit"=0.4, "RValue"="0.24899999797344208", "RStatus"="PASS", "RetVal"="0", "Units"="Volts", "header1"="=== CCD overvoltage protection test ====", "header2"="---ISO----------------------------------\r\r\r\r\r\r\r\r\r\r\r\r\r\r\r\r\r\r\r\r\r\r\r\r\r", "ExpectedValue"=""}, {"Test_Name"="796. CheckFpgaRegister \"984\" \"0\" \"0\"", "Step_Type"="StringValueTest", "LowLimit"=0.0, "HighLimit"=0.0, "RValue"="0", "RStatus"="PASS", "RetVal"="0", "Units"="", "header1"="=== CCD overvoltage protection test ====", "header2"="---ISO----------------------------------\r\r\r\r\r\r\r\r\r\r\r\r\r\r\r\r\r\r\r\r\r\r\r\r\r\r", "ExpectedValue"=""}, {"Test_Name"="797. SetAsicRegister \"1\" \"5\" \"07\"", "Step_Type"="", "LowLimit"=0.0, "HighLimit"=0.0, "RValue"="", "RStatus"="", "RetVal"="0", "Units"="", "header1"="=== CCD overvoltage protection test ====", "header2"="---ISO----------------------------------\r\r\r\r\r\r\r\r\r\r\r\r\r\r\r\r\r\r\r\r\r\r\r\r\r\r\r", "ExpectedValue"=""}, {"Test_Name"="798. CheckFpgaRegister \"984\" \"0\" \"1\"", "Step_Type"="StringValueTest", "LowLimit"=0.0, "HighLimit"=0.0, "RValue"="1", "RStatus"="PASS", "RetVal"="0", "Units"="", "header1"="=== CCD overvoltage protection test ====", "header2"="---ISO----------------------------------\r\r\r\r\r\r\r\r\r\r\r\r\r\r\r\r\r\r\r\r\r\r\r\r\r\r\r\r", "ExpectedValue"=""}, {"Test_Name"="799. SetAsicRegister \"1\" \"5\" \"00\"", "Step_Type"="", "LowLimit"=0.0, "HighLimit"=0.0, "RValue"="", "RStatus"="", "RetVal"="0", "Units"="", "header1"="=== CCD overvoltage protection test ====", "header2"="---ISO----------------------------------\r\r\r\r\r\r\r\r\r\r\r\r\r\r\r\r\r\r\r\r\r\r\r\r\r\r\r\r\r", "ExpectedValue"=""}, {"Test_Name"="800. CheckCFAdc \"PD1\" \"14\" \"15\"", "Step_Type"="NumericLimitTest", "LowLimit"=14.0, "HighLimit"=15.0, "RValue"="14.41100025177002", "RStatus"="PASS", "RetVal"="0", "Units"="Volts", "header1"="=== CCD overvoltage protection test ====", "header2"="---ISO----------------------------------\r\r\r\r\r\r\r\r\r\r\r\r\r\r\r\r\r\r\r\r\r\r\r\r\r\r\r\r\r\r", "ExpectedValue"=""}, {"Test_Name"="801. CheckCFAdc \"PD2\" \"14\" \"15\"", "Step_Type"="NumericLimitTest", "LowLimit"=14.0, "HighLimit"=15.0, "RValue"="14.425000190734863", "RStatus"="PASS", "RetVal"="0", "Units"="Volts", "header1"="=== CCD overvoltage protection test ====", "header2"="---ISO----------------------------------\r\r\r\r\r\r\r\r\r\r\r\r\r\r\r\r\r\r\r\r\r\r\r\r\r\r\r\r\r\r\r", "ExpectedValue"=""}, {"Test_Name"="802. CheckFpgaRegister \"984\" \"0\" \"1\"", "Step_Type"="StringValueTest", "LowLimit"=0.0, "HighLimit"=0.0, "RValue"="1", "RStatus"="PASS", "RetVal"="0", "Units"="", "header1"="=== CCD overvoltage protection test ====", "header2"="---ISO----------------------------------\r\r\r\r\r\r\r\r\r\r\r\r\r\r\r\r\r\r\r\r\r\r\r\r\r\r\r\r\r\r\r\r", "ExpectedValue"=""}, {"Test_Name"="805. SetAsicRegister \"1\" \"6\" \"11\"", "Step_Type"="", "LowLimit"=0.0, "HighLimit"=0.0, "RValue"="", "RStatus"="", "RetVal"="0", "Units"="", "header1"="=== CCD overvoltage protection test ====", "header2"="---ISO----------------------------------\r\r\r\r\r\r\r\r\r\r\r\r\r\r\r\r\r\r\r\r\r\r\r\r\r\r\r\r\r\r\r\r\r", "ExpectedValue"=""}, {"Test_Name"="806. SetG15PullupVbat \"0\" \"0\"", "Step_Type"="", "LowLimit"=0.0, "HighLimit"=0.0, "RValue"="", "RStatus"="", "RetVal"="0", "Units"="", "header1"="=== CCD overvoltage protection test ====", "header2"="---ISO----------------------------------\r\r\r\r\r\r\r\r\r\r\r\r\r\r\r\r\r\r\r\r\r\r\r\r\r\r\r\r\r\r\r\r\r\r", "ExpectedValue"=""}, {"Test_Name"="807. SetG15PullUp \"A\" \"9\"", "Step_Type"="", "LowLimit"=0.0, "HighLimit"=0.0, "RValue"="", "RStatus"="", "RetVal"="0", "Units"="", "header1"="=== CCD overvoltage protection test ====", "header2"="---ISO----------------------------------\r\r\r\r\r\r\r\r\r\r\r\r\r\r\r\r\r\r\r\r\r\r\r\r\r\r\r\r\r\r\r\r\r\r\r", "ExpectedValue"=""}, {"Test_Name"="808. SetG15PullDown \"A\" \"3\"", "Step_Type"="", "LowLimit"=0.0, "HighLimit"=0.0, "RValue"="", "RStatus"="", "RetVal"="0", "Units"="", "header1"="=== CCD overvoltage protection test ====", "header2"="---ISO----------------------------------\r\r\r\r\r\r\r\r\r\r\r\r\r\r\r\r\r\r\r\r\r\r\r\r\r\r\r\r\r\r\r\r\r\r\r\r", "ExpectedValue"=""}, {"Test_Name"="809. CheckCFAdc \"PD1\" \"1.2\" \"1.5\"", "Step_Type"="NumericLimitTest", "LowLimit"=1.2, "HighLimit"=1.5, "RValue"="1.3849999904632568", "RStatus"="PASS", "RetVal"="0", "Units"="Volts", "header1"="=== CCD overvoltage protection test ====", "header2"="---ISO----------------------------------\r\r\r\r\r\r\r\r\r\r\r\r\r\r\r\r\r\r\r\r\r\r\r\r\r\r\r\r\r\r\r\r\r\r\r\r\r", "ExpectedValue"=""}, {"Test_Name"="810. CheckFpgaRegister \"984\" \"0\" \"0\"", "Step_Type"="StringValueTest", "LowLimit"=0.0, "HighLimit"=0.0, "RValue"="0", "RStatus"="PASS", "RetVal"="0", "Units"="", "header1"="=== CCD overvoltage protection test ====", "header2"="---ISO----------------------------------\r\r\r\r\r\r\r\r\r\r\r\r\r\r\r\r\r\r\r\r\r\r\r\r\r\r\r\r\r\r\r\r\r\r\r\r\r\r", "ExpectedValue"=""}, {"Test_Name"="811. SetG15PullDown \"A\" \"4\"", "Step_Type"="", "LowLimit"=0.0, "HighLimit"=0.0, "RValue"="", "RStatus"="", "RetVal"="0", "Units"="", "header1"="=== CCD overvoltage protection test ====", "header2"="---ISO----------------------------------\r\r\r\r\r\r\r\r\r\r\r\r\r\r\r\r\r\r\r\r\r\r\r\r\r\r\r\r\r\r\r\r\r\r\r\r\r\r\r", "ExpectedValue"=""}, {"Test_Name"="812. CheckCFAdc \"PD1\" \"2.2\" \"2.65\"", "Step_Type"="NumericLimitTest", "LowLimit"=2.2, "HighLimit"=2.65, "RValue"="2.4200000762939453", "RStatus"="PASS", "RetVal"="0", "Units"="Volts", "header1"="=== CCD overvoltage protection test ====", "header2"="---ISO----------------------------------\r\r\r\r\r\r\r\r\r\r\r\r\r\r\r\r\r\r\r\r\r\r\r\r\r\r\r\r\r\r\r\r\r\r\r\r\r\r\r\r", "ExpectedValue"=""}, {"Test_Name"="813. CheckFpgaRegister \"984\" \"0\" \"1\"", "Step_Type"="StringValueTest", "LowLimit"=0.0, "HighLimit"=0.0, "RValue"="1", "RStatus"="PASS", "RetVal"="0", "Units"="", "header1"="=== CCD overvoltage protection test ====", "header2"="---ISO----------------------------------\r\r\r\r\r\r\r\r\r\r\r\r\r\r\r\r\r\r\r\r\r\r\r\r\r\r\r\r\r\r\r\r\r\r\r\r\r\r\r\r\r", "ExpectedValue"=""}, {"Test_Name"="816. SetFpgaRegister \"89E\" \"00\"", "Step_Type"="", "LowLimit"=0.0, "HighLimit"=0.0, "RValue"="", "RStatus"="", "RetVal"="0", "Units"="", "header1"="=== CCD overvoltage protection test ====", "header2"="---ISO----------------------------------\r\r\r\r\r\r\r\r\r\r\r\r\r\r\r\r\r\r\r\r\r\r\r\r\r\r\r\r\r\r\r\r\r\r\r\r\r\r\r\r\r\r", "ExpectedValue"=""}, {"Test_Name"="817. SelectMuxA \"1\" \"7\" \"0\"", "Step_Type"="", "LowLimit"=0.0, "HighLimit"=0.0, "RValue"="", "RStatus"="", "RetVal"="0", "Units"="", "header1"="=== CCD overvoltage protection test ====", "header2"="---ISO----------------------------------\r\r\r\r\r\r\r\r\r\r\r\r\r\r\r\r\r\r\r\r\r\r\r\r\r\r\r\r\r\r\r\r\r\r\r\r\r\r\r\r\r\r\r", "ExpectedValue"=""}, {"Test_Name"="818. SelectMuxB \"1\" \"15 \"0\"", "Step_Type"="", "LowLimit"=0.0, "HighLimit"=0.0, "RValue"="", "RStatus"="", "RetVal"="0", "Units"="", "header1"="=== CCD overvoltage protection test ====", "header2"="---ISO----------------------------------\r\r\r\r\r\r\r\r\r\r\r\r\r\r\r\r\r\r\r\r\r\r\r\r\r\r\r\r\r\r\r\r\r\r\r\r\r\r\r\r\r\r\r\r", "ExpectedValue"=""}, {"Test_Name"="819. SetG15PullUp \"A\" \"0\"", "Step_Type"="", "LowLimit"=0.0, "HighLimit"=0.0, "RValue"="", "RStatus"="", "RetVal"="0", "Units"="", "header1"="=== CCD overvoltage protection test ====", "header2"="---ISO----------------------------------\r\r\r\r\r\r\r\r\r\r\r\r\r\r\r\r\r\r\r\r\r\r\r\r\r\r\r\r\r\r\r\r\r\r\r\r\r\r\r\r\r\r\r\r\r", "ExpectedValue"=""}, {"Test_Name"="820. SetG15PullDown \"A\" \"0\"", "Step_Type"="", "LowLimit"=0.0, "HighLimit"=0.0, "RValue"="", "RStatus"="", "RetVal"="0", "Units"="", "header1"="=== CCD overvoltage protection test ====", "header2"="---ISO----------------------------------\r\r\r\r\r\r\r\r\r\r\r\r\r\r\r\r\r\r\r\r\r\r\r\r\r\r\r\r\r\r\r\r\r\r\r\r\r\r\r\r\r\r\r\r\r\r", "ExpectedValue"=""}, {"Test_Name"="821. SetG15PullUp \"B\" \"0\"", "Step_Type"="", "LowLimit"=0.0, "HighLimit"=0.0, "RValue"="", "RStatus"="", "RetVal"="0", "Units"="", "header1"="=== CCD overvoltage protection test ====", "header2"="---ISO----------------------------------\r\r\r\r\r\r\r\r\r\r\r\r\r\r\r\r\r\r\r\r\r\r\r\r\r\r\r\r\r\r\r\r\r\r\r\r\r\r\r\r\r\r\r\r\r\r\r", "ExpectedValue"=""}, {"Test_Name"="822. SetG15PullupVbat \"0\" \"0\"", "Step_Type"="", "LowLimit"=0.0, "HighLimit"=0.0, "RValue"="", "RStatus"="", "RetVal"="0", "Units"="", "header1"="=== CCD overvoltage protection test ====", "header2"="---ISO----------------------------------\r\r\r\r\r\r\r\r\r\r\r\r\r\r\r\r\r\r\r\r\r\r\r\r\r\r\r\r\r\r\r\r\r\r\r\r\r\r\r\r\r\r\r\r\r\r\r\r", "ExpectedValue"=""}, {"Test_Name"="823. SetFpgaRegister \"983\" \"00\"", "Step_Type"="", "LowLimit"=0.0, "HighLimit"=0.0, "RValue"="", "RStatus"="", "RetVal"="0", "Units"="", "header1"="=== CCD overvoltage protection test ====", "header2"="---ISO----------------------------------\r\r\r\r\r\r\r\r\r\r\r\r\r\r\r\r\r\r\r\r\r\r\r\r\r\r\r\r\r\r\r\r\r\r\r\r\r\r\r\r\r\r\r\r\r\r\r\r\r", "ExpectedValue"=""}, {"Test_Name"="826. --- Start Pin Driver test for ASIC 2---", "Step_Type"="", "LowLimit"=0.0, "HighLimit"=0.0, "RValue"="", "RStatus"="", "RetVal"="", "Units"="", "header1"="=== CCD overvoltage protection test ====", "header2"="--- Start Pin Driver test for ASIC 2----\r", "ExpectedValue"=""}, {"Test_Name"="830. SetReference \"128\"", "Step_Type"="", "LowLimit"=0.0, "HighLimit"=0.0, "RValue"="", "RStatus"="", "RetVal"="0", "Units"="", "header1"="=== CCD overvoltage protection test ====", "header2"="--- Start Pin Driver test for ASIC 2----\r\r", "ExpectedValue"=""}, {"Test_Name"="831. SetBaud \"1\"", "Step_Type"="", "LowLimit"=0.0, "HighLimit"=0.0, "RValue"="", "RStatus"="", "RetVal"="0", "Units"="", "header1"="=== CCD overvoltage protection test ====", "header2"="--- Start Pin Driver test for ASIC 2----\r\r\r", "ExpectedValue"=""}, {"Test_Name"="832. SelectAllMuxA \"2\" \"0\"", "Step_Type"="", "LowLimit"=0.0, "HighLimit"=0.0, "RValue"="", "RStatus"="", "RetVal"="0", "Units"="", "header1"="=== CCD overvoltage protection test ====", "header2"="--- Start Pin Driver test for ASIC 2----\r\r\r\r", "ExpectedValue"=""}, {"Test_Name"="833. SelectAllMuxB \"2\" \"0\"", "Step_Type"="", "LowLimit"=0.0, "HighLimit"=0.0, "RValue"="", "RStatus"="", "RetVal"="0", "Units"="", "header1"="=== CCD overvoltage protection test ====", "header2"="--- Start Pin Driver test for ASIC 2----\r\r\r\r\r", "ExpectedValue"=""}, {"Test_Name"="836. SetG15PullUp \"C\" \"1\"", "Step_Type"="", "LowLimit"=0.0, "HighLimit"=0.0, "RValue"="", "RStatus"="", "RetVal"="0", "Units"="", "header1"="=== CCD overvoltage protection test ====", "header2"="--- Start Pin Driver test for ASIC 2----\r\r\r\r\r\r", "ExpectedValue"=""}, {"Test_Name"="837. SetG15PullUp \"D\" \"1\"", "Step_Type"="", "LowLimit"=0.0, "HighLimit"=0.0, "RValue"="", "RStatus"="", "RetVal"="0", "Units"="", "header1"="=== CCD overvoltage protection test ====", "header2"="--- Start Pin Driver test for ASIC 2----\r\r\r\r\r\r\r", "ExpectedValue"=""}, {"Test_Name"="838. CheckCFAdc \"PD3\" \"4.5\" \"5.0\"", "Step_Type"="NumericLimitTest", "LowLimit"=4.5, "HighLimit"=5.0, "RValue"="4.790999889373779", "RStatus"="PASS", "RetVal"="0", "Units"="Volts", "header1"="=== CCD overvoltage protection test ====", "header2"="--- Start Pin Driver test for ASIC 2----\r\r\r\r\r\r\r\r", "ExpectedValue"=""}, {"Test_Name"="839. CheckCFAdc \"PD4\" \"4.5\" \"5.0\"", "Step_Type"="NumericLimitTest", "LowLimit"=4.5, "HighLimit"=5.0, "RValue"="4.76800012588501", "RStatus"="PASS", "RetVal"="0", "Units"="Volts", "header1"="=== CCD overvoltage protection test ====", "header2"="--- Start Pin Driver test for ASIC 2----\r\r\r\r\r\r\r\r\r", "ExpectedValue"=""}, {"Test_Name"="842. SetG15PullDown \"C\" \"3\"", "Step_Type"="", "LowLimit"=0.0, "HighLimit"=0.0, "RValue"="", "RStatus"="", "RetVal"="0", "Units"="", "header1"="=== CCD overvoltage protection test ====", "header2"="--- Start Pin Driver test for ASIC 2----\r\r\r\r\r\r\r\r\r\r", "ExpectedValue"=""}, {"Test_Name"="843. SetG15PullDown \"D\" \"3\"", "Step_Type"="", "LowLimit"=0.0, "HighLimit"=0.0, "RValue"="", "RStatus"="", "RetVal"="0", "Units"="", "header1"="=== CCD overvoltage protection test ====", "header2"="--- Start Pin Driver test for ASIC 2----\r\r\r\r\r\r\r\r\r\r\r", "ExpectedValue"=""}, {"Test_Name"="844. CheckCFAdc \"PD3\" \"4.1\" \"4.55\"", "Step_Type"="NumericLimitTest", "LowLimit"=4.1, "HighLimit"=4.55, "RValue"="4.373000144958496", "RStatus"="PASS", "RetVal"="0", "Units"="Volts", "header1"="=== CCD overvoltage protection test ====", "header2"="--- Start Pin Driver test for ASIC 2----\r\r\r\r\r\r\r\r\r\r\r\r", "ExpectedValue"=""}, {"Test_Name"="845. CheckCFAdc \"PD4\" \"4.1\" \"4.55\"", "Step_Type"="NumericLimitTest", "LowLimit"=4.1, "HighLimit"=4.55, "RValue"="4.369999885559082", "RStatus"="PASS", "RetVal"="0", "Units"="Volts", "header1"="=== CCD overvoltage protection test ====", "header2"="--- Start Pin Driver test for ASIC 2----\r\r\r\r\r\r\r\r\r\r\r\r\r", "ExpectedValue"=""}, {"Test_Name"="848. SetG15PullUp \"C\" \"7\"", "Step_Type"="", "LowLimit"=0.0, "HighLimit"=0.0, "RValue"="", "RStatus"="", "RetVal"="0", "Units"="", "header1"="=== CCD overvoltage protection test ====", "header2"="--- Start Pin Driver test for ASIC 2----\r\r\r\r\r\r\r\r\r\r\r\r\r\r", "ExpectedValue"=""}, {"Test_Name"="849. SetG15PullUp \"D\" \"7\"", "Step_Type"="", "LowLimit"=0.0, "HighLimit"=0.0, "RValue"="", "RStatus"="", "RetVal"="0", "Units"="", "header1"="=== CCD overvoltage protection test ====", "header2"="--- Start Pin Driver test for ASIC 2----\r\r\r\r\r\r\r\r\r\r\r\r\r\r\r", "ExpectedValue"=""}, {"Test_Name"="850. CheckCFAdc \"PD3\" \"2.2\" \"2.6\"", "Step_Type"="NumericLimitTest", "LowLimit"=2.2, "HighLimit"=2.6, "RValue"="2.440999984741211", "RStatus"="PASS", "RetVal"="0", "Units"="Volts", "header1"="=== CCD overvoltage protection test ====", "header2"="--- Start Pin Driver test for ASIC 2----\r\r\r\r\r\r\r\r\r\r\r\r\r\r\r\r", "ExpectedValue"=""}, {"Test_Name"="851. CheckCFAdc \"PD4\" \"2.2\" \"2.6\"", "Step_Type"="NumericLimitTest", "LowLimit"=2.2, "HighLimit"=2.6, "RValue"="2.444000005722046", "RStatus"="PASS", "RetVal"="0", "Units"="Volts", "header1"="=== CCD overvoltage protection test ====", "header2"="--- Start Pin Driver test for ASIC 2----\r\r\r\r\r\r\r\r\r\r\r\r\r\r\r\r\r", "ExpectedValue"=""}, {"Test_Name"="854. SetG15PullUp \"C\" \"1\"", "Step_Type"="", "LowLimit"=0.0, "HighLimit"=0.0, "RValue"="", "RStatus"="", "RetVal"="0", "Units"="", "header1"="=== CCD overvoltage protection test ====", "header2"="--- Start Pin Driver test for ASIC 2----\r\r\r\r\r\r\r\r\r\r\r\r\r\r\r\r\r\r", "ExpectedValue"=""}, {"Test_Name"="855. SetG15PullUp \"D\" \"1\"", "Step_Type"="", "LowLimit"=0.0, "HighLimit"=0.0, "RValue"="", "RStatus"="", "RetVal"="0", "Units"="", "header1"="=== CCD overvoltage protection test ====", "header2"="--- Start Pin Driver test for ASIC 2----\r\r\r\r\r\r\r\r\r\r\r\r\r\r\r\r\r\r\r", "ExpectedValue"=""}, {"Test_Name"="856. SetG15PullDown \"C\" \"4\"", "Step_Type"="", "LowLimit"=0.0, "HighLimit"=0.0, "RValue"="", "RStatus"="", "RetVal"="0", "Units"="", "header1"="=== CCD overvoltage protection test ====", "header2"="--- Start Pin Driver test for ASIC 2----\r\r\r\r\r\r\r\r\r\r\r\r\r\r\r\r\r\r\r\r", "ExpectedValue"=""}, {"Test_Name"="857. SetG15PullDown \"D\" \"4\"", "Step_Type"="", "LowLimit"=0.0, "HighLimit"=0.0, "RValue"="", "RStatus"="", "RetVal"="0", "Units"="", "header1"="=== CCD overvoltage protection test ====", "header2"="--- Start Pin Driver test for ASIC 2----\r\r\r\r\r\r\r\r\r\r\r\r\r\r\r\r\r\r\r\r\r", "ExpectedValue"=""}, {"Test_Name"="858. CheckCFAdc \"PD3\" \"4.3\" \"4.8\"", "Step_Type"="NumericLimitTest", "LowLimit"=4.3, "HighLimit"=4.8, "RValue"="4.613999843597412", "RStatus"="PASS", "RetVal"="0", "Units"="Volts", "header1"="=== CCD overvoltage protection test ====", "header2"="--- Start Pin Driver test for ASIC 2----\r\r\r\r\r\r\r\r\r\r\r\r\r\r\r\r\r\r\r\r\r\r", "ExpectedValue"=""}, {"Test_Name"="859. CheckCFAdc \"PD4\" \"4.3\" \"4.8\"", "Step_Type"="NumericLimitTest", "LowLimit"=4.3, "HighLimit"=4.8, "RValue"="4.5920000076293945", "RStatus"="PASS", "RetVal"="0", "Units"="Volts", "header1"="=== CCD overvoltage protection test ====", "header2"="--- Start Pin Driver test for ASIC 2----\r\r\r\r\r\r\r\r\r\r\r\r\r\r\r\r\r\r\r\r\r\r\r", "ExpectedValue"=""}, {"Test_Name"="862. SetG15PullUp \"C\" \"2\"", "Step_Type"="", "LowLimit"=0.0, "HighLimit"=0.0, "RValue"="", "RStatus"="", "RetVal"="0", "Units"="", "header1"="=== CCD overvoltage protection test ====", "header2"="--- Start Pin Driver test for ASIC 2----\r\r\r\r\r\r\r\r\r\r\r\r\r\r\r\r\r\r\r\r\r\r\r\r", "ExpectedValue"=""}, {"Test_Name"="863. SetG15PullUp \"D\" \"2\"", "Step_Type"="", "LowLimit"=0.0, "HighLimit"=0.0, "RValue"="", "RStatus"="", "RetVal"="0", "Units"="", "header1"="=== CCD overvoltage protection test ====", "header2"="--- Start Pin Driver test for ASIC 2----\r\r\r\r\r\r\r\r\r\r\r\r\r\r\r\r\r\r\r\r\r\r\r\r\r", "ExpectedValue"=""}, {"Test_Name"="864. SetG15PullDown \"C\" \"3\"", "Step_Type"="", "LowLimit"=0.0, "HighLimit"=0.0, "RValue"="", "RStatus"="", "RetVal"="0", "Units"="", "header1"="=== CCD overvoltage protection test ====", "header2"="--- Start Pin Driver test for ASIC 2----\r\r\r\r\r\r\r\r\r\r\r\r\r\r\r\r\r\r\r\r\r\r\r\r\r\r", "ExpectedValue"=""}, {"Test_Name"="865. SetG15PullDown \"D\" \"3\"", "Step_Type"="", "LowLimit"=0.0, "HighLimit"=0.0, "RValue"="", "RStatus"="", "RetVal"="0", "Units"="", "header1"="=== CCD overvoltage protection test ====", "header2"="--- Start Pin Driver test for ASIC 2----\r\r\r\r\r\r\r\r\r\r\r\r\r\r\r\r\r\r\r\r\r\r\r\r\r\r\r", "ExpectedValue"=""}, {"Test_Name"="866. CheckCFAdc \"PD3\" \"4.0\" \"4.45\"", "Step_Type"="NumericLimitTest", "LowLimit"=4.0, "HighLimit"=4.45, "RValue"="4.243000030517578", "RStatus"="PASS", "RetVal"="0", "Units"="Volts", "header1"="=== CCD overvoltage protection test ====", "header2"="--- Start Pin Driver test for ASIC 2----\r\r\r\r\r\r\r\r\r\r\r\r\r\r\r\r\r\r\r\r\r\r\r\r\r\r\r\r", "ExpectedValue"=""}, {"Test_Name"="867. CheckCFAdc \"PD4\" \"4.0\" \"4.45\"", "Step_Type"="NumericLimitTest", "LowLimit"=4.0, "HighLimit"=4.45, "RValue"="4.2220001220703125", "RStatus"="PASS", "RetVal"="0", "Units"="Volts", "header1"="=== CCD overvoltage protection test ====", "header2"="--- Start Pin Driver test for ASIC 2----\r\r\r\r\r\r\r\r\r\r\r\r\r\r\r\r\r\r\r\r\r\r\r\r\r\r\r\r\r", "ExpectedValue"=""}, {"Test_Name"="870. SetG15PullUp \"C\" \"2\"", "Step_Type"="", "LowLimit"=0.0, "HighLimit"=0.0, "RValue"="", "RStatus"="", "RetVal"="0", "Units"="", "header1"="=== CCD overvoltage protection test ====", "header2"="--- Start Pin Driver test for ASIC 2----\r\r\r\r\r\r\r\r\r\r\r\r\r\r\r\r\r\r\r\r\r\r\r\r\r\r\r\r\r\r", "ExpectedValue"=""}, {"Test_Name"="871. SetG15PullUp \"D\" \"2\"", "Step_Type"="", "LowLimit"=0.0, "HighLimit"=0.0, "RValue"="", "RStatus"="", "RetVal"="0", "Units"="", "header1"="=== CCD overvoltage protection test ====", "header2"="--- Start Pin Driver test for ASIC 2----\r\r\r\r\r\r\r\r\r\r\r\r\r\r\r\r\r\r\r\r\r\r\r\r\r\r\r\r\r\r\r", "ExpectedValue"=""}, {"Test_Name"="872. SetG15PullDown \"C\" \"4\"", "Step_Type"="", "LowLimit"=0.0, "HighLimit"=0.0, "RValue"="", "RStatus"="", "RetVal"="0", "Units"="", "header1"="=== CCD overvoltage protection test ====", "header2"="--- Start Pin Driver test for ASIC 2----\r\r\r\r\r\r\r\r\r\r\r\r\r\r\r\r\r\r\r\r\r\r\r\r\r\r\r\r\r\r\r\r", "ExpectedValue"=""}, {"Test_Name"="873. SetG15PullDown \"D\" \"4\"", "Step_Type"="", "LowLimit"=0.0, "HighLimit"=0.0, "RValue"="", "RStatus"="", "RetVal"="0", "Units"="", "header1"="=== CCD overvoltage protection test ====", "header2"="--- Start Pin Driver test for ASIC 2----\r\r\r\r\r\r\r\r\r\r\r\r\r\r\r\r\r\r\r\r\r\r\r\r\r\r\r\r\r\r\r\r\r", "ExpectedValue"=""}, {"Test_Name"="874. CheckCFAdc \"PD3\" \"4.3\" \"4.75\"", "Step_Type"="NumericLimitTest", "LowLimit"=4.3, "HighLimit"=4.75, "RValue"="4.577000141143799", "RStatus"="PASS", "RetVal"="0", "Units"="Volts", "header1"="=== CCD overvoltage protection test ====", "header2"="--- Start Pin Driver test for ASIC 2----\r\r\r\r\r\r\r\r\r\r\r\r\r\r\r\r\r\r\r\r\r\r\r\r\r\r\r\r\r\r\r\r\r\r", "ExpectedValue"=""}, {"Test_Name"="875. CheckCFAdc \"PD4\" \"4.3\" \"4.75\"", "Step_Type"="NumericLimitTest", "LowLimit"=4.3, "HighLimit"=4.75, "RValue"="4.554999828338623", "RStatus"="PASS", "RetVal"="0", "Units"="Volts", "header1"="=== CCD overvoltage protection test ====", "header2"="--- Start Pin Driver test for ASIC 2----\r\r\r\r\r\r\r\r\r\r\r\r\r\r\r\r\r\r\r\r\r\r\r\r\r\r\r\r\r\r\r\r\r\r\r", "ExpectedValue"=""}, {"Test_Name"="878. SetG15PullUp \"C\" \"3\"", "Step_Type"="", "LowLimit"=0.0, "HighLimit"=0.0, "RValue"="", "RStatus"="", "RetVal"="0", "Units"="", "header1"="=== CCD overvoltage protection test ====", "header2"="--- Start Pin Driver test for ASIC 2----\r\r\r\r\r\r\r\r\r\r\r\r\r\r\r\r\r\r\r\r\r\r\r\r\r\r\r\r\r\r\r\r\r\r\r\r", "ExpectedValue"=""}, {"Test_Name"="879. SetG15PullUp \"D\" \"3\"", "Step_Type"="", "LowLimit"=0.0, "HighLimit"=0.0, "RValue"="", "RStatus"="", "RetVal"="0", "Units"="", "header1"="=== CCD overvoltage protection test ====", "header2"="--- Start Pin Driver test for ASIC 2----\r\r\r\r\r\r\r\r\r\r\r\r\r\r\r\r\r\r\r\r\r\r\r\r\r\r\r\r\r\r\r\r\r\r\r\r\r", "ExpectedValue"=""}, {"Test_Name"="880. SetG15PullDown \"C\" \"4\"", "Step_Type"="", "LowLimit"=0.0, "HighLimit"=0.0, "RValue"="", "RStatus"="", "RetVal"="0", "Units"="", "header1"="=== CCD overvoltage protection test ====", "header2"="--- Start Pin Driver test for ASIC 2----\r\r\r\r\r\r\r\r\r\r\r\r\r\r\r\r\r\r\r\r\r\r\r\r\r\r\r\r\r\r\r\r\r\r\r\r\r\r", "ExpectedValue"=""}, {"Test_Name"="881. SetG15PullDown \"D\" \"4\"", "Step_Type"="", "LowLimit"=0.0, "HighLimit"=0.0, "RValue"="", "RStatus"="", "RetVal"="0", "Units"="", "header1"="=== CCD overvoltage protection test ====", "header2"="--- Start Pin Driver test for ASIC 2----\r\r\r\r\r\r\r\r\r\r\r\r\r\r\r\r\r\r\r\r\r\r\r\r\r\r\r\r\r\r\r\r\r\r\r\r\r\r\r", "ExpectedValue"=""}, {"Test_Name"="882. CheckCFAdc \"PD3\" \"4.1\" \"4.55\"", "Step_Type"="NumericLimitTest", "LowLimit"=4.1, "HighLimit"=4.55, "RValue"="4.335999965667725", "RStatus"="PASS", "RetVal"="0", "Units"="Volts", "header1"="=== CCD overvoltage protection test ====", "header2"="--- Start Pin Driver test for ASIC 2----\r\r\r\r\r\r\r\r\r\r\r\r\r\r\r\r\r\r\r\r\r\r\r\r\r\r\r\r\r\r\r\r\r\r\r\r\r\r\r\r", "ExpectedValue"=""}, {"Test_Name"="883. CheckCFAdc \"PD4\" \"4.1\" \"4.55\"", "Step_Type"="NumericLimitTest", "LowLimit"=4.1, "HighLimit"=4.55, "RValue"="4.323999881744385", "RStatus"="PASS", "RetVal"="0", "Units"="Volts", "header1"="=== CCD overvoltage protection test ====", "header2"="--- Start Pin Driver test for ASIC 2----\r\r\r\r\r\r\r\r\r\r\r\r\r\r\r\r\r\r\r\r\r\r\r\r\r\r\r\r\r\r\r\r\r\r\r\r\r\r\r\r\r", "ExpectedValue"=""}, {"Test_Name"="886. SetG15PullUp \"C\" \"4\"", "Step_Type"="", "LowLimit"=0.0, "HighLimit"=0.0, "RValue"="", "RStatus"="", "RetVal"="0", "Units"="", "header1"="=== CCD overvoltage protection test ====", "header2"="--- Start Pin Driver test for ASIC 2----\r\r\r\r\r\r\r\r\r\r\r\r\r\r\r\r\r\r\r\r\r\r\r\r\r\r\r\r\r\r\r\r\r\r\r\r\r\r\r\r\r\r", "ExpectedValue"=""}, {"Test_Name"="887. SetG15PullUp \"D\" \"4\"", "Step_Type"="", "LowLimit"=0.0, "HighLimit"=0.0, "RValue"="", "RStatus"="", "RetVal"="0", "Units"="", "header1"="=== CCD overvoltage protection test ====", "header2"="--- Start Pin Driver test for ASIC 2----\r\r\r\r\r\r\r\r\r\r\r\r\r\r\r\r\r\r\r\r\r\r\r\r\r\r\r\r\r\r\r\r\r\r\r\r\r\r\r\r\r\r\r", "ExpectedValue"=""}, {"Test_Name"="888. SetG15PullDown \"C\" \"4\"", "Step_Type"="", "LowLimit"=0.0, "HighLimit"=0.0, "RValue"="", "RStatus"="", "RetVal"="0", "Units"="", "header1"="=== CCD overvoltage protection test ====", "header2"="--- Start Pin Driver test for ASIC 2----\r\r\r\r\r\r\r\r\r\r\r\r\r\r\r\r\r\r\r\r\r\r\r\r\r\r\r\r\r\r\r\r\r\r\r\r\r\r\r\r\r\r\r\r", "ExpectedValue"=""}, {"Test_Name"="889. SetG15PullDown \"D\" \"4\"", "Step_Type"="", "LowLimit"=0.0, "HighLimit"=0.0, "RValue"="", "RStatus"="", "RetVal"="0", "Units"="", "header1"="=== CCD overvoltage protection test ====", "header2"="--- Start Pin Driver test for ASIC 2----\r\r\r\r\r\r\r\r\r\r\r\r\r\r\r\r\r\r\r\r\r\r\r\r\r\r\r\r\r\r\r\r\r\r\r\r\r\r\r\r\r\r\r\r\r", "ExpectedValue"=""}, {"Test_Name"="890. CheckCFAdc \"PD3\" \"3.7\" \"4.15\"", "Step_Type"="NumericLimitTest", "LowLimit"=3.7, "HighLimit"=4.15, "RValue"="3.9739999771118164", "RStatus"="PASS", "RetVal"="0", "Units"="Volts", "header1"="=== CCD overvoltage protection test ====", "header2"="--- Start Pin Driver test for ASIC 2----\r\r\r\r\r\r\r\r\r\r\r\r\r\r\r\r\r\r\r\r\r\r\r\r\r\r\r\r\r\r\r\r\r\r\r\r\r\r\r\r\r\r\r\r\r\r", "ExpectedValue"=""}, {"Test_Name"="891. CheckCFAdc \"PD4\" \"3.7\" \"4.15\"", "Step_Type"="NumericLimitTest", "LowLimit"=3.7, "HighLimit"=4.15, "RValue"="3.953000068664551", "RStatus"="PASS", "RetVal"="0", "Units"="Volts", "header1"="=== CCD overvoltage protection test ====", "header2"="--- Start Pin Driver test for ASIC 2----\r\r\r\r\r\r\r\r\r\r\r\r\r\r\r\r\r\r\r\r\r\r\r\r\r\r\r\r\r\r\r\r\r\r\r\r\r\r\r\r\r\r\r\r\r\r\r", "ExpectedValue"=""}, {"Test_Name"="894. SetG15PullUp \"C\" \"5\"", "Step_Type"="", "LowLimit"=0.0, "HighLimit"=0.0, "RValue"="", "RStatus"="", "RetVal"="0", "Units"="", "header1"="=== CCD overvoltage protection test ====", "header2"="--- Start Pin Driver test for ASIC 2----\r\r\r\r\r\r\r\r\r\r\r\r\r\r\r\r\r\r\r\r\r\r\r\r\r\r\r\r\r\r\r\r\r\r\r\r\r\r\r\r\r\r\r\r\r\r\r\r", "ExpectedValue"=""}, {"Test_Name"="895. SetG15PullUp \"D\" \"5\"", "Step_Type"="", "LowLimit"=0.0, "HighLimit"=0.0, "RValue"="", "RStatus"="", "RetVal"="0", "Units"="", "header1"="=== CCD overvoltage protection test ====", "header2"="--- Start Pin Driver test for ASIC 2----\r\r\r\r\r\r\r\r\r\r\r\r\r\r\r\r\r\r\r\r\r\r\r\r\r\r\r\r\r\r\r\r\r\r\r\r\r\r\r\r\r\r\r\r\r\r\r\r\r", "ExpectedValue"=""}, {"Test_Name"="896. SetG15PullDown \"C\" \"4\"", "Step_Type"="", "LowLimit"=0.0, "HighLimit"=0.0, "RValue"="", "RStatus"="", "RetVal"="0", "Units"="", "header1"="=== CCD overvoltage protection test ====", "header2"="--- Start Pin Driver test for ASIC 2----\r\r\r\r\r\r\r\r\r\r\r\r\r\r\r\r\r\r\r\r\r\r\r\r\r\r\r\r\r\r\r\r\r\r\r\r\r\r\r\r\r\r\r\r\r\r\r\r\r\r", "ExpectedValue"=""}, {"Test_Name"="897. SetG15PullDown \"D\" \"4\"", "Step_Type"="", "LowLimit"=0.0, "HighLimit"=0.0, "RValue"="", "RStatus"="", "RetVal"="0", "Units"="", "header1"="=== CCD overvoltage protection test ====", "header2"="--- Start Pin Driver test for ASIC 2----\r\r\r\r\r\r\r\r\r\r\r\r\r\r\r\r\r\r\r\r\r\r\r\r\r\r\r\r\r\r\r\r\r\r\r\r\r\r\r\r\r\r\r\r\r\r\r\r\r\r\r", "ExpectedValue"=""}, {"Test_Name"="898. CheckCFAdc \"PD3\" \"3.6\" \"4.0\"", "Step_Type"="NumericLimitTest", "LowLimit"=3.6, "HighLimit"=4.0, "RValue"="3.805999994277954", "RStatus"="PASS", "RetVal"="0", "Units"="Volts", "header1"="=== CCD overvoltage protection test ====", "header2"="--- Start Pin Driver test for ASIC 2----\r\r\r\r\r\r\r\r\r\r\r\r\r\r\r\r\r\r\r\r\r\r\r\r\r\r\r\r\r\r\r\r\r\r\r\r\r\r\r\r\r\r\r\r\r\r\r\r\r\r\r\r", "ExpectedValue"=""}, {"Test_Name"="899. CheckCFAdc \"PD4\" \"3.6\" \"4.0\"", "Step_Type"="NumericLimitTest", "LowLimit"=3.6, "HighLimit"=4.0, "RValue"="3.7869999408721924", "RStatus"="PASS", "RetVal"="0", "Units"="Volts", "header1"="=== CCD overvoltage protection test ====", "header2"="--- Start Pin Driver test for ASIC 2----\r\r\r\r\r\r\r\r\r\r\r\r\r\r\r\r\r\r\r\r\r\r\r\r\r\r\r\r\r\r\r\r\r\r\r\r\r\r\r\r\r\r\r\r\r\r\r\r\r\r\r\r\r", "ExpectedValue"=""}, {"Test_Name"="902. SetG15PullUp \"C\" \"6\"", "Step_Type"="", "LowLimit"=0.0, "HighLimit"=0.0, "RValue"="", "RStatus"="", "RetVal"="0", "Units"="", "header1"="=== CCD overvoltage protection test ====", "header2"="--- Start Pin Driver test for ASIC 2----\r\r\r\r\r\r\r\r\r\r\r\r\r\r\r\r\r\r\r\r\r\r\r\r\r\r\r\r\r\r\r\r\r\r\r\r\r\r\r\r\r\r\r\r\r\r\r\r\r\r\r\r\r\r", "ExpectedValue"=""}, {"Test_Name"="903. SetG15PullUp \"D\" \"6\"", "Step_Type"="", "LowLimit"=0.0, "HighLimit"=0.0, "RValue"="", "RStatus"="", "RetVal"="0", "Units"="", "header1"="=== CCD overvoltage protection test ====", "header2"="--- Start Pin Driver test for ASIC 2----\r\r\r\r\r\r\r\r\r\r\r\r\r\r\r\r\r\r\r\r\r\r\r\r\r\r\r\r\r\r\r\r\r\r\r\r\r\r\r\r\r\r\r\r\r\r\r\r\r\r\r\r\r\r\r", "ExpectedValue"=""}, {"Test_Name"="904. SetG15PullDown \"C\" \"4\"", "Step_Type"="", "LowLimit"=0.0, "HighLimit"=0.0, "RValue"="", "RStatus"="", "RetVal"="0", "Units"="", "header1"="=== CCD overvoltage protection test ====", "header2"="--- Start Pin Driver test for ASIC 2----\r\r\r\r\r\r\r\r\r\r\r\r\r\r\r\r\r\r\r\r\r\r\r\r\r\r\r\r\r\r\r\r\r\r\r\r\r\r\r\r\r\r\r\r\r\r\r\r\r\r\r\r\r\r\r\r", "ExpectedValue"=""}, {"Test_Name"="905. SetG15PullDown \"D\" \"4\"", "Step_Type"="", "LowLimit"=0.0, "HighLimit"=0.0, "RValue"="", "RStatus"="", "RetVal"="0", "Units"="", "header1"="=== CCD overvoltage protection test ====", "header2"="--- Start Pin Driver test for ASIC 2----\r\r\r\r\r\r\r\r\r\r\r\r\r\r\r\r\r\r\r\r\r\r\r\r\r\r\r\r\r\r\r\r\r\r\r\r\r\r\r\r\r\r\r\r\r\r\r\r\r\r\r\r\r\r\r\r\r", "ExpectedValue"=""}, {"Test_Name"="906. CheckCFAdc \"PD3\" \"3.45\" \"3.85\"", "Step_Type"="NumericLimitTest", "LowLimit"=3.45, "HighLimit"=3.85, "RValue"="3.6760001182556152", "RStatus"="PASS", "RetVal"="0", "Units"="Volts", "header1"="=== CCD overvoltage protection test ====", "header2"="--- Start Pin Driver test for ASIC 2----\r\r\r\r\r\r\r\r\r\r\r\r\r\r\r\r\r\r\r\r\r\r\r\r\r\r\r\r\r\r\r\r\r\r\r\r\r\r\r\r\r\r\r\r\r\r\r\r\r\r\r\r\r\r\r\r\r\r", "ExpectedValue"=""}, {"Test_Name"="907. CheckCFAdc \"PD4\" \"3.45\" \"3.85\"", "Step_Type"="NumericLimitTest", "LowLimit"=3.45, "HighLimit"=3.85, "RValue"="3.6659998893737793", "RStatus"="PASS", "RetVal"="0", "Units"="Volts", "header1"="=== CCD overvoltage protection test ====", "header2"="--- Start Pin Driver test for ASIC 2----\r\r\r\r\r\r\r\r\r\r\r\r\r\r\r\r\r\r\r\r\r\r\r\r\r\r\r\r\r\r\r\r\r\r\r\r\r\r\r\r\r\r\r\r\r\r\r\r\r\r\r\r\r\r\r\r\r\r\r", "ExpectedValue"=""}, {"Test_Name"="910. SetG15PullUp \"C\" \"7\"", "Step_Type"="", "LowLimit"=0.0, "HighLimit"=0.0, "RValue"="", "RStatus"="", "RetVal"="0", "Units"="", "header1"="=== CCD overvoltage protection test ====", "header2"="--- Start Pin Driver test for ASIC 2----\r\r\r\r\r\r\r\r\r\r\r\r\r\r\r\r\r\r\r\r\r\r\r\r\r\r\r\r\r\r\r\r\r\r\r\r\r\r\r\r\r\r\r\r\r\r\r\r\r\r\r\r\r\r\r\r\r\r\r\r", "ExpectedValue"=""}, {"Test_Name"="911. SetG15PullUp \"D\" \"7\"", "Step_Type"="", "LowLimit"=0.0, "HighLimit"=0.0, "RValue"="", "RStatus"="", "RetVal"="0", "Units"="", "header1"="=== CCD overvoltage protection test ====", "header2"="--- Start Pin Driver test for ASIC 2----\r\r\r\r\r\r\r\r\r\r\r\r\r\r\r\r\r\r\r\r\r\r\r\r\r\r\r\r\r\r\r\r\r\r\r\r\r\r\r\r\r\r\r\r\r\r\r\r\r\r\r\r\r\r\r\r\r\r\r\r\r", "ExpectedValue"=""}, {"Test_Name"="912. SetG15PullDown \"C\" \"4\"", "Step_Type"="", "LowLimit"=0.0, "HighLimit"=0.0, "RValue"="", "RStatus"="", "RetVal"="0", "Units"="", "header1"="=== CCD overvoltage protection test ====", "header2"="--- Start Pin Driver test for ASIC 2----\r\r\r\r\r\r\r\r\r\r\r\r\r\r\r\r\r\r\r\r\r\r\r\r\r\r\r\r\r\r\r\r\r\r\r\r\r\r\r\r\r\r\r\r\r\r\r\r\r\r\r\r\r\r\r\r\r\r\r\r\r\r", "ExpectedValue"=""}, {"Test_Name"="913. SetG15PullDown \"D\" \"4\"", "Step_Type"="", "LowLimit"=0.0, "HighLimit"=0.0, "RValue"="", "RStatus"="", "RetVal"="0", "Units"="", "header1"="=== CCD overvoltage protection test ====", "header2"="--- Start Pin Driver test for ASIC 2----\r\r\r\r\r\r\r\r\r\r\r\r\r\r\r\r\r\r\r\r\r\r\r\r\r\r\r\r\r\r\r\r\r\r\r\r\r\r\r\r\r\r\r\r\r\r\r\r\r\r\r\r\r\r\r\r\r\r\r\r\r\r\r", "ExpectedValue"=""}, {"Test_Name"="914. CheckCFAdc \"PD3\" \"3.3\" \"3.7\"", "Step_Type"="NumericLimitTest", "LowLimit"=3.3, "HighLimit"=3.7, "RValue"="3.490999937057495", "RStatus"="PASS", "RetVal"="0", "Units"="Volts", "header1"="=== CCD overvoltage protection test ====", "header2"="--- Start Pin Driver test for ASIC 2----\r\r\r\r\r\r\r\r\r\r\r\r\r\r\r\r\r\r\r\r\r\r\r\r\r\r\r\r\r\r\r\r\r\r\r\r\r\r\r\r\r\r\r\r\r\r\r\r\r\r\r\r\r\r\r\r\r\r\r\r\r\r\r\r", "ExpectedValue"=""}, {"Test_Name"="915. CheckCFAdc \"PD4\" \"3.3\" \"3.7\"", "Step_Type"="NumericLimitTest", "LowLimit"=3.3, "HighLimit"=3.7, "RValue"="3.4719998836517334", "RStatus"="PASS", "RetVal"="0", "Units"="Volts", "header1"="=== CCD overvoltage protection test ====", "header2"="--- Start Pin Driver test for ASIC 2----\r\r\r\r\r\r\r\r\r\r\r\r\r\r\r\r\r\r\r\r\r\r\r\r\r\r\r\r\r\r\r\r\r\r\r\r\r\r\r\r\r\r\r\r\r\r\r\r\r\r\r\r\r\r\r\r\r\r\r\r\r\r\r\r\r", "ExpectedValue"=""}, {"Test_Name"="918. SetG15PullUp \"C\" \"8\"", "Step_Type"="", "LowLimit"=0.0, "HighLimit"=0.0, "RValue"="", "RStatus"="", "RetVal"="0", "Units"="", "header1"="=== CCD overvoltage protection test ====", "header2"="--- Start Pin Driver test for ASIC 2----\r\r\r\r\r\r\r\r\r\r\r\r\r\r\r\r\r\r\r\r\r\r\r\r\r\r\r\r\r\r\r\r\r\r\r\r\r\r\r\r\r\r\r\r\r\r\r\r\r\r\r\r\r\r\r\r\r\r\r\r\r\r\r\r\r\r", "ExpectedValue"=""}, {"Test_Name"="919. SetG15PullUp \"D\" \"8\"", "Step_Type"="", "LowLimit"=0.0, "HighLimit"=0.0, "RValue"="", "RStatus"="", "RetVal"="0", "Units"="", "header1"="=== CCD overvoltage protection test ====", "header2"="--- Start Pin Driver test for ASIC 2----\r\r\r\r\r\r\r\r\r\r\r\r\r\r\r\r\r\r\r\r\r\r\r\r\r\r\r\r\r\r\r\r\r\r\r\r\r\r\r\r\r\r\r\r\r\r\r\r\r\r\r\r\r\r\r\r\r\r\r\r\r\r\r\r\r\r\r", "ExpectedValue"=""}, {"Test_Name"="920. SetG15PullDown \"C\" \"4\"", "Step_Type"="", "LowLimit"=0.0, "HighLimit"=0.0, "RValue"="", "RStatus"="", "RetVal"="0", "Units"="", "header1"="=== CCD overvoltage protection test ====", "header2"="--- Start Pin Driver test for ASIC 2----\r\r\r\r\r\r\r\r\r\r\r\r\r\r\r\r\r\r\r\r\r\r\r\r\r\r\r\r\r\r\r\r\r\r\r\r\r\r\r\r\r\r\r\r\r\r\r\r\r\r\r\r\r\r\r\r\r\r\r\r\r\r\r\r\r\r\r\r", "ExpectedValue"=""}, {"Test_Name"="921. SetG15PullDown \"D\" \"4\"", "Step_Type"="", "LowLimit"=0.0, "HighLimit"=0.0, "RValue"="", "RStatus"="", "RetVal"="0", "Units"="", "header1"="=== CCD overvoltage protection test ====", "header2"="--- Start Pin Driver test for ASIC 2----\r\r\r\r\r\r\r\r\r\r\r\r\r\r\r\r\r\r\r\r\r\r\r\r\r\r\r\r\r\r\r\r\r\r\r\r\r\r\r\r\r\r\r\r\r\r\r\r\r\r\r\r\r\r\r\r\r\r\r\r\r\r\r\r\r\r\r\r\r", "ExpectedValue"=""}, {"Test_Name"="922. CheckCFAdc \"PD3\" \"3.1\" \"3.5\"", "Step_Type"="NumericLimitTest", "LowLimit"=3.1, "HighLimit"=3.5, "RValue"="3.3239998817443848", "RStatus"="PASS", "RetVal"="0", "Units"="Volts", "header1"="=== CCD overvoltage protection test ====", "header2"="--- Start Pin Driver test for ASIC 2----\r\r\r\r\r\r\r\r\r\r\r\r\r\r\r\r\r\r\r\r\r\r\r\r\r\r\r\r\r\r\r\r\r\r\r\r\r\r\r\r\r\r\r\r\r\r\r\r\r\r\r\r\r\r\r\r\r\r\r\r\r\r\r\r\r\r\r\r\r\r", "ExpectedValue"=""}, {"Test_Name"="923. CheckCFAdc \"PD4\" \"3.1\" \"3.5\"", "Step_Type"="NumericLimitTest", "LowLimit"=3.1, "HighLimit"=3.5, "RValue"="3.305000066757202", "RStatus"="PASS", "RetVal"="0", "Units"="Volts", "header1"="=== CCD overvoltage protection test ====", "header2"="--- Start Pin Driver test for ASIC 2----\r\r\r\r\r\r\r\r\r\r\r\r\r\r\r\r\r\r\r\r\r\r\r\r\r\r\r\r\r\r\r\r\r\r\r\r\r\r\r\r\r\r\r\r\r\r\r\r\r\r\r\r\r\r\r\r\r\r\r\r\r\r\r\r\r\r\r\r\r\r\r", "ExpectedValue"=""}, {"Test_Name"="926. SetG15PullUp \"C\" \"9\"", "Step_Type"="", "LowLimit"=0.0, "HighLimit"=0.0, "RValue"="", "RStatus"="", "RetVal"="0", "Units"="", "header1"="=== CCD overvoltage protection test ====", "header2"="--- Start Pin Driver test for ASIC 2----\r\r\r\r\r\r\r\r\r\r\r\r\r\r\r\r\r\r\r\r\r\r\r\r\r\r\r\r\r\r\r\r\r\r\r\r\r\r\r\r\r\r\r\r\r\r\r\r\r\r\r\r\r\r\r\r\r\r\r\r\r\r\r\r\r\r\r\r\r\r\r\r", "ExpectedValue"=""}, {"Test_Name"="927. SetG15PullUp \"D\" \"9\"", "Step_Type"="", "LowLimit"=0.0, "HighLimit"=0.0, "RValue"="", "RStatus"="", "RetVal"="0", "Units"="", "header1"="=== CCD overvoltage protection test ====", "header2"="--- Start Pin Driver test for ASIC 2----\r\r\r\r\r\r\r\r\r\r\r\r\r\r\r\r\r\r\r\r\r\r\r\r\r\r\r\r\r\r\r\r\r\r\r\r\r\r\r\r\r\r\r\r\r\r\r\r\r\r\r\r\r\r\r\r\r\r\r\r\r\r\r\r\r\r\r\r\r\r\r\r\r", "ExpectedValue"=""}, {"Test_Name"="928. SetG15PullDown \"C\" \"4\"", "Step_Type"="", "LowLimit"=0.0, "HighLimit"=0.0, "RValue"="", "RStatus"="", "RetVal"="0", "Units"="", "header1"="=== CCD overvoltage protection test ====", "header2"="--- Start Pin Driver test for ASIC 2----\r\r\r\r\r\r\r\r\r\r\r\r\r\r\r\r\r\r\r\r\r\r\r\r\r\r\r\r\r\r\r\r\r\r\r\r\r\r\r\r\r\r\r\r\r\r\r\r\r\r\r\r\r\r\r\r\r\r\r\r\r\r\r\r\r\r\r\r\r\r\r\r\r\r", "ExpectedValue"=""}, {"Test_Name"="929. SetG15PullDown \"D\" \"4\"", "Step_Type"="", "LowLimit"=0.0, "HighLimit"=0.0, "RValue"="", "RStatus"="", "RetVal"="0", "Units"="", "header1"="=== CCD overvoltage protection test ====", "header2"="--- Start Pin Driver test for ASIC 2----\r\r\r\r\r\r\r\r\r\r\r\r\r\r\r\r\r\r\r\r\r\r\r\r\r\r\r\r\r\r\r\r\r\r\r\r\r\r\r\r\r\r\r\r\r\r\r\r\r\r\r\r\r\r\r\r\r\r\r\r\r\r\r\r\r\r\r\r\r\r\r\r\r\r\r", "ExpectedValue"=""}, {"Test_Name"="930. CheckCFAdc \"PD3\" \"2.2\" \"2.6\"", "Step_Type"="NumericLimitTest", "LowLimit"=2.2, "HighLimit"=2.6, "RValue"="2.4509999752044678", "RStatus"="PASS", "RetVal"="0", "Units"="Volts", "header1"="=== CCD overvoltage protection test ====", "header2"="--- Start Pin Driver test for ASIC 2----\r\r\r\r\r\r\r\r\r\r\r\r\r\r\r\r\r\r\r\r\r\r\r\r\r\r\r\r\r\r\r\r\r\r\r\r\r\r\r\r\r\r\r\r\r\r\r\r\r\r\r\r\r\r\r\r\r\r\r\r\r\r\r\r\r\r\r\r\r\r\r\r\r\r\r\r", "ExpectedValue"=""}, {"Test_Name"="931. CheckCFAdc \"PD4\" \"2.2\" \"2.6\"", "Step_Type"="NumericLimitTest", "LowLimit"=2.2, "HighLimit"=2.6, "RValue"="2.434999942779541", "RStatus"="PASS", "RetVal"="0", "Units"="Volts", "header1"="=== CCD overvoltage protection test ====", "header2"="--- Start Pin Driver test for ASIC 2----\r\r\r\r\r\r\r\r\r\r\r\r\r\r\r\r\r\r\r\r\r\r\r\r\r\r\r\r\r\r\r\r\r\r\r\r\r\r\r\r\r\r\r\r\r\r\r\r\r\r\r\r\r\r\r\r\r\r\r\r\r\r\r\r\r\r\r\r\r\r\r\r\r\r\r\r\r", "ExpectedValue"=""}, {"Test_Name"="934. SetG15PullUp \"C\" \"2\"", "Step_Type"="", "LowLimit"=0.0, "HighLimit"=0.0, "RValue"="", "RStatus"="", "RetVal"="0", "Units"="", "header1"="=== CCD overvoltage protection test ====", "header2"="--- Start Pin Driver test for ASIC 2----\r\r\r\r\r\r\r\r\r\r\r\r\r\r\r\r\r\r\r\r\r\r\r\r\r\r\r\r\r\r\r\r\r\r\r\r\r\r\r\r\r\r\r\r\r\r\r\r\r\r\r\r\r\r\r\r\r\r\r\r\r\r\r\r\r\r\r\r\r\r\r\r\r\r\r\r\r\r", "ExpectedValue"=""}, {"Test_Name"="935. SetG15PullUp \"D\" \"2\"", "Step_Type"="", "LowLimit"=0.0, "HighLimit"=0.0, "RValue"="", "RStatus"="", "RetVal"="0", "Units"="", "header1"="=== CCD overvoltage protection test ====", "header2"="--- Start Pin Driver test for ASIC 2----\r\r\r\r\r\r\r\r\r\r\r\r\r\r\r\r\r\r\r\r\r\r\r\r\r\r\r\r\r\r\r\r\r\r\r\r\r\r\r\r\r\r\r\r\r\r\r\r\r\r\r\r\r\r\r\r\r\r\r\r\r\r\r\r\r\r\r\r\r\r\r\r\r\r\r\r\r\r\r", "ExpectedValue"=""}, {"Test_Name"="936. SetG15PullDown \"C\" \"0\"", "Step_Type"="", "LowLimit"=0.0, "HighLimit"=0.0, "RValue"="", "RStatus"="", "RetVal"="0", "Units"="", "header1"="=== CCD overvoltage protection test ====", "header2"="--- Start Pin Driver test for ASIC 2----\r\r\r\r\r\r\r\r\r\r\r\r\r\r\r\r\r\r\r\r\r\r\r\r\r\r\r\r\r\r\r\r\r\r\r\r\r\r\r\r\r\r\r\r\r\r\r\r\r\r\r\r\r\r\r\r\r\r\r\r\r\r\r\r\r\r\r\r\r\r\r\r\r\r\r\r\r\r\r\r", "ExpectedValue"=""}, {"Test_Name"="937. SetG15PullDown \"D\" \"0\"", "Step_Type"="", "LowLimit"=0.0, "HighLimit"=0.0, "RValue"="", "RStatus"="", "RetVal"="0", "Units"="", "header1"="=== CCD overvoltage protection test ====", "header2"="--- Start Pin Driver test for ASIC 2----\r\r\r\r\r\r\r\r\r\r\r\r\r\r\r\r\r\r\r\r\r\r\r\r\r\r\r\r\r\r\r\r\r\r\r\r\r\r\r\r\r\r\r\r\r\r\r\r\r\r\r\r\r\r\r\r\r\r\r\r\r\r\r\r\r\r\r\r\r\r\r\r\r\r\r\r\r\r\r\r\r", "ExpectedValue"=""}, {"Test_Name"="938. CheckCFAdc \"PD3\" \"4.5\" \"5.0\"", "Step_Type"="NumericLimitTest", "LowLimit"=4.5, "HighLimit"=5.0, "RValue"="4.828000068664551", "RStatus"="PASS", "RetVal"="0", "Units"="Volts", "header1"="=== CCD overvoltage protection test ====", "header2"="--- Start Pin Driver test for ASIC 2----\r\r\r\r\r\r\r\r\r\r\r\r\r\r\r\r\r\r\r\r\r\r\r\r\r\r\r\r\r\r\r\r\r\r\r\r\r\r\r\r\r\r\r\r\r\r\r\r\r\r\r\r\r\r\r\r\r\r\r\r\r\r\r\r\r\r\r\r\r\r\r\r\r\r\r\r\r\r\r\r\r\r", "ExpectedValue"=""}, {"Test_Name"="939. CheckCFAdc \"PD4\" \"4.5\" \"5.0\"", "Step_Type"="NumericLimitTest", "LowLimit"=4.5, "HighLimit"=5.0, "RValue"="4.804999828338623", "RStatus"="PASS", "RetVal"="0", "Units"="Volts", "header1"="=== CCD overvoltage protection test ====", "header2"="--- Start Pin Driver test for ASIC 2----\r\r\r\r\r\r\r\r\r\r\r\r\r\r\r\r\r\r\r\r\r\r\r\r\r\r\r\r\r\r\r\r\r\r\r\r\r\r\r\r\r\r\r\r\r\r\r\r\r\r\r\r\r\r\r\r\r\r\r\r\r\r\r\r\r\r\r\r\r\r\r\r\r\r\r\r\r\r\r\r\r\r\r", "ExpectedValue"=""}, {"Test_Name"="940. ---", "Step_Type"="", "LowLimit"=0.0, "HighLimit"=0.0, "RValue"="", "RStatus"="", "RetVal"="", "Units"="", "header1"="=== CCD overvoltage protection test ====", "header2"="----------------------------------------\r", "ExpectedValue"=""}, {"Test_Name"="941. SetG15PullUp \"C\" \"2\"", "Step_Type"="", "LowLimit"=0.0, "HighLimit"=0.0, "RValue"="", "RStatus"="", "RetVal"="0", "Units"="", "header1"="=== CCD overvoltage protection test ====", "header2"="----------------------------------------\r\r", "ExpectedValue"=""}, {"Test_Name"="942. SetG15PullUp \"D\" \"2\"", "Step_Type"="", "LowLimit"=0.0, "HighLimit"=0.0, "RValue"="", "RStatus"="", "RetVal"="0", "Units"="", "header1"="=== CCD overvoltage protection test ====", "header2"="----------------------------------------\r\r\r", "ExpectedValue"=""}, {"Test_Name"="943. SetG15PullDown \"C\" \"5\"", "Step_Type"="", "LowLimit"=0.0, "HighLimit"=0.0, "RValue"="", "RStatus"="", "RetVal"="0", "Units"="", "header1"="=== CCD overvoltage protection test ====", "header2"="----------------------------------------\r\r\r\r", "ExpectedValue"=""}, {"Test_Name"="944. SetG15PullDown \"D\" \"5\"", "Step_Type"="", "LowLimit"=0.0, "HighLimit"=0.0, "RValue"="", "RStatus"="", "RetVal"="0", "Units"="", "header1"="=== CCD overvoltage protection test ====", "header2"="----------------------------------------\r\r\r\r\r", "ExpectedValue"=""}, {"Test_Name"="945. Pause \"500\"", "Step_Type"="", "LowLimit"=0.0, "HighLimit"=0.0, "RValue"="", "RStatus"="", "RetVal"="0", "Units"="", "header1"="=== CCD overvoltage protection test ====", "header2"="----------------------------------------\r\r\r\r\r\r", "ExpectedValue"=""}, {"Test_Name"="946. CheckCFAdc \"PD3\" \"-.15\" \".3\"", "Step_Type"="NumericLimitTest", "LowLimit"=-0.15, "HighLimit"=0.3, "RValue"="0.017999999225139618", "RStatus"="PASS", "RetVal"="0", "Units"="Volts", "header1"="=== CCD overvoltage protection test ====", "header2"="----------------------------------------\r\r\r\r\r\r\r", "ExpectedValue"=""}, {"Test_Name"="947. CheckCFAdc \"PD4\" \"-.15\" \".3\"", "Step_Type"="NumericLimitTest", "LowLimit"=-0.15, "HighLimit"=0.3, "RValue"="0.008999999612569809", "RStatus"="PASS", "RetVal"="0", "Units"="Volts", "header1"="=== CCD overvoltage protection test ====", "header2"="----------------------------------------\r\r\r\r\r\r\r\r", "ExpectedValue"=""}, {"Test_Name"="949. SetG15PullUp \"C\" \"0\"", "Step_Type"="", "LowLimit"=0.0, "HighLimit"=0.0, "RValue"="", "RStatus"="", "RetVal"="0", "Units"="", "header1"="=== CCD overvoltage protection test ====", "header2"="----------------------------------------\r\r\r\r\r\r\r\r\r", "ExpectedValue"=""}, {"Test_Name"="950. SetG15PullUp \"D\" \"0\"", "Step_Type"="", "LowLimit"=0.0, "HighLimit"=0.0, "RValue"="", "RStatus"="", "RetVal"="0", "Units"="", "header1"="=== CCD overvoltage protection test ====", "header2"="----------------------------------------\r\r\r\r\r\r\r\r\r\r", "ExpectedValue"=""}, {"Test_Name"="951. SetG15PullDown \"C\" \"0\"", "Step_Type"="", "LowLimit"=0.0, "HighLimit"=0.0, "RValue"="", "RStatus"="", "RetVal"="0", "Units"="", "header1"="=== CCD overvoltage protection test ====", "header2"="----------------------------------------\r\r\r\r\r\r\r\r\r\r\r", "ExpectedValue"=""}, {"Test_Name"="952. SetG15PullDown \"D\" \"0\"", "Step_Type"="", "LowLimit"=0.0, "HighLimit"=0.0, "RValue"="", "RStatus"="", "RetVal"="0", "Units"="", "header1"="=== CCD overvoltage protection test ====", "header2"="----------------------------------------\r\r\r\r\r\r\r\r\r\r\r\r", "ExpectedValue"=""}, {"Test_Name"="954. SelectAllMuxA \"2\" \"0\"", "Step_Type"="", "LowLimit"=0.0, "HighLimit"=0.0, "RValue"="", "RStatus"="", "RetVal"="0", "Units"="", "header1"="=== CCD overvoltage protection test ====", "header2"="----------------------------------------\r\r\r\r\r\r\r\r\r\r\r\r\r", "ExpectedValue"=""}, {"Test_Name"="955. SelectAllMuxB \"2\" \"0\"", "Step_Type"="", "LowLimit"=0.0, "HighLimit"=0.0, "RValue"="", "RStatus"="", "RetVal"="0", "Units"="", "header1"="=== CCD overvoltage protection test ====", "header2"="----------------------------------------\r\r\r\r\r\r\r\r\r\r\r\r\r\r", "ExpectedValue"=""}, {"Test_Name"="957. ---Start Pull Up to 15v test ASIC 2---", "Step_Type"="", "LowLimit"=0.0, "HighLimit"=0.0, "RValue"="", "RStatus"="", "RetVal"="", "Units"="", "header1"="=== CCD overvoltage protection test ====", "header2"="---Start Pull Up to 15v test ASIC 2-----\r", "ExpectedValue"=""}, {"Test_Name"="960. SetG15PullUp \"C\" \"9\"", "Step_Type"="", "LowLimit"=0.0, "HighLimit"=0.0, "RValue"="", "RStatus"="", "RetVal"="0", "Units"="", "header1"="=== CCD overvoltage protection test ====", "header2"="---Start Pull Up to 15v test ASIC 2-----\r\r", "ExpectedValue"=""}, {"Test_Name"="961. SetG15PullUp \"D\" \"9\"", "Step_Type"="", "LowLimit"=0.0, "HighLimit"=0.0, "RValue"="", "RStatus"="", "RetVal"="0", "Units"="", "header1"="=== CCD overvoltage protection test ====", "header2"="---Start Pull Up to 15v test ASIC 2-----\r\r\r", "ExpectedValue"=""}, {"Test_Name"="962. SetG15PullDown \"C\" \"4\"", "Step_Type"="", "LowLimit"=0.0, "HighLimit"=0.0, "RValue"="", "RStatus"="", "RetVal"="0", "Units"="", "header1"="=== CCD overvoltage protection test ====", "header2"="---Start Pull Up to 15v test ASIC 2-----\r\r\r\r", "ExpectedValue"=""}, {"Test_Name"="963. SetG15PullDown \"D\" \"4\"", "Step_Type"="", "LowLimit"=0.0, "HighLimit"=0.0, "RValue"="", "RStatus"="", "RetVal"="0", "Units"="", "header1"="=== CCD overvoltage protection test ====", "header2"="---Start Pull Up to 15v test ASIC 2-----\r\r\r\r\r", "ExpectedValue"=""}, {"Test_Name"="964. SetG15PullupVbat \"1\" \"1\"", "Step_Type"="", "LowLimit"=0.0, "HighLimit"=0.0, "RValue"="", "RStatus"="", "RetVal"="0", "Units"="", "header1"="=== CCD overvoltage protection test ====", "header2"="---Start Pull Up to 15v test ASIC 2-----\r\r\r\r\r\r", "ExpectedValue"=""}, {"Test_Name"="965. CheckCFAdc \"PD3\" \"6.95\" \"7.7\"", "Step_Type"="NumericLimitTest", "LowLimit"=6.95, "HighLimit"=7.7, "RValue"="7.315999984741211", "RStatus"="PASS", "RetVal"="0", "Units"="Volts", "header1"="=== CCD overvoltage protection test ====", "header2"="---Start Pull Up to 15v test ASIC 2-----\r\r\r\r\r\r\r", "ExpectedValue"=""}, {"Test_Name"="966. CheckCFAdc \"PD4\" \"6.95\" \"7.7\"", "Step_Type"="NumericLimitTest", "LowLimit"=6.95, "HighLimit"=7.7, "RValue"="7.26800012588501", "RStatus"="PASS", "RetVal"="0", "Units"="Volts", "header1"="=== CCD overvoltage protection test ====", "header2"="---Start Pull Up to 15v test ASIC 2-----\r\r\r\r\r\r\r\r", "ExpectedValue"=""}, {"Test_Name"="968. SetG15PullupVbat \"1\" \"0\"", "Step_Type"="", "LowLimit"=0.0, "HighLimit"=0.0, "RValue"="", "RStatus"="", "RetVal"="0", "Units"="", "header1"="=== CCD overvoltage protection test ====", "header2"="---Start Pull Up to 15v test ASIC 2-----\r\r\r\r\r\r\r\r\r", "ExpectedValue"=""}, {"Test_Name"="969. SetG15PullDown \"C\" \"0\"", "Step_Type"="", "LowLimit"=0.0, "HighLimit"=0.0, "RValue"="", "RStatus"="", "RetVal"="0", "Units"="", "header1"="=== CCD overvoltage protection test ====", "header2"="---Start Pull Up to 15v test ASIC 2-----\r\r\r\r\r\r\r\r\r\r", "ExpectedValue"=""}, {"Test_Name"="970. SetG15PullDown \"D\" \"0\"", "Step_Type"="", "LowLimit"=0.0, "HighLimit"=0.0, "RValue"="", "RStatus"="", "RetVal"="0", "Units"="", "header1"="=== CCD overvoltage protection test ====", "header2"="---Start Pull Up to 15v test ASIC 2-----\r\r\r\r\r\r\r\r\r\r\r", "ExpectedValue"=""}, {"Test_Name"="971. CheckCFAdc \"PD3\" \"4.5\" \"5.0\"", "Step_Type"="NumericLimitTest", "LowLimit"=4.5, "HighLimit"=5.0, "RValue"="4.817999839782715", "RStatus"="PASS", "RetVal"="0", "Units"="Volts", "header1"="=== CCD overvoltage protection test ====", "header2"="---Start Pull Up to 15v test ASIC 2-----\r\r\r\r\r\r\r\r\r\r\r\r", "ExpectedValue"=""}, {"Test_Name"="972. CheckCFAdc \"PD4\" \"4.5\" \"5.0\"", "Step_Type"="NumericLimitTest", "LowLimit"=4.5, "HighLimit"=5.0, "RValue"="4.804999828338623", "RStatus"="PASS", "RetVal"="0", "Units"="Volts", "header1"="=== CCD overvoltage protection test ====", "header2"="---Start Pull Up to 15v test ASIC 2-----\r\r\r\r\r\r\r\r\r\r\r\r\r", "ExpectedValue"=""}, {"Test_Name"="974. SetG15PullUp \"C\" \"0\"", "Step_Type"="", "LowLimit"=0.0, "HighLimit"=0.0, "RValue"="", "RStatus"="", "RetVal"="0", "Units"="", "header1"="=== CCD overvoltage protection test ====", "header2"="---Start Pull Up to 15v test ASIC 2-----\r\r\r\r\r\r\r\r\r\r\r\r\r\r", "ExpectedValue"=""}, {"Test_Name"="975. SetG15PullUp \"D\" \"0\"", "Step_Type"="", "LowLimit"=0.0, "HighLimit"=0.0, "RValue"="", "RStatus"="", "RetVal"="0", "Units"="", "header1"="=== CCD overvoltage protection test ====", "header2"="---Start Pull Up to 15v test ASIC 2-----\r\r\r\r\r\r\r\r\r\r\r\r\r\r\r", "ExpectedValue"=""}, {"Test_Name"="976. SetG15PullDown \"C\" \"0\"", "Step_Type"="", "LowLimit"=0.0, "HighLimit"=0.0, "RValue"="", "RStatus"="", "RetVal"="0", "Units"="", "header1"="=== CCD overvoltage protection test ====", "header2"="---Start Pull Up to 15v test ASIC 2-----\r\r\r\r\r\r\r\r\r\r\r\r\r\r\r\r", "ExpectedValue"=""}, {"Test_Name"="977. SetG15PullDown \"D\" \"0\"", "Step_Type"="", "LowLimit"=0.0, "HighLimit"=0.0, "RValue"="", "RStatus"="", "RetVal"="0", "Units"="", "header1"="=== CCD overvoltage protection test ====", "header2"="---Start Pull Up to 15v test ASIC 2-----\r\r\r\r\r\r\r\r\r\r\r\r\r\r\r\r\r", "ExpectedValue"=""}, {"Test_Name"="979. --- DAC Comparator Tests ASIC 2 ---", "Step_Type"="", "LowLimit"=0.0, "HighLimit"=0.0, "RValue"="", "RStatus"="", "RetVal"="", "Units"="", "header1"="=== CCD overvoltage protection test ====", "header2"="--- DAC Comparator Tests ASIC 2 --------\r", "ExpectedValue"=""}, {"Test_Name"="981. SetBaud \"1\"", "Step_Type"="", "LowLimit"=0.0, "HighLimit"=0.0, "RValue"="", "RStatus"="", "RetVal"="0", "Units"="", "header1"="=== CCD overvoltage protection test ====", "header2"="--- DAC Comparator Tests ASIC 2 --------\r\r", "ExpectedValue"=""}, {"Test_Name"="982. SelectMuxA \"2\" \"9\" \"1\"", "Step_Type"="", "LowLimit"=0.0, "HighLimit"=0.0, "RValue"="", "RStatus"="", "RetVal"="0", "Units"="", "header1"="=== CCD overvoltage protection test ====", "header2"="--- DAC Comparator Tests ASIC 2 --------\r\r\r", "ExpectedValue"=""}, {"Test_Name"="983. SelectMuxA \"2\" \"15\" \"1\"", "Step_Type"="", "LowLimit"=0.0, "HighLimit"=0.0, "RValue"="", "RStatus"="", "RetVal"="0", "Units"="", "header1"="=== CCD overvoltage protection test ====", "header2"="--- DAC Comparator Tests ASIC 2 --------\r\r\r\r", "ExpectedValue"=""}, {"Test_Name"="986. SetG15PullUp \"C\" \"9\"", "Step_Type"="", "LowLimit"=0.0, "HighLimit"=0.0, "RValue"="", "RStatus"="", "RetVal"="0", "Units"="", "header1"="=== CCD overvoltage protection test ====", "header2"="--- DAC Comparator Tests ASIC 2 --------\r\r\r\r\r", "ExpectedValue"=""}, {"Test_Name"="987. SetG15PullUp \"D\" \"9\"", "Step_Type"="", "LowLimit"=0.0, "HighLimit"=0.0, "RValue"="", "RStatus"="", "RetVal"="0", "Units"="", "header1"="=== CCD overvoltage protection test ====", "header2"="--- DAC Comparator Tests ASIC 2 --------\r\r\r\r\r\r", "ExpectedValue"=""}, {"Test_Name"="988. SetG15PullDown \"C\" \"4\"", "Step_Type"="", "LowLimit"=0.0, "HighLimit"=0.0, "RValue"="", "RStatus"="", "RetVal"="0", "Units"="", "header1"="=== CCD overvoltage protection test ====", "header2"="--- DAC Comparator Tests ASIC 2 --------\r\r\r\r\r\r\r", "ExpectedValue"=""}, {"Test_Name"="989. SetG15PullDown \"D\" \"4\"", "Step_Type"="", "LowLimit"=0.0, "HighLimit"=0.0, "RValue"="", "RStatus"="", "RetVal"="0", "Units"="", "header1"="=== CCD overvoltage protection test ====", "header2"="--- DAC Comparator Tests ASIC 2 --------\r\r\r\r\r\r\r\r", "ExpectedValue"=""}, {"Test_Name"="991. CheckCFAdc \"PD3\" \"2.2\" \"2.6\"", "Step_Type"="NumericLimitTest", "LowLimit"=2.2, "HighLimit"=2.6, "RValue"="2.440999984741211", "RStatus"="PASS", "RetVal"="0", "Units"="Volts", "header1"="=== CCD overvoltage protection test ====", "header2"="--- DAC Comparator Tests ASIC 2 --------\r\r\r\r\r\r\r\r\r", "ExpectedValue"=""}, {"Test_Name"="994. SetReference \"53\"", "Step_Type"="", "LowLimit"=0.0, "HighLimit"=0.0, "RValue"="", "RStatus"="", "RetVal"="0", "Units"="", "header1"="=== CCD overvoltage protection test ====", "header2"="--- DAC Comparator Tests ASIC 2 --------\r\r\r\r\r\r\r\r\r\r", "ExpectedValue"=""}, {"Test_Name"="995. Pause \"100\"", "Step_Type"="", "LowLimit"=0.0, "HighLimit"=0.0, "RValue"="", "RStatus"="", "RetVal"="0", "Units"="", "header1"="=== CCD overvoltage protection test ====", "header2"="--- DAC Comparator Tests ASIC 2 --------\r\r\r\r\r\r\r\r\r\r\r", "ExpectedValue"=""}, {"Test_Name"="996. CheckFpgaRegister \"8A8\" \"2\" \"0\"", "Step_Type"="StringValueTest", "LowLimit"=0.0, "HighLimit"=0.0, "RValue"="3", "RStatus"="PASS", "RetVal"="0", "Units"="", "header1"="=== CCD overvoltage protection test ====", "header2"="--- DAC Comparator Tests ASIC 2 --------\r\r\r\r\r\r\r\r\r\r\r\r", "ExpectedValue"=""}, {"Test_Name"="997. CheckFpgaRegister \"8A8\" \"3\" \"0\"", "Step_Type"="StringValueTest", "LowLimit"=0.0, "HighLimit"=0.0, "RValue"="3", "RStatus"="PASS", "RetVal"="0", "Units"="", "header1"="=== CCD overvoltage protection test ====", "header2"="--- DAC Comparator Tests ASIC 2 --------\r\r\r\r\r\r\r\r\r\r\r\r\r", "ExpectedValue"=""}, {"Test_Name"="1000. SetReference \"65\"", "Step_Type"="", "LowLimit"=0.0, "HighLimit"=0.0, "RValue"="", "RStatus"="", "RetVal"="0", "Units"="", "header1"="=== CCD overvoltage protection test ====", "header2"="--- DAC Comparator Tests ASIC 2 --------\r\r\r\r\r\r\r\r\r\r\r\r\r\r", "ExpectedValue"=""}, {"Test_Name"="1001. Pause \"100\"", "Step_Type"="", "LowLimit"=0.0, "HighLimit"=0.0, "RValue"="", "RStatus"="", "RetVal"="0", "Units"="", "header1"="=== CCD overvoltage protection test ====", "header2"="--- DAC Comparator Tests ASIC 2 --------\r\r\r\r\r\r\r\r\r\r\r\r\r\r\r", "ExpectedValue"=""}, {"Test_Name"="1002. CheckFpgaRegister \"8A8\" \"2\" \"1\"", "Step_Type"="StringValueTest", "LowLimit"=0.0, "HighLimit"=0.0, "RValue"="15", "RStatus"="PASS", "RetVal"="0", "Units"="", "header1"="=== CCD overvoltage protection test ====", "header2"="--- DAC Comparator Tests ASIC 2 --------\r\r\r\r\r\r\r\r\r\r\r\r\r\r\r\r", "ExpectedValue"=""}, {"Test_Name"="1003. CheckFpgaRegister \"8A8\" \"3\" \"1\"", "Step_Type"="StringValueTest", "LowLimit"=0.0, "HighLimit"=0.0, "RValue"="15", "RStatus"="PASS", "RetVal"="0", "Units"="", "header1"="=== CCD overvoltage protection test ====", "header2"="--- DAC Comparator Tests ASIC 2 --------\r\r\r\r\r\r\r\r\r\r\r\r\r\r\r\r\r", "ExpectedValue"=""}, {"Test_Name"="1005. SetReference \"128\"", "Step_Type"="", "LowLimit"=0.0, "HighLimit"=0.0, "RValue"="", "RStatus"="", "RetVal"="0", "Units"="", "header1"="=== CCD overvoltage protection test ====", "header2"="--- DAC Comparator Tests ASIC 2 --------\r\r\r\r\r\r\r\r\r\r\r\r\r\r\r\r\r\r", "ExpectedValue"=""}, {"Test_Name"="1006. SelectAllMuxA \"2\" \"0\"", "Step_Type"="", "LowLimit"=0.0, "HighLimit"=0.0, "RValue"="", "RStatus"="", "RetVal"="0", "Units"="", "header1"="=== CCD overvoltage protection test ====", "header2"="--- DAC Comparator Tests ASIC 2 --------\r\r\r\r\r\r\r\r\r\r\r\r\r\r\r\r\r\r\r", "ExpectedValue"=""}, {"Test_Name"="1007. SelectAllMuxB \"2\" \"0\"", "Step_Type"="", "LowLimit"=0.0, "HighLimit"=0.0, "RValue"="", "RStatus"="", "RetVal"="0", "Units"="", "header1"="=== CCD overvoltage protection test ====", "header2"="--- DAC Comparator Tests ASIC 2 --------\r\r\r\r\r\r\r\r\r\r\r\r\r\r\r\r\r\r\r\r", "ExpectedValue"=""}, {"Test_Name"="1008. SetG15PullUp \"C\" \"0\"", "Step_Type"="", "LowLimit"=0.0, "HighLimit"=0.0, "RValue"="", "RStatus"="", "RetVal"="0", "Units"="", "header1"="=== CCD overvoltage protection test ====", "header2"="--- DAC Comparator Tests ASIC 2 --------\r\r\r\r\r\r\r\r\r\r\r\r\r\r\r\r\r\r\r\r\r", "ExpectedValue"=""}, {"Test_Name"="1009. SetG15PullUp \"D\" \"0\"", "Step_Type"="", "LowLimit"=0.0, "HighLimit"=0.0, "RValue"="", "RStatus"="", "RetVal"="0", "Units"="", "header1"="=== CCD overvoltage protection test ====", "header2"="--- DAC Comparator Tests ASIC 2 --------\r\r\r\r\r\r\r\r\r\r\r\r\r\r\r\r\r\r\r\r\r\r", "ExpectedValue"=""}, {"Test_Name"="1010. SetG15PullDown \"C\" \"0\"", "Step_Type"="", "LowLimit"=0.0, "HighLimit"=0.0, "RValue"="", "RStatus"="", "RetVal"="0", "Units"="", "header1"="=== CCD overvoltage protection test ====", "header2"="--- DAC Comparator Tests ASIC 2 --------\r\r\r\r\r\r\r\r\r\r\r\r\r\r\r\r\r\r\r\r\r\r\r", "ExpectedValue"=""}, {"Test_Name"="1011. SetG15PullDown \"D\" \"0\"", "Step_Type"="", "LowLimit"=0.0, "HighLimit"=0.0, "RValue"="", "RStatus"="", "RetVal"="0", "Units"="", "header1"="=== CCD overvoltage protection test ====", "header2"="--- DAC Comparator Tests ASIC 2 --------\r\r\r\r\r\r\r\r\r\r\r\r\r\r\r\r\r\r\r\r\r\r\r\r", "ExpectedValue"=""}, {"Test_Name"="1014. --- Start Switch Matrix 1B MUX B (ASIC 1) and Switch Matrix 1B MUX D (ASIC 2) ---", "Step_Type"="", "LowLimit"=0.0, "HighLimit"=0.0, "RValue"="", "RStatus"="", "RetVal"="", "Units"="", "header1"="=== CCD overvoltage protection test ====", "header2"="--- Start Switch Matrix 1B MUX B (ASIC 1) and Switch Matrix 1B MUX D (ASIC 2) ---\r", "ExpectedValue"=""}, {"Test_Name"="1018. SelectAllMuxB \"1\" \"0\"", "Step_Type"="", "LowLimit"=0.0, "HighLimit"=0.0, "RValue"="", "RStatus"="", "RetVal"="0", "Units"="", "header1"="=== CCD overvoltage protection test ====", "header2"="--- Start Switch Matrix 1B MUX B (ASIC 1) and Switch Matrix 1B MUX D (ASIC 2) ---\r\r", "ExpectedValue"=""}, {"Test_Name"="1019. SelectAllMuxB \"2\" \"0\"", "Step_Type"="", "LowLimit"=0.0, "HighLimit"=0.0, "RValue"="", "RStatus"="", "RetVal"="0", "Units"="", "header1"="=== CCD overvoltage protection test ====", "header2"="--- Start Switch Matrix 1B MUX B (ASIC 1) and Switch Matrix 1B MUX D (ASIC 2) ---\r\r\r", "ExpectedValue"=""}, {"Test_Name"="1022. SetG15PullUp \"B\" \"9\"", "Step_Type"="", "LowLimit"=0.0, "HighLimit"=0.0, "RValue"="", "RStatus"="", "RetVal"="0", "Units"="", "header1"="=== CCD overvoltage protection test ====", "header2"="--- Start Switch Matrix 1B MUX B (ASIC 1) and Switch Matrix 1B MUX D (ASIC 2) ---\r\r\r\r", "ExpectedValue"=""}, {"Test_Name"="1023. SetG15PullUp \"D\" \"0\"", "Step_Type"="", "LowLimit"=0.0, "HighLimit"=0.0, "RValue"="", "RStatus"="", "RetVal"="0", "Units"="", "header1"="=== CCD overvoltage protection test ====", "header2"="--- Start Switch Matrix 1B MUX B (ASIC 1) and Switch Matrix 1B MUX D (ASIC 2) ---\r\r\r\r\r", "ExpectedValue"=""}, {"Test_Name"="1024. SetG15PullDown \"B\" \"4\"", "Step_Type"="", "LowLimit"=0.0, "HighLimit"=0.0, "RValue"="", "RStatus"="", "RetVal"="0", "Units"="", "header1"="=== CCD overvoltage protection test ====", "header2"="--- Start Switch Matrix 1B MUX B (ASIC 1) and Switch Matrix 1B MUX D (ASIC 2) ---\r\r\r\r\r\r", "ExpectedValue"=""}, {"Test_Name"="1025. SetG15PullDown \"D\" \"0\"", "Step_Type"="", "LowLimit"=0.0, "HighLimit"=0.0, "RValue"="", "RStatus"="", "RetVal"="0", "Units"="", "header1"="=== CCD overvoltage protection test ====", "header2"="--- Start Switch Matrix 1B MUX B (ASIC 1) and Switch Matrix 1B MUX D (ASIC 2) ---\r\r\r\r\r\r\r", "ExpectedValue"=""}, {"Test_Name"="1026. CheckCFAdc \"PD2\" \"2.2\" \"2.65\"", "Step_Type"="NumericLimitTest", "LowLimit"=2.2, "HighLimit"=2.65, "RValue"="2.4549999237060547", "RStatus"="PASS", "RetVal"="0", "Units"="Volts", "header1"="=== CCD overvoltage protection test ====", "header2"="--- Start Switch Matrix 1B MUX B (ASIC 1) and Switch Matrix 1B MUX D (ASIC 2) ---\r\r\r\r\r\r\r\r", "ExpectedValue"=""}, {"Test_Name"="1027. CheckCFAdc \"PD4\" \"-.15\" \"1.1\"", "Step_Type"="NumericLimitTest", "LowLimit"=-0.15, "HighLimit"=1.1, "RValue"="0.7120000123977661", "RStatus"="PASS", "RetVal"="0", "Units"="Volts", "header1"="=== CCD overvoltage protection test ====", "header2"="--- Start Switch Matrix 1B MUX B (ASIC 1) and Switch Matrix 1B MUX D (ASIC 2) ---\r\r\r\r\r\r\r\r\r", "ExpectedValue"=""}, {"Test_Name"="1029. SelectMuxB \"1\" \"1\" \"1\"", "Step_Type"="", "LowLimit"=0.0, "HighLimit"=0.0, "RValue"="", "RStatus"="", "RetVal"="0", "Units"="", "header1"="=== CCD overvoltage protection test ====", "header2"="--- Start Switch Matrix 1B MUX B (ASIC 1) and Switch Matrix 1B MUX D (ASIC 2) ---\r\r\r\r\r\r\r\r\r\r", "ExpectedValue"=""}, {"Test_Name"="1030. SelectMuxB \"2\" \"1\" \"1\"", "Step_Type"="", "LowLimit"=0.0, "HighLimit"=0.0, "RValue"="", "RStatus"="", "RetVal"="0", "Units"="", "header1"="=== CCD overvoltage protection test ====", "header2"="--- Start Switch Matrix 1B MUX B (ASIC 1) and Switch Matrix 1B MUX D (ASIC 2) ---\r\r\r\r\r\r\r\r\r\r\r", "ExpectedValue"=""}, {"Test_Name"="1031. CheckCFAdc \"PD4\" \"2.2\" \"2.65\"", "Step_Type"="NumericLimitTest", "LowLimit"=2.2, "HighLimit"=2.65, "RValue"="2.453000068664551", "RStatus"="PASS", "RetVal"="0", "Units"="Volts", "header1"="=== CCD overvoltage protection test ====", "header2"="--- Start Switch Matrix 1B MUX B (ASIC 1) and Switch Matrix 1B MUX D (ASIC 2) ---\r\r\r\r\r\r\r\r\r\r\r\r", "ExpectedValue"=""}, {"Test_Name"="1032. SelectAllMuxB \"1\" \"0\"", "Step_Type"="", "LowLimit"=0.0, "HighLimit"=0.0, "RValue"="", "RStatus"="", "RetVal"="0", "Units"="", "header1"="=== CCD overvoltage protection test ====", "header2"="--- Start Switch Matrix 1B MUX B (ASIC 1) and Switch Matrix 1B MUX D (ASIC 2) ---\r\r\r\r\r\r\r\r\r\r\r\r\r", "ExpectedValue"=""}, {"Test_Name"="1033. SelectAllMuxB \"2\" \"0\"", "Step_Type"="", "LowLimit"=0.0, "HighLimit"=0.0, "RValue"="", "RStatus"="", "RetVal"="0", "Units"="", "header1"="=== CCD overvoltage protection test ====", "header2"="--- Start Switch Matrix 1B MUX B (ASIC 1) and Switch Matrix 1B MUX D (ASIC 2) ---\r\r\r\r\r\r\r\r\r\r\r\r\r\r", "ExpectedValue"=""}, {"Test_Name"="1035. SelectMuxB \"1\" \"2\" \"1\"", "Step_Type"="", "LowLimit"=0.0, "HighLimit"=0.0, "RValue"="", "RStatus"="", "RetVal"="0", "Units"="", "header1"="=== CCD overvoltage protection test ====", "header2"="--- Start Switch Matrix 1B MUX B (ASIC 1) and Switch Matrix 1B MUX D (ASIC 2) ---\r\r\r\r\r\r\r\r\r\r\r\r\r\r\r", "ExpectedValue"=""}, {"Test_Name"="1036. SelectMuxB \"2\" \"2\" \"1\"", "Step_Type"="", "LowLimit"=0.0, "HighLimit"=0.0, "RValue"="", "RStatus"="", "RetVal"="0", "Units"="", "header1"="=== CCD overvoltage protection test ====", "header2"="--- Start Switch Matrix 1B MUX B (ASIC 1) and Switch Matrix 1B MUX D (ASIC 2) ---\r\r\r\r\r\r\r\r\r\r\r\r\r\r\r\r", "ExpectedValue"=""}, {"Test_Name"="1037. CheckCFAdc \"PD4\" \"2.2\" \"2.65\"", "Step_Type"="NumericLimitTest", "LowLimit"=2.2, "HighLimit"=2.65, "RValue"="2.4619998931884766", "RStatus"="PASS", "RetVal"="0", "Units"="Volts", "header1"="=== CCD overvoltage protection test ====", "header2"="--- Start Switch Matrix 1B MUX B (ASIC 1) and Switch Matrix 1B MUX D (ASIC 2) ---\r\r\r\r\r\r\r\r\r\r\r\r\r\r\r\r\r", "ExpectedValue"=""}, {"Test_Name"="1038. SelectAllMuxB \"1\" \"0\"", "Step_Type"="", "LowLimit"=0.0, "HighLimit"=0.0, "RValue"="", "RStatus"="", "RetVal"="0", "Units"="", "header1"="=== CCD overvoltage protection test ====", "header2"="--- Start Switch Matrix 1B MUX B (ASIC 1) and Switch Matrix 1B MUX D (ASIC 2) ---\r\r\r\r\r\r\r\r\r\r\r\r\r\r\r\r\r\r", "ExpectedValue"=""}, {"Test_Name"="1039. SelectAllMuxB \"2\" \"0\"", "Step_Type"="", "LowLimit"=0.0, "HighLimit"=0.0, "RValue"="", "RStatus"="", "RetVal"="0", "Units"="", "header1"="=== CCD overvoltage protection test ====", "header2"="--- Start Switch Matrix 1B MUX B (ASIC 1) and Switch Matrix 1B MUX D (ASIC 2) ---\r\r\r\r\r\r\r\r\r\r\r\r\r\r\r\r\r\r\r", "ExpectedValue"=""}, {"Test_Name"="1041. SelectMuxB \"1\" \"3\" \"1\"", "Step_Type"="", "LowLimit"=0.0, "HighLimit"=0.0, "RValue"="", "RStatus"="", "RetVal"="0", "Units"="", "header1"="=== CCD overvoltage protection test ====", "header2"="--- Start Switch Matrix 1B MUX B (ASIC 1) and Switch Matrix 1B MUX D (ASIC 2) ---\r\r\r\r\r\r\r\r\r\r\r\r\r\r\r\r\r\r\r\r", "ExpectedValue"=""}, {"Test_Name"="1042. SelectMuxB \"2\" \"3\" \"1\"", "Step_Type"="", "LowLimit"=0.0, "HighLimit"=0.0, "RValue"="", "RStatus"="", "RetVal"="0", "Units"="", "header1"="=== CCD overvoltage protection test ====", "header2"="--- Start Switch Matrix 1B MUX B (ASIC 1) and Switch Matrix 1B MUX D (ASIC 2) ---\r\r\r\r\r\r\r\r\r\r\r\r\r\r\r\r\r\r\r\r\r", "ExpectedValue"=""}, {"Test_Name"="1043. CheckCFAdc \"PD4\" \"2.2\" \"2.65\"", "Step_Type"="NumericLimitTest", "LowLimit"=2.2, "HighLimit"=2.65, "RValue"="2.453000068664551", "RStatus"="PASS", "RetVal"="0", "Units"="Volts", "header1"="=== CCD overvoltage protection test ====", "header2"="--- Start Switch Matrix 1B MUX B (ASIC 1) and Switch Matrix 1B MUX D (ASIC 2) ---\r\r\r\r\r\r\r\r\r\r\r\r\r\r\r\r\r\r\r\r\r\r", "ExpectedValue"=""}, {"Test_Name"="1044. SelectAllMuxB \"1\" \"0\"", "Step_Type"="", "LowLimit"=0.0, "HighLimit"=0.0, "RValue"="", "RStatus"="", "RetVal"="0", "Units"="", "header1"="=== CCD overvoltage protection test ====", "header2"="--- Start Switch Matrix 1B MUX B (ASIC 1) and Switch Matrix 1B MUX D (ASIC 2) ---\r\r\r\r\r\r\r\r\r\r\r\r\r\r\r\r\r\r\r\r\r\r\r", "ExpectedValue"=""}, {"Test_Name"="1045. SelectAllMuxB \"2\" \"0\"", "Step_Type"="", "LowLimit"=0.0, "HighLimit"=0.0, "RValue"="", "RStatus"="", "RetVal"="0", "Units"="", "header1"="=== CCD overvoltage protection test ====", "header2"="--- Start Switch Matrix 1B MUX B (ASIC 1) and Switch Matrix 1B MUX D (ASIC 2) ---\r\r\r\r\r\r\r\r\r\r\r\r\r\r\r\r\r\r\r\r\r\r\r\r", "ExpectedValue"=""}, {"Test_Name"="1047. SelectMuxB \"1\" \"6\" \"1\"", "Step_Type"="", "LowLimit"=0.0, "HighLimit"=0.0, "RValue"="", "RStatus"="", "RetVal"="0", "Units"="", "header1"="=== CCD overvoltage protection test ====", "header2"="--- Start Switch Matrix 1B MUX B (ASIC 1) and Switch Matrix 1B MUX D (ASIC 2) ---\r\r\r\r\r\r\r\r\r\r\r\r\r\r\r\r\r\r\r\r\r\r\r\r\r", "ExpectedValue"=""}, {"Test_Name"="1048. SelectMuxB \"2\" \"6\" \"1\"", "Step_Type"="", "LowLimit"=0.0, "HighLimit"=0.0, "RValue"="", "RStatus"="", "RetVal"="0", "Units"="", "header1"="=== CCD overvoltage protection test ====", "header2"="--- Start Switch Matrix 1B MUX B (ASIC 1) and Switch Matrix 1B MUX D (ASIC 2) ---\r\r\r\r\r\r\r\r\r\r\r\r\r\r\r\r\r\r\r\r\r\r\r\r\r\r", "ExpectedValue"=""}, {"Test_Name"="1049. CheckCFAdc \"PD4\" \"2.2\" \"2.65\"", "Step_Type"="NumericLimitTest", "LowLimit"=2.2, "HighLimit"=2.65, "RValue"="2.4619998931884766", "RStatus"="PASS", "RetVal"="0", "Units"="Volts", "header1"="=== CCD overvoltage protection test ====", "header2"="--- Start Switch Matrix 1B MUX B (ASIC 1) and Switch Matrix 1B MUX D (ASIC 2) ---\r\r\r\r\r\r\r\r\r\r\r\r\r\r\r\r\r\r\r\r\r\r\r\r\r\r\r", "ExpectedValue"=""}, {"Test_Name"="1050. SelectAllMuxB \"1\" \"0\"", "Step_Type"="", "LowLimit"=0.0, "HighLimit"=0.0, "RValue"="", "RStatus"="", "RetVal"="0", "Units"="", "header1"="=== CCD overvoltage protection test ====", "header2"="--- Start Switch Matrix 1B MUX B (ASIC 1) and Switch Matrix 1B MUX D (ASIC 2) ---\r\r\r\r\r\r\r\r\r\r\r\r\r\r\r\r\r\r\r\r\r\r\r\r\r\r\r\r", "ExpectedValue"=""}, {"Test_Name"="1051. SelectAllMuxB \"2\" \"0\"", "Step_Type"="", "LowLimit"=0.0, "HighLimit"=0.0, "RValue"="", "RStatus"="", "RetVal"="0", "Units"="", "header1"="=== CCD overvoltage protection test ====", "header2"="--- Start Switch Matrix 1B MUX B (ASIC 1) and Switch Matrix 1B MUX D (ASIC 2) ---\r\r\r\r\r\r\r\r\r\r\r\r\r\r\r\r\r\r\r\r\r\r\r\r\r\r\r\r\r", "ExpectedValue"=""}, {"Test_Name"="1053. SelectMuxB \"1\" \"7\" \"1\"", "Step_Type"="", "LowLimit"=0.0, "HighLimit"=0.0, "RValue"="", "RStatus"="", "RetVal"="0", "Units"="", "header1"="=== CCD overvoltage protection test ====", "header2"="--- Start Switch Matrix 1B MUX B (ASIC 1) and Switch Matrix 1B MUX D (ASIC 2) ---\r\r\r\r\r\r\r\r\r\r\r\r\r\r\r\r\r\r\r\r\r\r\r\r\r\r\r\r\r\r", "ExpectedValue"=""}, {"Test_Name"="1054. SelectMuxB \"2\" \"7\" \"1\"", "Step_Type"="", "LowLimit"=0.0, "HighLimit"=0.0, "RValue"="", "RStatus"="", "RetVal"="0", "Units"="", "header1"="=== CCD overvoltage protection test ====", "header2"="--- Start Switch Matrix 1B MUX B (ASIC 1) and Switch Matrix 1B MUX D (ASIC 2) ---\r\r\r\r\r\r\r\r\r\r\r\r\r\r\r\r\r\r\r\r\r\r\r\r\r\r\r\r\r\r\r", "ExpectedValue"=""}, {"Test_Name"="1055. CheckCFAdc \"PD4\" \"2.2\" \"2.65\"", "Step_Type"="NumericLimitTest", "LowLimit"=2.2, "HighLimit"=2.65, "RValue"="2.444000005722046", "RStatus"="PASS", "RetVal"="0", "Units"="Volts", "header1"="=== CCD overvoltage protection test ====", "header2"="--- Start Switch Matrix 1B MUX B (ASIC 1) and Switch Matrix 1B MUX D (ASIC 2) ---\r\r\r\r\r\r\r\r\r\r\r\r\r\r\r\r\r\r\r\r\r\r\r\r\r\r\r\r\r\r\r\r", "ExpectedValue"=""}, {"Test_Name"="1056. SelectAllMuxB \"1\" \"0\"", "Step_Type"="", "LowLimit"=0.0, "HighLimit"=0.0, "RValue"="", "RStatus"="", "RetVal"="0", "Units"="", "header1"="=== CCD overvoltage protection test ====", "header2"="--- Start Switch Matrix 1B MUX B (ASIC 1) and Switch Matrix 1B MUX D (ASIC 2) ---\r\r\r\r\r\r\r\r\r\r\r\r\r\r\r\r\r\r\r\r\r\r\r\r\r\r\r\r\r\r\r\r\r", "ExpectedValue"=""}, {"Test_Name"="1057. SelectAllMuxB \"2\" \"0\"", "Step_Type"="", "LowLimit"=0.0, "HighLimit"=0.0, "RValue"="", "RStatus"="", "RetVal"="0", "Units"="", "header1"="=== CCD overvoltage protection test ====", "header2"="--- Start Switch Matrix 1B MUX B (ASIC 1) and Switch Matrix 1B MUX D (ASIC 2) ---\r\r\r\r\r\r\r\r\r\r\r\r\r\r\r\r\r\r\r\r\r\r\r\r\r\r\r\r\r\r\r\r\r\r", "ExpectedValue"=""}, {"Test_Name"="1059. SelectMuxB \"1\" \"8\" \"1\"", "Step_Type"="", "LowLimit"=0.0, "HighLimit"=0.0, "RValue"="", "RStatus"="", "RetVal"="0", "Units"="", "header1"="=== CCD overvoltage protection test ====", "header2"="--- Start Switch Matrix 1B MUX B (ASIC 1) and Switch Matrix 1B MUX D (ASIC 2) ---\r\r\r\r\r\r\r\r\r\r\r\r\r\r\r\r\r\r\r\r\r\r\r\r\r\r\r\r\r\r\r\r\r\r\r", "ExpectedValue"=""}, {"Test_Name"="1060. SelectMuxB \"2\" \"8\" \"1\"", "Step_Type"="", "LowLimit"=0.0, "HighLimit"=0.0, "RValue"="", "RStatus"="", "RetVal"="0", "Units"="", "header1"="=== CCD overvoltage protection test ====", "header2"="--- Start Switch Matrix 1B MUX B (ASIC 1) and Switch Matrix 1B MUX D (ASIC 2) ---\r\r\r\r\r\r\r\r\r\r\r\r\r\r\r\r\r\r\r\r\r\r\r\r\r\r\r\r\r\r\r\r\r\r\r\r", "ExpectedValue"=""}, {"Test_Name"="1061. CheckCFAdc \"PD4\" \"2.2\" \"2.65\"", "Step_Type"="NumericLimitTest", "LowLimit"=2.2, "HighLimit"=2.65, "RValue"="2.4619998931884766", "RStatus"="PASS", "RetVal"="0", "Units"="Volts", "header1"="=== CCD overvoltage protection test ====", "header2"="--- Start Switch Matrix 1B MUX B (ASIC 1) and Switch Matrix 1B MUX D (ASIC 2) ---\r\r\r\r\r\r\r\r\r\r\r\r\r\r\r\r\r\r\r\r\r\r\r\r\r\r\r\r\r\r\r\r\r\r\r\r\r", "ExpectedValue"=""}, {"Test_Name"="1062. SelectAllMuxB \"1\" \"0\"", "Step_Type"="", "LowLimit"=0.0, "HighLimit"=0.0, "RValue"="", "RStatus"="", "RetVal"="0", "Units"="", "header1"="=== CCD overvoltage protection test ====", "header2"="--- Start Switch Matrix 1B MUX B (ASIC 1) and Switch Matrix 1B MUX D (ASIC 2) ---\r\r\r\r\r\r\r\r\r\r\r\r\r\r\r\r\r\r\r\r\r\r\r\r\r\r\r\r\r\r\r\r\r\r\r\r\r\r", "ExpectedValue"=""}, {"Test_Name"="1063. SelectAllMuxB \"2\" \"0\"", "Step_Type"="", "LowLimit"=0.0, "HighLimit"=0.0, "RValue"="", "RStatus"="", "RetVal"="0", "Units"="", "header1"="=== CCD overvoltage protection test ====", "header2"="--- Start Switch Matrix 1B MUX B (ASIC 1) and Switch Matrix 1B MUX D (ASIC 2) ---\r\r\r\r\r\r\r\r\r\r\r\r\r\r\r\r\r\r\r\r\r\r\r\r\r\r\r\r\r\r\r\r\r\r\r\r\r\r\r", "ExpectedValue"=""}, {"Test_Name"="1065. SelectMuxB \"1\" \"9\" \"1\"", "Step_Type"="", "LowLimit"=0.0, "HighLimit"=0.0, "RValue"="", "RStatus"="", "RetVal"="0", "Units"="", "header1"="=== CCD overvoltage protection test ====", "header2"="--- Start Switch Matrix 1B MUX B (ASIC 1) and Switch Matrix 1B MUX D (ASIC 2) ---\r\r\r\r\r\r\r\r\r\r\r\r\r\r\r\r\r\r\r\r\r\r\r\r\r\r\r\r\r\r\r\r\r\r\r\r\r\r\r\r", "ExpectedValue"=""}, {"Test_Name"="1066. SelectMuxB \"2\" \"9\" \"1\"", "Step_Type"="", "LowLimit"=0.0, "HighLimit"=0.0, "RValue"="", "RStatus"="", "RetVal"="0", "Units"="", "header1"="=== CCD overvoltage protection test ====", "header2"="--- Start Switch Matrix 1B MUX B (ASIC 1) and Switch Matrix 1B MUX D (ASIC 2) ---\r\r\r\r\r\r\r\r\r\r\r\r\r\r\r\r\r\r\r\r\r\r\r\r\r\r\r\r\r\r\r\r\r\r\r\r\r\r\r\r\r", "ExpectedValue"=""}, {"Test_Name"="1067. CheckCFAdc \"PD4\" \"2.2\" \"2.65\"", "Step_Type"="NumericLimitTest", "LowLimit"=2.2, "HighLimit"=2.65, "RValue"="2.4619998931884766", "RStatus"="PASS", "RetVal"="0", "Units"="Volts", "header1"="=== CCD overvoltage protection test ====", "header2"="--- Start Switch Matrix 1B MUX B (ASIC 1) and Switch Matrix 1B MUX D (ASIC 2) ---\r\r\r\r\r\r\r\r\r\r\r\r\r\r\r\r\r\r\r\r\r\r\r\r\r\r\r\r\r\r\r\r\r\r\r\r\r\r\r\r\r\r", "ExpectedValue"=""}, {"Test_Name"="1068. SelectAllMuxB \"1\" \"0\"", "Step_Type"="", "LowLimit"=0.0, "HighLimit"=0.0, "RValue"="", "RStatus"="", "RetVal"="0", "Units"="", "header1"="=== CCD overvoltage protection test ====", "header2"="--- Start Switch Matrix 1B MUX B (ASIC 1) and Switch Matrix 1B MUX D (ASIC 2) ---\r\r\r\r\r\r\r\r\r\r\r\r\r\r\r\r\r\r\r\r\r\r\r\r\r\r\r\r\r\r\r\r\r\r\r\r\r\r\r\r\r\r\r", "ExpectedValue"=""}, {"Test_Name"="1069. SelectAllMuxB \"2\" \"0\"", "Step_Type"="", "LowLimit"=0.0, "HighLimit"=0.0, "RValue"="", "RStatus"="", "RetVal"="0", "Units"="", "header1"="=== CCD overvoltage protection test ====", "header2"="--- Start Switch Matrix 1B MUX B (ASIC 1) and Switch Matrix 1B MUX D (ASIC 2) ---\r\r\r\r\r\r\r\r\r\r\r\r\r\r\r\r\r\r\r\r\r\r\r\r\r\r\r\r\r\r\r\r\r\r\r\r\r\r\r\r\r\r\r\r", "ExpectedValue"=""}, {"Test_Name"="1071. SelectMuxB \"1\" \"10\" \"1\"", "Step_Type"="", "LowLimit"=0.0, "HighLimit"=0.0, "RValue"="", "RStatus"="", "RetVal"="0", "Units"="", "header1"="=== CCD overvoltage protection test ====", "header2"="--- Start Switch Matrix 1B MUX B (ASIC 1) and Switch Matrix 1B MUX D (ASIC 2) ---\r\r\r\r\r\r\r\r\r\r\r\r\r\r\r\r\r\r\r\r\r\r\r\r\r\r\r\r\r\r\r\r\r\r\r\r\r\r\r\r\r\r\r\r\r", "ExpectedValue"=""}, {"Test_Name"="1072. SelectMuxB \"2\" \"10\" \"1\"", "Step_Type"="", "LowLimit"=0.0, "HighLimit"=0.0, "RValue"="", "RStatus"="", "RetVal"="0", "Units"="", "header1"="=== CCD overvoltage protection test ====", "header2"="--- Start Switch Matrix 1B MUX B (ASIC 1) and Switch Matrix 1B MUX D (ASIC 2) ---\r\r\r\r\r\r\r\r\r\r\r\r\r\r\r\r\r\r\r\r\r\r\r\r\r\r\r\r\r\r\r\r\r\r\r\r\r\r\r\r\r\r\r\r\r\r", "ExpectedValue"=""}, {"Test_Name"="1073. CheckCFAdc \"PD4\" \"2.2\" \"2.65\"", "Step_Type"="NumericLimitTest", "LowLimit"=2.2, "HighLimit"=2.65, "RValue"="2.4619998931884766", "RStatus"="PASS", "RetVal"="0", "Units"="Volts", "header1"="=== CCD overvoltage protection test ====", "header2"="--- Start Switch Matrix 1B MUX B (ASIC 1) and Switch Matrix 1B MUX D (ASIC 2) ---\r\r\r\r\r\r\r\r\r\r\r\r\r\r\r\r\r\r\r\r\r\r\r\r\r\r\r\r\r\r\r\r\r\r\r\r\r\r\r\r\r\r\r\r\r\r\r", "ExpectedValue"=""}, {"Test_Name"="1074. SelectAllMuxB \"1\" \"0\"", "Step_Type"="", "LowLimit"=0.0, "HighLimit"=0.0, "RValue"="", "RStatus"="", "RetVal"="0", "Units"="", "header1"="=== CCD overvoltage protection test ====", "header2"="--- Start Switch Matrix 1B MUX B (ASIC 1) and Switch Matrix 1B MUX D (ASIC 2) ---\r\r\r\r\r\r\r\r\r\r\r\r\r\r\r\r\r\r\r\r\r\r\r\r\r\r\r\r\r\r\r\r\r\r\r\r\r\r\r\r\r\r\r\r\r\r\r\r", "ExpectedValue"=""}, {"Test_Name"="1075. SelectAllMuxB \"2\" \"0\"", "Step_Type"="", "LowLimit"=0.0, "HighLimit"=0.0, "RValue"="", "RStatus"="", "RetVal"="0", "Units"="", "header1"="=== CCD overvoltage protection test ====", "header2"="--- Start Switch Matrix 1B MUX B (ASIC 1) and Switch Matrix 1B MUX D (ASIC 2) ---\r\r\r\r\r\r\r\r\r\r\r\r\r\r\r\r\r\r\r\r\r\r\r\r\r\r\r\r\r\r\r\r\r\r\r\r\r\r\r\r\r\r\r\r\r\r\r\r\r", "ExpectedValue"=""}, {"Test_Name"="1077. SelectMuxB \"1\" \"11\" \"1\"", "Step_Type"="", "LowLimit"=0.0, "HighLimit"=0.0, "RValue"="", "RStatus"="", "RetVal"="0", "Units"="", "header1"="=== CCD overvoltage protection test ====", "header2"="--- Start Switch Matrix 1B MUX B (ASIC 1) and Switch Matrix 1B MUX D (ASIC 2) ---\r\r\r\r\r\r\r\r\r\r\r\r\r\r\r\r\r\r\r\r\r\r\r\r\r\r\r\r\r\r\r\r\r\r\r\r\r\r\r\r\r\r\r\r\r\r\r\r\r\r", "ExpectedValue"=""}, {"Test_Name"="1078. SelectMuxB \"2\" \"11\" \"1\"", "Step_Type"="", "LowLimit"=0.0, "HighLimit"=0.0, "RValue"="", "RStatus"="", "RetVal"="0", "Units"="", "header1"="=== CCD overvoltage protection test ====", "header2"="--- Start Switch Matrix 1B MUX B (ASIC 1) and Switch Matrix 1B MUX D (ASIC 2) ---\r\r\r\r\r\r\r\r\r\r\r\r\r\r\r\r\r\r\r\r\r\r\r\r\r\r\r\r\r\r\r\r\r\r\r\r\r\r\r\r\r\r\r\r\r\r\r\r\r\r\r", "ExpectedValue"=""}, {"Test_Name"="1079. CheckCFAdc \"PD4\" \"2.2\" \"2.65\"", "Step_Type"="NumericLimitTest", "LowLimit"=2.2, "HighLimit"=2.65, "RValue"="2.453000068664551", "RStatus"="PASS", "RetVal"="0", "Units"="Volts", "header1"="=== CCD overvoltage protection test ====", "header2"="--- Start Switch Matrix 1B MUX B (ASIC 1) and Switch Matrix 1B MUX D (ASIC 2) ---\r\r\r\r\r\r\r\r\r\r\r\r\r\r\r\r\r\r\r\r\r\r\r\r\r\r\r\r\r\r\r\r\r\r\r\r\r\r\r\r\r\r\r\r\r\r\r\r\r\r\r\r", "ExpectedValue"=""}, {"Test_Name"="1080. SelectAllMuxB \"1\" \"0\"", "Step_Type"="", "LowLimit"=0.0, "HighLimit"=0.0, "RValue"="", "RStatus"="", "RetVal"="0", "Units"="", "header1"="=== CCD overvoltage protection test ====", "header2"="--- Start Switch Matrix 1B MUX B (ASIC 1) and Switch Matrix 1B MUX D (ASIC 2) ---\r\r\r\r\r\r\r\r\r\r\r\r\r\r\r\r\r\r\r\r\r\r\r\r\r\r\r\r\r\r\r\r\r\r\r\r\r\r\r\r\r\r\r\r\r\r\r\r\r\r\r\r\r", "ExpectedValue"=""}, {"Test_Name"="1081. SelectAllMuxB \"2\" \"0\"", "Step_Type"="", "LowLimit"=0.0, "HighLimit"=0.0, "RValue"="", "RStatus"="", "RetVal"="0", "Units"="", "header1"="=== CCD overvoltage protection test ====", "header2"="--- Start Switch Matrix 1B MUX B (ASIC 1) and Switch Matrix 1B MUX D (ASIC 2) ---\r\r\r\r\r\r\r\r\r\r\r\r\r\r\r\r\r\r\r\r\r\r\r\r\r\r\r\r\r\r\r\r\r\r\r\r\r\r\r\r\r\r\r\r\r\r\r\r\r\r\r\r\r\r", "ExpectedValue"=""}, {"Test_Name"="1083. SelectMuxB \"1\" \"12\" \"1\"", "Step_Type"="", "LowLimit"=0.0, "HighLimit"=0.0, "RValue"="", "RStatus"="", "RetVal"="0", "Units"="", "header1"="=== CCD overvoltage protection test ====", "header2"="--- Start Switch Matrix 1B MUX B (ASIC 1) and Switch Matrix 1B MUX D (ASIC 2) ---\r\r\r\r\r\r\r\r\r\r\r\r\r\r\r\r\r\r\r\r\r\r\r\r\r\r\r\r\r\r\r\r\r\r\r\r\r\r\r\r\r\r\r\r\r\r\r\r\r\r\r\r\r\r\r", "ExpectedValue"=""}, {"Test_Name"="1084. SelectMuxB \"2\" \"12\" \"1\"", "Step_Type"="", "LowLimit"=0.0, "HighLimit"=0.0, "RValue"="", "RStatus"="", "RetVal"="0", "Units"="", "header1"="=== CCD overvoltage protection test ====", "header2"="--- Start Switch Matrix 1B MUX B (ASIC 1) and Switch Matrix 1B MUX D (ASIC 2) ---\r\r\r\r\r\r\r\r\r\r\r\r\r\r\r\r\r\r\r\r\r\r\r\r\r\r\r\r\r\r\r\r\r\r\r\r\r\r\r\r\r\r\r\r\r\r\r\r\r\r\r\r\r\r\r\r", "ExpectedValue"=""}, {"Test_Name"="1085. CheckCFAdc \"PD4\" \"2.2\" \"2.65\"", "Step_Type"="NumericLimitTest", "LowLimit"=2.2, "HighLimit"=2.65, "RValue"="2.4619998931884766", "RStatus"="PASS", "RetVal"="0", "Units"="Volts", "header1"="=== CCD overvoltage protection test ====", "header2"="--- Start Switch Matrix 1B MUX B (ASIC 1) and Switch Matrix 1B MUX D (ASIC 2) ---\r\r\r\r\r\r\r\r\r\r\r\r\r\r\r\r\r\r\r\r\r\r\r\r\r\r\r\r\r\r\r\r\r\r\r\r\r\r\r\r\r\r\r\r\r\r\r\r\r\r\r\r\r\r\r\r\r", "ExpectedValue"=""}, {"Test_Name"="1086. SelectAllMuxB \"1\" \"0\"", "Step_Type"="", "LowLimit"=0.0, "HighLimit"=0.0, "RValue"="", "RStatus"="", "RetVal"="0", "Units"="", "header1"="=== CCD overvoltage protection test ====", "header2"="--- Start Switch Matrix 1B MUX B (ASIC 1) and Switch Matrix 1B MUX D (ASIC 2) ---\r\r\r\r\r\r\r\r\r\r\r\r\r\r\r\r\r\r\r\r\r\r\r\r\r\r\r\r\r\r\r\r\r\r\r\r\r\r\r\r\r\r\r\r\r\r\r\r\r\r\r\r\r\r\r\r\r\r", "ExpectedValue"=""}, {"Test_Name"="1087. SelectAllMuxB \"2\" \"0\"", "Step_Type"="", "LowLimit"=0.0, "HighLimit"=0.0, "RValue"="", "RStatus"="", "RetVal"="0", "Units"="", "header1"="=== CCD overvoltage protection test ====", "header2"="--- Start Switch Matrix 1B MUX B (ASIC 1) and Switch Matrix 1B MUX D (ASIC 2) ---\r\r\r\r\r\r\r\r\r\r\r\r\r\r\r\r\r\r\r\r\r\r\r\r\r\r\r\r\r\r\r\r\r\r\r\r\r\r\r\r\r\r\r\r\r\r\r\r\r\r\r\r\r\r\r\r\r\r\r", "ExpectedValue"=""}, {"Test_Name"="1089. SelectMuxB \"1\" \"13\" \"1\"", "Step_Type"="", "LowLimit"=0.0, "HighLimit"=0.0, "RValue"="", "RStatus"="", "RetVal"="0", "Units"="", "header1"="=== CCD overvoltage protection test ====", "header2"="--- Start Switch Matrix 1B MUX B (ASIC 1) and Switch Matrix 1B MUX D (ASIC 2) ---\r\r\r\r\r\r\r\r\r\r\r\r\r\r\r\r\r\r\r\r\r\r\r\r\r\r\r\r\r\r\r\r\r\r\r\r\r\r\r\r\r\r\r\r\r\r\r\r\r\r\r\r\r\r\r\r\r\r\r\r", "ExpectedValue"=""}, {"Test_Name"="1090. SelectMuxB \"2\" \"13\" \"1\"", "Step_Type"="", "LowLimit"=0.0, "HighLimit"=0.0, "RValue"="", "RStatus"="", "RetVal"="0", "Units"="", "header1"="=== CCD overvoltage protection test ====", "header2"="--- Start Switch Matrix 1B MUX B (ASIC 1) and Switch Matrix 1B MUX D (ASIC 2) ---\r\r\r\r\r\r\r\r\r\r\r\r\r\r\r\r\r\r\r\r\r\r\r\r\r\r\r\r\r\r\r\r\r\r\r\r\r\r\r\r\r\r\r\r\r\r\r\r\r\r\r\r\r\r\r\r\r\r\r\r\r", "ExpectedValue"=""}, {"Test_Name"="1091. CheckCFAdc \"PD4\" \"2.2\" \"2.65\"", "Step_Type"="NumericLimitTest", "LowLimit"=2.2, "HighLimit"=2.65, "RValue"="2.4619998931884766", "RStatus"="PASS", "RetVal"="0", "Units"="Volts", "header1"="=== CCD overvoltage protection test ====", "header2"="--- Start Switch Matrix 1B MUX B (ASIC 1) and Switch Matrix 1B MUX D (ASIC 2) ---\r\r\r\r\r\r\r\r\r\r\r\r\r\r\r\r\r\r\r\r\r\r\r\r\r\r\r\r\r\r\r\r\r\r\r\r\r\r\r\r\r\r\r\r\r\r\r\r\r\r\r\r\r\r\r\r\r\r\r\r\r\r", "ExpectedValue"=""}, {"Test_Name"="1092. SelectAllMuxB \"1\" \"0\"", "Step_Type"="", "LowLimit"=0.0, "HighLimit"=0.0, "RValue"="", "RStatus"="", "RetVal"="0", "Units"="", "header1"="=== CCD overvoltage protection test ====", "header2"="--- Start Switch Matrix 1B MUX B (ASIC 1) and Switch Matrix 1B MUX D (ASIC 2) ---\r\r\r\r\r\r\r\r\r\r\r\r\r\r\r\r\r\r\r\r\r\r\r\r\r\r\r\r\r\r\r\r\r\r\r\r\r\r\r\r\r\r\r\r\r\r\r\r\r\r\r\r\r\r\r\r\r\r\r\r\r\r\r", "ExpectedValue"=""}, {"Test_Name"="1093. SelectAllMuxB \"2\" \"0\"", "Step_Type"="", "LowLimit"=0.0, "HighLimit"=0.0, "RValue"="", "RStatus"="", "RetVal"="0", "Units"="", "header1"="=== CCD overvoltage protection test ====", "header2"="--- Start Switch Matrix 1B MUX B (ASIC 1) and Switch Matrix 1B MUX D (ASIC 2) ---\r\r\r\r\r\r\r\r\r\r\r\r\r\r\r\r\r\r\r\r\r\r\r\r\r\r\r\r\r\r\r\r\r\r\r\r\r\r\r\r\r\r\r\r\r\r\r\r\r\r\r\r\r\r\r\r\r\r\r\r\r\r\r\r", "ExpectedValue"=""}, {"Test_Name"="1095. SelectMuxB \"1\" \"14\" \"1\"", "Step_Type"="", "LowLimit"=0.0, "HighLimit"=0.0, "RValue"="", "RStatus"="", "RetVal"="0", "Units"="", "header1"="=== CCD overvoltage protection test ====", "header2"="--- Start Switch Matrix 1B MUX B (ASIC 1) and Switch Matrix 1B MUX D (ASIC 2) ---\r\r\r\r\r\r\r\r\r\r\r\r\r\r\r\r\r\r\r\r\r\r\r\r\r\r\r\r\r\r\r\r\r\r\r\r\r\r\r\r\r\r\r\r\r\r\r\r\r\r\r\r\r\r\r\r\r\r\r\r\r\r\r\r\r", "ExpectedValue"=""}, {"Test_Name"="1096. SelectMuxB \"2\" \"14\" \"1\"", "Step_Type"="", "LowLimit"=0.0, "HighLimit"=0.0, "RValue"="", "RStatus"="", "RetVal"="0", "Units"="", "header1"="=== CCD overvoltage protection test ====", "header2"="--- Start Switch Matrix 1B MUX B (ASIC 1) and Switch Matrix 1B MUX D (ASIC 2) ---\r\r\r\r\r\r\r\r\r\r\r\r\r\r\r\r\r\r\r\r\r\r\r\r\r\r\r\r\r\r\r\r\r\r\r\r\r\r\r\r\r\r\r\r\r\r\r\r\r\r\r\r\r\r\r\r\r\r\r\r\r\r\r\r\r\r", "ExpectedValue"=""}, {"Test_Name"="1097. CheckCFAdc \"PD4\" \"2.2\" \"2.65\"", "Step_Type"="NumericLimitTest", "LowLimit"=2.2, "HighLimit"=2.65, "RValue"="2.453000068664551", "RStatus"="PASS", "RetVal"="0", "Units"="Volts", "header1"="=== CCD overvoltage protection test ====", "header2"="--- Start Switch Matrix 1B MUX B (ASIC 1) and Switch Matrix 1B MUX D (ASIC 2) ---\r\r\r\r\r\r\r\r\r\r\r\r\r\r\r\r\r\r\r\r\r\r\r\r\r\r\r\r\r\r\r\r\r\r\r\r\r\r\r\r\r\r\r\r\r\r\r\r\r\r\r\r\r\r\r\r\r\r\r\r\r\r\r\r\r\r\r", "ExpectedValue"=""}, {"Test_Name"="1098. SelectAllMuxB \"1\" \"0\"", "Step_Type"="", "LowLimit"=0.0, "HighLimit"=0.0, "RValue"="", "RStatus"="", "RetVal"="0", "Units"="", "header1"="=== CCD overvoltage protection test ====", "header2"="--- Start Switch Matrix 1B MUX B (ASIC 1) and Switch Matrix 1B MUX D (ASIC 2) ---\r\r\r\r\r\r\r\r\r\r\r\r\r\r\r\r\r\r\r\r\r\r\r\r\r\r\r\r\r\r\r\r\r\r\r\r\r\r\r\r\r\r\r\r\r\r\r\r\r\r\r\r\r\r\r\r\r\r\r\r\r\r\r\r\r\r\r\r", "ExpectedValue"=""}, {"Test_Name"="1099. SelectAllMuxB \"2\" \"0\"", "Step_Type"="", "LowLimit"=0.0, "HighLimit"=0.0, "RValue"="", "RStatus"="", "RetVal"="0", "Units"="", "header1"="=== CCD overvoltage protection test ====", "header2"="--- Start Switch Matrix 1B MUX B (ASIC 1) and Switch Matrix 1B MUX D (ASIC 2) ---\r\r\r\r\r\r\r\r\r\r\r\r\r\r\r\r\r\r\r\r\r\r\r\r\r\r\r\r\r\r\r\r\r\r\r\r\r\r\r\r\r\r\r\r\r\r\r\r\r\r\r\r\r\r\r\r\r\r\r\r\r\r\r\r\r\r\r\r\r", "ExpectedValue"=""}, {"Test_Name"="1101. SelectMuxB \"1\" \"15\" \"1\"", "Step_Type"="", "LowLimit"=0.0, "HighLimit"=0.0, "RValue"="", "RStatus"="", "RetVal"="0", "Units"="", "header1"="=== CCD overvoltage protection test ====", "header2"="--- Start Switch Matrix 1B MUX B (ASIC 1) and Switch Matrix 1B MUX D (ASIC 2) ---\r\r\r\r\r\r\r\r\r\r\r\r\r\r\r\r\r\r\r\r\r\r\r\r\r\r\r\r\r\r\r\r\r\r\r\r\r\r\r\r\r\r\r\r\r\r\r\r\r\r\r\r\r\r\r\r\r\r\r\r\r\r\r\r\r\r\r\r\r\r", "ExpectedValue"=""}, {"Test_Name"="1102. SelectMuxB \"2\" \"15\" \"1\"", "Step_Type"="", "LowLimit"=0.0, "HighLimit"=0.0, "RValue"="", "RStatus"="", "RetVal"="0", "Units"="", "header1"="=== CCD overvoltage protection test ====", "header2"="--- Start Switch Matrix 1B MUX B (ASIC 1) and Switch Matrix 1B MUX D (ASIC 2) ---\r\r\r\r\r\r\r\r\r\r\r\r\r\r\r\r\r\r\r\r\r\r\r\r\r\r\r\r\r\r\r\r\r\r\r\r\r\r\r\r\r\r\r\r\r\r\r\r\r\r\r\r\r\r\r\r\r\r\r\r\r\r\r\r\r\r\r\r\r\r\r", "ExpectedValue"=""}, {"Test_Name"="1103. CheckCFAdc \"PD4\" \"2.2\" \"2.65\"", "Step_Type"="NumericLimitTest", "LowLimit"=2.2, "HighLimit"=2.65, "RValue"="2.444000005722046", "RStatus"="PASS", "RetVal"="0", "Units"="Volts", "header1"="=== CCD overvoltage protection test ====", "header2"="--- Start Switch Matrix 1B MUX B (ASIC 1) and Switch Matrix 1B MUX D (ASIC 2) ---\r\r\r\r\r\r\r\r\r\r\r\r\r\r\r\r\r\r\r\r\r\r\r\r\r\r\r\r\r\r\r\r\r\r\r\r\r\r\r\r\r\r\r\r\r\r\r\r\r\r\r\r\r\r\r\r\r\r\r\r\r\r\r\r\r\r\r\r\r\r\r\r", "ExpectedValue"=""}, {"Test_Name"="1104. SelectAllMuxB \"1\" \"0\"", "Step_Type"="", "LowLimit"=0.0, "HighLimit"=0.0, "RValue"="", "RStatus"="", "RetVal"="0", "Units"="", "header1"="=== CCD overvoltage protection test ====", "header2"="--- Start Switch Matrix 1B MUX B (ASIC 1) and Switch Matrix 1B MUX D (ASIC 2) ---\r\r\r\r\r\r\r\r\r\r\r\r\r\r\r\r\r\r\r\r\r\r\r\r\r\r\r\r\r\r\r\r\r\r\r\r\r\r\r\r\r\r\r\r\r\r\r\r\r\r\r\r\r\r\r\r\r\r\r\r\r\r\r\r\r\r\r\r\r\r\r\r\r", "ExpectedValue"=""}, {"Test_Name"="1105. SelectAllMuxB \"2\" \"0\"", "Step_Type"="", "LowLimit"=0.0, "HighLimit"=0.0, "RValue"="", "RStatus"="", "RetVal"="0", "Units"="", "header1"="=== CCD overvoltage protection test ====", "header2"="--- Start Switch Matrix 1B MUX B (ASIC 1) and Switch Matrix 1B MUX D (ASIC 2) ---\r\r\r\r\r\r\r\r\r\r\r\r\r\r\r\r\r\r\r\r\r\r\r\r\r\r\r\r\r\r\r\r\r\r\r\r\r\r\r\r\r\r\r\r\r\r\r\r\r\r\r\r\r\r\r\r\r\r\r\r\r\r\r\r\r\r\r\r\r\r\r\r\r\r", "ExpectedValue"=""}, {"Test_Name"="1107. SetG15PullUp \"B\" \"0\"", "Step_Type"="", "LowLimit"=0.0, "HighLimit"=0.0, "RValue"="", "RStatus"="", "RetVal"="0", "Units"="", "header1"="=== CCD overvoltage protection test ====", "header2"="--- Start Switch Matrix 1B MUX B (ASIC 1) and Switch Matrix 1B MUX D (ASIC 2) ---\r\r\r\r\r\r\r\r\r\r\r\r\r\r\r\r\r\r\r\r\r\r\r\r\r\r\r\r\r\r\r\r\r\r\r\r\r\r\r\r\r\r\r\r\r\r\r\r\r\r\r\r\r\r\r\r\r\r\r\r\r\r\r\r\r\r\r\r\r\r\r\r\r\r\r", "ExpectedValue"=""}, {"Test_Name"="1108. SetG15PullUp \"D\" \"0\"", "Step_Type"="", "LowLimit"=0.0, "HighLimit"=0.0, "RValue"="", "RStatus"="", "RetVal"="0", "Units"="", "header1"="=== CCD overvoltage protection test ====", "header2"="--- Start Switch Matrix 1B MUX B (ASIC 1) and Switch Matrix 1B MUX D (ASIC 2) ---\r\r\r\r\r\r\r\r\r\r\r\r\r\r\r\r\r\r\r\r\r\r\r\r\r\r\r\r\r\r\r\r\r\r\r\r\r\r\r\r\r\r\r\r\r\r\r\r\r\r\r\r\r\r\r\r\r\r\r\r\r\r\r\r\r\r\r\r\r\r\r\r\r\r\r\r", "ExpectedValue"=""}, {"Test_Name"="1109. SetG15PullDown \"B\" \"0\"", "Step_Type"="", "LowLimit"=0.0, "HighLimit"=0.0, "RValue"="", "RStatus"="", "RetVal"="0", "Units"="", "header1"="=== CCD overvoltage protection test ====", "header2"="--- Start Switch Matrix 1B MUX B (ASIC 1) and Switch Matrix 1B MUX D (ASIC 2) ---\r\r\r\r\r\r\r\r\r\r\r\r\r\r\r\r\r\r\r\r\r\r\r\r\r\r\r\r\r\r\r\r\r\r\r\r\r\r\r\r\r\r\r\r\r\r\r\r\r\r\r\r\r\r\r\r\r\r\r\r\r\r\r\r\r\r\r\r\r\r\r\r\r\r\r\r\r", "ExpectedValue"=""}, {"Test_Name"="1110. SetG15PullDown \"D\" \"0\"", "Step_Type"="", "LowLimit"=0.0, "HighLimit"=0.0, "RValue"="", "RStatus"="", "RetVal"="0", "Units"="", "header1"="=== CCD overvoltage protection test ====", "header2"="--- Start Switch Matrix 1B MUX B (ASIC 1) and Switch Matrix 1B MUX D (ASIC 2) ---\r\r\r\r\r\r\r\r\r\r\r\r\r\r\r\r\r\r\r\r\r\r\r\r\r\r\r\r\r\r\r\r\r\r\r\r\r\r\r\r\r\r\r\r\r\r\r\r\r\r\r\r\r\r\r\r\r\r\r\r\r\r\r\r\r\r\r\r\r\r\r\r\r\r\r\r\r\r", "ExpectedValue"=""}, {"Test_Name"="1113.  --- USE SW 1 to Test Vcomm and also test MUX2 A B  Asic 2 ---", "Step_Type"="", "LowLimit"=0.0, "HighLimit"=0.0, "RValue"="", "RStatus"="", "RetVal"="", "Units"="", "header1"="=== CCD overvoltage protection test ====", "header2"="--- USE SW 1 to Test Vcomm and also test MUX2 A B  Asic 2 ---\r", "ExpectedValue"=""}, {"Test_Name"="1114. SetFpgaRegister \"89E\" \"40\"", "Step_Type"="", "LowLimit"=0.0, "HighLimit"=0.0, "RValue"="", "RStatus"="", "RetVal"="0", "Units"="", "header1"="=== CCD overvoltage protection test ====", "header2"="--- USE SW 1 to Test Vcomm and also test MUX2 A B  Asic 2 ---\r\r", "ExpectedValue"=""}, {"Test_Name"="1115. SetFpgaRegister \"959\" \"02\"", "Step_Type"="", "LowLimit"=0.0, "HighLimit"=0.0, "RValue"="", "RStatus"="", "RetVal"="0", "Units"="", "header1"="=== CCD overvoltage protection test ====", "header2"="--- USE SW 1 to Test Vcomm and also test MUX2 A B  Asic 2 ---\r\r\r", "ExpectedValue"=""}, {"Test_Name"="1116. SetAsicRegister \"2\" \"4\" \"30\"", "Step_Type"="", "LowLimit"=0.0, "HighLimit"=0.0, "RValue"="", "RStatus"="", "RetVal"="0", "Units"="", "header1"="=== CCD overvoltage protection test ====", "header2"="--- USE SW 1 to Test Vcomm and also test MUX2 A B  Asic 2 ---\r\r\r\r", "ExpectedValue"=""}, {"Test_Name"="1117. SelectMuxA \"2\" \"2\" \"1\"", "Step_Type"="", "LowLimit"=0.0, "HighLimit"=0.0, "RValue"="", "RStatus"="", "RetVal"="0", "Units"="", "header1"="=== CCD overvoltage protection test ====", "header2"="--- USE SW 1 to Test Vcomm and also test MUX2 A B  Asic 2 ---\r\r\r\r\r", "ExpectedValue"=""}, {"Test_Name"="1118. SelectMuxB \"2\" \"10\" \"1\"", "Step_Type"="", "LowLimit"=0.0, "HighLimit"=0.0, "RValue"="", "RStatus"="", "RetVal"="0", "Units"="", "header1"="=== CCD overvoltage protection test ====", "header2"="--- USE SW 1 to Test Vcomm and also test MUX2 A B  Asic 2 ---\r\r\r\r\r\r", "ExpectedValue"=""}, {"Test_Name"="1119. CheckCFAdc \"PD3\" \"-.15\" \".3\"", "Step_Type"="NumericLimitTest", "LowLimit"=-0.15, "HighLimit"=0.3, "RValue"="0.054999999701976776", "RStatus"="PASS", "RetVal"="0", "Units"="Volts", "header1"="=== CCD overvoltage protection test ====", "header2"="--- USE SW 1 to Test Vcomm and also test MUX2 A B  Asic 2 ---\r\r\r\r\r\r\r", "ExpectedValue"=""}, {"Test_Name"="1120. CheckCFAdc \"PD4\" \"7.2\" \"7.9\"", "Step_Type"="NumericLimitTest", "LowLimit"=7.2, "HighLimit"=7.9, "RValue"="7.611000061035156", "RStatus"="PASS", "RetVal"="0", "Units"="Volts", "header1"="=== CCD overvoltage protection test ====", "header2"="--- USE SW 1 to Test Vcomm and also test MUX2 A B  Asic 2 ---\r\r\r\r\r\r\r\r", "ExpectedValue"=""}, {"Test_Name"="1122. SetAsicRegister \"2\" \"4\" \"38\"", "Step_Type"="", "LowLimit"=0.0, "HighLimit"=0.0, "RValue"="", "RStatus"="", "RetVal"="0", "Units"="", "header1"="=== CCD overvoltage protection test ====", "header2"="--- USE SW 1 to Test Vcomm and also test MUX2 A B  Asic 2 ---\r\r\r\r\r\r\r\r\r", "ExpectedValue"=""}, {"Test_Name"="1123. CheckCFAdc \"PD3\" \"3.4\" \"3.8\"", "Step_Type"="NumericLimitTest", "LowLimit"=3.4, "HighLimit"=3.8, "RValue"="3.6670000553131104", "RStatus"="PASS", "RetVal"="0", "Units"="Volts", "header1"="=== CCD overvoltage protection test ====", "header2"="--- USE SW 1 to Test Vcomm and also test MUX2 A B  Asic 2 ---\r\r\r\r\r\r\r\r\r\r", "ExpectedValue"=""}, {"Test_Name"="1124. CheckCFAdc \"PD4\" \"7.2\" \"7.9\"", "Step_Type"="NumericLimitTest", "LowLimit"=7.2, "HighLimit"=7.9, "RValue"="7.619999885559082", "RStatus"="PASS", "RetVal"="0", "Units"="Volts", "header1"="=== CCD overvoltage protection test ====", "header2"="--- USE SW 1 to Test Vcomm and also test MUX2 A B  Asic 2 ---\r\r\r\r\r\r\r\r\r\r\r", "ExpectedValue"=""}, {"Test_Name"="1125. SelectAllMuxA \"2\" \"0\"", "Step_Type"="", "LowLimit"=0.0, "HighLimit"=0.0, "RValue"="", "RStatus"="", "RetVal"="0", "Units"="", "header1"="=== CCD overvoltage protection test ====", "header2"="--- USE SW 1 to Test Vcomm and also test MUX2 A B  Asic 2 ---\r\r\r\r\r\r\r\r\r\r\r\r", "ExpectedValue"=""}, {"Test_Name"="1126. SelectAllMuxB \"2\" \"0\"", "Step_Type"="", "LowLimit"=0.0, "HighLimit"=0.0, "RValue"="", "RStatus"="", "RetVal"="0", "Units"="", "header1"="=== CCD overvoltage protection test ====", "header2"="--- USE SW 1 to Test Vcomm and also test MUX2 A B  Asic 2 ---\r\r\r\r\r\r\r\r\r\r\r\r\r", "ExpectedValue"=""}, {"Test_Name"="1127. SetFpgaRegister \"89E\" \"00\"", "Step_Type"="", "LowLimit"=0.0, "HighLimit"=0.0, "RValue"="", "RStatus"="", "RetVal"="0", "Units"="", "header1"="=== CCD overvoltage protection test ====", "header2"="--- USE SW 1 to Test Vcomm and also test MUX2 A B  Asic 2 ---\r\r\r\r\r\r\r\r\r\r\r\r\r\r", "ExpectedValue"=""}, {"Test_Name"="1128. SetFpgaRegister \"959\" \"00\"", "Step_Type"="", "LowLimit"=0.0, "HighLimit"=0.0, "RValue"="", "RStatus"="", "RetVal"="0", "Units"="", "header1"="=== CCD overvoltage protection test ====", "header2"="--- USE SW 1 to Test Vcomm and also test MUX2 A B  Asic 2 ---\r\r\r\r\r\r\r\r\r\r\r\r\r\r\r", "ExpectedValue"=""}, {"Test_Name"="1129. SetAsicRegister \"2\" \"4\" \"00\"", "Step_Type"="", "LowLimit"=0.0, "HighLimit"=0.0, "RValue"="", "RStatus"="", "RetVal"="0", "Units"="", "header1"="=== CCD overvoltage protection test ====", "header2"="--- USE SW 1 to Test Vcomm and also test MUX2 A B  Asic 2 ---\r\r\r\r\r\r\r\r\r\r\r\r\r\r\r\r", "ExpectedValue"=""}, {"Test_Name"="1132. ---24V Detect---", "Step_Type"="", "LowLimit"=0.0, "HighLimit"=0.0, "RValue"="", "RStatus"="", "RetVal"="", "Units"="", "header1"="=== CCD overvoltage protection test ====", "header2"="---24V Detect---------------------------\r", "ExpectedValue"=""}, {"Test_Name"="1134. Apply_17V_to_VBAT.exe", "Step_Type"="", "LowLimit"=0.0, "HighLimit"=0.0, "RValue"="", "RStatus"="", "RetVal"="", "Units"="", "header1"="=== CCD overvoltage protection test ====", "header2"="---24V Detect---------------------------\r\r", "ExpectedValue"=""}, {"Test_Name"="1138. CheckFpgaRegister \"85A\" \"0\" \"0\"", "Step_Type"="StringValueTest", "LowLimit"=0.0, "HighLimit"=0.0, "RValue"="42", "RStatus"="PASS", "RetVal"="0", "Units"="", "header1"="=== CCD overvoltage protection test ====", "header2"="---24V Detect---------------------------\r\r\r", "ExpectedValue"=""}, {"Test_Name"="1140. Apply_19V_to_VBAT.exe", "Step_Type"="", "LowLimit"=0.0, "HighLimit"=0.0, "RValue"="", "RStatus"="", "RetVal"="", "Units"="", "header1"="=== CCD overvoltage protection test ====", "header2"="---24V Detect---------------------------\r\r\r\r", "ExpectedValue"=""}, {"Test_Name"="1143. CheckFpgaRegister \"85A\" \"0\" \"1\"", "Step_Type"="StringValueTest", "LowLimit"=0.0, "HighLimit"=0.0, "RValue"="43", "RStatus"="PASS", "RetVal"="0", "Units"="", "header1"="=== CCD overvoltage protection test ====", "header2"="---24V Detect---------------------------\r\r\r\r\r", "ExpectedValue"=""}, {"Test_Name"="1146. ---ID test connector 1 ---", "Step_Type"="", "LowLimit"=0.0, "HighLimit"=0.0, "RValue"="", "RStatus"="", "RetVal"="", "Units"="", "header1"="=== CCD overvoltage protection test ====", "header2"="---ID test connector 1 -----------------\r", "ExpectedValue"=""}, {"Test_Name"="1148. Set_J17Low-J18High.exe", "Step_Type"="", "LowLimit"=0.0, "HighLimit"=0.0, "RValue"="", "RStatus"="", "RetVal"="", "Units"="", "header1"="=== CCD overvoltage protection test ====", "header2"="---ID test connector 1 -----------------\r\r", "ExpectedValue"=""}, {"Test_Name"="1150. CheckFpgaRegister \"87A\" \"0\" \"1\"", "Step_Type"="StringValueTest", "LowLimit"=0.0, "HighLimit"=0.0, "RValue"="2", "RStatus"="FAIL", "RetVal"="0", "Units"="", "header1"="=== CCD overvoltage protection test ====", "header2"="---ID test connector 1 -----------------\r\r\r", "ExpectedValue"=""}, {"Test_Name"="1151. CheckFpgaRegister \"87A\" \"1\" \"0\"", "Step_Type"="StringValueTest", "LowLimit"=0.0, "HighLimit"=0.0, "RValue"="2", "RStatus"="FAIL", "RetVal"="0", "Units"="", "header1"="=== CCD overvoltage protection test ====", "header2"="---ID test connector 1 -----------------\r\r\r\r", "ExpectedValue"=""}, {"Test_Name"="1153. Set_J17High-J18Low.exe", "Step_Type"="", "LowLimit"=0.0, "HighLimit"=0.0, "RValue"="", "RStatus"="", "RetVal"="", "Units"="", "header1"="=== CCD overvoltage protection test ====", "header2"="---ID test connector 1 -----------------\r\r\r\r\r", "ExpectedValue"=""}, {"Test_Name"="1155. CheckFpgaRegister \"87A\" \"0\" \"0\"", "Step_Type"="StringValueTest", "LowLimit"=0.0, "HighLimit"=0.0, "RValue"="1", "RStatus"="FAIL", "RetVal"="0", "Units"="", "header1"="=== CCD overvoltage protection test ====", "header2"="---ID test connector 1 -----------------\r\r\r\r\r\r", "ExpectedValue"=""}, {"Test_Name"="1156. CheckFpgaRegister \"87A\" \"1\" \"1\"", "Step_Type"="StringValueTest", "LowLimit"=0.0, "HighLimit"=0.0, "RValue"="1", "RStatus"="FAIL", "RetVal"="0", "Units"="", "header1"="=== CCD overvoltage protection test ====", "header2"="---ID test connector 1 -----------------\r\r\r\r\r\r\r", "ExpectedValue"=""}, {"Test_Name"="1194.  --- Test for shorted pins ---", "Step_Type"="", "LowLimit"=0.0, "HighLimit"=0.0, "RValue"="", "RStatus"="", "RetVal"="", "Units"="", "header1"="=== CCD overvoltage protection test ====", "header2"="--- Test for shorted pins --------------\r", "ExpectedValue"=""}, {"Test_Name"="1197. SelectAllMuxA \"1\" \"0\"", "Step_Type"="", "LowLimit"=0.0, "HighLimit"=0.0, "RValue"="", "RStatus"="", "RetVal"="0", "Units"="", "header1"="=== CCD overvoltage protection test ====", "header2"="--- Test for shorted pins --------------\r\r", "ExpectedValue"=""}, {"Test_Name"="1198. SelectAllMuxB \"1\" \"0\"", "Step_Type"="", "LowLimit"=0.0, "HighLimit"=0.0, "RValue"="", "RStatus"="", "RetVal"="0", "Units"="", "header1"="=== CCD overvoltage protection test ====", "header2"="--- Test for shorted pins --------------\r\r\r", "ExpectedValue"=""}, {"Test_Name"="1199. SetG15PullUp \"A\" \"9\"", "Step_Type"="", "LowLimit"=0.0, "HighLimit"=0.0, "RValue"="", "RStatus"="", "RetVal"="0", "Units"="", "header1"="=== CCD overvoltage protection test ====", "header2"="--- Test for shorted pins --------------\r\r\r\r", "ExpectedValue"=""}, {"Test_Name"="1200. SetG15PullDown \"B\" \"4\"", "Step_Type"="", "LowLimit"=0.0, "HighLimit"=0.0, "RValue"="", "RStatus"="", "RetVal"="0", "Units"="", "header1"="=== CCD overvoltage protection test ====", "header2"="--- Test for shorted pins --------------\r\r\r\r\r", "ExpectedValue"=""}, {"Test_Name"="1202. SelectMuxA \"1\" \"1\" \"1\"", "Step_Type"="", "LowLimit"=0.0, "HighLimit"=0.0, "RValue"="", "RStatus"="", "RetVal"="0", "Units"="", "header1"="=== CCD overvoltage protection test ====", "header2"="--- Test for shorted pins --------------\r\r\r\r\r\r", "ExpectedValue"=""}, {"Test_Name"="1203. SelectMuxB \"1\" \"1\" \"1\"", "Step_Type"="", "LowLimit"=0.0, "HighLimit"=0.0, "RValue"="", "RStatus"="", "RetVal"="0", "Units"="", "header1"="=== CCD overvoltage protection test ====", "header2"="--- Test for shorted pins --------------\r\r\r\r\r\r\r", "ExpectedValue"=""}, {"Test_Name"="1204. CheckCFAdc \"PD1\" \"2.2\" \"2.65\"", "Step_Type"="NumericLimitTest", "LowLimit"=2.2, "HighLimit"=2.65, "RValue"="2.447999954223633", "RStatus"="PASS", "RetVal"="0", "Units"="Volts", "header1"="=== CCD overvoltage protection test ====", "header2"="--- Test for shorted pins --------------\r\r\r\r\r\r\r\r", "ExpectedValue"=""}, {"Test_Name"="1205. CheckCFAdc \"PD2\" \"2.2\" \"2.65\"", "Step_Type"="NumericLimitTest", "LowLimit"=2.2, "HighLimit"=2.65, "RValue"="2.4549999237060547", "RStatus"="PASS", "RetVal"="0", "Units"="Volts", "header1"="=== CCD overvoltage protection test ====", "header2"="--- Test for shorted pins --------------\r\r\r\r\r\r\r\r\r", "ExpectedValue"=""}, {"Test_Name"="1207. SelectAllMuxA \"1\" \"0\"", "Step_Type"="", "LowLimit"=0.0, "HighLimit"=0.0, "RValue"="", "RStatus"="", "RetVal"="0", "Units"="", "header1"="=== CCD overvoltage protection test ====", "header2"="--- Test for shorted pins --------------\r\r\r\r\r\r\r\r\r\r", "ExpectedValue"=""}, {"Test_Name"="1208. SelectAllMuxB \"1\" \"0\"", "Step_Type"="", "LowLimit"=0.0, "HighLimit"=0.0, "RValue"="", "RStatus"="", "RetVal"="0", "Units"="", "header1"="=== CCD overvoltage protection test ====", "header2"="--- Test for shorted pins --------------\r\r\r\r\r\r\r\r\r\r\r", "ExpectedValue"=""}, {"Test_Name"="1209. CheckCFAdc \"PD1\" \"4.5\" \"5.0\"", "Step_Type"="NumericLimitTest", "LowLimit"=4.5, "HighLimit"=5.0, "RValue"="4.775000095367432", "RStatus"="PASS", "RetVal"="0", "Units"="Volts", "header1"="=== CCD overvoltage protection test ====", "header2"="--- Test for shorted pins --------------\r\r\r\r\r\r\r\r\r\r\r\r", "ExpectedValue"=""}, {"Test_Name"="1210. CheckCFAdc \"PD2\" \"-.15\" \".3\"", "Step_Type"="NumericLimitTest", "LowLimit"=-0.15, "HighLimit"=0.3, "RValue"="0.017999999225139618", "RStatus"="PASS", "RetVal"="0", "Units"="Volts", "header1"="=== CCD overvoltage protection test ====", "header2"="--- Test for shorted pins --------------\r\r\r\r\r\r\r\r\r\r\r\r\r", "ExpectedValue"=""}, {"Test_Name"="1213. SelectMuxB \"1\" \"1\" \"1\"", "Step_Type"="", "LowLimit"=0.0, "HighLimit"=0.0, "RValue"="", "RStatus"="", "RetVal"="0", "Units"="", "header1"="=== CCD overvoltage protection test ====", "header2"="--- Test for shorted pins --------------\r\r\r\r\r\r\r\r\r\r\r\r\r\r", "ExpectedValue"=""}, {"Test_Name"="1214. SelectAllMuxA \"1\" \"1\"", "Step_Type"="", "LowLimit"=0.0, "HighLimit"=0.0, "RValue"="", "RStatus"="", "RetVal"="0", "Units"="", "header1"="=== CCD overvoltage protection test ====", "header2"="--- Test for shorted pins --------------\r\r\r\r\r\r\r\r\r\r\r\r\r\r\r", "ExpectedValue"=""}, {"Test_Name"="1215. SelectMuxA \"1\" \"1\" \"0\"", "Step_Type"="", "LowLimit"=0.0, "HighLimit"=0.0, "RValue"="", "RStatus"="", "RetVal"="0", "Units"="", "header1"="=== CCD overvoltage protection test ====", "header2"="--- Test for shorted pins --------------\r\r\r\r\r\r\r\r\r\r\r\r\r\r\r\r", "ExpectedValue"=""}, {"Test_Name"="1216. CheckCFAdc \"PD2\" \"-.15\" \".3\"", "Step_Type"="NumericLimitTest", "LowLimit"=-0.15, "HighLimit"=0.3, "RValue"="0.027000000700354576", "RStatus"="PASS", "RetVal"="0", "Units"="Volts", "header1"="=== CCD overvoltage protection test ====", "header2"="--- Test for shorted pins --------------\r\r\r\r\r\r\r\r\r\r\r\r\r\r\r\r\r", "ExpectedValue"=""}, {"Test_Name"="1217. SelectAllMuxA \"1\" \"0\"", "Step_Type"="", "LowLimit"=0.0, "HighLimit"=0.0, "RValue"="", "RStatus"="", "RetVal"="0", "Units"="", "header1"="=== CCD overvoltage protection test ====", "header2"="--- Test for shorted pins --------------\r\r\r\r\r\r\r\r\r\r\r\r\r\r\r\r\r\r", "ExpectedValue"=""}, {"Test_Name"="1218. SelectAllMuxB \"1\" \"0\"", "Step_Type"="", "LowLimit"=0.0, "HighLimit"=0.0, "RValue"="", "RStatus"="", "RetVal"="0", "Units"="", "header1"="=== CCD overvoltage protection test ====", "header2"="--- Test for shorted pins --------------\r\r\r\r\r\r\r\r\r\r\r\r\r\r\r\r\r\r\r", "ExpectedValue"=""}, {"Test_Name"="1221. SelectMuxB \"1\" \"2\" \"1\"", "Step_Type"="", "LowLimit"=0.0, "HighLimit"=0.0, "RValue"="", "RStatus"="", "RetVal"="0", "Units"="", "header1"="=== CCD overvoltage protection test ====", "header2"="--- Test for shorted pins --------------\r\r\r\r\r\r\r\r\r\r\r\r\r\r\r\r\r\r\r\r", "ExpectedValue"=""}, {"Test_Name"="1222. SelectAllMuxA \"1\" \"1\"", "Step_Type"="", "LowLimit"=0.0, "HighLimit"=0.0, "RValue"="", "RStatus"="", "RetVal"="0", "Units"="", "header1"="=== CCD overvoltage protection test ====", "header2"="--- Test for shorted pins --------------\r\r\r\r\r\r\r\r\r\r\r\r\r\r\r\r\r\r\r\r\r", "ExpectedValue"=""}, {"Test_Name"="1223. SelectMuxA \"1\" \"2\" \"0\"", "Step_Type"="", "LowLimit"=0.0, "HighLimit"=0.0, "RValue"="", "RStatus"="", "RetVal"="0", "Units"="", "header1"="=== CCD overvoltage protection test ====", "header2"="--- Test for shorted pins --------------\r\r\r\r\r\r\r\r\r\r\r\r\r\r\r\r\r\r\r\r\r\r", "ExpectedValue"=""}, {"Test_Name"="1224. CheckCFAdc \"PD2\" \"-.15\" \".3\"", "Step_Type"="NumericLimitTest", "LowLimit"=-0.15, "HighLimit"=0.3, "RValue"="0.035999998450279236", "RStatus"="PASS", "RetVal"="0", "Units"="Volts", "header1"="=== CCD overvoltage protection test ====", "header2"="--- Test for shorted pins --------------\r\r\r\r\r\r\r\r\r\r\r\r\r\r\r\r\r\r\r\r\r\r\r", "ExpectedValue"=""}, {"Test_Name"="1225. SelectAllMuxA \"1\" \"0\"", "Step_Type"="", "LowLimit"=0.0, "HighLimit"=0.0, "RValue"="", "RStatus"="", "RetVal"="0", "Units"="", "header1"="=== CCD overvoltage protection test ====", "header2"="--- Test for shorted pins --------------\r\r\r\r\r\r\r\r\r\r\r\r\r\r\r\r\r\r\r\r\r\r\r\r", "ExpectedValue"=""}, {"Test_Name"="1226. SelectAllMuxB \"1\" \"0\"", "Step_Type"="", "LowLimit"=0.0, "HighLimit"=0.0, "RValue"="", "RStatus"="", "RetVal"="0", "Units"="", "header1"="=== CCD overvoltage protection test ====", "header2"="--- Test for shorted pins --------------\r\r\r\r\r\r\r\r\r\r\r\r\r\r\r\r\r\r\r\r\r\r\r\r\r", "ExpectedValue"=""}, {"Test_Name"="1229. SelectMuxB \"1\" \"3\" \"1\"", "Step_Type"="", "LowLimit"=0.0, "HighLimit"=0.0, "RValue"="", "RStatus"="", "RetVal"="0", "Units"="", "header1"="=== CCD overvoltage protection test ====", "header2"="--- Test for shorted pins --------------\r\r\r\r\r\r\r\r\r\r\r\r\r\r\r\r\r\r\r\r\r\r\r\r\r\r", "ExpectedValue"=""}, {"Test_Name"="1230. SelectAllMuxA \"1\" \"1\"", "Step_Type"="", "LowLimit"=0.0, "HighLimit"=0.0, "RValue"="", "RStatus"="", "RetVal"="0", "Units"="", "header1"="=== CCD overvoltage protection test ====", "header2"="--- Test for shorted pins --------------\r\r\r\r\r\r\r\r\r\r\r\r\r\r\r\r\r\r\r\r\r\r\r\r\r\r\r", "ExpectedValue"=""}, {"Test_Name"="1231. SelectMuxA \"1\" \"3\" \"0\"", "Step_Type"="", "LowLimit"=0.0, "HighLimit"=0.0, "RValue"="", "RStatus"="", "RetVal"="0", "Units"="", "header1"="=== CCD overvoltage protection test ====", "header2"="--- Test for shorted pins --------------\r\r\r\r\r\r\r\r\r\r\r\r\r\r\r\r\r\r\r\r\r\r\r\r\r\r\r\r", "ExpectedValue"=""}, {"Test_Name"="1232. CheckCFAdc \"PD2\" \"-.15\" \".3\"", "Step_Type"="NumericLimitTest", "LowLimit"=-0.15, "HighLimit"=0.3, "RValue"="0.035999998450279236", "RStatus"="PASS", "RetVal"="0", "Units"="Volts", "header1"="=== CCD overvoltage protection test ====", "header2"="--- Test for shorted pins --------------\r\r\r\r\r\r\r\r\r\r\r\r\r\r\r\r\r\r\r\r\r\r\r\r\r\r\r\r\r", "ExpectedValue"=""}, {"Test_Name"="1233. SelectAllMuxA \"1\" \"0\"", "Step_Type"="", "LowLimit"=0.0, "HighLimit"=0.0, "RValue"="", "RStatus"="", "RetVal"="0", "Units"="", "header1"="=== CCD overvoltage protection test ====", "header2"="--- Test for shorted pins --------------\r\r\r\r\r\r\r\r\r\r\r\r\r\r\r\r\r\r\r\r\r\r\r\r\r\r\r\r\r\r", "ExpectedValue"=""}, {"Test_Name"="1234. SelectAllMuxB \"1\" \"0\"", "Step_Type"="", "LowLimit"=0.0, "HighLimit"=0.0, "RValue"="", "RStatus"="", "RetVal"="0", "Units"="", "header1"="=== CCD overvoltage protection test ====", "header2"="--- Test for shorted pins --------------\r\r\r\r\r\r\r\r\r\r\r\r\r\r\r\r\r\r\r\r\r\r\r\r\r\r\r\r\r\r\r", "ExpectedValue"=""}, {"Test_Name"="1237. SelectMuxB \"1\" \"6\" \"1\"", "Step_Type"="", "LowLimit"=0.0, "HighLimit"=0.0, "RValue"="", "RStatus"="", "RetVal"="0", "Units"="", "header1"="=== CCD overvoltage protection test ====", "header2"="--- Test for shorted pins --------------\r\r\r\r\r\r\r\r\r\r\r\r\r\r\r\r\r\r\r\r\r\r\r\r\r\r\r\r\r\r\r\r", "ExpectedValue"=""}, {"Test_Name"="1238. SelectAllMuxA \"1\" \"1\"", "Step_Type"="", "LowLimit"=0.0, "HighLimit"=0.0, "RValue"="", "RStatus"="", "RetVal"="0", "Units"="", "header1"="=== CCD overvoltage protection test ====", "header2"="--- Test for shorted pins --------------\r\r\r\r\r\r\r\r\r\r\r\r\r\r\r\r\r\r\r\r\r\r\r\r\r\r\r\r\r\r\r\r\r", "ExpectedValue"=""}, {"Test_Name"="1239. SelectMuxA \"1\" \"6\" \"0\"", "Step_Type"="", "LowLimit"=0.0, "HighLimit"=0.0, "RValue"="", "RStatus"="", "RetVal"="0", "Units"="", "header1"="=== CCD overvoltage protection test ====", "header2"="--- Test for shorted pins --------------\r\r\r\r\r\r\r\r\r\r\r\r\r\r\r\r\r\r\r\r\r\r\r\r\r\r\r\r\r\r\r\r\r\r", "ExpectedValue"=""}, {"Test_Name"="1240. CheckCFAdc \"PD2\" \"-.15\" \".3\"", "Step_Type"="NumericLimitTest", "LowLimit"=-0.15, "HighLimit"=0.3, "RValue"="0.027000000700354576", "RStatus"="PASS", "RetVal"="0", "Units"="Volts", "header1"="=== CCD overvoltage protection test ====", "header2"="--- Test for shorted pins --------------\r\r\r\r\r\r\r\r\r\r\r\r\r\r\r\r\r\r\r\r\r\r\r\r\r\r\r\r\r\r\r\r\r\r\r", "ExpectedValue"=""}, {"Test_Name"="1241. SelectAllMuxA \"1\" \"0\"", "Step_Type"="", "LowLimit"=0.0, "HighLimit"=0.0, "RValue"="", "RStatus"="", "RetVal"="0", "Units"="", "header1"="=== CCD overvoltage protection test ====", "header2"="--- Test for shorted pins --------------\r\r\r\r\r\r\r\r\r\r\r\r\r\r\r\r\r\r\r\r\r\r\r\r\r\r\r\r\r\r\r\r\r\r\r\r", "ExpectedValue"=""}, {"Test_Name"="1242. SelectAllMuxB \"1\" \"0\"", "Step_Type"="", "LowLimit"=0.0, "HighLimit"=0.0, "RValue"="", "RStatus"="", "RetVal"="0", "Units"="", "header1"="=== CCD overvoltage protection test ====", "header2"="--- Test for shorted pins --------------\r\r\r\r\r\r\r\r\r\r\r\r\r\r\r\r\r\r\r\r\r\r\r\r\r\r\r\r\r\r\r\r\r\r\r\r\r", "ExpectedValue"=""}, {"Test_Name"="1245. SelectMuxB \"1\" \"7\" \"1\"", "Step_Type"="", "LowLimit"=0.0, "HighLimit"=0.0, "RValue"="", "RStatus"="", "RetVal"="0", "Units"="", "header1"="=== CCD overvoltage protection test ====", "header2"="--- Test for shorted pins --------------\r\r\r\r\r\r\r\r\r\r\r\r\r\r\r\r\r\r\r\r\r\r\r\r\r\r\r\r\r\r\r\r\r\r\r\r\r\r", "ExpectedValue"=""}, {"Test_Name"="1246. SelectAllMuxA \"1\" \"1\"", "Step_Type"="", "LowLimit"=0.0, "HighLimit"=0.0, "RValue"="", "RStatus"="", "RetVal"="0", "Units"="", "header1"="=== CCD overvoltage protection test ====", "header2"="--- Test for shorted pins --------------\r\r\r\r\r\r\r\r\r\r\r\r\r\r\r\r\r\r\r\r\r\r\r\r\r\r\r\r\r\r\r\r\r\r\r\r\r\r\r", "ExpectedValue"=""}, {"Test_Name"="1247. SelectMuxA \"1\" \"7\" \"0\"", "Step_Type"="", "LowLimit"=0.0, "HighLimit"=0.0, "RValue"="", "RStatus"="", "RetVal"="0", "Units"="", "header1"="=== CCD overvoltage protection test ====", "header2"="--- Test for shorted pins --------------\r\r\r\r\r\r\r\r\r\r\r\r\r\r\r\r\r\r\r\r\r\r\r\r\r\r\r\r\r\r\r\r\r\r\r\r\r\r\r\r", "ExpectedValue"=""}, {"Test_Name"="1248. CheckCFAdc \"PD2\" \"-.15\" \".3\"", "Step_Type"="NumericLimitTest", "LowLimit"=-0.15, "HighLimit"=0.3, "RValue"="0.035999998450279236", "RStatus"="PASS", "RetVal"="0", "Units"="Volts", "header1"="=== CCD overvoltage protection test ====", "header2"="--- Test for shorted pins --------------\r\r\r\r\r\r\r\r\r\r\r\r\r\r\r\r\r\r\r\r\r\r\r\r\r\r\r\r\r\r\r\r\r\r\r\r\r\r\r\r\r", "ExpectedValue"=""}, {"Test_Name"="1249. SelectAllMuxA \"1\" \"0\"", "Step_Type"="", "LowLimit"=0.0, "HighLimit"=0.0, "RValue"="", "RStatus"="", "RetVal"="0", "Units"="", "header1"="=== CCD overvoltage protection test ====", "header2"="--- Test for shorted pins --------------\r\r\r\r\r\r\r\r\r\r\r\r\r\r\r\r\r\r\r\r\r\r\r\r\r\r\r\r\r\r\r\r\r\r\r\r\r\r\r\r\r\r", "ExpectedValue"=""}, {"Test_Name"="1250. SelectAllMuxB \"1\" \"0\"", "Step_Type"="", "LowLimit"=0.0, "HighLimit"=0.0, "RValue"="", "RStatus"="", "RetVal"="0", "Units"="", "header1"="=== CCD overvoltage protection test ====", "header2"="--- Test for shorted pins --------------\r\r\r\r\r\r\r\r\r\r\r\r\r\r\r\r\r\r\r\r\r\r\r\r\r\r\r\r\r\r\r\r\r\r\r\r\r\r\r\r\r\r\r", "ExpectedValue"=""}, {"Test_Name"="1253. SelectMuxB \"1\" \"8\" \"1\"", "Step_Type"="", "LowLimit"=0.0, "HighLimit"=0.0, "RValue"="", "RStatus"="", "RetVal"="0", "Units"="", "header1"="=== CCD overvoltage protection test ====", "header2"="--- Test for shorted pins --------------\r\r\r\r\r\r\r\r\r\r\r\r\r\r\r\r\r\r\r\r\r\r\r\r\r\r\r\r\r\r\r\r\r\r\r\r\r\r\r\r\r\r\r\r", "ExpectedValue"=""}, {"Test_Name"="1254. SelectAllMuxA \"1\" \"1\"", "Step_Type"="", "LowLimit"=0.0, "HighLimit"=0.0, "RValue"="", "RStatus"="", "RetVal"="0", "Units"="", "header1"="=== CCD overvoltage protection test ====", "header2"="--- Test for shorted pins --------------\r\r\r\r\r\r\r\r\r\r\r\r\r\r\r\r\r\r\r\r\r\r\r\r\r\r\r\r\r\r\r\r\r\r\r\r\r\r\r\r\r\r\r\r\r", "ExpectedValue"=""}, {"Test_Name"="1255. SelectMuxA \"1\" \"8\" \"0\"", "Step_Type"="", "LowLimit"=0.0, "HighLimit"=0.0, "RValue"="", "RStatus"="", "RetVal"="0", "Units"="", "header1"="=== CCD overvoltage protection test ====", "header2"="--- Test for shorted pins --------------\r\r\r\r\r\r\r\r\r\r\r\r\r\r\r\r\r\r\r\r\r\r\r\r\r\r\r\r\r\r\r\r\r\r\r\r\r\r\r\r\r\r\r\r\r\r", "ExpectedValue"=""}, {"Test_Name"="1256. CheckCFAdc \"PD2\" \"-.15\" \".3\"", "Step_Type"="NumericLimitTest", "LowLimit"=-0.15, "HighLimit"=0.3, "RValue"="0.035999998450279236", "RStatus"="PASS", "RetVal"="0", "Units"="Volts", "header1"="=== CCD overvoltage protection test ====", "header2"="--- Test for shorted pins --------------\r\r\r\r\r\r\r\r\r\r\r\r\r\r\r\r\r\r\r\r\r\r\r\r\r\r\r\r\r\r\r\r\r\r\r\r\r\r\r\r\r\r\r\r\r\r\r", "ExpectedValue"=""}, {"Test_Name"="1257. SelectAllMuxA \"1\" \"0\"", "Step_Type"="", "LowLimit"=0.0, "HighLimit"=0.0, "RValue"="", "RStatus"="", "RetVal"="0", "Units"="", "header1"="=== CCD overvoltage protection test ====", "header2"="--- Test for shorted pins --------------\r\r\r\r\r\r\r\r\r\r\r\r\r\r\r\r\r\r\r\r\r\r\r\r\r\r\r\r\r\r\r\r\r\r\r\r\r\r\r\r\r\r\r\r\r\r\r\r", "ExpectedValue"=""}, {"Test_Name"="1258. SelectAllMuxB \"1\" \"0\"", "Step_Type"="", "LowLimit"=0.0, "HighLimit"=0.0, "RValue"="", "RStatus"="", "RetVal"="0", "Units"="", "header1"="=== CCD overvoltage protection test ====", "header2"="--- Test for shorted pins --------------\r\r\r\r\r\r\r\r\r\r\r\r\r\r\r\r\r\r\r\r\r\r\r\r\r\r\r\r\r\r\r\r\r\r\r\r\r\r\r\r\r\r\r\r\r\r\r\r\r", "ExpectedValue"=""}, {"Test_Name"="1261. SelectMuxB \"1\" \"9\" \"1\"", "Step_Type"="", "LowLimit"=0.0, "HighLimit"=0.0, "RValue"="", "RStatus"="", "RetVal"="0", "Units"="", "header1"="=== CCD overvoltage protection test ====", "header2"="--- Test for shorted pins --------------\r\r\r\r\r\r\r\r\r\r\r\r\r\r\r\r\r\r\r\r\r\r\r\r\r\r\r\r\r\r\r\r\r\r\r\r\r\r\r\r\r\r\r\r\r\r\r\r\r\r", "ExpectedValue"=""}, {"Test_Name"="1262. SelectAllMuxA \"1\" \"1\"", "Step_Type"="", "LowLimit"=0.0, "HighLimit"=0.0, "RValue"="", "RStatus"="", "RetVal"="0", "Units"="", "header1"="=== CCD overvoltage protection test ====", "header2"="--- Test for shorted pins --------------\r\r\r\r\r\r\r\r\r\r\r\r\r\r\r\r\r\r\r\r\r\r\r\r\r\r\r\r\r\r\r\r\r\r\r\r\r\r\r\r\r\r\r\r\r\r\r\r\r\r\r", "ExpectedValue"=""}, {"Test_Name"="1263. SelectMuxA \"1\" \"9\" \"0\"", "Step_Type"="", "LowLimit"=0.0, "HighLimit"=0.0, "RValue"="", "RStatus"="", "RetVal"="0", "Units"="", "header1"="=== CCD overvoltage protection test ====", "header2"="--- Test for shorted pins --------------\r\r\r\r\r\r\r\r\r\r\r\r\r\r\r\r\r\r\r\r\r\r\r\r\r\r\r\r\r\r\r\r\r\r\r\r\r\r\r\r\r\r\r\r\r\r\r\r\r\r\r\r", "ExpectedValue"=""}, {"Test_Name"="1264. CheckCFAdc \"PD2\" \"-.15\" \".3\"", "Step_Type"="NumericLimitTest", "LowLimit"=-0.15, "HighLimit"=0.3, "RValue"="0.035999998450279236", "RStatus"="PASS", "RetVal"="0", "Units"="Volts", "header1"="=== CCD overvoltage protection test ====", "header2"="--- Test for shorted pins --------------\r\r\r\r\r\r\r\r\r\r\r\r\r\r\r\r\r\r\r\r\r\r\r\r\r\r\r\r\r\r\r\r\r\r\r\r\r\r\r\r\r\r\r\r\r\r\r\r\r\r\r\r\r", "ExpectedValue"=""}, {"Test_Name"="1265. SelectAllMuxA \"1\" \"0\"", "Step_Type"="", "LowLimit"=0.0, "HighLimit"=0.0, "RValue"="", "RStatus"="", "RetVal"="0", "Units"="", "header1"="=== CCD overvoltage protection test ====", "header2"="--- Test for shorted pins --------------\r\r\r\r\r\r\r\r\r\r\r\r\r\r\r\r\r\r\r\r\r\r\r\r\r\r\r\r\r\r\r\r\r\r\r\r\r\r\r\r\r\r\r\r\r\r\r\r\r\r\r\r\r\r", "ExpectedValue"=""}, {"Test_Name"="1266. SelectAllMuxB \"1\" \"0\"", "Step_Type"="", "LowLimit"=0.0, "HighLimit"=0.0, "RValue"="", "RStatus"="", "RetVal"="0", "Units"="", "header1"="=== CCD overvoltage protection test ====", "header2"="--- Test for shorted pins --------------\r\r\r\r\r\r\r\r\r\r\r\r\r\r\r\r\r\r\r\r\r\r\r\r\r\r\r\r\r\r\r\r\r\r\r\r\r\r\r\r\r\r\r\r\r\r\r\r\r\r\r\r\r\r\r", "ExpectedValue"=""}, {"Test_Name"="1269. SelectMuxB \"1\" \"10\" \"1\"", "Step_Type"="", "LowLimit"=0.0, "HighLimit"=0.0, "RValue"="", "RStatus"="", "RetVal"="0", "Units"="", "header1"="=== CCD overvoltage protection test ====", "header2"="--- Test for shorted pins --------------\r\r\r\r\r\r\r\r\r\r\r\r\r\r\r\r\r\r\r\r\r\r\r\r\r\r\r\r\r\r\r\r\r\r\r\r\r\r\r\r\r\r\r\r\r\r\r\r\r\r\r\r\r\r\r\r", "ExpectedValue"=""}, {"Test_Name"="1270. SelectAllMuxA \"1\" \"1\"", "Step_Type"="", "LowLimit"=0.0, "HighLimit"=0.0, "RValue"="", "RStatus"="", "RetVal"="0", "Units"="", "header1"="=== CCD overvoltage protection test ====", "header2"="--- Test for shorted pins --------------\r\r\r\r\r\r\r\r\r\r\r\r\r\r\r\r\r\r\r\r\r\r\r\r\r\r\r\r\r\r\r\r\r\r\r\r\r\r\r\r\r\r\r\r\r\r\r\r\r\r\r\r\r\r\r\r\r", "ExpectedValue"=""}, {"Test_Name"="1271. SelectMuxA \"1\" \"10\" \"0\"", "Step_Type"="", "LowLimit"=0.0, "HighLimit"=0.0, "RValue"="", "RStatus"="", "RetVal"="0", "Units"="", "header1"="=== CCD overvoltage protection test ====", "header2"="--- Test for shorted pins --------------\r\r\r\r\r\r\r\r\r\r\r\r\r\r\r\r\r\r\r\r\r\r\r\r\r\r\r\r\r\r\r\r\r\r\r\r\r\r\r\r\r\r\r\r\r\r\r\r\r\r\r\r\r\r\r\r\r\r", "ExpectedValue"=""}, {"Test_Name"="1272. CheckCFAdc \"PD2\" \"-.15\" \".3\"", "Step_Type"="NumericLimitTest", "LowLimit"=-0.15, "HighLimit"=0.3, "RValue"="0.035999998450279236", "RStatus"="PASS", "RetVal"="0", "Units"="Volts", "header1"="=== CCD overvoltage protection test ====", "header2"="--- Test for shorted pins --------------\r\r\r\r\r\r\r\r\r\r\r\r\r\r\r\r\r\r\r\r\r\r\r\r\r\r\r\r\r\r\r\r\r\r\r\r\r\r\r\r\r\r\r\r\r\r\r\r\r\r\r\r\r\r\r\r\r\r\r", "ExpectedValue"=""}, {"Test_Name"="1273. SelectAllMuxA \"1\" \"0\"", "Step_Type"="", "LowLimit"=0.0, "HighLimit"=0.0, "RValue"="", "RStatus"="", "RetVal"="0", "Units"="", "header1"="=== CCD overvoltage protection test ====", "header2"="--- Test for shorted pins --------------\r\r\r\r\r\r\r\r\r\r\r\r\r\r\r\r\r\r\r\r\r\r\r\r\r\r\r\r\r\r\r\r\r\r\r\r\r\r\r\r\r\r\r\r\r\r\r\r\r\r\r\r\r\r\r\r\r\r\r\r", "ExpectedValue"=""}, {"Test_Name"="1274. SelectAllMuxB \"1\" \"0\"", "Step_Type"="", "LowLimit"=0.0, "HighLimit"=0.0, "RValue"="", "RStatus"="", "RetVal"="0", "Units"="", "header1"="=== CCD overvoltage protection test ====", "header2"="--- Test for shorted pins --------------\r\r\r\r\r\r\r\r\r\r\r\r\r\r\r\r\r\r\r\r\r\r\r\r\r\r\r\r\r\r\r\r\r\r\r\r\r\r\r\r\r\r\r\r\r\r\r\r\r\r\r\r\r\r\r\r\r\r\r\r\r", "ExpectedValue"=""}, {"Test_Name"="1277. SelectMuxB \"1\" \"11\" \"1\"", "Step_Type"="", "LowLimit"=0.0, "HighLimit"=0.0, "RValue"="", "RStatus"="", "RetVal"="0", "Units"="", "header1"="=== CCD overvoltage protection test ====", "header2"="--- Test for shorted pins --------------\r\r\r\r\r\r\r\r\r\r\r\r\r\r\r\r\r\r\r\r\r\r\r\r\r\r\r\r\r\r\r\r\r\r\r\r\r\r\r\r\r\r\r\r\r\r\r\r\r\r\r\r\r\r\r\r\r\r\r\r\r\r", "ExpectedValue"=""}, {"Test_Name"="1278. SelectAllMuxA \"1\" \"1\"", "Step_Type"="", "LowLimit"=0.0, "HighLimit"=0.0, "RValue"="", "RStatus"="", "RetVal"="0", "Units"="", "header1"="=== CCD overvoltage protection test ====", "header2"="--- Test for shorted pins --------------\r\r\r\r\r\r\r\r\r\r\r\r\r\r\r\r\r\r\r\r\r\r\r\r\r\r\r\r\r\r\r\r\r\r\r\r\r\r\r\r\r\r\r\r\r\r\r\r\r\r\r\r\r\r\r\r\r\r\r\r\r\r\r", "ExpectedValue"=""}, {"Test_Name"="1279. SelectMuxA \"1\" \"11\" \"0\"", "Step_Type"="", "LowLimit"=0.0, "HighLimit"=0.0, "RValue"="", "RStatus"="", "RetVal"="0", "Units"="", "header1"="=== CCD overvoltage protection test ====", "header2"="--- Test for shorted pins --------------\r\r\r\r\r\r\r\r\r\r\r\r\r\r\r\r\r\r\r\r\r\r\r\r\r\r\r\r\r\r\r\r\r\r\r\r\r\r\r\r\r\r\r\r\r\r\r\r\r\r\r\r\r\r\r\r\r\r\r\r\r\r\r\r", "ExpectedValue"=""}, {"Test_Name"="1280. CheckCFAdc \"PD2\" \"-.15\" \".3\"", "Step_Type"="NumericLimitTest", "LowLimit"=-0.15, "HighLimit"=0.3, "RValue"="0.035999998450279236", "RStatus"="PASS", "RetVal"="0", "Units"="Volts", "header1"="=== CCD overvoltage protection test ====", "header2"="--- Test for shorted pins --------------\r\r\r\r\r\r\r\r\r\r\r\r\r\r\r\r\r\r\r\r\r\r\r\r\r\r\r\r\r\r\r\r\r\r\r\r\r\r\r\r\r\r\r\r\r\r\r\r\r\r\r\r\r\r\r\r\r\r\r\r\r\r\r\r\r", "ExpectedValue"=""}, {"Test_Name"="1281. SelectAllMuxA \"1\" \"0\"", "Step_Type"="", "LowLimit"=0.0, "HighLimit"=0.0, "RValue"="", "RStatus"="", "RetVal"="0", "Units"="", "header1"="=== CCD overvoltage protection test ====", "header2"="--- Test for shorted pins --------------\r\r\r\r\r\r\r\r\r\r\r\r\r\r\r\r\r\r\r\r\r\r\r\r\r\r\r\r\r\r\r\r\r\r\r\r\r\r\r\r\r\r\r\r\r\r\r\r\r\r\r\r\r\r\r\r\r\r\r\r\r\r\r\r\r\r", "ExpectedValue"=""}, {"Test_Name"="1282. SelectAllMuxB \"1\" \"0\"", "Step_Type"="", "LowLimit"=0.0, "HighLimit"=0.0, "RValue"="", "RStatus"="", "RetVal"="0", "Units"="", "header1"="=== CCD overvoltage protection test ====", "header2"="--- Test for shorted pins --------------\r\r\r\r\r\r\r\r\r\r\r\r\r\r\r\r\r\r\r\r\r\r\r\r\r\r\r\r\r\r\r\r\r\r\r\r\r\r\r\r\r\r\r\r\r\r\r\r\r\r\r\r\r\r\r\r\r\r\r\r\r\r\r\r\r\r\r", "ExpectedValue"=""}, {"Test_Name"="1285. SelectMuxB \"1\" \"12\" \"1\"", "Step_Type"="", "LowLimit"=0.0, "HighLimit"=0.0, "RValue"="", "RStatus"="", "RetVal"="0", "Units"="", "header1"="=== CCD overvoltage protection test ====", "header2"="--- Test for shorted pins --------------\r\r\r\r\r\r\r\r\r\r\r\r\r\r\r\r\r\r\r\r\r\r\r\r\r\r\r\r\r\r\r\r\r\r\r\r\r\r\r\r\r\r\r\r\r\r\r\r\r\r\r\r\r\r\r\r\r\r\r\r\r\r\r\r\r\r\r\r", "ExpectedValue"=""}, {"Test_Name"="1286. SelectAllMuxA \"1\" \"1\"", "Step_Type"="", "LowLimit"=0.0, "HighLimit"=0.0, "RValue"="", "RStatus"="", "RetVal"="0", "Units"="", "header1"="=== CCD overvoltage protection test ====", "header2"="--- Test for shorted pins --------------\r\r\r\r\r\r\r\r\r\r\r\r\r\r\r\r\r\r\r\r\r\r\r\r\r\r\r\r\r\r\r\r\r\r\r\r\r\r\r\r\r\r\r\r\r\r\r\r\r\r\r\r\r\r\r\r\r\r\r\r\r\r\r\r\r\r\r\r\r", "ExpectedValue"=""}, {"Test_Name"="1287. SelectMuxA \"1\" \"12\" \"0\"", "Step_Type"="", "LowLimit"=0.0, "HighLimit"=0.0, "RValue"="", "RStatus"="", "RetVal"="0", "Units"="", "header1"="=== CCD overvoltage protection test ====", "header2"="--- Test for shorted pins --------------\r\r\r\r\r\r\r\r\r\r\r\r\r\r\r\r\r\r\r\r\r\r\r\r\r\r\r\r\r\r\r\r\r\r\r\r\r\r\r\r\r\r\r\r\r\r\r\r\r\r\r\r\r\r\r\r\r\r\r\r\r\r\r\r\r\r\r\r\r\r", "ExpectedValue"=""}, {"Test_Name"="1288. CheckCFAdc \"PD2\" \"-.15\" \".3\"", "Step_Type"="NumericLimitTest", "LowLimit"=-0.15, "HighLimit"=0.3, "RValue"="0.035999998450279236", "RStatus"="PASS", "RetVal"="0", "Units"="Volts", "header1"="=== CCD overvoltage protection test ====", "header2"="--- Test for shorted pins --------------\r\r\r\r\r\r\r\r\r\r\r\r\r\r\r\r\r\r\r\r\r\r\r\r\r\r\r\r\r\r\r\r\r\r\r\r\r\r\r\r\r\r\r\r\r\r\r\r\r\r\r\r\r\r\r\r\r\r\r\r\r\r\r\r\r\r\r\r\r\r\r", "ExpectedValue"=""}, {"Test_Name"="1289. SelectAllMuxA \"1\" \"0\"", "Step_Type"="", "LowLimit"=0.0, "HighLimit"=0.0, "RValue"="", "RStatus"="", "RetVal"="0", "Units"="", "header1"="=== CCD overvoltage protection test ====", "header2"="--- Test for shorted pins --------------\r\r\r\r\r\r\r\r\r\r\r\r\r\r\r\r\r\r\r\r\r\r\r\r\r\r\r\r\r\r\r\r\r\r\r\r\r\r\r\r\r\r\r\r\r\r\r\r\r\r\r\r\r\r\r\r\r\r\r\r\r\r\r\r\r\r\r\r\r\r\r\r", "ExpectedValue"=""}, {"Test_Name"="1290. SelectAllMuxB \"1\" \"0\"", "Step_Type"="", "LowLimit"=0.0, "HighLimit"=0.0, "RValue"="", "RStatus"="", "RetVal"="0", "Units"="", "header1"="=== CCD overvoltage protection test ====", "header2"="--- Test for shorted pins --------------\r\r\r\r\r\r\r\r\r\r\r\r\r\r\r\r\r\r\r\r\r\r\r\r\r\r\r\r\r\r\r\r\r\r\r\r\r\r\r\r\r\r\r\r\r\r\r\r\r\r\r\r\r\r\r\r\r\r\r\r\r\r\r\r\r\r\r\r\r\r\r\r\r", "ExpectedValue"=""}, {"Test_Name"="1293. SelectMuxB \"1\" \"13\" \"1\"", "Step_Type"="", "LowLimit"=0.0, "HighLimit"=0.0, "RValue"="", "RStatus"="", "RetVal"="0", "Units"="", "header1"="=== CCD overvoltage protection test ====", "header2"="--- Test for shorted pins --------------\r\r\r\r\r\r\r\r\r\r\r\r\r\r\r\r\r\r\r\r\r\r\r\r\r\r\r\r\r\r\r\r\r\r\r\r\r\r\r\r\r\r\r\r\r\r\r\r\r\r\r\r\r\r\r\r\r\r\r\r\r\r\r\r\r\r\r\r\r\r\r\r\r\r", "ExpectedValue"=""}, {"Test_Name"="1294. SelectAllMuxA \"1\" \"1\"", "Step_Type"="", "LowLimit"=0.0, "HighLimit"=0.0, "RValue"="", "RStatus"="", "RetVal"="0", "Units"="", "header1"="=== CCD overvoltage protection test ====", "header2"="--- Test for shorted pins --------------\r\r\r\r\r\r\r\r\r\r\r\r\r\r\r\r\r\r\r\r\r\r\r\r\r\r\r\r\r\r\r\r\r\r\r\r\r\r\r\r\r\r\r\r\r\r\r\r\r\r\r\r\r\r\r\r\r\r\r\r\r\r\r\r\r\r\r\r\r\r\r\r\r\r\r", "ExpectedValue"=""}, {"Test_Name"="1295. SelectMuxA \"1\" \"13\" \"0\"", "Step_Type"="", "LowLimit"=0.0, "HighLimit"=0.0, "RValue"="", "RStatus"="", "RetVal"="0", "Units"="", "header1"="=== CCD overvoltage protection test ====", "header2"="--- Test for shorted pins --------------\r\r\r\r\r\r\r\r\r\r\r\r\r\r\r\r\r\r\r\r\r\r\r\r\r\r\r\r\r\r\r\r\r\r\r\r\r\r\r\r\r\r\r\r\r\r\r\r\r\r\r\r\r\r\r\r\r\r\r\r\r\r\r\r\r\r\r\r\r\r\r\r\r\r\r\r", "ExpectedValue"=""}, {"Test_Name"="1296. CheckCFAdc \"PD2\" \"-.15\" \".3\"", "Step_Type"="NumericLimitTest", "LowLimit"=-0.15, "HighLimit"=0.3, "RValue"="0.027000000700354576", "RStatus"="PASS", "RetVal"="0", "Units"="Volts", "header1"="=== CCD overvoltage protection test ====", "header2"="--- Test for shorted pins --------------\r\r\r\r\r\r\r\r\r\r\r\r\r\r\r\r\r\r\r\r\r\r\r\r\r\r\r\r\r\r\r\r\r\r\r\r\r\r\r\r\r\r\r\r\r\r\r\r\r\r\r\r\r\r\r\r\r\r\r\r\r\r\r\r\r\r\r\r\r\r\r\r\r\r\r\r\r", "ExpectedValue"=""}, {"Test_Name"="1297. SelectAllMuxA \"1\" \"0\"", "Step_Type"="", "LowLimit"=0.0, "HighLimit"=0.0, "RValue"="", "RStatus"="", "RetVal"="0", "Units"="", "header1"="=== CCD overvoltage protection test ====", "header2"="--- Test for shorted pins --------------\r\r\r\r\r\r\r\r\r\r\r\r\r\r\r\r\r\r\r\r\r\r\r\r\r\r\r\r\r\r\r\r\r\r\r\r\r\r\r\r\r\r\r\r\r\r\r\r\r\r\r\r\r\r\r\r\r\r\r\r\r\r\r\r\r\r\r\r\r\r\r\r\r\r\r\r\r\r", "ExpectedValue"=""}, {"Test_Name"="1298. SelectAllMuxB \"1\" \"0\"", "Step_Type"="", "LowLimit"=0.0, "HighLimit"=0.0, "RValue"="", "RStatus"="", "RetVal"="0", "Units"="", "header1"="=== CCD overvoltage protection test ====", "header2"="--- Test for shorted pins --------------\r\r\r\r\r\r\r\r\r\r\r\r\r\r\r\r\r\r\r\r\r\r\r\r\r\r\r\r\r\r\r\r\r\r\r\r\r\r\r\r\r\r\r\r\r\r\r\r\r\r\r\r\r\r\r\r\r\r\r\r\r\r\r\r\r\r\r\r\r\r\r\r\r\r\r\r\r\r\r", "ExpectedValue"=""}, {"Test_Name"="1301. SelectMuxB \"1\" \"14\" \"1\"", "Step_Type"="", "LowLimit"=0.0, "HighLimit"=0.0, "RValue"="", "RStatus"="", "RetVal"="0", "Units"="", "header1"="=== CCD overvoltage protection test ====", "header2"="--- Test for shorted pins --------------\r\r\r\r\r\r\r\r\r\r\r\r\r\r\r\r\r\r\r\r\r\r\r\r\r\r\r\r\r\r\r\r\r\r\r\r\r\r\r\r\r\r\r\r\r\r\r\r\r\r\r\r\r\r\r\r\r\r\r\r\r\r\r\r\r\r\r\r\r\r\r\r\r\r\r\r\r\r\r\r", "ExpectedValue"=""}, {"Test_Name"="1302. SelectAllMuxA \"1\" \"1\"", "Step_Type"="", "LowLimit"=0.0, "HighLimit"=0.0, "RValue"="", "RStatus"="", "RetVal"="0", "Units"="", "header1"="=== CCD overvoltage protection test ====", "header2"="--- Test for shorted pins --------------\r\r\r\r\r\r\r\r\r\r\r\r\r\r\r\r\r\r\r\r\r\r\r\r\r\r\r\r\r\r\r\r\r\r\r\r\r\r\r\r\r\r\r\r\r\r\r\r\r\r\r\r\r\r\r\r\r\r\r\r\r\r\r\r\r\r\r\r\r\r\r\r\r\r\r\r\r\r\r\r\r", "ExpectedValue"=""}, {"Test_Name"="1303. SelectMuxA \"1\" \"14\" \"0\"", "Step_Type"="", "LowLimit"=0.0, "HighLimit"=0.0, "RValue"="", "RStatus"="", "RetVal"="0", "Units"="", "header1"="=== CCD overvoltage protection test ====", "header2"="--- Test for shorted pins --------------\r\r\r\r\r\r\r\r\r\r\r\r\r\r\r\r\r\r\r\r\r\r\r\r\r\r\r\r\r\r\r\r\r\r\r\r\r\r\r\r\r\r\r\r\r\r\r\r\r\r\r\r\r\r\r\r\r\r\r\r\r\r\r\r\r\r\r\r\r\r\r\r\r\r\r\r\r\r\r\r\r\r", "ExpectedValue"=""}, {"Test_Name"="1304. CheckCFAdc \"PD2\" \"-.15\" \".3\"", "Step_Type"="NumericLimitTest", "LowLimit"=-0.15, "HighLimit"=0.3, "RValue"="0.035999998450279236", "RStatus"="PASS", "RetVal"="0", "Units"="Volts", "header1"="=== CCD overvoltage protection test ====", "header2"="--- Test for shorted pins --------------\r\r\r\r\r\r\r\r\r\r\r\r\r\r\r\r\r\r\r\r\r\r\r\r\r\r\r\r\r\r\r\r\r\r\r\r\r\r\r\r\r\r\r\r\r\r\r\r\r\r\r\r\r\r\r\r\r\r\r\r\r\r\r\r\r\r\r\r\r\r\r\r\r\r\r\r\r\r\r\r\r\r\r", "ExpectedValue"=""}, {"Test_Name"="1305. SelectAllMuxA \"1\" \"0\"", "Step_Type"="", "LowLimit"=0.0, "HighLimit"=0.0, "RValue"="", "RStatus"="", "RetVal"="0", "Units"="", "header1"="=== CCD overvoltage protection test ====", "header2"="--- Test for shorted pins --------------\r\r\r\r\r\r\r\r\r\r\r\r\r\r\r\r\r\r\r\r\r\r\r\r\r\r\r\r\r\r\r\r\r\r\r\r\r\r\r\r\r\r\r\r\r\r\r\r\r\r\r\r\r\r\r\r\r\r\r\r\r\r\r\r\r\r\r\r\r\r\r\r\r\r\r\r\r\r\r\r\r\r\r\r", "ExpectedValue"=""}, {"Test_Name"="1306. SelectAllMuxB \"1\" \"0\"", "Step_Type"="", "LowLimit"=0.0, "HighLimit"=0.0, "RValue"="", "RStatus"="", "RetVal"="0", "Units"="", "header1"="=== CCD overvoltage protection test ====", "header2"="--- Test for shorted pins --------------\r\r\r\r\r\r\r\r\r\r\r\r\r\r\r\r\r\r\r\r\r\r\r\r\r\r\r\r\r\r\r\r\r\r\r\r\r\r\r\r\r\r\r\r\r\r\r\r\r\r\r\r\r\r\r\r\r\r\r\r\r\r\r\r\r\r\r\r\r\r\r\r\r\r\r\r\r\r\r\r\r\r\r\r\r", "ExpectedValue"=""}, {"Test_Name"="1309. SelectMuxB \"1\" \"15\" \"1\"", "Step_Type"="", "LowLimit"=0.0, "HighLimit"=0.0, "RValue"="", "RStatus"="", "RetVal"="0", "Units"="", "header1"="=== CCD overvoltage protection test ====", "header2"="--- Test for shorted pins --------------\r\r\r\r\r\r\r\r\r\r\r\r\r\r\r\r\r\r\r\r\r\r\r\r\r\r\r\r\r\r\r\r\r\r\r\r\r\r\r\r\r\r\r\r\r\r\r\r\r\r\r\r\r\r\r\r\r\r\r\r\r\r\r\r\r\r\r\r\r\r\r\r\r\r\r\r\r\r\r\r\r\r\r\r\r\r", "ExpectedValue"=""}, {"Test_Name"="1310. SelectAllMuxA \"1\" \"1\"", "Step_Type"="", "LowLimit"=0.0, "HighLimit"=0.0, "RValue"="", "RStatus"="", "RetVal"="0", "Units"="", "header1"="=== CCD overvoltage protection test ====", "header2"="--- Test for shorted pins --------------\r\r\r\r\r\r\r\r\r\r\r\r\r\r\r\r\r\r\r\r\r\r\r\r\r\r\r\r\r\r\r\r\r\r\r\r\r\r\r\r\r\r\r\r\r\r\r\r\r\r\r\r\r\r\r\r\r\r\r\r\r\r\r\r\r\r\r\r\r\r\r\r\r\r\r\r\r\r\r\r\r\r\r\r\r\r\r", "ExpectedValue"=""}, {"Test_Name"="1311. SelectMuxA \"1\" \"15\" \"0\"", "Step_Type"="", "LowLimit"=0.0, "HighLimit"=0.0, "RValue"="", "RStatus"="", "RetVal"="0", "Units"="", "header1"="=== CCD overvoltage protection test ====", "header2"="--- Test for shorted pins --------------\r\r\r\r\r\r\r\r\r\r\r\r\r\r\r\r\r\r\r\r\r\r\r\r\r\r\r\r\r\r\r\r\r\r\r\r\r\r\r\r\r\r\r\r\r\r\r\r\r\r\r\r\r\r\r\r\r\r\r\r\r\r\r\r\r\r\r\r\r\r\r\r\r\r\r\r\r\r\r\r\r\r\r\r\r\r\r\r", "ExpectedValue"=""}, {"Test_Name"="1312. CheckCFAdc \"PD2\" \"-.15\" \".3\"", "Step_Type"="NumericLimitTest", "LowLimit"=-0.15, "HighLimit"=0.3, "RValue"="0.035999998450279236", "RStatus"="PASS", "RetVal"="0", "Units"="Volts", "header1"="=== CCD overvoltage protection test ====", "header2"="--- Test for shorted pins --------------\r\r\r\r\r\r\r\r\r\r\r\r\r\r\r\r\r\r\r\r\r\r\r\r\r\r\r\r\r\r\r\r\r\r\r\r\r\r\r\r\r\r\r\r\r\r\r\r\r\r\r\r\r\r\r\r\r\r\r\r\r\r\r\r\r\r\r\r\r\r\r\r\r\r\r\r\r\r\r\r\r\r\r\r\r\r\r\r\r", "ExpectedValue"=""}, {"Test_Name"="1313. SelectAllMuxA \"1\" \"0\"", "Step_Type"="", "LowLimit"=0.0, "HighLimit"=0.0, "RValue"="", "RStatus"="", "RetVal"="0", "Units"="", "header1"="=== CCD overvoltage protection test ====", "header2"="--- Test for shorted pins --------------\r\r\r\r\r\r\r\r\r\r\r\r\r\r\r\r\r\r\r\r\r\r\r\r\r\r\r\r\r\r\r\r\r\r\r\r\r\r\r\r\r\r\r\r\r\r\r\r\r\r\r\r\r\r\r\r\r\r\r\r\r\r\r\r\r\r\r\r\r\r\r\r\r\r\r\r\r\r\r\r\r\r\r\r\r\r\r\r\r\r", "ExpectedValue"=""}, {"Test_Name"="1314. SelectAllMuxB \"1\" \"0\"", "Step_Type"="", "LowLimit"=0.0, "HighLimit"=0.0, "RValue"="", "RStatus"="", "RetVal"="0", "Units"="", "header1"="=== CCD overvoltage protection test ====", "header2"="--- Test for shorted pins --------------\r\r\r\r\r\r\r\r\r\r\r\r\r\r\r\r\r\r\r\r\r\r\r\r\r\r\r\r\r\r\r\r\r\r\r\r\r\r\r\r\r\r\r\r\r\r\r\r\r\r\r\r\r\r\r\r\r\r\r\r\r\r\r\r\r\r\r\r\r\r\r\r\r\r\r\r\r\r\r\r\r\r\r\r\r\r\r\r\r\r\r", "ExpectedValue"=""}, {"Test_Name"="1317. SelectAllMuxA \"1\" \"0\"", "Step_Type"="", "LowLimit"=0.0, "HighLimit"=0.0, "RValue"="", "RStatus"="", "RetVal"="0", "Units"="", "header1"="=== CCD overvoltage protection test ====", "header2"="--- Test for shorted pins --------------\r\r\r\r\r\r\r\r\r\r\r\r\r\r\r\r\r\r\r\r\r\r\r\r\r\r\r\r\r\r\r\r\r\r\r\r\r\r\r\r\r\r\r\r\r\r\r\r\r\r\r\r\r\r\r\r\r\r\r\r\r\r\r\r\r\r\r\r\r\r\r\r\r\r\r\r\r\r\r\r\r\r\r\r\r\r\r\r\r\r\r\r", "ExpectedValue"=""}, {"Test_Name"="1318. SelectAllMuxB \"1\" \"0\"", "Step_Type"="", "LowLimit"=0.0, "HighLimit"=0.0, "RValue"="", "RStatus"="", "RetVal"="0", "Units"="", "header1"="=== CCD overvoltage protection test ====", "header2"="--- Test for shorted pins --------------\r\r\r\r\r\r\r\r\r\r\r\r\r\r\r\r\r\r\r\r\r\r\r\r\r\r\r\r\r\r\r\r\r\r\r\r\r\r\r\r\r\r\r\r\r\r\r\r\r\r\r\r\r\r\r\r\r\r\r\r\r\r\r\r\r\r\r\r\r\r\r\r\r\r\r\r\r\r\r\r\r\r\r\r\r\r\r\r\r\r\r\r\r", "ExpectedValue"=""}, {"Test_Name"="1319. SetG15PullUp \"A\" \"0\"", "Step_Type"="", "LowLimit"=0.0, "HighLimit"=0.0, "RValue"="", "RStatus"="", "RetVal"="0", "Units"="", "header1"="=== CCD overvoltage protection test ====", "header2"="--- Test for shorted pins --------------\r\r\r\r\r\r\r\r\r\r\r\r\r\r\r\r\r\r\r\r\r\r\r\r\r\r\r\r\r\r\r\r\r\r\r\r\r\r\r\r\r\r\r\r\r\r\r\r\r\r\r\r\r\r\r\r\r\r\r\r\r\r\r\r\r\r\r\r\r\r\r\r\r\r\r\r\r\r\r\r\r\r\r\r\r\r\r\r\r\r\r\r\r\r", "ExpectedValue"=""}, {"Test_Name"="1320. SetG15PullUp \"B\" \"0\"", "Step_Type"="", "LowLimit"=0.0, "HighLimit"=0.0, "RValue"="", "RStatus"="", "RetVal"="0", "Units"="", "header1"="=== CCD overvoltage protection test ====", "header2"="--- Test for shorted pins --------------\r\r\r\r\r\r\r\r\r\r\r\r\r\r\r\r\r\r\r\r\r\r\r\r\r\r\r\r\r\r\r\r\r\r\r\r\r\r\r\r\r\r\r\r\r\r\r\r\r\r\r\r\r\r\r\r\r\r\r\r\r\r\r\r\r\r\r\r\r\r\r\r\r\r\r\r\r\r\r\r\r\r\r\r\r\r\r\r\r\r\r\r\r\r\r", "ExpectedValue"=""}, {"Test_Name"="1321. SetG15PullDown \"A\" \"0\"", "Step_Type"="", "LowLimit"=0.0, "HighLimit"=0.0, "RValue"="", "RStatus"="", "RetVal"="0", "Units"="", "header1"="=== CCD overvoltage protection test ====", "header2"="--- Test for shorted pins --------------\r\r\r\r\r\r\r\r\r\r\r\r\r\r\r\r\r\r\r\r\r\r\r\r\r\r\r\r\r\r\r\r\r\r\r\r\r\r\r\r\r\r\r\r\r\r\r\r\r\r\r\r\r\r\r\r\r\r\r\r\r\r\r\r\r\r\r\r\r\r\r\r\r\r\r\r\r\r\r\r\r\r\r\r\r\r\r\r\r\r\r\r\r\r\r\r", "ExpectedValue"=""}, {"Test_Name"="1322. SetG15PullDown \"B\" \"0\"", "Step_Type"="", "LowLimit"=0.0, "HighLimit"=0.0, "RValue"="", "RStatus"="", "RetVal"="0", "Units"="", "header1"="=== CCD overvoltage protection test ====", "header2"="--- Test for shorted pins --------------\r\r\r\r\r\r\r\r\r\r\r\r\r\r\r\r\r\r\r\r\r\r\r\r\r\r\r\r\r\r\r\r\r\r\r\r\r\r\r\r\r\r\r\r\r\r\r\r\r\r\r\r\r\r\r\r\r\r\r\r\r\r\r\r\r\r\r\r\r\r\r\r\r\r\r\r\r\r\r\r\r\r\r\r\r\r\r\r\r\r\r\r\r\r\r\r\r", "ExpectedValue"=""}, {"Test_Name"="1325.  ---HS CAN TX RX test with square wave---", "Step_Type"="", "LowLimit"=0.0, "HighLimit"=0.0, "RValue"="", "RStatus"="", "RetVal"="", "Units"="", "header1"="=== CCD overvoltage protection test ====", "header2"="---HS CAN TX RX test with square wave---\r", "ExpectedValue"=""}, {"Test_Name"="1326. ResetAsicRegister \"1\" \"ALL\"", "Step_Type"="", "LowLimit"=0.0, "HighLimit"=0.0, "RValue"="", "RStatus"="", "RetVal"="0", "Units"="", "header1"="=== CCD overvoltage protection test ====", "header2"="---HS CAN TX RX test with square wave---\r\r", "ExpectedValue"=""}, {"Test_Name"="1327. SetFpgaRegister \"129\" \"00\"", "Step_Type"="", "LowLimit"=0.0, "HighLimit"=0.0, "RValue"="", "RStatus"="", "RetVal"="0", "Units"="", "header1"="=== CCD overvoltage protection test ====", "header2"="---HS CAN TX RX test with square wave---\r\r\r", "ExpectedValue"=""}, {"Test_Name"="1328. CheckFpgaRegister \"984\" \"02\" \"0\"", "Step_Type"="StringValueTest", "LowLimit"=0.0, "HighLimit"=0.0, "RValue"="2", "RStatus"="PASS", "RetVal"="0", "Units"="", "header1"="=== CCD overvoltage protection test ====", "header2"="---HS CAN TX RX test with square wave---\r\r\r\r", "ExpectedValue"=""}, {"Test_Name"="1330. SetAsicRegister \"1\" \"00\" \"20\"", "Step_Type"="", "LowLimit"=0.0, "HighLimit"=0.0, "RValue"="", "RStatus"="", "RetVal"="0", "Units"="", "header1"="=== CCD overvoltage protection test ====", "header2"="---HS CAN TX RX test with square wave---\r\r\r\r\r", "ExpectedValue"=""}, {"Test_Name"="1331. SetAsicRegister \"1\" \"01\" \"08\"", "Step_Type"="", "LowLimit"=0.0, "HighLimit"=0.0, "RValue"="", "RStatus"="", "RetVal"="0", "Units"="", "header1"="=== CCD overvoltage protection test ====", "header2"="---HS CAN TX RX test with square wave---\r\r\r\r\r\r", "ExpectedValue"=""}, {"Test_Name"="1332. SetAsicRegister \"1\" \"02\" \"28\"", "Step_Type"="", "LowLimit"=0.0, "HighLimit"=0.0, "RValue"="", "RStatus"="", "RetVal"="0", "Units"="", "header1"="=== CCD overvoltage protection test ====", "header2"="---HS CAN TX RX test with square wave---\r\r\r\r\r\r\r", "ExpectedValue"=""}, {"Test_Name"="1333. SetAsicRegister \"1\" \"04\" \"c0\"", "Step_Type"="", "LowLimit"=0.0, "HighLimit"=0.0, "RValue"="", "RStatus"="", "RetVal"="0", "Units"="", "header1"="=== CCD overvoltage protection test ====", "header2"="---HS CAN TX RX test with square wave---\r\r\r\r\r\r\r\r", "ExpectedValue"=""}, {"Test_Name"="1334. SetAsicRegister \"1\" \"07\" \"0c\"", "Step_Type"="", "LowLimit"=0.0, "HighLimit"=0.0, "RValue"="", "RStatus"="", "RetVal"="0", "Units"="", "header1"="=== CCD overvoltage protection test ====", "header2"="---HS CAN TX RX test with square wave---\r\r\r\r\r\r\r\r\r", "ExpectedValue"=""}, {"Test_Name"="1335. SetFpgaRegister \"983\" \"80\"", "Step_Type"="", "LowLimit"=0.0, "HighLimit"=0.0, "RValue"="", "RStatus"="", "RetVal"="0", "Units"="", "header1"="=== CCD overvoltage protection test ====", "header2"="---HS CAN TX RX test with square wave---\r\r\r\r\r\r\r\r\r\r", "ExpectedValue"=""}, {"Test_Name"="1336. CheckFpgaRegister \"984\" \"02\" \"1\"", "Step_Type"="StringValueTest", "LowLimit"=0.0, "HighLimit"=0.0, "RValue"="6", "RStatus"="PASS", "RetVal"="0", "Units"="", "header1"="=== CCD overvoltage protection test ====", "header2"="---HS CAN TX RX test with square wave---\r\r\r\r\r\r\r\r\r\r\r", "ExpectedValue"=""}, {"Test_Name"="1338. ResetAsicRegister \"1\" \"ALL\"", "Step_Type"="", "LowLimit"=0.0, "HighLimit"=0.0, "RValue"="", "RStatus"="", "RetVal"="0", "Units"="", "header1"="=== CCD overvoltage protection test ====", "header2"="---HS CAN TX RX test with square wave---\r\r\r\r\r\r\r\r\r\r\r\r", "ExpectedValue"=""}, {"Test_Name"="1339. SetFpgaRegister \"129\" \"00\"", "Step_Type"="", "LowLimit"=0.0, "HighLimit"=0.0, "RValue"="", "RStatus"="", "RetVal"="0", "Units"="", "header1"="=== CCD overvoltage protection test ====", "header2"="---HS CAN TX RX test with square wave---\r\r\r\r\r\r\r\r\r\r\r\r\r", "ExpectedValue"=""}, {"Test_Name"="1340. CheckFpgaRegister \"984\" \"02\" \"0\"", "Step_Type"="StringValueTest", "LowLimit"=0.0, "HighLimit"=0.0, "RValue"="2", "RStatus"="PASS", "RetVal"="0", "Units"="", "header1"="=== CCD overvoltage protection test ====", "header2"="---HS CAN TX RX test with square wave---\r\r\r\r\r\r\r\r\r\r\r\r\r\r", "ExpectedValue"=""}, {"Test_Name"="1341. SetAsicRegister \"1\" \"00\" \"20\"", "Step_Type"="", "LowLimit"=0.0, "HighLimit"=0.0, "RValue"="", "RStatus"="", "RetVal"="0", "Units"="", "header1"="=== CCD overvoltage protection test ====", "header2"="---HS CAN TX RX test with square wave---\r\r\r\r\r\r\r\r\r\r\r\r\r\r\r", "ExpectedValue"=""}, {"Test_Name"="1342. SetAsicRegister \"1\" \"01\" \"08\"", "Step_Type"="", "LowLimit"=0.0, "HighLimit"=0.0, "RValue"="", "RStatus"="", "RetVal"="0", "Units"="", "header1"="=== CCD overvoltage protection test ====", "header2"="---HS CAN TX RX test with square wave---\r\r\r\r\r\r\r\r\r\r\r\r\r\r\r\r", "ExpectedValue"=""}, {"Test_Name"="1343. SetAsicRegister \"1\" \"02\" \"28\"", "Step_Type"="", "LowLimit"=0.0, "HighLimit"=0.0, "RValue"="", "RStatus"="", "RetVal"="0", "Units"="", "header1"="=== CCD overvoltage protection test ====", "header2"="---HS CAN TX RX test with square wave---\r\r\r\r\r\r\r\r\r\r\r\r\r\r\r\r\r", "ExpectedValue"=""}, {"Test_Name"="1344. SetAsicRegister \"1\" \"04\" \"c0\"", "Step_Type"="", "LowLimit"=0.0, "HighLimit"=0.0, "RValue"="", "RStatus"="", "RetVal"="0", "Units"="", "header1"="=== CCD overvoltage protection test ====", "header2"="---HS CAN TX RX test with square wave---\r\r\r\r\r\r\r\r\r\r\r\r\r\r\r\r\r\r", "ExpectedValue"=""}, {"Test_Name"="1345. SetAsicRegister \"1\" \"07\" \"0c\"", "Step_Type"="", "LowLimit"=0.0, "HighLimit"=0.0, "RValue"="", "RStatus"="", "RetVal"="0", "Units"="", "header1"="=== CCD overvoltage protection test ====", "header2"="---HS CAN TX RX test with square wave---\r\r\r\r\r\r\r\r\r\r\r\r\r\r\r\r\r\r\r", "ExpectedValue"=""}, {"Test_Name"="1346. SetFpgaRegister \"983\" \"40\"", "Step_Type"="", "LowLimit"=0.0, "HighLimit"=0.0, "RValue"="", "RStatus"="", "RetVal"="0", "Units"="", "header1"="=== CCD overvoltage protection test ====", "header2"="---HS CAN TX RX test with square wave---\r\r\r\r\r\r\r\r\r\r\r\r\r\r\r\r\r\r\r\r", "ExpectedValue"=""}, {"Test_Name"="1347. CheckFpgaRegister \"984\" \"02\" \"1\"", "Step_Type"="StringValueTest", "LowLimit"=0.0, "HighLimit"=0.0, "RValue"="6", "RStatus"="PASS", "RetVal"="0", "Units"="", "header1"="=== CCD overvoltage protection test ====", "header2"="---HS CAN TX RX test with square wave---\r\r\r\r\r\r\r\r\r\r\r\r\r\r\r\r\r\r\r\r\r", "ExpectedValue"=""}, {"Test_Name"="1351. CheckGepWifiModule \"'SSP Wifi'\"", "Step_Type"="StringValueTest", "LowLimit"=0.0, "HighLimit"=0.0, "RValue"="b'2.6$2.7$2$0$0.6$0.8$250MHZ$28$ScopeNotInit$'", "RStatus"="Fail", "RetVal"="33", "Units"="", "header1"="=== CCD overvoltage protection test ====", "header2"="---HS CAN TX RX test with square wave---\r\r\r\r\r\r\r\r\r\r\r\r\r\r\r\r\r\r\r\r\r\r", "ExpectedValue"=""}, {"Test_Name"="1356. CheckVehCommSPI", "Step_Type"="", "LowLimit"=0.0, "HighLimit"=0.0, "RValue"="", "RStatus"="", "RetVal"="2030", "Units"="", "header1"="=== CCD overvoltage protection test ====", "header2"="---HS CAN TX RX test with square wave---\r\r\r\r\r\r\r\r\r\r\r\r\r\r\r\r\r\r\r\r\r\r\r", "ExpectedValue"=""}, {"Test_Name"="1359. CheckRealtimeClock \"2\"", "Step_Type"="StringValueTest", "LowLimit"=0.0, "HighLimit"=0.0, "RValue"="1464737167", "RStatus"="PASS", "RetVal"="0", "Units"="", "header1"="=== CCD overvoltage protection test ====", "header2"="---HS CAN TX RX test with square wave---\r\r\r\r\r\r\r\r\r\r\r\r\r\r\r\r\r\r\r\r\r\r\r\r", "ExpectedValue"=""}, {"Test_Name"="1423. SetG15PullupVbat \"0\" \"0\"", "Step_Type"="", "LowLimit"=0.0, "HighLimit"=0.0, "RValue"="", "RStatus"="", "RetVal"="0", "Units"="", "header1"="=== CCD overvoltage protection test ====", "header2"="---HS CAN TX RX test with square wave---\r\r\r\r\r\r\r\r\r\r\r\r\r\r\r\r\r\r\r\r\r\r\r\r\r", "ExpectedValue"=""}, {"Test_Name"="1424. SetG15PullUp \"A\" \"0\"", "Step_Type"="", "LowLimit"=0.0, "HighLimit"=0.0, "RValue"="", "RStatus"="", "RetVal"="0", "Units"="", "header1"="=== CCD overvoltage protection test ====", "header2"="---HS CAN TX RX test with square wave---\r\r\r\r\r\r\r\r\r\r\r\r\r\r\r\r\r\r\r\r\r\r\r\r\r\r", "ExpectedValue"=""}, {"Test_Name"="1425. SetG15PullUp \"B\" \"0\"", "Step_Type"="", "LowLimit"=0.0, "HighLimit"=0.0, "RValue"="", "RStatus"="", "RetVal"="0", "Units"="", "header1"="=== CCD overvoltage protection test ====", "header2"="---HS CAN TX RX test with square wave---\r\r\r\r\r\r\r\r\r\r\r\r\r\r\r\r\r\r\r\r\r\r\r\r\r\r\r", "ExpectedValue"=""}, {"Test_Name"="1426. SetG15PullDown \"A\" \"0\"", "Step_Type"="", "LowLimit"=0.0, "HighLimit"=0.0, "RValue"="", "RStatus"="", "RetVal"="0", "Units"="", "header1"="=== CCD overvoltage protection test ====", "header2"="---HS CAN TX RX test with square wave---\r\r\r\r\r\r\r\r\r\r\r\r\r\r\r\r\r\r\r\r\r\r\r\r\r\r\r\r", "ExpectedValue"=""}, {"Test_Name"="1427. SetG15PullDown \"B\" \"0\"", "Step_Type"="", "LowLimit"=0.0, "HighLimit"=0.0, "RValue"="", "RStatus"="", "RetVal"="0", "Units"="", "header1"="=== CCD overvoltage protection test ====", "header2"="---HS CAN TX RX test with square wave---\r\r\r\r\r\r\r\r\r\r\r\r\r\r\r\r\r\r\r\r\r\r\r\r\r\r\r\r\r", "ExpectedValue"=""}, {"Test_Name"="1428. SelectAllMuxA \"1\" \"0\"", "Step_Type"="", "LowLimit"=0.0, "HighLimit"=0.0, "RValue"="", "RStatus"="", "RetVal"="0", "Units"="", "header1"="=== CCD overvoltage protection test ====", "header2"="---HS CAN TX RX test with square wave---\r\r\r\r\r\r\r\r\r\r\r\r\r\r\r\r\r\r\r\r\r\r\r\r\r\r\r\r\r\r", "ExpectedValue"=""}, {"Test_Name"="1429. SelectAllMuxB \"1\" \"0\"", "Step_Type"="", "LowLimit"=0.0, "HighLimit"=0.0, "RValue"="", "RStatus"="", "RetVal"="0", "Units"="", "header1"="=== CCD overvoltage protection test ====", "header2"="---HS CAN TX RX test with square wave---\r\r\r\r\r\r\r\r\r\r\r\r\r\r\r\r\r\r\r\r\r\r\r\r\r\r\r\r\r\r\r", "ExpectedValue"=""}, {"Test_Name"="1431. SetG15PullupVbat \"1\" \"0\"", "Step_Type"="", "LowLimit"=0.0, "HighLimit"=0.0, "RValue"="", "RStatus"="", "RetVal"="0", "Units"="", "header1"="=== CCD overvoltage protection test ====", "header2"="---HS CAN TX RX test with square wave---\r\r\r\r\r\r\r\r\r\r\r\r\r\r\r\r\r\r\r\r\r\r\r\r\r\r\r\r\r\r\r\r", "ExpectedValue"=""}, {"Test_Name"="1432. SetG15PullUp \"C\" \"0\"", "Step_Type"="", "LowLimit"=0.0, "HighLimit"=0.0, "RValue"="", "RStatus"="", "RetVal"="0", "Units"="", "header1"="=== CCD overvoltage protection test ====", "header2"="---HS CAN TX RX test with square wave---\r\r\r\r\r\r\r\r\r\r\r\r\r\r\r\r\r\r\r\r\r\r\r\r\r\r\r\r\r\r\r\r\r", "ExpectedValue"=""}, {"Test_Name"="1433. SetG15PullUp \"D\" \"0\"", "Step_Type"="", "LowLimit"=0.0, "HighLimit"=0.0, "RValue"="", "RStatus"="", "RetVal"="0", "Units"="", "header1"="=== CCD overvoltage protection test ====", "header2"="---HS CAN TX RX test with square wave---\r\r\r\r\r\r\r\r\r\r\r\r\r\r\r\r\r\r\r\r\r\r\r\r\r\r\r\r\r\r\r\r\r\r", "ExpectedValue"=""}, {"Test_Name"="1434. SetG15PullDown \"C\" \"0\"", "Step_Type"="", "LowLimit"=0.0, "HighLimit"=0.0, "RValue"="", "RStatus"="", "RetVal"="0", "Units"="", "header1"="=== CCD overvoltage protection test ====", "header2"="---HS CAN TX RX test with square wave---\r\r\r\r\r\r\r\r\r\r\r\r\r\r\r\r\r\r\r\r\r\r\r\r\r\r\r\r\r\r\r\r\r\r\r", "ExpectedValue"=""}, {"Test_Name"="1435. SetG15PullDown \"D\" \"0\"", "Step_Type"="", "LowLimit"=0.0, "HighLimit"=0.0, "RValue"="", "RStatus"="", "RetVal"="0", "Units"="", "header1"="=== CCD overvoltage protection test ====", "header2"="---HS CAN TX RX test with square wave---\r\r\r\r\r\r\r\r\r\r\r\r\r\r\r\r\r\r\r\r\r\r\r\r\r\r\r\r\r\r\r\r\r\r\r\r", "ExpectedValue"=""}, {"Test_Name"="1436. SelectAllMuxA \"2\" \"0\"", "Step_Type"="", "LowLimit"=0.0, "HighLimit"=0.0, "RValue"="", "RStatus"="", "RetVal"="0", "Units"="", "header1"="=== CCD overvoltage protection test ====", "header2"="---HS CAN TX RX test with square wave---\r\r\r\r\r\r\r\r\r\r\r\r\r\r\r\r\r\r\r\r\r\r\r\r\r\r\r\r\r\r\r\r\r\r\r\r\r", "ExpectedValue"=""}, {"Test_Name"="1437. SelectAllMuxB \"2\" \"0\"", "Step_Type"="", "LowLimit"=0.0, "HighLimit"=0.0, "RValue"="", "RStatus"="", "RetVal"="0", "Units"="", "header1"="=== CCD overvoltage protection test ====", "header2"="---HS CAN TX RX test with square wave---\r\r\r\r\r\r\r\r\r\r\r\r\r\r\r\r\r\r\r\r\r\r\r\r\r\r\r\r\r\r\r\r\r\r\r\r\r\r", "ExpectedValue"=""}, {"Test_Name"="1439. ResetAsicRegister \"1\" \"ALL\"", "Step_Type"="", "LowLimit"=0.0, "HighLimit"=0.0, "RValue"="", "RStatus"="", "RetVal"="0", "Units"="", "header1"="=== CCD overvoltage protection test ====", "header2"="---HS CAN TX RX test with square wave---\r\r\r\r\r\r\r\r\r\r\r\r\r\r\r\r\r\r\r\r\r\r\r\r\r\r\r\r\r\r\r\r\r\r\r\r\r\r\r", "ExpectedValue"=""}, {"Test_Name"="1440. ResetAsicRegister \"2\" \"ALL\"", "Step_Type"="", "LowLimit"=0.0, "HighLimit"=0.0, "RValue"="", "RStatus"="", "RetVal"="0", "Units"="", "header1"="=== CCD overvoltage protection test ====", "header2"="---HS CAN TX RX test with square wave---\r\r\r\r\r\r\r\r\r\r\r\r\r\r\r\r\r\r\r\r\r\r\r\r\r\r\r\r\r\r\r\r\r\r\r\r\r\r\r\r", "ExpectedValue"=""}, {"Test_Name"="1442. SetFpgaRegister \"8AD\" \"1\"", "Step_Type"="", "LowLimit"=0.0, "HighLimit"=0.0, "RValue"="", "RStatus"="", "RetVal"="0", "Units"="", "header1"="=== CCD overvoltage protection test ====", "header2"="---HS CAN TX RX test with square wave---\r\r\r\r\r\r\r\r\r\r\r\r\r\r\r\r\r\r\r\r\r\r\r\r\r\r\r\r\r\r\r\r\r\r\r\r\r\r\r\r\r", "ExpectedValue"=""}, {"Test_Name"="1458.  === NO TRIP TESTS AT 120 mA ===", "Step_Type"="", "LowLimit"=0.0, "HighLimit"=0.0, "RValue"="", "RStatus"="", "RetVal"="", "Units"="", "header1"="=== NO TRIP TESTS AT 120 mA ============", "header2"="---HS CAN TX RX test with square wave---\r\r\r\r\r\r\r\r\r\r\r\r\r\r\r\r\r\r\r\r\r\r\r\r\r\r\r\r\r\r\r\r\r\r\r\r\r\r\r\r\r\r", "ExpectedValue"=""}, {"Test_Name"="1462. No_Trip_Tests_at_120mA.exe", "Step_Type"="", "LowLimit"=0.0, "HighLimit"=0.0, "RValue"="", "RStatus"="", "RetVal"="", "Units"="", "header1"="=== NO TRIP TESTS AT 120 mA ============", "header2"="---HS CAN TX RX test with square wave---\r\r\r\r\r\r\r\r\r\r\r\r\r\r\r\r\r\r\r\r\r\r\r\r\r\r\r\r\r\r\r\r\r\r\r\r\r\r\r\r\r\r\r", "ExpectedValue"=""}, {"Test_Name"="1465. SelectMuxA \"1\" \"1\" \"1\"", "Step_Type"="", "LowLimit"=0.0, "HighLimit"=0.0, "RValue"="", "RStatus"="", "RetVal"="0", "Units"="", "header1"="=== NO TRIP TESTS AT 120 mA ============", "header2"="---HS CAN TX RX test with square wave---\r\r\r\r\r\r\r\r\r\r\r\r\r\r\r\r\r\r\r\r\r\r\r\r\r\r\r\r\r\r\r\r\r\r\r\r\r\r\r\r\r\r\r\r", "ExpectedValue"=""}, {"Test_Name"="1466. SelectMuxA \"2\" \"1\" \"1\"", "Step_Type"="", "LowLimit"=0.0, "HighLimit"=0.0, "RValue"="", "RStatus"="", "RetVal"="0", "Units"="", "header1"="=== NO TRIP TESTS AT 120 mA ============", "header2"="---HS CAN TX RX test with square wave---\r\r\r\r\r\r\r\r\r\r\r\r\r\r\r\r\r\r\r\r\r\r\r\r\r\r\r\r\r\r\r\r\r\r\r\r\r\r\r\r\r\r\r\r\r", "ExpectedValue"=""}, {"Test_Name"="1467. CheckCFAdc \"PD1\" \"14\" \"15.5\"", "Step_Type"="NumericLimitTest", "LowLimit"=14.0, "HighLimit"=15.5, "RValue"="2.8259999752044678", "RStatus"="Fail", "RetVal"="0", "Units"="Volts", "header1"="=== NO TRIP TESTS AT 120 mA ============", "header2"="---HS CAN TX RX test with square wave---\r\r\r\r\r\r\r\r\r\r\r\r\r\r\r\r\r\r\r\r\r\r\r\r\r\r\r\r\r\r\r\r\r\r\r\r\r\r\r\r\r\r\r\r\r\r", "ExpectedValue"=""}, {"Test_Name"="1468. CheckCFAdc \"PD3\" \"14\" \"15.5\"", "Step_Type"="NumericLimitTest", "LowLimit"=14.0, "HighLimit"=15.5, "RValue"="3.203000068664551", "RStatus"="Fail", "RetVal"="0", "Units"="Volts", "header1"="=== NO TRIP TESTS AT 120 mA ============", "header2"="---HS CAN TX RX test with square wave---\r\r\r\r\r\r\r\r\r\r\r\r\r\r\r\r\r\r\r\r\r\r\r\r\r\r\r\r\r\r\r\r\r\r\r\r\r\r\r\r\r\r\r\r\r\r\r", "ExpectedValue"=""}], 2 "Result":T1, 3 "Report Text":string, 5 "Excel Column Names":string[](array[string])=["59. GetScannerDeviceType", "66. PromptUserPassFail \"Please listen for a beep!\" \"OK\" \"Cancel\"", "68. PromptUserPassFail \"Did you hear a beep?\" \"YES\" \"NO\"", "72. PromptUserPassFail \"Did you Verify the 2 LEDs turn on near uSD connector?\" \"YES\" \"NO\"", "119. CheckTestAppVersion \"2.6\"", "120. CheckFPGAVersion \"2.7\"", "121. CheckIPLVersion \"0.6\"", "122. CheckSPL1Version \"0.8\"", "128. CheckCFAdc \"VBAT\" \"14.5\" \"15.6\"", "131. CheckCFAdc \"PVA_Volts\" \"9.7\" \"10.3\"", "140. CheckCFAdc \"PD1\" \"19.5\" \"20.5\"", "141. CheckCFAdc \"PD2\" \"19.5\" \"20.5\"", "142. CheckCFAdc \"PD3\" \"19.5\" \"20.5\"", "143. CheckCFAdc \"PD4\" \"19.5\" \"20.5\"", "144. CheckFpgaRegister \"8ae\" \"0\" \"1\"", "165. CheckCFAdc \"PD1\" \"4.5\" \"5.0\"", "166. CheckCFAdc \"PD2\" \"4.5\" \"5.0\"", "171. CheckCFAdc \"PD1\" \"4.1\" \"4.55\"", "172. CheckCFAdc \"PD2\" \"4.1\" \"4.55\"", "177. CheckCFAdc \"PD1\" \"2.3\" \"2.6\"", "178. CheckCFAdc \"PD2\" \"2.3\" \"2.6\"", "185. CheckCFAdc \"PD1\" \"4.35\" \"4.85\"", "186. CheckCFAdc \"PD2\" \"4.35\" \"4.85\"", "193. CheckCFAdc \"PD1\" \"3.95\" \"4.45\"", "194. CheckCFAdc \"PD2\" \"3.95\" \"4.45\"", "201. CheckCFAdc \"PD1\" \"4.3\" \"4.8\"", "202. CheckCFAdc \"PD2\" \"4.3\" \"4.8\"", "209. CheckCFAdc \"PD1\" \"4.1\" \"4.6\"", "210. CheckCFAdc \"PD2\" \"4.1\" \"4.6\"", "217. CheckCFAdc \"PD1\" \"3.7\" \"4.2\"", "218. CheckCFAdc \"PD2\" \"3.7\" \"4.2\"", "225. CheckCFAdc \"PD1\" \"3.5\" \"4.0\"", "226. CheckCFAdc \"PD2\" \"3.5\" \"4.0\"", "233. CheckCFAdc \"PD1\" \"3.4\" \"3.9\"", "234. CheckCFAdc \"PD2\" \"3.4\" \"3.9\"", "241. CheckCFAdc \"PD1\" \"3.25\" \"3.7\"", "242. CheckCFAdc \"PD2\" \"3.25\" \"3.7\"", "249. CheckCFAdc \"PD1\" \"3.1\" \"3.5\"", "250. CheckCFAdc \"PD2\" \"3.1\" \"3.5\"", "257. CheckCFAdc \"PD1\" \"2.25\" \"2.65\"", "258. CheckCFAdc \"PD2\" \"2.25\" \"2.65\"", "265. CheckCFAdc \"PD1\" \"4.55\" \"5.0\"", "266. CheckCFAdc \"PD2\" \"4.55\" \"5.0\"", "273. CheckCFAdc \"PD1\" \"-.15\" \".3\"", "274. CheckCFAdc \"PD2\" \"-.15\" \".3\"", "292. CheckCFAdc \"PD1\" \"14\" \"15.5\"", "296. CheckCFAdc \"PD1\" \"-.15\" \".3\"", "298. CheckCFAdc \"PD1\" \"14\" \"15.5\"", "312. CheckCFAdc \"PD1\" \"-.15\" \"1.2\"", "315. CheckCFAdc \"PD1\" \"12.5\" \"13.5\"", "317. CheckCFAdc \"PD1\" \"11\" \"12.2\"", "321. CheckCFAdc \"PD2\" \"-.15\" \"1.4\"", "324. CheckCFAdc \"PD2\" \"12.3\" \"13.7\"", "326. CheckCFAdc \"PD2\" \"11\" \"12.2\"", "328. CheckCFAdc \"PD2\" \"14\" \"15.5\"", "330. CheckCFAdc \"PD2\" \"-.15\" \".3\"", "347. CheckCFAdc \"PD1\" \"6.9\" \"7.7\"", "348. CheckCFAdc \"PD2\" \"6.9\" \"7.7\"", "352. CheckCFAdc \"PD1\" \"2.15\" \"2.65\"", "353. CheckCFAdc \"PD2\" \"2.15\" \"2.65\"", "373. CheckCFAdc \"PD1\" \"2.15\" \"2.65\"", "378. CheckFpgaRegister \"8A8\" \"0\" \"0\"", "379. CheckFpgaRegister \"8A8\" \"1\" \"0\"", "380. CheckFpgaRegister \"858\" \"4\" \"0\"", "381. CheckFpgaRegister \"859\" \"6\" \"0\"", "382. ComparatorCheck \"9\" \"0\"", "383. ComparatorCheck \"15\" \"0\"", "388. CheckFpgaRegister \"8A8\" \"0\" \"1\"", "389. CheckFpgaRegister \"8A8\" \"1\" \"1\"", "390. CheckFpgaRegister \"858\" \"4\" \"1\"", "391. CheckFpgaRegister \"859\" \"6\" \"1\"", "392. ComparatorCheck \"9\" \"1\"", "393. ComparatorCheck \"15\" \"1\"", "416. CheckCFAdc \"PD1\" \"2.2\" \"2.65\"", "417. CheckCFAdc \"PD3\" \"-.15\" \"1.2\"", "421. CheckCFAdc \"PD3\" \"2.2\" \"2.65\"", "427. CheckCFAdc \"PD3\" \"2.2\" \"2.65\"", "433. CheckCFAdc \"PD3\" \"2.2\" \"2.65\"", "439. CheckCFAdc \"PD3\" \"2.2\" \"2.65\"", "445. CheckCFAdc \"PD3\" \"2.2\" \"2.65\"", "451. CheckCFAdc \"PD3\" \"2.2\" \"2.65\"", "457. CheckCFAdc \"PD3\" \"2.2\" \"2.65\"", "463. CheckCFAdc \"PD3\" \"2.2\" \"2.65\"", "469. CheckCFAdc \"PD3\" \"2.2\" \"2.65\"", "475. CheckCFAdc \"PD3\" \"2.2\" \"2.65\"", "481. CheckCFAdc \"PD3\" \"2.2\" \"2.65\"", "487. CheckCFAdc \"PD3\" \"2.2\" \"2.65\"", "493. CheckCFAdc \"PD3\" \"2.2\" \"2.65\"", "505. CheckCFAdc \"PD1\" \"2.3\" \"2.7\"", "506. CheckCFAdc \"PD2\" \"2.3\" \"2.7\"", "516. CheckCFAdc \"PD1\" \"-.15\" \".3\"", "517. CheckCFAdc \"PD2\" \"7.2\" \"8\"", "520. CheckCFAdc \"PD1\" \"3.35\" \"3.85\"", "521. CheckCFAdc \"PD2\" \"7.2\" \"8.0\"", "522. CheckFpgaRegister \"984\" \"1\" \"0\"", "524. CheckCFAdc \"PD1\" \"-.15\" \".3\"", "525. CheckCFAdc \"PD2\" \"3.5\" \"3.95\"", "528. CheckCFAdc \"PD1\" \"4.3\" \"4.9\"", "529. CheckCFAdc \"PD2\" \"3.5\" \"3.9\"", "530. CheckFpgaRegister \"984\" \"1\" \"1\"", "533. CheckFpgaRegister \"984\" \"1\" \"0\"", "535. CheckFpgaRegister \"984\" \"1\" \"1\"", "538. CheckFpgaRegister \"984\" \"1\" \"0\"", "541. CheckCFAdc \"PD1\" \"7.4\" \"8.3\"", "542. CheckCFAdc \"PD2\" \"-.15\" \".3\"", "544. CheckCFAdc \"PD1\" \"-.15\" \".3\"", "545. CheckCFAdc \"PD2\" \"-.15\" \".3\"", "547. CheckCFAdc \"PD1\" \"7.4\" \"8.3\"", "548. CheckCFAdc \"PD2\" \"7.2\" \"8.0\"", "550. CheckCFAdc \"PD1\" \"-.15\" \".3\"", "551. CheckCFAdc \"PD2\" \"7.2\" \"8.0\"", "558. CheckCFAdc \"PD1\" \"-.15\" \".3\"", "559. CheckCFAdc \"PD2\" \"12.8\" \"14\"", "569. CheckCFAdc \"PD1\" \"5.0\" \"5.5\"", "570. CheckCFAdc \"PD2\" \"4.8\" \"5.3\"", "572. CheckCFAdc \"PD1\" \"-.15\" \"0.3\"", "573. CheckCFAdc \"PD2\" \"4.8\" \"5.3\"", "584. CheckCFAdc \"PD1\" \"4.5\" \"5.0\"", "585. CheckCFAdc \"PD2\" \".5\" \"1.4\"", "586. CheckFpgaRegister \"632\" \"0\" \"0\"", "590. CheckCFAdc \"PD1\" \".5\" \"1.5\"", "591. CheckCFAdc \"PD2\" \"4.5\" \"5.0\"", "592. CheckFpgaRegister \"632\" \"0\" \"1\"", "595. CheckCFAdc \"PD1\" \"4.5\" \"5.0\"", "596. CheckCFAdc \"PD2\" \".5\" \"1.6\"", "597. CheckFpgaRegister \"632\" \"0\" \"0\"", "601. CheckCFAdc \"PD1\" \"4.6\" \"5.2\"", "602. CheckCFAdc \"PD2\" \"-.15\" \".3\"", "606. CheckCFAdc \"PD1\" \".5\" \"1.5\"", "607. CheckCFAdc \"PD2\" \".5\" \"2.4\"", "614. CheckCFAdc \"PD1\" \"2.3\" \"2.75\"", "615. CheckCFAdc \"PD2\" \"2.3\" \"2.65\"", "618. CheckCFAdc \"PD1\" \"4.5\" \"5.0\"", "620. CheckCanRxStatus \"0\"", "622. CheckCFAdc \"PD1\" \"-.15\" \".3\"", "623. CheckCFAdc \"PD2\" \"2.3\" \"2.7\"", "624. CheckCanRxStatus \"1\"", "628. CheckCFAdc \"PD1\" \"2.3\" \"2.7\"", "629. CheckCFAdc \"PD2\" \"-.15\" \".3\"", "630. CheckCanRxStatus \"0\"", "655. CheckCFAdc \"PD1\" \"-.15\" \".3\"", "656. CheckCFAdc \"PD2\" \"2.2\" \"2.65\"", "659. CheckCFAdc \"PD1\" \"4.4\" \"4.9\"", "660. CheckCFAdc \"PD2\" \".2\" \".6\"", "667. CheckCFAdc \"PD1\" \"-.15\" \".3\"", "668. CheckCFAdc \"PD2\" \"6.9\" \"7.7\"", "688. CheckCFAdc \"PD1\" \"1.0\" \"1.5\"", "689. CheckCFAdc \"PD2\" \".1\" \"1.0\"", "699. CheckCFAdc \"PD1\" \"6.9\" \"7.7\"", "707. CheckCFAdc \"PD1\" \"-.15\" \".3\"", "708. CheckCFAdc \"PD2\" \"4.4\" \"4.9\"", "710. CheckCFAdc \"PD2\" \"-.15\" \".3\"", "724. CheckCFAdc \"PD1\" \"2.3\" \"2.7\"", "725. CheckCFAdc \"PD2\" \"2.3\" \"2.7\"", "727. CheckCFAdc \"PD1\" \"4.4\" \"5.0\"", "729. CheckCanRxStatus \"0\"", "731. CheckCFAdc \"PD1\" \"-.15\" \".3\"", "732. CheckCFAdc \"PD2\" \"2.3\" \"2.7\"", "733. CheckCanRxStatus \"1\"", "737. CheckCFAdc \"PD1\" \"2.3\" \"2.7\"", "738. CheckCFAdc \"PD2\" \"-.15\" \".3\"", "739. CheckCanRxStatus \"0\"", "757. CheckCFAdc \"PD1\" \"-.15\" \".3\"", "758. CheckCFAdc \"PD2\" \"7.3\" \"8.0\"", "761. CheckCFAdc \"PD1\" \"3.4\" \"3.85\"", "762. CheckCFAdc \"PD2\" \"7.3\" \"8.0\"", "778. CheckFpgaRegister \"984\" \"0\" \"1\"", "781. CheckCFAdc \"PD1\" \"-.15\" \".44\"", "782. CheckCFAdc \"PD2\" \"14\" \"15\"", "783. CheckFpgaRegister \"984\" \"0\" \"0\"", "785. CheckFpgaRegister \"984\" \"0\" \"1\"", "787. CheckCFAdc \"PD2\" \"-.15\" \".4\"", "788. CheckCFAdc \"PD1\" \"14\" \"15\"", "789. CheckFpgaRegister \"984\" \"0\" \"0\"", "791. CheckFpgaRegister \"984\" \"0\" \"1\"", "794. CheckCFAdc \"PD1\" \"-.15\" \".44\"", "795. CheckCFAdc \"PD2\" \"-.15\" \".4\"", "796. CheckFpgaRegister \"984\" \"0\" \"0\"", "798. CheckFpgaRegister \"984\" \"0\" \"1\"", "800. CheckCFAdc \"PD1\" \"14\" \"15\"", "801. CheckCFAdc \"PD2\" \"14\" \"15\"", "802. CheckFpgaRegister \"984\" \"0\" \"1\"", "809. CheckCFAdc \"PD1\" \"1.2\" \"1.5\"", "810. CheckFpgaRegister \"984\" \"0\" \"0\"", "812. CheckCFAdc \"PD1\" \"2.2\" \"2.65\"", "813. CheckFpgaRegister \"984\" \"0\" \"1\"", "838. CheckCFAdc \"PD3\" \"4.5\" \"5.0\"", "839. CheckCFAdc \"PD4\" \"4.5\" \"5.0\"", "844. CheckCFAdc \"PD3\" \"4.1\" \"4.55\"", "845. CheckCFAdc \"PD4\" \"4.1\" \"4.55\"", "850. CheckCFAdc \"PD3\" \"2.2\" \"2.6\"", "851. CheckCFAdc \"PD4\" \"2.2\" \"2.6\"", "858. CheckCFAdc \"PD3\" \"4.3\" \"4.8\"", "859. CheckCFAdc \"PD4\" \"4.3\" \"4.8\"", "866. CheckCFAdc \"PD3\" \"4.0\" \"4.45\"", "867. CheckCFAdc \"PD4\" \"4.0\" \"4.45\"", "874. CheckCFAdc \"PD3\" \"4.3\" \"4.75\"", "875. CheckCFAdc \"PD4\" \"4.3\" \"4.75\"", "882. CheckCFAdc \"PD3\" \"4.1\" \"4.55\"", "883. CheckCFAdc \"PD4\" \"4.1\" \"4.55\"", "890. CheckCFAdc \"PD3\" \"3.7\" \"4.15\"", "891. CheckCFAdc \"PD4\" \"3.7\" \"4.15\"", "898. CheckCFAdc \"PD3\" \"3.6\" \"4.0\"", "899. CheckCFAdc \"PD4\" \"3.6\" \"4.0\"", "906. CheckCFAdc \"PD3\" \"3.45\" \"3.85\"", "907. CheckCFAdc \"PD4\" \"3.45\" \"3.85\"", "914. CheckCFAdc \"PD3\" \"3.3\" \"3.7\"", "915. CheckCFAdc \"PD4\" \"3.3\" \"3.7\"", "922. CheckCFAdc \"PD3\" \"3.1\" \"3.5\"", "923. CheckCFAdc \"PD4\" \"3.1\" \"3.5\"", "930. CheckCFAdc \"PD3\" \"2.2\" \"2.6\"", "931. CheckCFAdc \"PD4\" \"2.2\" \"2.6\"", "938. CheckCFAdc \"PD3\" \"4.5\" \"5.0\"", "939. CheckCFAdc \"PD4\" \"4.5\" \"5.0\"", "946. CheckCFAdc \"PD3\" \"-.15\" \".3\"", "947. CheckCFAdc \"PD4\" \"-.15\" \".3\"", "965. CheckCFAdc \"PD3\" \"6.95\" \"7.7\"", "966. CheckCFAdc \"PD4\" \"6.95\" \"7.7\"", "971. CheckCFAdc \"PD3\" \"4.5\" \"5.0\"", "972. CheckCFAdc \"PD4\" \"4.5\" \"5.0\"", "991. CheckCFAdc \"PD3\" \"2.2\" \"2.6\"", "996. CheckFpgaRegister \"8A8\" \"2\" \"0\"", "997. CheckFpgaRegister \"8A8\" \"3\" \"0\"", "1002. CheckFpgaRegister \"8A8\" \"2\" \"1\"", "1003. CheckFpgaRegister \"8A8\" \"3\" \"1\"", "1026. CheckCFAdc \"PD2\" \"2.2\" \"2.65\"", "1027. CheckCFAdc \"PD4\" \"-.15\" \"1.1\"", "1031. CheckCFAdc \"PD4\" \"2.2\" \"2.65\"", "1037. CheckCFAdc \"PD4\" \"2.2\" \"2.65\"", "1043. CheckCFAdc \"PD4\" \"2.2\" \"2.65\"", "1049. CheckCFAdc \"PD4\" \"2.2\" \"2.65\"", "1055. CheckCFAdc \"PD4\" \"2.2\" \"2.65\"", "1061. CheckCFAdc \"PD4\" \"2.2\" \"2.65\"", "1067. CheckCFAdc \"PD4\" \"2.2\" \"2.65\"", "1073. CheckCFAdc \"PD4\" \"2.2\" \"2.65\"", "1079. CheckCFAdc \"PD4\" \"2.2\" \"2.65\"", "1085. CheckCFAdc \"PD4\" \"2.2\" \"2.65\"", "1091. CheckCFAdc \"PD4\" \"2.2\" \"2.65\"", "1097. CheckCFAdc \"PD4\" \"2.2\" \"2.65\"", "1103. CheckCFAdc \"PD4\" \"2.2\" \"2.65\"", "1119. CheckCFAdc \"PD3\" \"-.15\" \".3\"", "1120. CheckCFAdc \"PD4\" \"7.2\" \"7.9\"", "1123. CheckCFAdc \"PD3\" \"3.4\" \"3.8\"", "1124. CheckCFAdc \"PD4\" \"7.2\" \"7.9\"", "1138. CheckFpgaRegister \"85A\" \"0\" \"0\"", "1143. CheckFpgaRegister \"85A\" \"0\" \"1\"", "1150. CheckFpgaRegister \"87A\" \"0\" \"1\"", "1151. CheckFpgaRegister \"87A\" \"1\" \"0\"", "1155. CheckFpgaRegister \"87A\" \"0\" \"0\"", "1156. CheckFpgaRegister \"87A\" \"1\" \"1\"", "1204. CheckCFAdc \"PD1\" \"2.2\" \"2.65\"", "1205. CheckCFAdc \"PD2\" \"2.2\" \"2.65\"", "1209. CheckCFAdc \"PD1\" \"4.5\" \"5.0\"", "1210. CheckCFAdc \"PD2\" \"-.15\" \".3\"", "1216. CheckCFAdc \"PD2\" \"-.15\" \".3\"", "1224. CheckCFAdc \"PD2\" \"-.15\" \".3\"", "1232. CheckCFAdc \"PD2\" \"-.15\" \".3\"", "1240. CheckCFAdc \"PD2\" \"-.15\" \".3\"", "1248. CheckCFAdc \"PD2\" \"-.15\" \".3\"", "1256. CheckCFAdc \"PD2\" \"-.15\" \".3\"", "1264. CheckCFAdc \"PD2\" \"-.15\" \".3\"", "1272. CheckCFAdc \"PD2\" \"-.15\" \".3\"", "1280. CheckCFAdc \"PD2\" \"-.15\" \".3\"", "1288. CheckCFAdc \"PD2\" \"-.15\" \".3\"", "1296. CheckCFAdc \"PD2\" \"-.15\" \".3\"", "1304. CheckCFAdc \"PD2\" \"-.15\" \".3\"", "1312. CheckCFAdc \"PD2\" \"-.15\" \".3\"", "1328. CheckFpgaRegister \"984\" \"02\" \"0\"", "1336. CheckFpgaRegister \"984\" \"02\" \"1\"", "1340. CheckFpgaRegister \"984\" \"02\" \"0\"", "1347. CheckFpgaRegister \"984\" \"02\" \"1\"", "1351. CheckGepWifiModule \"'SSP Wifi'\"", "1359. CheckRealtimeClock \"2\"", "1467. CheckCFAdc \"PD1\" \"14\" \"15.5\"", "1468. CheckCFAdc \"PD3\" \"14\" \"15.5\""])   [LabVIEW 2015]
uses:
  ResultCluster.ctl
  <vilib>/Utility/config.llb/Read Key (String).vi
  <vilib>/Utility/config.llb/Read Key (Double).vi
  <vilib>/Utility/config.llb/NI_LVConfig.lvlib
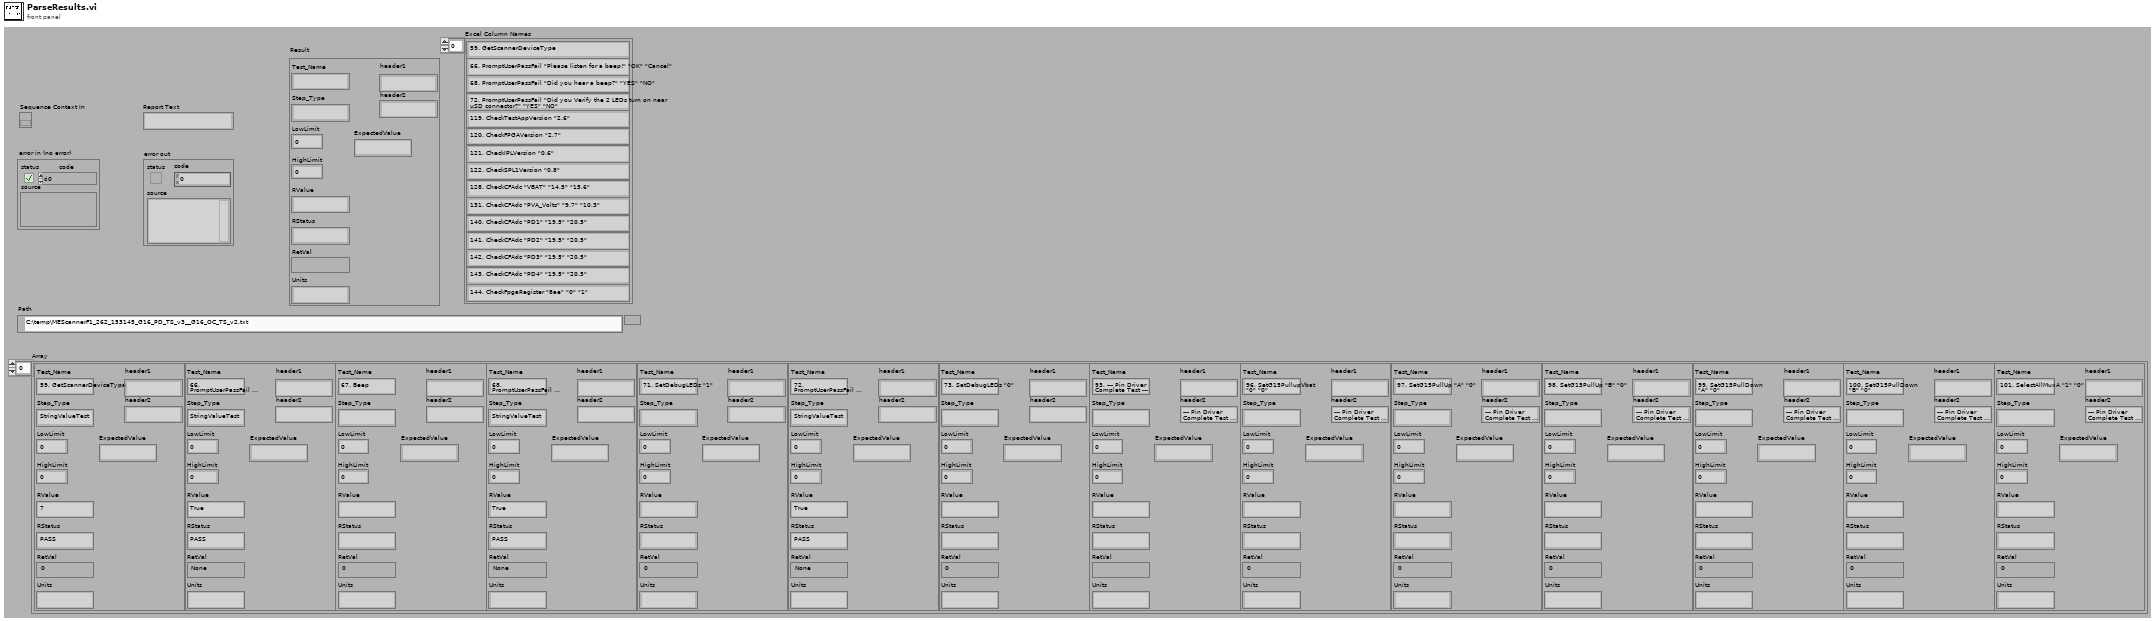
[diagram p1: front panel]
types:
  T1 = typedef "ResultCluster.ctl" = cluster{"Test_Name":string, "Step_Type":string, "LowLimit":dbl, "HighLimit":dbl, "RValue":string, "RStatus":string, "RetVal":string, "Units":string, "header1":string, "header2":string, "ExpectedValue":string}
  T2 = typedef "NI_LVConfig.lvlib/Config Data RefNum.ctl" = refnum<k1>
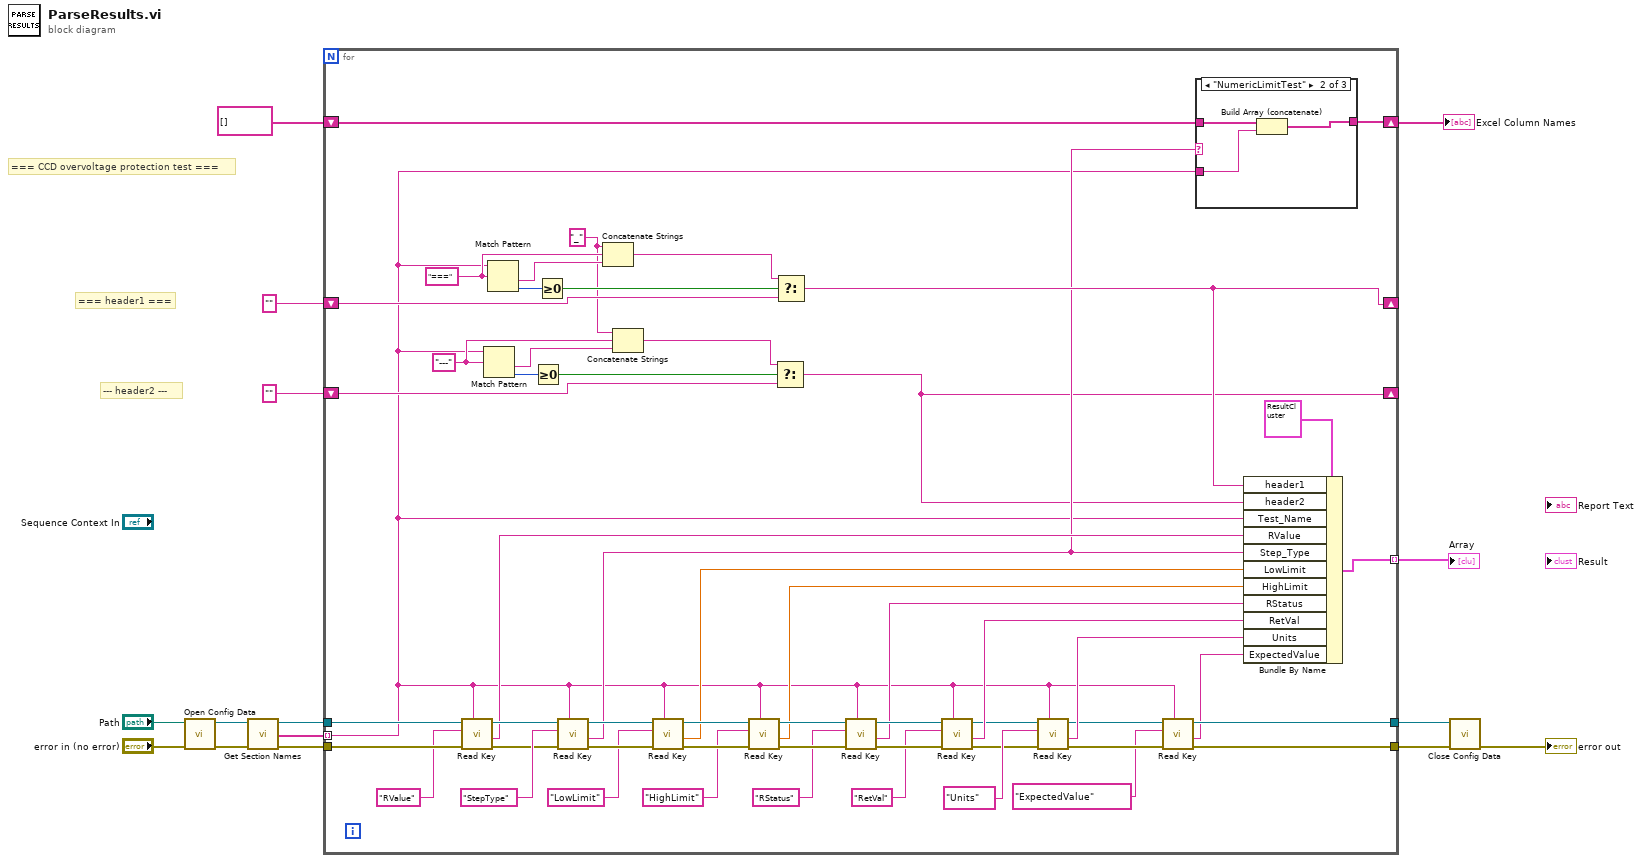
[diagram p0: block diagram]
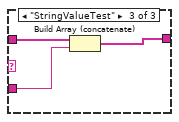
[diagram p3: hidden frame]
diagram:
  # "=== CCD overvoltage protection test ==="
  # "--- header2 ---"
  # "=== header1 ==="
  n1 = call <vilib>:"Open Config Data.vi"("error in (no error)"="error in (no error)", "configuration file path"="Path") -> ("error out"=w11:errorcluster, "refnum"=w14:T2)  [unwired: 7 in, 1 out]
  n2 = call <vilib>:"Get Section Names.vi"("error in (no error)"=w11, "refnum"=w14) -> ("error out"=w10:errorcluster, "section names"=w13:string[], "refnum out"=w12:T2)  [unwired: 7 in]
  n3 = for {
    tunnel: w13 -> [w17] mode=indexing
    tunnel: w12 -> [w69]
    tunnel: w10 -> [w65]
    tunnel: [w50] -> w9 mode=indexing
    tunnel: [w21] -> w8
    tunnel: [w19] -> w5
    shift-right: [w28] -> _
    shift-left: "" ("key") -> [w39]
    shift-right: [w23] -> _
    shift-left: "" ("key") -> [w37]
    shift-right: [w25] -> w1
    shift-left: string[] [] -> [w26]
    w22 = "_" ("string")
    w31 = "---" ("regular expression")
    w32 = "===" ("regular expression")
    n4 = call-poly <vilib>:"Read Key.vi"("section"=w17, "error in (no error)"=w65, "key"="RValue", "refnum"=w69) -> ("error out"=w48:errorcluster, "value"=w46:string, "refnum out"=w47:T2)  [unwired: 4 in, 1 out]
    n5 = Match Pattern(string=w17, regular expression=w31) -> (after substring=w30:string, offset past match=w38:i32)  [unwired: 1 in, 2 out]
    n6 = Match Pattern(string=w17, regular expression=w32) -> (after substring=w33:string, offset past match=w40:i32)  [unwired: 1 in, 2 out]
    n7 = Greater Or Equal To 0?(x=w38) -> (x >= 0?=w35:bool)
    n8 = Greater Or Equal To 0?(x=w40) -> (x >= 0?=w34:bool)
    n9 = call-poly <vilib>:"Read Key.vi"("section"=w17, "error in (no error)"=w48, "key"="StepType", "refnum"=w47) -> ("error out"=w64:errorcluster, "value"=w24:string, "refnum out"=w67:T2)  [unwired: 4 in, 1 out]
    n10 = Concatenate Strings(w22, w32, w33) -> (w29:string)
    n11 = Concatenate Strings(w22, w31, w30) -> (w27:string)
    n12 = call-poly <vilib>:"Read Key.vi"("section"=w17, "error in (no error)"=w64, "key"="LowLimit", "refnum"=w67) -> ("error out"=w63:errorcluster, "value"=w57:dbl, "refnum out"=w68:T2)  [unwired: 4 in, 1 out]
    n13 = call-poly <vilib>:"Read Key.vi"("section"=w17, "error in (no error)"=w63, "key"="HighLimit", "refnum"=w68) -> ("error out"=w62:errorcluster, "value"=w56:dbl, "refnum out"=w66:T2)  [unwired: 4 in, 1 out]
    n14 = Select(t=w27, s=w35, f=w37) -> (s? t:f=w23:string)
    n15 = Select(t=w29, s=w34, f=w39) -> (s? t:f=w28:string)
    n16 = call-poly <vilib>:"Read Key.vi"("section"=w17, "error in (no error)"=w62, "key"="RStatus", "refnum"=w66) -> ("error out"=w60:errorcluster, "value"=w55:string, "refnum out"=w61:T2)  [unwired: 4 in, 1 out]
    n17 = call-poly <vilib>:"Read Key.vi"("section"=w17, "error in (no error)"=w60, "key"="RetVal", "refnum"=w61) -> ("error out"=w42:errorcluster, "value"=w54:string, "refnum out"=w41:T2)  [unwired: 4 in, 1 out]
    n18 = call-poly <vilib>:"Read Key.vi"("section"=w17, "error in (no error)"=w42, "key"="Units", "refnum"=w41) -> ("error out"=w43:errorcluster, "value"=w44:string, "refnum out"=w20:T2)  [unwired: 4 in, 1 out]
    n19 = call-poly <vilib>:"Read Key.vi"("section"=w17, "error in (no error)"=w43, "key"="ExpectedValue", "refnum"=w20) -> ("error out"=w21:errorcluster, "value"=w16:string, "refnum out"=w19:T2)  [unwired: 4 in, 1 out]
    n20 = case shown="\"NumericLimitTest\"" w24 {
      tunnel: w17 -> [_ w73 w76]
      tunnel: w26 -> [w70 w72 w75]
      tunnel: [w70 w71 w74] -> w25
      frame "False", Default {
      }
      frame "NumericLimitTest" {
        n21 = Build Array (concatenate)(w72, w73) -> (w71:string[])
      }
      frame "StringValueTest" {
        n22 = Build Array (concatenate)(w75, w76) -> (w74:string[])
      }
    }
    n23 = Bundle By Name(cluster=T1 {"Test_Name"="", "Step_Type"="", "LowLimit"=0.0, "HighLimit"=0.0, "RValue"="", "RStatus"="", "RetVal"="", "Units"="", "header1"="", "header2"="", "ExpectedValue"=""} ("Result"), "header1"=w28, "header2"=w23, "Test_Name"=w17, "RValue"=w46, "Step_Type"=w24, "LowLimit"=w57, "HighLimit"=w56, "RStatus"=w55, "RetVal"=w54, "Units"=w44, "ExpectedValue"=w16) -> (w50:T1)
  }
  "Array" <- w9
  "Excel Column Names" <- w1
  n24 = call <vilib>:"Close Config Data.vi"("error in (no error)"=w8, "refnum"=w5) -> ("error out"=→"error out":errorcluster)  [unwired: 8 in, 1 out]
